vi "NoGV_Omniax_MotorDrive_XYZR_20111213stable2.vi"() -> ()   [LabVIEW 2010]
uses:
  <vilib>/Utility/file.llb/Read From Spreadsheet File (string).vi
  <vilib>/Utility/file.llb/Read From Spreadsheet File (DBL).vi
  <vilib>/Instr/_visa.llb/VISA Configure Serial Port (Instr).vi
  <vilib>/Utility/file.llb/Write To Spreadsheet File (string).vi
  <vilib>/Utility/file.llb/Write To Spreadsheet File (DBL).vi
panel:
  out "Scanning":bool
  out "Laser Shutter":bool
  in  "SHUTTER SYNC":bool
  in  "Laser Shutter":bool
  out "#th loop":dbl
  in  "# of loops":dbl
  in  "LOOP":bool
  out "OP":bool
  out "CL":bool
  out "V5 Valve \nopend/closed":bool
  in  "OK Button":bool
  out "STATUS":string
  in  "Delete Button":bool
  in  "String":string
  in  "Add Button":bool
  in  "Set Button":bool
  in  "Preset positions":i32(ring) items=["ZERO", "Default", "CDOSE", "QMS", "test", "test2", "test3", "yag position", "Sample Long Edge  ", "SPUTTER POS"]
  out "Presets":i32[][](array[numeric])
  out "X MINPOS":i32=-94296
  out "X MAXPOS":i32=-34296
  out "Y MINPOS":i32=-94296
  out "Y MAXPOS":i32=-34296
  out "R MAXPOS":i32=-34296
  out "R MINPOS":i32=-94296
  out "Z MINPOS":i32=-94296
  out "Z MAXPOS":i32=-34296
  in  "HARDSTOP":bool
  in  "GO":bool
  out "XYZR VEL PV Array":i32[](array[numeric])
  out "XYZ in RANGE Array":bool[](array[boolean])
  out "STEP SP Array":i32[](array[numeric])
  out "RUNHOLDArray":i32[](array[numeric])
  out "ZCONSTArray":dbl[](array[numeric])
  out "RCONSTArray":dbl[](array[numeric])
  out "XCONSTArray":dbl[](array[numeric])
  out "YCONSTArray":dbl[](array[numeric])
  out "Error Array":errorcluster[](array[cluster])
  out "COM PORT Array":refnum<visa-resource-name>[](array[refnum])
  out "Z COM PORT":refnum<visa-resource-name>="COM6"
  in  "Tab Control 3":enum32{"Status", "Reset"}(tab)
  out "Y in Range":bool
  out "Y Scan":bool
  out "Y in Motion":bool
  out "Y Backlash corr":bool
  out "X  in Range":bool
  out "X Scan":bool
  out "X  in Motion":bool
  out "X Backlash corr":bool
  out "Z in Range":bool
  out "Z Scan":bool
  out "Z in Motion":bool
  out "Z Backlash corr":bool
  out "R in Range":bool
  out "R Scan":bool
  out "R in Motion":bool
  out "R Backlash corr":bool
  out "X Ready":bool
  out "Y Ready":bool
  out "Z Ready":bool
  out "R Ready":bool
  in  "Reset Y Position mm":dbl
  out "Reset Y Motor Steps":i32
  in  "Reset X Position mm":dbl
  out "Reset X Motor Steps":i32
  in  "Reset Z Position mm":dbl
  out "Reset Z Motor Steps":i32
  in  "Reset R Position deg":dbl
  out "Reset R Motor Steps":i32
  in  "Reset":bool
  in  "Tab Control 2":enum32{"mm", "step"}(tab)
  in  "X Scan Length SP mm":dbl
  in  "X Scan Velocity SP mm/sec":dbl
  in  "Y Scan Length SP mm":dbl
  in  "Y Scan Velocity SP mm/sec":dbl
  in  "Set Scan \nParameters":bool
  in  "Z Scan Length SP mm":dbl
  in  "Z Scan Velocity SP mm/sec":dbl
  in  "R Scan Length SP deg":dbl
  in  "R Scan Velocity SP deg/sec":dbl
  in  "Z as dominating length":bool
  in  "X Scan Velocity SP steps/sec":i32=1 min=1 max=102400 step=1
  in  "X Scan Length SP steps":i32 min=-2304000 max=2304000 step=100
  out "X Scan length MV mm":dbl
  out "X Scan velocity MV mm/sec":dbl format="%#_6f"
  in  "Y Scan Velocity SP steps/sec":i32=1 min=1 max=102400 step=1
  in  "Y Scan Length SP steps":i32 min=-2304000 max=2304000 step=100
  out "Y Scan length MV mm":dbl
  out "Y Scan velocity MV mm/sec":dbl format="%#_6f"
  in  "Z Scan Velocity SP steps/sec":i32=1 min=1 max=204800 step=1
  in  "Z Scan Length SP steps":i32 min=-10240000 max=92160000 step=100
  out "Z Scan length MV mm":dbl
  out "Z Scan velocity MV mm/sec":dbl format="%#_6f"
  in  "R Scan Velocity SP steps/sec":i32=1 min=1 max=102400 step=1
  in  "R Scan Length SP steps":i32 min=-1501867 max=4642133 step=100
  out "R Scan length MV deg":dbl
  out "R Scan velocity MV deg/sec":dbl format="%#_6f"
  out "atan Y/Z":dbl
  in  "Tab Control":enum32{"mm", "step"}(tab)
  in  "X Position SP mm":dbl
  in  "X Velocity SP mm/sec":dbl
  in  "X Move Set":bool
  in  "Y Move Set":bool
  in  "Y Position SP mm":dbl
  in  "Y Velocity SP mm/sec":dbl
  in  "Z Position SP mm":dbl
  in  "Z Velocity SP mm/sec":dbl
  in  "Z Move Set":bool
  in  "R Position SP deg":dbl
  in  "R Velocity SP deg/sec":dbl
  in  "R Move Set":bool
  in  "X Velocity SP step/sec":i32 min=1 max=128000
  out "X Velocity MV mm/sec":dbl
  in  "Y Velocity SP step/sec":i32 min=1 max=128000
  out "Y Velocity MV mm/sec":dbl
  in  "Z Velocity SP step/sec":i32 min=1 max=204800
  out "Z Velocity MV mm/sec":dbl
  in  "R Velocity SP step/sec":i32 min=1 max=20000
  out "R Velocity MVdeg/sec":dbl
  in  "Y Step SP":i32=-20000 min=-2304000 max=2304000 step=500
  out "Y Position MV mm":dbl
  in  "X Step SP":i32=-20000 min=-2304000 max=2304000 step=500
  out "X Position MV mm":dbl
  in  "Z Step SP":i32=-20000 min=0 max=102400000 step=500
  out "Z Position MV mm":dbl
  in  "R Step SP":i32=-20000 min=-6144000 max=0 step=500
  out "R Position MV deg":dbl
  out "X Step PV":i32 max=2000
  out "Y Step PV":i32 max=2000
  out "Z Step PV":i32 max=2000
  out "R Step PV":i32 max=2000
  in  "Clear ZY":bool
  out "ZY Graph":cluster{dbl[], dbl[]}(graph)
  out "ZR Graph":cluster{"Y":dbl[], "Y":dbl[]}[](graph)
  out "XY Graph":cluster{"Y":dbl[], "Y":dbl[]}[](graph)
  out "X Scan Duration":dbl
  out "Y Scan Duration":dbl
  out "Z Scan Duration":dbl
  out "R Scan Duration":dbl
  out "R Backlash steps/sec":i32
  out "R Backlash":i32
  out "R Holding Current %":i32
  out "R Run Current %":i32
  out "R offset deg":dbl
  out "R deg/rev":dbl
  out "R steps/rev":u32
  out "R velocity PV step/sec":i32
  out "R COM PORT":refnum<visa-resource-name>="COM5"
  out "R Position deg PV":dbl=270.5
  out "Z Backlash steps/sec":i32
  out "Z Backlash":i32
  out "Z Holding Current %":i32
  out "Z Run Current %":i32
  out "Z offset mm":dbl
  out "Z mm/rev":dbl
  out "Z steps/rev":u32
  out "Z  velocity PV step/sec":i32
  out "Z Position mm PV":dbl=45.0
  out "X Position mm PV":dbl
  out "X velocity PV step/sec":i32
  in  "Send scan parameter":bool
  out "X Backlash steps/sec":i32
  out "X Backlash":i32
  out "X Holding Current %":i32
  out "X Run Current %":i32
  out "X offset mm":dbl
  out "X mm/rev":dbl
  out "X steps/rev":u32
  out "X COM PORT":refnum<visa-resource-name>="COM5"
  out "Y Backlash steps/sec":i32
  out "Y Backlash":i32
  out "Y Holding Current %":i32
  out "Y Run Current %":i32
  in  "Scan Cancel":bool
  out "Y Position mm PV":dbl
  out "Y offset mm":dbl
  out "Y mm/rev":dbl
  out "Y steps/rev":u32
  out "Y velocity PV step/sec":i32
  in  "Scan Go":bool
  in  "Stop":bool
  out "Y COM PORT":refnum<visa-resource-name>="COM5"
  # "MX"
  # "MY"
  # "MZ"
  # "MR"
  # "V5 Indicators"
  # "L"
  # "M"
  # "B"
  # "S"
  # "R"
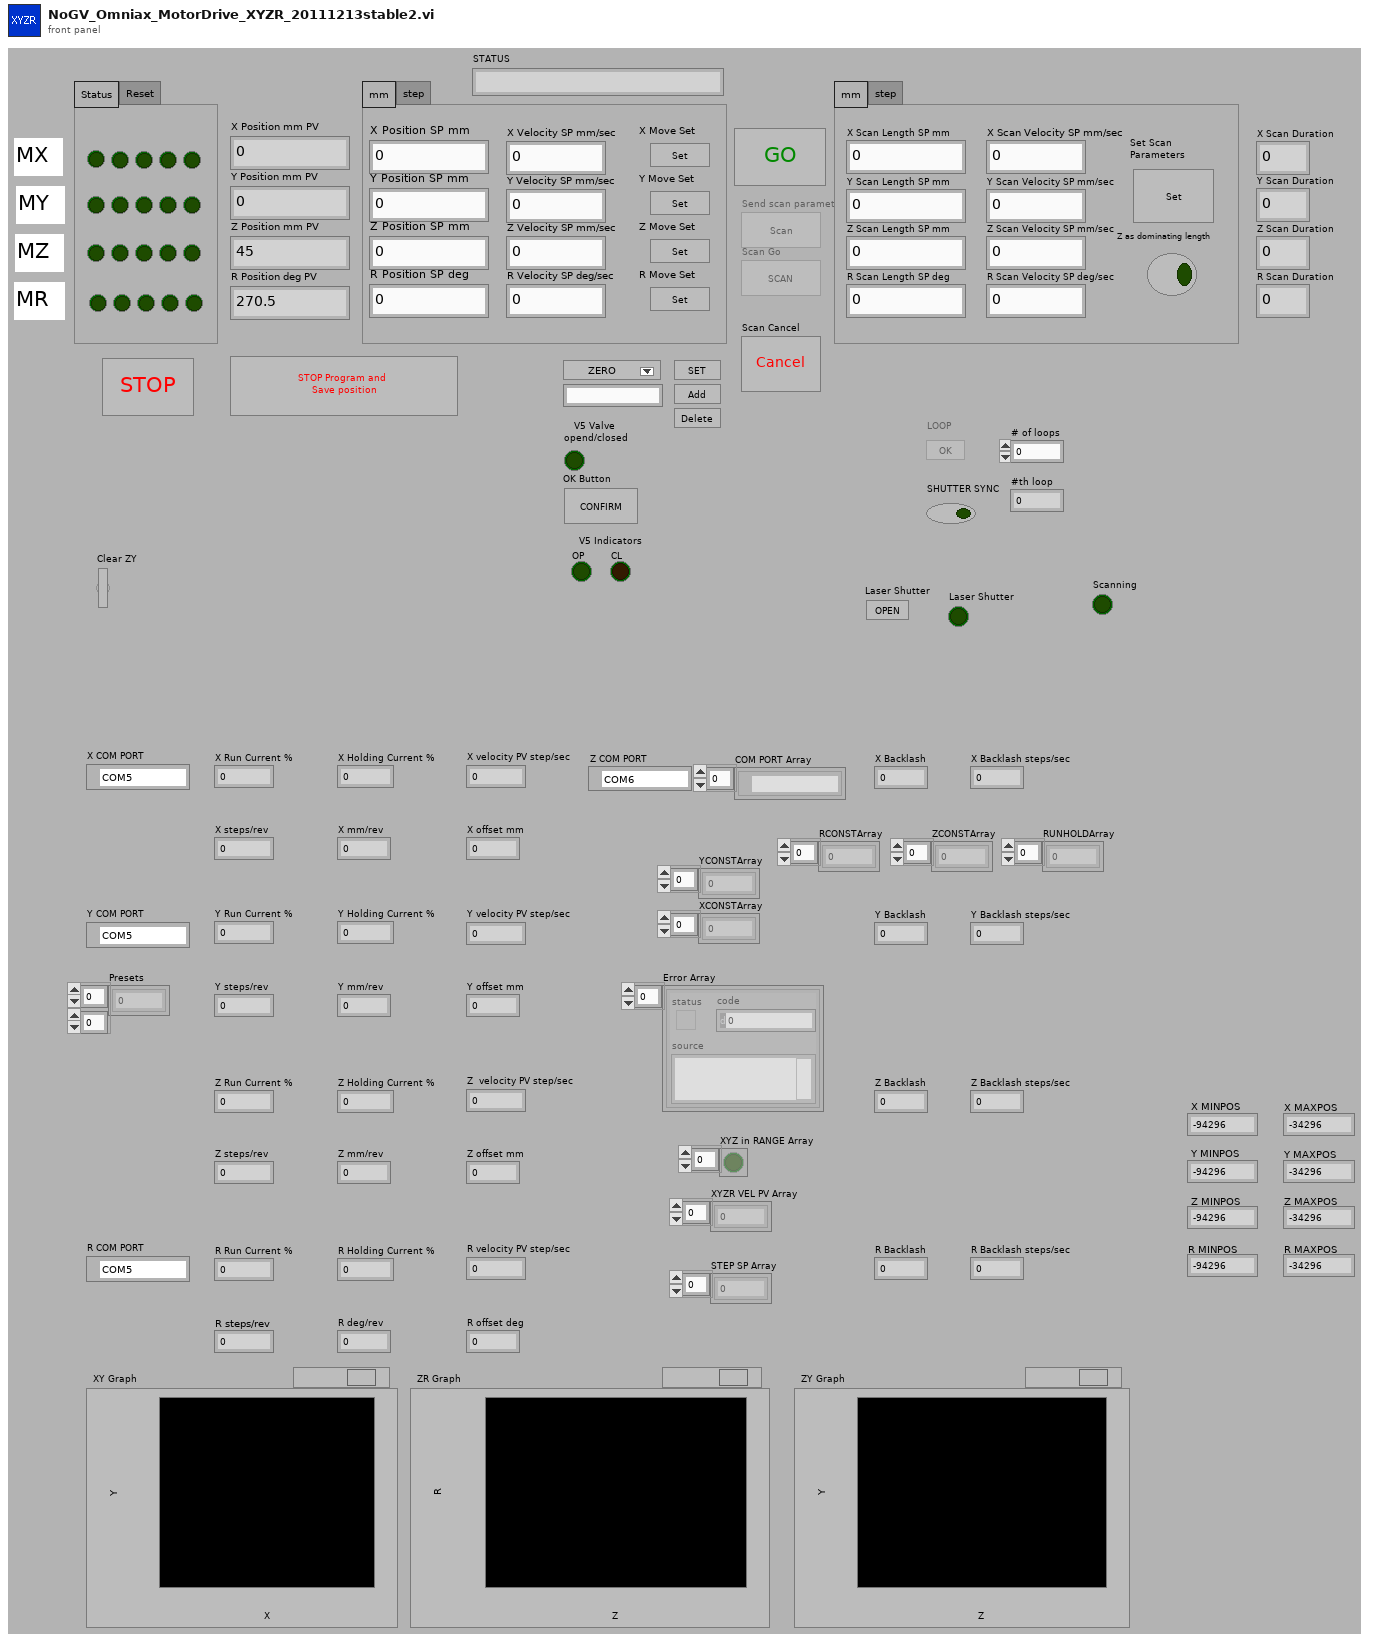
[diagram p1: front panel]
types:
  T1 = cluster{"Error Array OUT[0]":errorcluster, "Error Array OUT[1]":errorcluster, "Error Array OUT[2]":errorcluster, "Error Array OUT[3]":errorcluster, "Error Array OUT[4]":errorcluster, "Error Array OUT[5]":errorcluster, "Error Array OUT[6]":errorcluster, "Error Array OUT[7]":errorcluster, "Error Array OUT[8]":errorcluster}
  T2 = cluster{"COM PORT Array OUT[0]":refnum<visa-resource-name>, "COM PORT Array OUT[1]":refnum<visa-resource-name>, "COM PORT Array OUT[2]":refnum<visa-resource-name>, "COM PORT Array OUT[3]":refnum<visa-resource-name>, "COM PORT Array OUT[4]":refnum<visa-resource-name>, "COM PORT Array OUT[5]":refnum<visa-resource-name>, "COM PORT Array OUT[6]":refnum<visa-resource-name>, "COM PORT Array OUT[7]":refnum<visa-resource-name>, "COM PORT Array OUT[8]":refnum<visa-resource-name>}
  T3 = cluster{"STEP SP Array OUT[0]":i32, "STEP SP Array OUT[1]":i32, "STEP SP Array OUT[2]":i32, "STEP SP Array OUT[3]":i32, "STEP SP Array OUT[4]":i32, "STEP SP Array OUT[5]":i32, "STEP SP Array OUT[6]":i32, "STEP SP Array OUT[7]":i32, "STEP SP Array OUT[8]":i32}
  T4 = cluster{"XYZR MAX MIN POS[0]":i32, "XYZR MAX MIN POS[1]":i32, "XYZR MAX MIN POS[2]":i32, "XYZR MAX MIN POS[3]":i32, "XYZR MAX MIN POS[4]":i32, "XYZR MAX MIN POS[5]":i32, "XYZR MAX MIN POS[6]":i32, "XYZR MAX MIN POS[7]":i32, "XYZR MAX MIN POS[8]":i32}
  T5 = cluster{"XYZ in RANGE Array OUT[0]":bool, "XYZ in RANGE Array OUT[1]":bool, "XYZ in RANGE Array OUT[2]":bool, "XYZ in RANGE Array OUT[3]":bool, "XYZ in RANGE Array OUT[4]":bool, "XYZ in RANGE Array OUT[5]":bool, "XYZ in RANGE Array OUT[6]":bool, "XYZ in RANGE Array OUT[7]":bool, "XYZ in RANGE Array OUT[8]":bool}
  T6 = cluster{"XY Max Min array OUT[0]":dbl, "XY Max Min array OUT[1]":dbl, "XY Max Min array OUT[2]":dbl, "XY Max Min array OUT[3]":dbl, "XY Max Min array OUT[4]":dbl, "XY Max Min array OUT[5]":dbl, "XY Max Min array OUT[6]":dbl, "XY Max Min array OUT[7]":dbl, "XY Max Min array OUT[8]":dbl}
  T7 = cluster{"XYZR VEL PV Array OUT[0]":i32, "XYZR VEL PV Array OUT[1]":i32, "XYZR VEL PV Array OUT[2]":i32, "XYZR VEL PV Array OUT[3]":i32, "XYZR VEL PV Array OUT[4]":i32, "XYZR VEL PV Array OUT[5]":i32, "XYZR VEL PV Array OUT[6]":i32, "XYZR VEL PV Array OUT[7]":i32, "XYZR VEL PV Array OUT[8]":i32}
  T8 = cluster{"[0]":i32, "[1]":i32, "[2]":i32, "[3]":i32, "[4]":i32, "[5]":i32, "[6]":i32, "[7]":i32, "[8]":i32}
  T9 = enum8{"Enabled", "Disabled", "Disabled and Grayed Out"}
  T10 = enum16{"Stop", "Reset", "Run Current", "Holding Current", "Accel Rate", "Decel Rate", "Move to Relative Position", "Move to Absolute Position", "Echo Mode", "Print Parameter", "Send String", "Microstep Resolution", "Set Current Position", "Max Velocity"}
  T11 = cluster{"Presets[0]":i32, "Presets[1]":i32, "Presets[2]":i32, "Presets[3]":i32, "Presets[4]":i32, "Presets[5]":i32, "Presets[6]":i32, "Presets[7]":i32, "Presets[8]":i32}
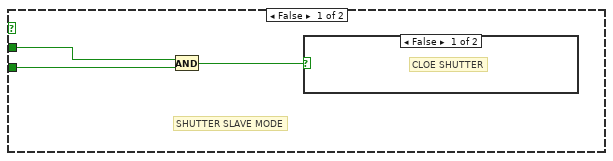
[diagram p2: hidden frame]
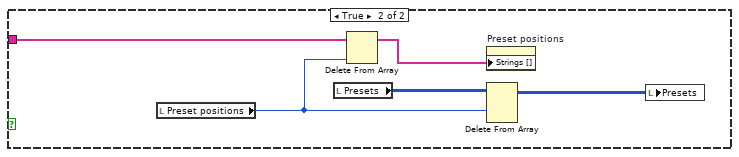
[diagram p4: hidden frame]
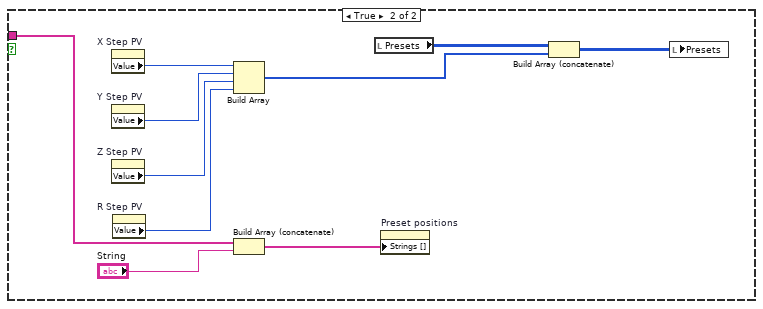
[diagram p5: hidden frame]
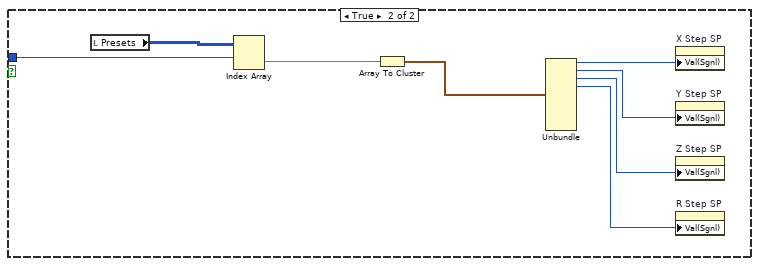
[diagram p6: hidden frame]
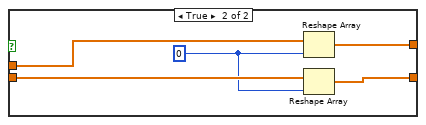
[diagram p8: hidden frame]
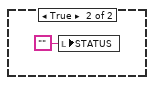
[diagram p10: hidden frame]
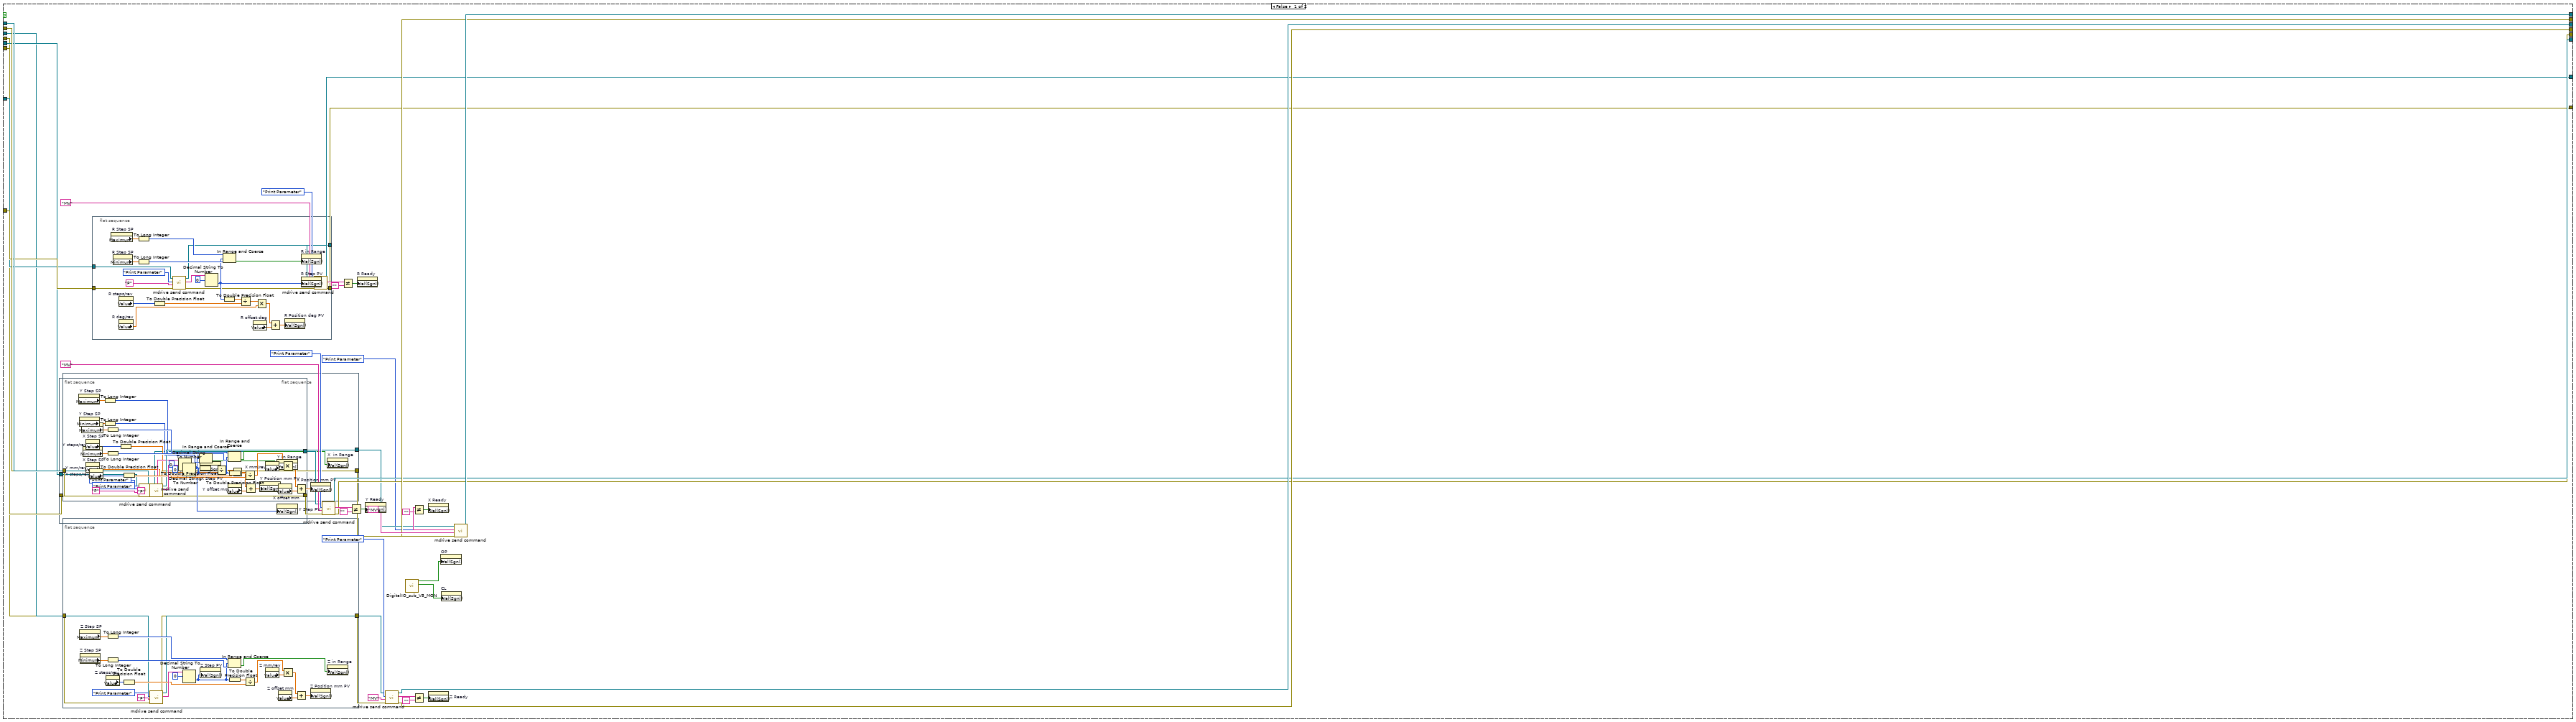
[diagram p11: hidden frame]
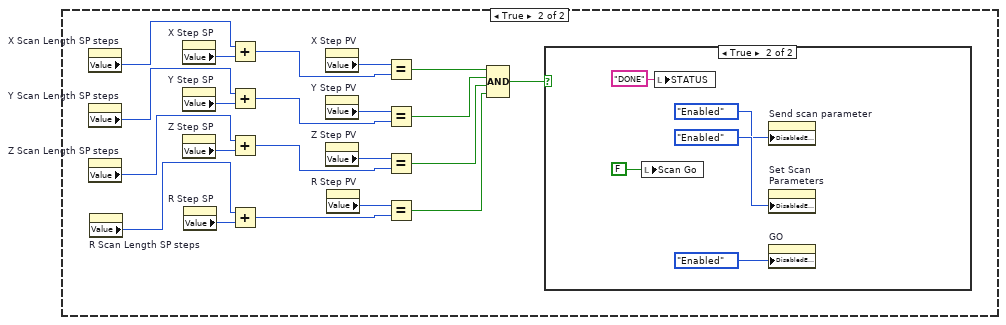
[diagram p14: hidden frame]
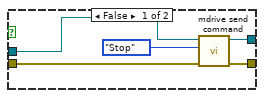
[diagram p16: hidden frame]
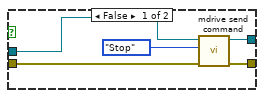
[diagram p18: hidden frame]
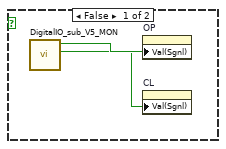
[diagram p20: hidden frame]
diagram:
  (unwired) FALSE ("LOOP MODE")
  n1 = flat-sequence {
    tunnel: [w153] -> w10
    tunnel: [w152] -> w9
    tunnel: [w151] -> w8
    tunnel: [w150] -> w7
    tunnel: [w149] -> w6
    tunnel: [w148] -> w5
    tunnel: [w147] -> w4
    tunnel: [w146] -> w3
    tunnel: [w143] -> w2
    tunnel: [w113] -> w1
    tunnel: [w188] -> w13
    tunnel: [w189] -> w14
    tunnel: [w190] -> w15
    tunnel: [w191] -> w16
    tunnel: [w192] -> w17
    tunnel: [w193] -> w18
    tunnel: [w194] -> w19
    tunnel: [w195] -> w20
    tunnel: [w196] -> w21
    tunnel: [w197] -> w22
    tunnel: w10 -> [w197]
    tunnel: w9 -> [w196]
    tunnel: w8 -> [w195]
    tunnel: w7 -> [w194]
    tunnel: w6 -> [w193]
    tunnel: w5 -> [w192]
    tunnel: w4 -> [w191]
    tunnel: w3 -> [w190]
    tunnel: w2 -> [w189]
    tunnel: w1 -> [w188]
    frame #0 {
      w113 = path "C:/Documents and Settings/b_ogasawara/Desktop/lv1/LV codes/IMS/PRESET.TXT"
      w111 = 0 ("element")
      w143 = path "C:/Documents and Settings/b_ogasawara/Desktop/lv1/LV codes/IMS/POS.TXT"
      w173 = refnum<visa-resource-name> "COM7" ("COM PORT")
      w174 = refnum<visa-resource-name> "COM5" ("COM PORT")
      w175 = refnum<visa-resource-name> "COM6" ("VISA resource name")
      w176 = refnum<visa-resource-name> "COM4" ("COM PORT")
      n2 = property on="Z Step SP" class="DigNum (strict)"() -> ("Maximum"=w68:dbl)  [unwired: 2 in, 2 out]
      n3 = property on="R Step SP" class="DigNum (strict)"() -> ("Maximum"=w66:dbl)  [unwired: 2 in, 2 out]
      n4 = property on="Z Step SP" class="DigNum (strict)"() -> ("Minimum"=w69:dbl)  [unwired: 2 in, 2 out]
      n5 = property on="R Step SP" class="DigNum (strict)"() -> ("Minimum"=w67:dbl)  [unwired: 2 in, 2 out]
      n6 = property on="X steps/rev" class="DigNum (strict)"() -> ("Value"=w84:u32)  [unwired: 2 in, 2 out]
      n7 = property on="Y steps/rev" class="DigNum (strict)"() -> ("Value"=w83:u32)  [unwired: 2 in, 2 out]
      n8 = property on="Z steps/rev" class="DigNum (strict)"() -> ("Value"=w82:u32)  [unwired: 2 in, 2 out]
      n9 = property on="R steps/rev" class="DigNum (strict)"() -> ("Value"=w81:u32)  [unwired: 2 in, 2 out]
      n10 = call "DigitalIO_sub_V5_MON.vi"() -> ("CL"=w70:bool, "OP"=w71:bool)  [unwired: 8 in]
      n11 = local read "RUNHOLDArray"() -> (w163:i32[])
      n12 = local read "STEP SP Array"() -> (w166:i32[])
      n13 = local read "XYZ in RANGE Array"() -> (w165:bool[])
      n14 = local read "XYZR VEL PV Array"() -> (w164:i32[])
      n15 = property on="R offset deg" class="DigNum (strict)"() -> ("Value"=w76:dbl)  [unwired: 2 in, 2 out]
      n16 = property on="X offset mm" class="DigNum (strict)"() -> ("Value"=w73:dbl)  [unwired: 2 in, 2 out]
      n17 = property on="Y offset mm" class="DigNum (strict)"() -> ("Value"=w74:dbl)  [unwired: 2 in, 2 out]
      n18 = property on="Z offset mm" class="DigNum (strict)"() -> ("Value"=w75:dbl)  [unwired: 2 in, 2 out]
      n19 = property on="OP" class="Bool (strict)"("Val(Sgnl)"=w71) -> ()  [unwired: 2 in, 2 out]
      n20 = property on="CL" class="Bool (strict)"("Val(Sgnl)"=w70) -> ()  [unwired: 2 in, 2 out]
      n21 = Build Array(w176, w175, w174, w173) -> (w171:refnum<visa-resource-name>[])
      n22 = Build Array(w68, w69, w66, w67) -> (w65:dbl[])
      n23 = local write "STATUS"("INITIALIZING" ("STATUS")) -> ()
      n24 = for {
        N: 4 -> [_]
        tunnel: w171 -> [w179] mode=indexing
        tunnel: [w178] -> w169 mode=indexing
        tunnel: [w177] -> w170 mode=indexing
        w181 = u16 0 items=["None", "XON/XOFF", "RTS/CTS", "XON/XOFF & RTS/CTS", "DTR/DSR", "XON/XOFF & DTR/DSR"] ("flow control (0:none)")
        w182 = u16 10 items=["1.0"=10, "1.5"=15, "2.0"=20] ("stop bits (10: 1 bit)")
        # "Stop bits"
        n25 = call-poly "VISA Configure Serial Port"("VISA resource name"=w179, "timeout (10sec)"=u32 10000, "baud rate (9600)"=u32 9600, "data bits (8)"=u16 8, "parity (0:none)"=enum16{"None", "Odd", "Even", "Mark", "Space"}."None", "stop bits (10: 1 bit)"=w182, "flow control (0:none)"=w181) -> ("VISA resource name out"=w178:refnum<visa-resource-name>, "error out"=w177:errorcluster)  [unwired: 7 in]
      }
      "COM PORT Array" <- w169
      "Error Array" <- w170
      n26 = call "InitializeMotorsXYZR_V2.vi"("COM PORT Array IN"=w169, "STEP SP Array IN"=w166, "XYZ in RANGE Array IN"=w165, "XYZR VEL PV Array IN"=w164, "RUNHOLDArray IN"=w163, "Error Array IN"=w170, "ZR Max Min array"=w65) -> ("XY Max Min array OUT"=w64:dbl[], "COM PORT Array OUT"=w168:refnum<visa-resource-name>[], "STEP SP Array OUT"=w162:i32[], "XYZ in RANGE Array OUT"=w161:bool[], "XYZR VEL PV Array OUT"=w160:i32[], "XYZR MAX MIN POS"=w145:i32[], "Error Array OUT"=w167:errorcluster[])  [unwired: 6 in]
      n27 = Array To Cluster(array=w167) -> (cluster=w158:T1)
      n28 = Array To Cluster(array=w168) -> (cluster=w159:T2)
      n29 = Array To Cluster(array=w162) -> (cluster=w157:T3)
      n30 = Array To Cluster(array=w145) -> (cluster=w154:T4)
      n31 = Array To Cluster(array=w161) -> (cluster=w156:T5)
      n32 = Array To Cluster(array=w64) -> (cluster=w63:T6)
      n33 = Array To Cluster(array=w160) -> (cluster=w155:T7)
      n34 = Unbundle(w157) -> ("STEP SP Array OUT[0]"=w127:i32, "STEP SP Array OUT[1]"=w128:i32, "STEP SP Array OUT[2]"=w129:i32, "STEP SP Array OUT[3]"=w130:i32)  [unwired: 5 out]
      n35 = Unbundle(w154) -> ("XYZR MAX MIN POS[0]"=w138:i32, "XYZR MAX MIN POS[1]"=w137:i32, "XYZR MAX MIN POS[2]"=w136:i32, "XYZR MAX MIN POS[3]"=w135:i32, "XYZR MAX MIN POS[4]"=w134:i32, "XYZR MAX MIN POS[5]"=w133:i32, "XYZR MAX MIN POS[6]"=w132:i32, "XYZR MAX MIN POS[7]"=w131:i32)  [unwired: 1 out]
      n36 = Unbundle(w156) -> ("XYZ in RANGE Array OUT[0]"=w142:bool, "XYZ in RANGE Array OUT[1]"=w141:bool, "XYZ in RANGE Array OUT[2]"=w140:bool, "XYZ in RANGE Array OUT[3]"=w139:bool)  [unwired: 5 out]
      n37 = Unbundle(w63) -> ("XY Max Min array OUT[0]"=w62:dbl, "XY Max Min array OUT[1]"=w60:dbl, "XY Max Min array OUT[2]"=w59:dbl, "XY Max Min array OUT[3]"=w61:dbl)  [unwired: 5 out]
      n38 = Unbundle(w155) -> ("XYZR VEL PV Array OUT[0]"=w126:i32, "XYZR VEL PV Array OUT[1]"=w125:i32, "XYZR VEL PV Array OUT[2]"=w124:i32, "XYZR VEL PV Array OUT[3]"=w123:i32)  [unwired: 5 out]
      n39 = call-poly <vilib>:"Read From Spreadsheet File.vi"("file path (dialog if empty)"=w113) -> ("all rows"=w118:string[][])  [unwired: 6 in, 4 out]
      n40 = call-poly <vilib>:"Read From Spreadsheet File.vi"("file path (dialog if empty)"=w143) -> ("first row"=w144:dbl[])  [unwired: 6 in, 4 out]
      n41 = To Long Integer(number=w144) -> (32bit integer=w110:i32[])
      n42 = Transpose 2D Array(2D array=w118) -> (transposed array=w117:string[][])
      n43 = property on="X Step SP" class="DigNum (strict)"("Val(Sgnl)"=w127) -> ()  [unwired: 2 in, 2 out]
      n44 = property on="Y Step SP" class="DigNum (strict)"("Val(Sgnl)"=w128) -> ()  [unwired: 2 in, 2 out]
      n45 = property on="Z Step SP" class="DigNum (strict)"("Val(Sgnl)"=w129) -> ()  [unwired: 2 in, 2 out]
      n46 = property on="R Step SP" class="DigNum (strict)"("Val(Sgnl)"=w130) -> ()  [unwired: 2 in, 2 out]
      n47 = property on="X MAXPOS" class="DigNum (strict)"("Val(Sgnl)"=w138) -> ()  [unwired: 2 in, 2 out]
      n48 = property on="X MINPOS" class="DigNum (strict)"("Val(Sgnl)"=w137) -> ()  [unwired: 2 in, 2 out]
      n49 = property on="Y MAXPOS" class="DigNum (strict)"("Val(Sgnl)"=w136) -> ()  [unwired: 2 in, 2 out]
      n50 = property on="Y MINPOS" class="DigNum (strict)"("Val(Sgnl)"=w135) -> ()  [unwired: 2 in, 2 out]
      n51 = property on="Z MAXPOS" class="DigNum (strict)"("Val(Sgnl)"=w134) -> ()  [unwired: 2 in, 2 out]
      n52 = property on="Z MINPOS" class="DigNum (strict)"("Val(Sgnl)"=w133) -> ()  [unwired: 2 in, 2 out]
      n53 = property on="R MAXPOS" class="DigNum (strict)"("Val(Sgnl)"=w132) -> ()  [unwired: 2 in, 2 out]
      n54 = property on="R MINPOS" class="DigNum (strict)"("Val(Sgnl)"=w131) -> ()  [unwired: 2 in, 2 out]
      n55 = property on="X  in Range" class="Bool (strict)"("Val(Sgnl)"=w142) -> ()  [unwired: 2 in, 2 out]
      n56 = property on="Y in Range" class="Bool (strict)"("Val(Sgnl)"=w141) -> ()  [unwired: 2 in, 2 out]
      n57 = property on="Z in Range" class="Bool (strict)"("Val(Sgnl)"=w140) -> ()  [unwired: 2 in, 2 out]
      n58 = property on="R in Range" class="Bool (strict)"("Val(Sgnl)"=w139) -> ()  [unwired: 2 in, 2 out]
      n59 = property on="X velocity PV step/sec" class="DigNum (strict)"("Val(Sgnl)"=w126) -> ()  [unwired: 2 in, 2 out]
      n60 = property on="R velocity PV step/sec" class="DigNum (strict)"("Val(Sgnl)"=w123) -> ()  [unwired: 2 in, 2 out]
      n61 = property on="X Step SP" class="DigNum (strict)"("Maximum"=w62) -> ()  [unwired: 2 in, 2 out]
      n62 = property on="X Step SP" class="DigNum (strict)"("Minimum"=w60) -> ()  [unwired: 2 in, 2 out]
      n63 = property on="Y Step SP" class="DigNum (strict)"("Maximum"=w59) -> ()  [unwired: 2 in, 2 out]
      n64 = property on="Y Step SP" class="DigNum (strict)"("Minimum"=w61) -> ()  [unwired: 2 in, 2 out]
      n65 = property on="Y velocity PV step/sec" class="DigNum (strict)"("Val(Sgnl)"=w125) -> ()  [unwired: 2 in, 2 out]
      n66 = property on="Z  velocity PV step/sec" class="DigNum (strict)"("Val(Sgnl)"=w124) -> ()  [unwired: 2 in, 2 out]
      n67 = Array To Cluster(array=w110) -> (cluster=w109:T8)
      n68 = Delete From Array(array=w117, index (row)=0) -> (deleted portion=w112:string[], array with subset deleted=w115:string[][])  [unwired: 2 in]
      n69 = Transpose 2D Array(2D array=w115) -> (transposed array=w114:string[][])
      n70 = property on="Preset positions" class="Ring (strict)"("Strings []"=w112) -> ()  [unwired: 2 in, 2 out]
      n71 = Unbundle(w109) -> ("[0]"=w85:i32, "[1]"=w86:i32, "[2]"=w87:i32, "[3]"=w88:i32)  [unwired: 5 out]
      n72 = To Double Precision Float(number=w84) -> (double precision float=w105:dbl)
      n73 = To Double Precision Float(number=w85) -> (double precision float=w106:dbl)
      n74 = To Double Precision Float(number=w83) -> (double precision float=w101:dbl)
      n75 = To Double Precision Float(number=w86) -> (double precision float=w102:dbl)
      n76 = To Double Precision Float(number=w87) -> (double precision float=w98:dbl)
      n77 = To Double Precision Float(number=w82) -> (double precision float=w97:dbl)
      n78 = To Double Precision Float(number=w88) -> (double precision float=w94:dbl)
      n79 = To Double Precision Float(number=w81) -> (double precision float=w93:dbl)
      n80 = property on="Reset X Motor Steps" class="DigNum (strict)"("Val(Sgnl)"=w85) -> ()  [unwired: 2 in, 2 out]
      n81 = property on="Reset Y Motor Steps" class="DigNum (strict)"("Val(Sgnl)"=w86) -> ()  [unwired: 2 in, 2 out]
      n82 = property on="Reset Z Motor Steps" class="DigNum (strict)"("Val(Sgnl)"=w87) -> ()  [unwired: 2 in, 2 out]
      n83 = property on="Reset R Motor Steps" class="DigNum (strict)"("Val(Sgnl)"=w88) -> ()  [unwired: 2 in, 2 out]
      n84 = Decimal String To Number(string=w114) -> (number=w116:i32[][])  [unwired: 2 in, 1 out]
      n85 = Divide(x=w106, y=w105) -> (x/y=w108:dbl)
      n86 = Divide(x=w102, y=w101) -> (x/y=w104:dbl)
      n87 = Divide(x=w98, y=w97) -> (x/y=w100:dbl)
      n88 = Divide(x=w94, y=w93) -> (x/y=w96:dbl)
      n89 = Initialize Array(w111, w111, 4 ("dimension size")) -> (w121:i32[][])
      n90 = Build Array (concatenate)(w121, w116) -> (→"Presets":i32[][])
      n91 = property on="X mm/rev" class="DigNum (strict)"() -> ("Value"=w78:dbl)  [unwired: 2 in, 2 out]
      n92 = property on="Y mm/rev" class="DigNum (strict)"() -> ("Value"=w79:dbl)  [unwired: 2 in, 2 out]
      n93 = property on="Z mm/rev" class="DigNum (strict)"() -> ("Value"=w80:dbl)  [unwired: 2 in, 2 out]
      n94 = property on="R deg/rev" class="DigNum (strict)"() -> ("Value"=w77:dbl)  [unwired: 2 in, 2 out]
      n95 = Multiply(x=w108, y=w78) -> (x*y=w107:dbl)
      n96 = Multiply(x=w104, y=w79) -> (x*y=w103:dbl)
      n97 = Multiply(x=w100, y=w80) -> (x*y=w99:dbl)
      n98 = Multiply(x=w96, y=w77) -> (x*y=w95:dbl)
      n99 = Add(x=w107, y=w73) -> (x+y=w89:dbl)
      n100 = Add(x=w103, y=w74) -> (x+y=w90:dbl)
      n101 = Add(x=w99, y=w75) -> (x+y=w91:dbl)
      n102 = Add(x=w95, y=w76) -> (x+y=w92:dbl)
      n103 = property on="X Position mm PV" class="DigNum (strict)"("Val(Sgnl)"=w89) -> ()  [unwired: 2 in, 2 out]
      n104 = property on="X Position SP mm" class="DigNum (strict)"("Val(Sgnl)"=w89) -> ()  [unwired: 2 in, 2 out]
      n105 = property on="Y Position SP mm" class="DigNum (strict)"("Val(Sgnl)"=w90) -> ()  [unwired: 2 in, 2 out]
      n106 = property on="Y Position mm PV" class="DigNum (strict)"("Val(Sgnl)"=w90) -> ()  [unwired: 2 in, 2 out]
      n107 = property on="Z Position SP mm" class="DigNum (strict)"("Val(Sgnl)"=w91) -> ()  [unwired: 2 in, 2 out]
      n108 = property on="Z Position mm PV" class="DigNum (strict)"("Val(Sgnl)"=w91) -> ()  [unwired: 2 in, 2 out]
      n109 = property on="R Position deg PV" class="DigNum (strict)"("Val(Sgnl)"=w92) -> ()  [unwired: 2 in, 2 out]
      n110 = property on="R Position SP deg" class="DigNum (strict)"("Val(Sgnl)"=w92) -> ()  [unwired: 2 in, 2 out]
      n111 = Unbundle(w159) -> ("COM PORT Array OUT[0]"=w153:refnum<visa-resource-name>, "COM PORT Array OUT[1]"=w152:refnum<visa-resource-name>, "COM PORT Array OUT[2]"=w151:refnum<visa-resource-name>, "COM PORT Array OUT[3]"=w150:refnum<visa-resource-name>)  [unwired: 5 out]
      n112 = Unbundle(w158) -> ("Error Array OUT[0]"=w149:errorcluster, "Error Array OUT[1]"=w148:errorcluster, "Error Array OUT[2]"=w147:errorcluster, "Error Array OUT[3]"=w146:errorcluster)  [unwired: 5 out]
      "X COM PORT" <- w176
      "Z COM PORT" <- w175
      "Y COM PORT" <- w174
      "R COM PORT" <- w173
    }
    frame #1 {
      w186 = T9."Disabled and Grayed Out" ("Disabled")
      w187 = T9."Enabled" ("Disabled")
      n113 = property on="LOOP" class="Bool (strict)"("DisabledEnum"=w186) -> ()  [unwired: 2 in, 2 out]
      n114 = property on="GO" class="Bool"("DisabledEnum"=w187) -> ()  [unwired: 2 in, 2 out]
      n115 = property on="Set Scan \nParameters" class="Bool"("DisabledEnum"=w187) -> ()  [unwired: 2 in, 2 out]
      n116 = property on="Send scan parameter" class="Bool"("DisabledEnum"=w186) -> ()  [unwired: 2 in, 2 out]
    }
  }
  n117 = local read "X  in Range"() -> (w33:bool)
  n118 = local read "Z  velocity PV step/sec"() -> (w26:i32)
  n119 = local read "Y in Range"() -> (w32:bool)
  n120 = local read "Z in Range"() -> (w31:bool)
  n121 = local read "R in Range"() -> (w30:bool)
  n122 = local read "X velocity PV step/sec"() -> (w29:i32)
  n123 = local read "Y velocity PV step/sec"() -> (w27:i32)
  n124 = local read "R velocity PV step/sec"() -> (w28:i32)
  n125 = flat-sequence {
    frame #0 {
      n126 = property on="Y Scan" class="Bool (strict)"("Val(Sgnl)"=FALSE ("Value (Signaling)")) -> ()  [unwired: 2 in, 2 out]
      n127 = property on="Z Scan Velocity SP mm/sec" class="DigNum (strict)"("Val(Sgnl)"=0.1 ("Value (Signaling)")) -> ()  [unwired: 2 in, 2 out]
      n128 = property on="Z Scan Velocity SP steps/sec" class="DigNum (strict)"("Minimum"=1.0 ("Data Entry Limits:Maximum")) -> ()  [unwired: 2 in, 2 out]
      n129 = property on="R Scan" class="Bool (strict)"("Val(Sgnl)"=FALSE ("Value (Signaling)")) -> ()  [unwired: 2 in, 2 out]
      n130 = property on="X Scan Velocity SP mm/sec" class="DigNum (strict)"("Val(Sgnl)"=0.1 ("Value (Signaling)")) -> ()  [unwired: 2 in, 2 out]
      n131 = property on="R Velocity SP deg/sec" class="DigNum (strict)"("Val(Sgnl)"=0.1 ("Value (Signaling)")) -> ()  [unwired: 2 in, 2 out]
      n132 = property on="Z Scan Velocity SP steps/sec" class="DigNum (strict)"("Maximum"=204800.0 ("Data Entry Limits:Maximum")) -> ()  [unwired: 2 in, 2 out]
      n133 = property on="X Scan" class="Bool (strict)"("Val(Sgnl)"=FALSE ("Value (Signaling)")) -> ()  [unwired: 2 in, 2 out]
      n134 = property on="Y Scan Velocity SP mm/sec" class="DigNum (strict)"("Val(Sgnl)"=0.1 ("Value (Signaling)")) -> ()  [unwired: 2 in, 2 out]
      n135 = property on="Z Scan" class="Bool (strict)"("Val(Sgnl)"=FALSE ("Value (Signaling)")) -> ()  [unwired: 2 in, 2 out]
      n136 = property on="Scan Go" class="Bool (strict)"("DisabledEnum"=T9."Disabled and Grayed Out" ("Disabled")) -> ()  [unwired: 2 in, 2 out]
    }
  }
  n137 = flat-sequence {
    tunnel: [w212] -> w45
    frame #0 {
      w210 = 0.2 ("MM/rev")
      w215 = u32 51200 ("step/rev")
      w217 = 128000 ("Value (Signaling)")
      w218 = 1.0 ("Data Entry Limits:Minimum")
      w211 = 0.0 ("offset")
      # "a=1000000"
      n138 = property on="X Velocity SP step/sec" class="DigNum (strict)"("Val(Sgnl)"=w217) -> ()  [unwired: 2 in, 2 out]
      n139 = To Double Precision Float(number=w215) -> (double precision float=w220:dbl)
      n140 = To Double Precision Float(number=w217) -> (double precision float=w209:dbl)
      n141 = Divide(x=w209, y=w220) -> (x/y=w219:dbl)
      n142 = property on="X Velocity SP step/sec" class="DigNum (strict)"("Maximum"=w209) -> ()  [unwired: 2 in, 2 out]
      n143 = Multiply(x=w219, y=w210) -> (x*y=w213:dbl)
      n144 = To Double Precision Float(number=w217) -> (double precision float=w216:dbl)
      n145 = To Double Precision Float(number=w215) -> (double precision float=w214:dbl)
      n146 = property on="X Velocity SP step/sec" class="DigNum (strict)"("Minimum"=w218) -> ()  [unwired: 2 in, 2 out]
      n147 = Build Array(w218, w216, w214, w213, w209, w210, w211) -> (w212:dbl[])
      n148 = property on="X Velocity SP mm/sec" class="DigNum (strict)"("Val(Sgnl)"=w213) -> ()  [unwired: 2 in, 2 out]
      "X offset mm" <- w211
      "X steps/rev" <- w215
      "X mm/rev" <- w210
    }
  }
  n149 = flat-sequence {
    tunnel: [w224] -> w46
    frame #0 {
      w222 = 0.2 ("MM/rev")
      w227 = u32 51200 ("step/rev")
      w229 = 128000 ("Value (Signaling)")
      w230 = 1.0 ("Data Entry Limits:Minimum")
      w223 = 0.0 ("offset")
      n150 = property on="Y Velocity SP step/sec" class="DigNum (strict)"("Val(Sgnl)"=w229) -> ()  [unwired: 2 in, 2 out]
      n151 = To Double Precision Float(number=w227) -> (double precision float=w232:dbl)
      n152 = To Double Precision Float(number=w229) -> (double precision float=w221:dbl)
      n153 = Divide(x=w221, y=w232) -> (x/y=w231:dbl)
      n154 = property on="Y Velocity SP step/sec" class="DigNum (strict)"("Maximum"=w221) -> ()  [unwired: 2 in, 2 out]
      n155 = Multiply(x=w231, y=w222) -> (x*y=w225:dbl)
      n156 = To Double Precision Float(number=w229) -> (double precision float=w228:dbl)
      n157 = To Double Precision Float(number=w227) -> (double precision float=w226:dbl)
      n158 = property on="Y Velocity SP step/sec" class="DigNum (strict)"("Minimum"=w230) -> ()  [unwired: 2 in, 2 out]
      n159 = Build Array(w230, w228, w226, w225, w221, w222, w223) -> (w224:dbl[])
      n160 = property on="Y Velocity SP mm/sec" class="DigNum (strict)"("Val(Sgnl)"=w225) -> ()  [unwired: 2 in, 2 out]
      "Y offset mm" <- w223
      "Y steps/rev" <- w227
      "Y mm/rev" <- w222
    }
  }
  n161 = flat-sequence {
    frame #0 {
      n162 = property on="X Backlash corr" class="Bool (strict)"("Val(Sgnl)"=FALSE ("Value (Signaling)")) -> ()  [unwired: 2 in, 2 out]
      n163 = property on="Y Backlash corr" class="Bool (strict)"("Val(Sgnl)"=FALSE ("Value (Signaling)")) -> ()  [unwired: 2 in, 2 out]
      n164 = property on="R Backlash corr" class="Bool (strict)"("Val(Sgnl)"=FALSE ("Value (Signaling)")) -> ()  [unwired: 2 in, 2 out]
      n165 = property on="Z Backlash corr" class="Bool (strict)"("Val(Sgnl)"=FALSE ("Value (Signaling)")) -> ()  [unwired: 2 in, 2 out]
      "Z Backlash steps/sec" <- 25600 ("Z Backlash steps/sec")
      "Z Backlash" <- -12800 ("Z Backlash")
      "X Backlash steps/sec" <- 25600 ("Value (Signaling)")
      "X Backlash" <- 5120 ("Backlash2")
      "Y Backlash" <- -5120 ("Backlash2")
      "Y Backlash steps/sec" <- 25600 ("Value (Signaling)")
      "R Backlash steps/sec" <- 6400 ("R Backlash steps/sec")
      "R Backlash" <- -12800 ("R Backlash")
    }
  }
  n166 = flat-sequence {
    tunnel: [w245] -> w43
    frame #0 {
      w247 = 0.2 ("Z mm/rev")
      w251 = u32 51200 ("step/rev")
      w253 = 204800 ("Value (Signaling)")
      w254 = 1.0 ("Data Entry Limits:Minimum")
      w246 = 0.0 ("Z offset mm")
      n167 = property on="Z Velocity SP step/sec" class="DigNum (strict)"("Val(Sgnl)"=w253) -> ()  [unwired: 2 in, 2 out]
      n168 = To Double Precision Float(number=w251) -> (double precision float=w256:dbl)
      n169 = To Double Precision Float(number=w253) -> (double precision float=w249:dbl)
      n170 = Divide(x=w249, y=w256) -> (x/y=w255:dbl)
      n171 = property on="Z Velocity SP step/sec" class="DigNum (strict)"("Maximum"=w249) -> ()  [unwired: 2 in, 2 out]
      n172 = Multiply(x=w255, y=w247) -> (x*y=w248:dbl)
      n173 = To Double Precision Float(number=w251) -> (double precision float=w250:dbl)
      n174 = To Double Precision Float(number=w253) -> (double precision float=w252:dbl)
      n175 = Build Array(w254, w252, w250, w249, w248, w247, w246) -> (w245:dbl[])
      n176 = property on="Z Velocity SP mm/sec" class="DigNum (strict)"("Val(Sgnl)"=w248) -> ()  [unwired: 2 in, 2 out]
      n177 = property on="Z Velocity SP step/sec" class="DigNum (strict)"("Minimum"=w254) -> ()  [unwired: 2 in, 2 out]
      "Z offset mm" <- w246
      "Z mm/rev" <- w247
      "Z steps/rev" <- w251
    }
  }
  n178 = flat-sequence {
    tunnel: [w257] -> w42
    frame #0 {
      w260 = 20 ("R Holding Current %")
      w259 = 40 ("R Run Current %")
      w262 = 20 ("Holding Current %")
      w261 = 40 ("Run Current %")
      w264 = 20 ("Holding Current %")
      w265 = 40 ("Run Current %")
      w263 = 40 ("Z Run Current %")
      w258 = 20 ("Z Holding Current %")
      n179 = Build Array(w265, w264, w263, w262, w261, w260, w259, w258) -> (w257:i32[])
      "Z Holding Current %" <- w258
      "Z Run Current %" <- w263
      "X Run Current %" <- w265
      "X Holding Current %" <- w264
      "Y Run Current %" <- w261
      "Y Holding Current %" <- w262
      "R Holding Current %" <- w260
      "R Run Current %" <- w259
    }
  }
  n180 = flat-sequence {
    tunnel: [w266] -> w44
    frame #0 {
      w275 = 1.0 ("Data Entry Limits:Minimum")
      w269 = 0.0 ("R offset deg")
      w270 = -3.0 ("R deg/rev")
      w273 = u32 51200 ("step/rev")
      w274 = 20000 ("Value (Signaling)")
      n181 = property on="R Velocity SP step/sec" class="DigNum (strict)"("Val(Sgnl)"=w274) -> ()  [unwired: 2 in, 2 out]
      n182 = To Double Precision Float(number=w273) -> (double precision float=w276:dbl)
      n183 = To Double Precision Float(number=w274) -> (double precision float=w272:dbl)
      n184 = Divide(x=w272, y=w276) -> (x/y=w278:dbl)
      n185 = property on="R Velocity SP step/sec" class="DigNum (strict)"("Maximum"=w272) -> ()  [unwired: 2 in, 2 out]
      n186 = Multiply(x=w278, y=w270) -> (x*y=w277:dbl)
      n187 = To Double Precision Float(number=w273) -> (double precision float=w267:dbl)
      n188 = To Double Precision Float(number=w274) -> (double precision float=w268:dbl)
      n189 = Absolute Value(x=w277) -> (abs(x)=w271:dbl)
      n190 = Build Array(w275, w268, w267, w272, w271, w270, w269) -> (w266:dbl[])
      n191 = property on="R Velocity SP deg/sec" class="DigNum (strict)"("Val(Sgnl)"=w271) -> ()  [unwired: 2 in, 2 out]
      n192 = property on="R Velocity SP step/sec" class="DigNum (strict)"("Minimum"=w275) -> ()  [unwired: 2 in, 2 out]
      "R offset deg" <- w269
      "R deg/rev" <- w270
      "R steps/rev" <- w273
    }
  }
  n193 = property on="Z Step SP" class="DigNum (strict)"("Minimum"=0.0 ("lower limit")) -> ()  [unwired: 2 in, 2 out]
  n194 = property on="R Step SP" class="DigNum (strict)"("Maximum"=0.0 ("Data Entry Limits:Maximum")) -> ()  [unwired: 2 in, 2 out]
  n195 = property on="R Step SP" class="DigNum (strict)"("Minimum"=-6144000.0 ("Data Entry Limits:Minimum")) -> ()  [unwired: 2 in, 2 out]
  n196 = property on="Z Step SP" class="DigNum (strict)"("Maximum"=102400000.0 ("upper limit")) -> ()  [unwired: 2 in, 2 out]
  n197 = Build Array(w33, w32, w31, w30) -> (→"XYZ in RANGE Array":bool[])
  n198 = Build Array("X Step SP", "Y Step SP", "Z Step SP", "R Step SP", "X Velocity SP step/sec", "Y Velocity SP step/sec", "Z Velocity SP step/sec", "R Velocity SP step/sec") -> (→"STEP SP Array":i32[])
  n199 = Build Array(w29, w27, w26, w28) -> (→"XYZR VEL PV Array":i32[])
  n200 = while {
    tunnel: [w306] -> w49
    tunnel: [w309] -> w50
    tunnel: [w312] -> w58
    tunnel: [w305] -> w57
    tunnel: [w311] -> w52
    tunnel: [w310] -> w51
    tunnel: [w308] -> w48
    tunnel: [w307] -> w47
    tunnel: w22 -> [w320]
    tunnel: w21 -> [w318]
    tunnel: w20 -> [w316]
    tunnel: w19 -> [w314]
    tunnel: w18 -> [w319]
    tunnel: w17 -> [w317]
    tunnel: w16 -> [w315]
    tunnel: w15 -> [w313]
    tunnel: w14 -> [w302]
    tunnel: w13 -> [w301]
    shift-right: [w295] -> _
    shift-left: dbl[] [] -> [w293]
    shift-right: [w294] -> _
    shift-left: dbl[] [] -> [w292]
    stop <- w303 stop-if-true
    # "XZYR"
    n201 = property on="Preset positions" class="Ring (strict)"() -> ("Strings []"=w296:string[])  [unwired: 2 in, 2 out]
    n202 = event shown="[0] Timeout" {
      selector: _ -> [_ _ _ _ _ _ _ _ _ _ _ _ _ _ _ _ _]
      dyn-events: _ -> [_ _ _ _ _ _ _ _ _ _ _ _ _ _ _ _ _]
      timeout: 100 -> [_ _ _ _ _ _ _ _ _ _ _ _ _ _ _ _ _]
      tunnel: w320 -> [w524 _ w1390 w1686 _ _ _ _ _ _ _ _ w2216 w2350 w2417 w2647 w2695]
      tunnel: w319 -> [w523 _ w1389 w1707 _ _ _ _ _ _ _ _ w2217 w2348 w2416 w2651 w2691]
      tunnel: w318 -> [w522 _ w1387 w1689 _ _ _ _ _ _ _ _ w2184 w2349 w2415 w2646 w2693]
      tunnel: w317 -> [w521 _ w1388 w1706 _ _ _ _ _ _ _ _ w2185 w2347 w2414 w2650 w2689]
      tunnel: w316 -> [w520 _ w1385 w1692 _ _ _ _ _ _ _ _ w2196 w2346 w2413 w2645 w2687]
      tunnel: w315 -> [w519 _ w1386 w1705 _ _ _ _ _ _ _ _ w2197 w2344 w2412 w2649 w2685]
      tunnel: w314 -> [w518 _ w1383 w1695 _ _ _ _ _ _ _ _ w2172 w2345 w2411 w2644 w2699]
      tunnel: w313 -> [w517 _ w1384 w1704 _ _ _ _ _ _ _ _ w2173 w2343 w2410 w2648 w2697]
      tunnel: [w500 _ _ _ _ _ _ _ _ _ _ _ _ _ _ _ _] -> w295
      tunnel: [w498 _ _ _ _ _ _ _ _ _ _ _ _ _ _ _ _] -> w294
      tunnel: w293 -> [w503 _ _ _ _ _ _ _ _ _ _ _ _ _ _ _ _]
      tunnel: w292 -> [w502 _ _ _ _ _ _ _ _ _ _ _ _ _ _ _ _]
      tunnel: [w496 _ w1368 _ _ _ _ _ _ _ _ _ _ _ _ _ _] -> w286
      tunnel: [w495 _ w1367 _ _ _ _ _ _ _ _ _ _ _ _ _ _] -> w283
      tunnel: [w494 _ w1366 _ _ _ _ _ _ _ _ _ _ _ _ _ _] -> w285
      tunnel: [w493 _ w1365 _ _ _ _ _ _ _ _ _ _ _ _ _ _] -> w284
      tunnel: [w490 _ w1364 _ _ _ _ _ _ _ _ _ _ _ _ _ _] -> w282
      tunnel: [w489 _ w1363 _ _ _ _ _ _ _ _ _ _ _ _ _ _] -> w281
      tunnel: [w492 _ w1362 _ _ _ _ _ _ _ _ _ _ _ _ _ _] -> w279
      tunnel: [_ _ w1361 _ _ _ _ _ _ _ _ _ _ _ _ _ _] -> w280
      tunnel: [w491 _ _ _ _ _ _ _ _ _ _ _ _ _ _ _ _] -> _
      event Timeout {
        # "R"
        # "Y"
        # "Z"
        # "X"
        n203 = event-data() -> ()  [unwired: 1 in, 2 out]
        n204 = property on="X Position mm PV" class="DigNum (strict)"() -> ("Value"=w537:dbl)  [unwired: 2 in, 2 out]
        n205 = property on="Z Position mm PV" class="DigNum (strict)"() -> ("Value"=w506:dbl)  [unwired: 2 in, 2 out]
        n206 = property on="Y Position mm PV" class="DigNum (strict)"() -> ("Value"=w505:dbl)  [unwired: 2 in, 2 out]
        n207 = property on="R Position deg PV" class="DigNum (strict)"() -> ("Value"=w538:dbl)  [unwired: 2 in, 2 out]
        n208 = property on="GO" class="Bool"() -> ("DisabledEnum"=w513:T9)  [unwired: 2 in, 2 out]
        n209 = property on="Y Scan Length SP steps" class="DigNum (strict)"() -> ("Value"=w527:i32)  [unwired: 2 in, 2 out]
        n210 = property on="Z Scan Length SP steps" class="DigNum (strict)"() -> ("Value"=w528:i32)  [unwired: 2 in, 2 out]
        n211 = call "Build XY Graph2"("Reset"=TRUE, "Y Input"=w538, "X Input"=w506) -> ("XY Graph"=→"ZR Graph":cluster{"Y":dbl[], "Y":dbl[]}[])  [unwired: 7 in, 1 out]
        n212 = call "Build XY Graph"("Reset"=TRUE, "Y Input"=w505, "X Input"=w537) -> ("XY Graph"=→"XY Graph":cluster{"Y":dbl[], "Y":dbl[]}[])  [unwired: 7 in, 1 out]
        n213 = Build Array (concatenate)(w503, w506) -> (w501:dbl[])
        n214 = Build Array (concatenate)(w502, w505) -> (w499:dbl[])
        n215 = Equal?(x=w513, y=T9."Enabled") -> (x = y?=w511:bool)
        n216 = To Double Precision Float(number=w527) -> (double precision float=w526:dbl)
        n217 = To Double Precision Float(number=w528) -> (double precision float=w525:dbl)
        n218 = Bundle(w501, w499) -> (→"ZY Graph":cluster{dbl[], dbl[]})  [unwired: 1 in]
        n219 = property on="Clear ZY" class="Bool (strict)"() -> ("Value"=w497:bool)  [unwired: 2 in, 2 out]
        n220 = property on="Scan Go" class="Bool (strict)"() -> ("DisabledEnum"=w510:T9)  [unwired: 2 in, 2 out]
        n221 = property on="GO" class="Bool"() -> ("DisabledEnum"=w516:T9)  [unwired: 2 in, 2 out]
        n222 = Divide(x=w526, y=w525) -> (x/y=w529:dbl)
        n223 = Equal?(x=w510, y=T9."Disabled and Grayed Out") -> (x = y?=w507:bool)
        n224 = Equal?(x=w516, y=T9."Disabled and Grayed Out") -> (x = y?=w514:bool)
        n225 = Inverse Tangent(1:w529) -> (0:w530:dbl)
        n226 = case shown="True" w514 {
          tunnel: [w580 w706] -> w496
          tunnel: [w579 w705] -> w495
          tunnel: [w578 w704] -> w494
          tunnel: [w577 w703] -> w493
          tunnel: [w576 w702] -> w490
          tunnel: [w575 w701] -> w489
          tunnel: [w574 w700] -> w492
          tunnel: [w573 w699] -> w491
          tunnel: w524 -> [w566 w698]
          tunnel: w523 -> [w564 w697]
          tunnel: w522 -> [w553 w696]
          tunnel: w521 -> [w552 w695]
          tunnel: w520 -> [w557 w694]
          tunnel: w519 -> [w556 w693]
          tunnel: w518 -> [w562 w692]
          tunnel: w517 -> [w563 w691]
          frame False {
            n227 = flat-sequence {
              tunnel: [w621] -> w558
              tunnel: w557 -> [w620]
              tunnel: [w619] -> w559
              tunnel: w556 -> [w618]
              frame #0 {
                n228 = property on="Y Step SP" class="DigNum (strict)"() -> ("Maximum"=w635:dbl)  [unwired: 2 in, 2 out]
                n229 = property on="Y Step SP" class="DigNum (strict)"() -> ("Minimum"=w637:dbl)  [unwired: 2 in, 2 out]
                n230 = property on="Y steps/rev" class="DigNum (strict)"() -> ("Value"=w632:u32)  [unwired: 2 in, 2 out]
                n231 = property on="Y mm/rev" class="DigNum (strict)"() -> ("Value"=w630:dbl)  [unwired: 2 in, 2 out]
                n232 = To Long Integer(number=w635) -> (32bit integer=w634:i32)
                n233 = To Long Integer(number=w637) -> (32bit integer=w636:i32)
                n234 = To Double Precision Float(number=w632) -> (double precision float=w633:dbl)
                n235 = call "mdrive send command.vi"("error in (no error)"=w618, "Extra"="P", "Command"=T10."Print Parameter", "VISA resource name"=w620) -> ("error out"=w619:errorcluster, "read buffer"=w639:string, "VISA resource name out"=w621:refnum<visa-resource-name>)  [unwired: 3 in]
                n236 = Decimal String To Number(string=w639, offset=0) -> (number=w622:i32)  [unwired: 1 in, 1 out]
                n237 = In Range and Coerce(upper limit=w634, x=w622, lower limit=w636) -> (In Range?=w623:bool)  [unwired: 1 out]
                n238 = To Double Precision Float(number=w622) -> (double precision float=w627:dbl)
                n239 = Divide(x=w627, y=w633) -> (x/y=w631:dbl)
                n240 = property on="Y offset mm" class="DigNum (strict)"() -> ("Value"=w628:dbl)  [unwired: 2 in, 2 out]
                n241 = Multiply(x=w631, y=w630) -> (x*y=w629:dbl)
                n242 = Add(x=w629, y=w628) -> (x+y=w626:dbl)
                n243 = property on="Y Position mm PV" class="DigNum (strict)"("Val(Sgnl)"=w626) -> ()  [unwired: 2 in, 2 out]
                n244 = property on="Y in Range" class="Bool (strict)"("Val(Sgnl)"=w623) -> ()  [unwired: 2 in, 2 out]
                n245 = property on="Y Step PV" class="DigNum (strict)"("Val(Sgnl)"=w622) -> ()  [unwired: 2 in, 2 out]
              }
            }
            n246 = flat-sequence {
              tunnel: [w665] -> w551
              tunnel: w566 -> [w664]
              tunnel: [w663] -> w565
              tunnel: w564 -> [w662]
              frame #0 {
                n247 = property on="X Step SP" class="DigNum (strict)"() -> ("Maximum"=w679:dbl)  [unwired: 2 in, 2 out]
                n248 = property on="X Step SP" class="DigNum (strict)"() -> ("Minimum"=w681:dbl)  [unwired: 2 in, 2 out]
                n249 = property on="X steps/rev" class="DigNum (strict)"() -> ("Value"=w676:u32)  [unwired: 2 in, 2 out]
                n250 = To Long Integer(number=w679) -> (32bit integer=w678:i32)
                n251 = To Long Integer(number=w681) -> (32bit integer=w680:i32)
                n252 = To Double Precision Float(number=w676) -> (double precision float=w677:dbl)
                n253 = call "mdrive send command.vi"("error in (no error)"=w662, "Extra"="P", "Command"=T10."Print Parameter", "VISA resource name"=w664) -> ("error out"=w663:errorcluster, "read buffer"=w683:string, "VISA resource name out"=w665:refnum<visa-resource-name>)  [unwired: 3 in]
                n254 = Decimal String To Number(string=w683, offset=0) -> (number=w666:i32)  [unwired: 1 in, 1 out]
                n255 = property on="X Step PV" class="DigNum (strict)"("Val(Sgnl)"=w666) -> ()  [unwired: 2 in, 2 out]
                n256 = In Range and Coerce(upper limit=w678, x=w666, lower limit=w680) -> (In Range?=w667:bool)  [unwired: 1 out]
                n257 = To Double Precision Float(number=w666) -> (double precision float=w671:dbl)
                n258 = Divide(x=w671, y=w677) -> (x/y=w675:dbl)
                n259 = property on="X mm/rev" class="DigNum (strict)"() -> ("Value"=w674:dbl)  [unwired: 2 in, 2 out]
                n260 = property on="X offset mm" class="DigNum (strict)"() -> ("Value"=w672:dbl)  [unwired: 2 in, 2 out]
                n261 = Multiply(x=w675, y=w674) -> (x*y=w673:dbl)
                n262 = Add(x=w673, y=w672) -> (x+y=w670:dbl)
                n263 = property on="X Position mm PV" class="DigNum (strict)"("Val(Sgnl)"=w670) -> ()  [unwired: 2 in, 2 out]
                n264 = property on="X  in Range" class="Bool (strict)"("Val(Sgnl)"=w667) -> ()  [unwired: 2 in, 2 out]
              }
            }
            n265 = flat-sequence {
              tunnel: [w599] -> w555
              tunnel: [w598] -> w554
              tunnel: w553 -> [w597]
              tunnel: w552 -> [w596]
              frame #0 {
                n266 = property on="Z Step SP" class="DigNum (strict)"() -> ("Maximum"=w613:dbl)  [unwired: 2 in, 2 out]
                n267 = property on="Z Step SP" class="DigNum (strict)"() -> ("Minimum"=w615:dbl)  [unwired: 2 in, 2 out]
                n268 = property on="Z steps/rev" class="DigNum (strict)"() -> ("Value"=w610:u32)  [unwired: 2 in, 2 out]
                n269 = To Long Integer(number=w613) -> (32bit integer=w612:i32)
                n270 = To Long Integer(number=w615) -> (32bit integer=w614:i32)
                n271 = To Double Precision Float(number=w610) -> (double precision float=w611:dbl)
                n272 = call "mdrive send command.vi"("error in (no error)"=w596, "Extra"="P", "Command"=T10."Print Parameter", "VISA resource name"=w597) -> ("error out"=w598:errorcluster, "read buffer"=w617:string, "VISA resource name out"=w599:refnum<visa-resource-name>)  [unwired: 3 in]
                n273 = Decimal String To Number(string=w617, offset=0) -> (number=w600:i32)  [unwired: 1 in, 1 out]
                n274 = property on="Z Step PV" class="DigNum (strict)"("Val(Sgnl)"=w600) -> ()  [unwired: 2 in, 2 out]
                n275 = In Range and Coerce(upper limit=w612, x=w600, lower limit=w614) -> (In Range?=w601:bool)  [unwired: 1 out]
                n276 = To Double Precision Float(number=w600) -> (double precision float=w605:dbl)
                n277 = Divide(x=w605, y=w611) -> (x/y=w609:dbl)
                n278 = property on="Z mm/rev" class="DigNum (strict)"() -> ("Value"=w608:dbl)  [unwired: 2 in, 2 out]
                n279 = property on="Z offset mm" class="DigNum (strict)"() -> ("Value"=w606:dbl)  [unwired: 2 in, 2 out]
                n280 = Multiply(x=w609, y=w608) -> (x*y=w607:dbl)
                n281 = Add(x=w607, y=w606) -> (x+y=w604:dbl)
                n282 = property on="Z Position mm PV" class="DigNum (strict)"("Val(Sgnl)"=w604) -> ()  [unwired: 2 in, 2 out]
                n283 = property on="Z in Range" class="Bool (strict)"("Val(Sgnl)"=w601) -> ()  [unwired: 2 in, 2 out]
              }
            }
            n284 = flat-sequence {
              tunnel: [w643] -> w560
              tunnel: w562 -> [w642]
              tunnel: [w641] -> w561
              tunnel: w563 -> [w640]
              frame #0 {
                n285 = property on="R Step SP" class="DigNum (strict)"() -> ("Maximum"=w657:dbl)  [unwired: 2 in, 2 out]
                n286 = property on="R Step SP" class="DigNum (strict)"() -> ("Minimum"=w659:dbl)  [unwired: 2 in, 2 out]
                n287 = property on="R steps/rev" class="DigNum (strict)"() -> ("Value"=w654:u32)  [unwired: 2 in, 2 out]
                n288 = property on="R deg/rev" class="DigNum (strict)"() -> ("Value"=w652:dbl)  [unwired: 2 in, 2 out]
                n289 = To Long Integer(number=w657) -> (32bit integer=w656:i32)
                n290 = To Long Integer(number=w659) -> (32bit integer=w658:i32)
                n291 = To Double Precision Float(number=w654) -> (double precision float=w655:dbl)
                n292 = call "mdrive send command.vi"("error in (no error)"=w640, "Extra"="P", "Command"=T10."Print Parameter", "VISA resource name"=w642) -> ("error out"=w641:errorcluster, "read buffer"=w661:string, "VISA resource name out"=w643:refnum<visa-resource-name>)  [unwired: 3 in]
                n293 = Decimal String To Number(string=w661, offset=0) -> (number=w644:i32)  [unwired: 1 in, 1 out]
                n294 = In Range and Coerce(upper limit=w656, x=w644, lower limit=w658) -> (In Range?=w645:bool)  [unwired: 1 out]
                n295 = To Double Precision Float(number=w644) -> (double precision float=w649:dbl)
                n296 = Divide(x=w649, y=w655) -> (x/y=w653:dbl)
                n297 = property on="R offset deg" class="DigNum (strict)"() -> ("Value"=w650:dbl)  [unwired: 2 in, 2 out]
                n298 = Multiply(x=w653, y=w652) -> (x*y=w651:dbl)
                n299 = Add(x=w651, y=w650) -> (x+y=w648:dbl)
                n300 = property on="R Position deg PV" class="DigNum (strict)"("Val(Sgnl)"=w648) -> ()  [unwired: 2 in, 2 out]
                n301 = property on="R in Range" class="Bool (strict)"("Val(Sgnl)"=w645) -> ()  [unwired: 2 in, 2 out]
                n302 = property on="R Step PV" class="DigNum (strict)"("Val(Sgnl)"=w644) -> ()  [unwired: 2 in, 2 out]
              }
            }
            n303 = call "mdrive send command.vi"("error in (no error)"=w561, "Extra"="MV", "Command"=T10."Print Parameter", "VISA resource name"=w560) -> ("error out"=w573:errorcluster, "read buffer"=w582:string, "VISA resource name out"=w574:refnum<visa-resource-name>)  [unwired: 3 in]
            n304 = call "mdrive send command.vi"("error in (no error)"=w559, "Extra"="MV", "Command"=T10."Print Parameter", "VISA resource name"=w558) -> ("error out"=w575:errorcluster, "read buffer"=w586:string, "VISA resource name out"=w576:refnum<visa-resource-name>)  [unwired: 3 in]
            n305 = Not Equal?(x=w582, y="") -> (x != y?=w569:bool)
            n306 = Not Equal?(x=w586, y="") -> (x != y?=w570:bool)
            n307 = property on="R Ready" class="Bool (strict)"("Val(Sgnl)"=w569) -> ()  [unwired: 2 in, 2 out]
            n308 = property on="Y Ready" class="Bool (strict)"("Val(Sgnl)"=w570) -> ()  [unwired: 2 in, 2 out]
            n309 = call "mdrive send command.vi"("error in (no error)"=w554, "Extra"="MV", "Command"=T10."Print Parameter", "VISA resource name"=w555) -> ("error out"=w577:errorcluster, "read buffer"=w590:string, "VISA resource name out"=w578:refnum<visa-resource-name>)  [unwired: 3 in]
            n310 = call "DigitalIO_sub_V5_MON.vi"() -> ("CL"=w567:bool, "OP"=w568:bool)  [unwired: 8 in]
            n311 = Not Equal?(x=w590, y="") -> (x != y?=w571:bool)
            n312 = property on="Z Ready" class="Bool (strict)"("Val(Sgnl)"=w571) -> ()  [unwired: 2 in, 2 out]
            n313 = property on="OP" class="Bool (strict)"("Val(Sgnl)"=w568) -> ()  [unwired: 2 in, 2 out]
            n314 = property on="CL" class="Bool (strict)"("Val(Sgnl)"=w567) -> ()  [unwired: 2 in, 2 out]
            n315 = call "mdrive send command.vi"("error in (no error)"=w565, "Extra"="MV", "Command"=T10."Print Parameter", "VISA resource name"=w551) -> ("error out"=w579:errorcluster, "read buffer"=w594:string, "VISA resource name out"=w580:refnum<visa-resource-name>)  [unwired: 3 in]
            n316 = Not Equal?(x=w594, y="") -> (x != y?=w572:bool)
            n317 = property on="X Ready" class="Bool (strict)"("Val(Sgnl)"=w572) -> ()  [unwired: 2 in, 2 out]
          }
          frame True {
            n318 = flat-sequence {
              tunnel: [w1216] -> w762
              tunnel: [w1215] -> w761
              tunnel: [w1214] -> w760
              tunnel: w698 -> [w1213]
              tunnel: w697 -> [w1212]
              tunnel: [w1238] -> w759
              tunnel: [w1237] -> w758
              tunnel: [w1235] -> w757
              tunnel: [w1236] -> w756
              tunnel: w762 -> [w1235]
              tunnel: w761 -> [w1234]
              tunnel: w760 -> [w1233]
              tunnel: w759 -> [w1252]
              tunnel: [w1252] -> w755
              tunnel: w758 -> [w1251]
              tunnel: [w1251] -> w754
              tunnel: w757 -> [w1250]
              tunnel: [w1250] -> w753
              tunnel: w756 -> [w1249]
              tunnel: [w1249] -> w752
              tunnel: [w1256] -> w751
              tunnel: [w1257] -> w750
              tunnel: [w1253] -> w749
              tunnel: w752 -> [w1253]
              tunnel: w753 -> [w1254]
              tunnel: w754 -> [w1258]
              tunnel: w755 -> [w1255]
              tunnel: w751 -> [w1268]
              tunnel: w750 -> [w1269]
              tunnel: w749 -> [w1271]
              tunnel: [w1267] -> w705
              tunnel: [w1266] -> w706
              frame #0 {
                n319 = property on="X Step SP" class="DigNum (strict)"() -> ("Maximum"=w1228:dbl)  [unwired: 2 in, 2 out]
                n320 = property on="X Step SP" class="DigNum (strict)"() -> ("Minimum"=w1230:dbl)  [unwired: 2 in, 2 out]
                n321 = property on="X steps/rev" class="DigNum (strict)"() -> ("Value"=w1225:u32)  [unwired: 2 in, 2 out]
                n322 = property on="X offset mm" class="DigNum (strict)"() -> ("Value"=w1221:dbl)  [unwired: 2 in, 2 out]
                n323 = To Long Integer(number=w1228) -> (32bit integer=w1227:i32)
                n324 = To Long Integer(number=w1230) -> (32bit integer=w1229:i32)
                n325 = To Double Precision Float(number=w1225) -> (double precision float=w1226:dbl)
                n326 = call "mdrive send command.vi"("error in (no error)"=w1212, "Extra"="P", "Command"=T10."Print Parameter", "VISA resource name"=w1213) -> ("error out"=w1214:errorcluster, "read buffer"=w1232:string, "VISA resource name out"=w1215:refnum<visa-resource-name>)  [unwired: 3 in]
                n327 = Decimal String To Number(string=w1232, offset=0) -> (number=w1211:i32)  [unwired: 1 in, 1 out]
                n328 = property on="X Step PV" class="DigNum (strict)"("Val(Sgnl)"=w1211) -> ()  [unwired: 2 in, 2 out]
                n329 = In Range and Coerce(upper limit=w1227, x=w1211, lower limit=w1229) -> (In Range?=w1216:bool)  [unwired: 1 out]
                n330 = To Double Precision Float(number=w1211) -> (double precision float=w1220:dbl)
                n331 = property on="X  in Range" class="Bool (strict)"("Val(Sgnl)"=w1216) -> ()  [unwired: 2 in, 2 out]
                n332 = Divide(x=w1220, y=w1226) -> (x/y=w1224:dbl)
                n333 = property on="X mm/rev" class="DigNum (strict)"() -> ("Value"=w1223:dbl)  [unwired: 2 in, 2 out]
                n334 = Multiply(x=w1224, y=w1223) -> (x*y=w1222:dbl)
                n335 = Add(x=w1222, y=w1221) -> (x+y=w1219:dbl)
                n336 = property on="X Position mm PV" class="DigNum (strict)"("Val(Sgnl)"=w1219) -> ()  [unwired: 2 in, 2 out]
              }
              frame #1 {
                n337 = call "mdrive send command.vi"("error in (no error)"=w1233, "Extra"="MV", "Command"=T10."Print Parameter", "VISA resource name"=w1234) -> ("error out"=w1237:errorcluster, "read buffer"=w1241:string, "VISA resource name out"=w1238:refnum<visa-resource-name>)  [unwired: 3 in]
                n338 = Decimal String To Number(string=w1241, offset=0 ("offset (0)")) -> (number=w1244:i32)  [unwired: 1 in, 1 out]
                n339 = Not Equal?(x=w1241, y="") -> (x != y?=w1239:bool)
                n340 = property on="X Ready" class="Bool (strict)"("Val(Sgnl)"=w1239) -> ()  [unwired: 2 in, 2 out]
                n341 = Number To Boolean Array(number=w1244) -> (Boolean array=w1243:bool[])
                n342 = Index Array(array=w1243, index=0) -> (element=w1236:bool)
                n343 = property on="X  in Motion" class="Bool (strict)"("Val(Sgnl)"=w1236) -> ()  [unwired: 2 in, 2 out]
              }
              frame #2 {
                n344 = Wait (ms)(milliseconds to wait=u32 50) -> ()  [unwired: 1 out]
              }
              frame #3 {
                n345 = case shown="True" w1254 {
                  tunnel: w1255 -> [w1261 w1265]
                  tunnel: [w1262 w1265] -> w1256
                  tunnel: [w1263 w1264] -> w1257
                  tunnel: w1258 -> [w1260 w1264]
                  frame False {
                    n346 = call "mdrive send command.vi"("error in (no error)"=w1260, "Command"=T10."Stop", "VISA resource name"=w1261) -> ("error out"=w1263:errorcluster, "VISA resource name out"=w1262:refnum<visa-resource-name>)  [unwired: 4 in, 1 out]
                  }
                  frame True {
                  }
                }
              }
              frame #4 {
                n347 = property on="X Backlash corr" class="Bool (strict)"() -> ("Value"=w1272:bool)  [unwired: 2 in, 2 out]
                n348 = Implies(1:w1271, 2:w1272) -> (0:w1270:bool)
                n349 = case shown="False" w1270 {
                  tunnel: w1269 -> [w1280 w1337]
                  tunnel: w1268 -> [w1279 w1338]
                  tunnel: [w1274 w1337] -> w1267
                  tunnel: [w1278 w1338] -> w1266
                  frame False {
                    # "Backlash"
                    n350 = flat-sequence {
                      tunnel: [w1295] -> w1292
                      tunnel: [w1297] -> w1291
                      tunnel: [w1296] -> w1290
                      tunnel: w1280 -> [w1294]
                      tunnel: w1279 -> [w1293]
                      tunnel: w1292 -> [w1305]
                      tunnel: [w1305] -> w1289
                      tunnel: w1291 -> [w1304]
                      tunnel: w1290 -> [w1303]
                      tunnel: [w1302] -> w1288
                      tunnel: [w1301] -> w1287
                      tunnel: [w1300] -> w1277
                      tunnel: w1289 -> [w1319]
                      tunnel: w1288 -> [w1310]
                      tunnel: w1287 -> [w1318]
                      tunnel: [w1310] -> w1286
                      tunnel: [w1318] -> w1285
                      tunnel: [w1309] -> w1282
                      tunnel: [w1317] -> w1281
                      tunnel: w1277 -> [w1317]
                      tunnel: w1286 -> [w1322]
                      tunnel: w1285 -> [w1323]
                      tunnel: [w1321] -> w1284
                      tunnel: [w1329] -> w1283
                      tunnel: w1282 -> [w1329]
                      tunnel: w1281 -> [w1325]
                      tunnel: [w1324] -> w1275
                      tunnel: w1284 -> [w1332]
                      tunnel: w1283 -> [w1331]
                      tunnel: [w1333] -> w1276
                      tunnel: w1275 -> [w1333]
                      tunnel: [w1332] -> w1273
                      tunnel: [w1336] -> w1278
                      tunnel: w1276 -> [w1336]
                      tunnel: [w1334] -> w1274
                      tunnel: w1273 -> [w1334]
                      frame #0 {
                        n351 = property on="X Backlash steps/sec" class="DigNum (strict)"() -> ("Value"=w1295:i32)  [unwired: 2 in, 2 out]
                        n352 = Number To Decimal String(number=w1295) -> (decimal integer string=w1298:string)  [unwired: 1 in]
                        n353 = call "mdrive send command.vi"("error in (no error)"=w1294, "Extra"=w1298, "Command"=T10."Max Velocity", "VISA resource name"=w1293) -> ("error out"=w1296:errorcluster, "VISA resource name out"=w1297:refnum<visa-resource-name>)  [unwired: 3 in, 1 out]
                      }
                      frame #1 {
                        n354 = property on="X Backlash" class="DigNum (strict)"() -> ("Value"=w1300:i32)  [unwired: 2 in, 2 out]
                        n355 = Number To Decimal String(number=w1300) -> (decimal integer string=w1306:string)  [unwired: 1 in]
                        n356 = call "mdrive send command.vi"("error in (no error)"=w1303, "Extra"=w1306, "Command"=T10."Move to Relative Position", "VISA resource name"=w1304) -> ("error out"=w1302:errorcluster, "VISA resource name out"=w1301:refnum<visa-resource-name>)  [unwired: 3 in, 1 out]
                      }
                      frame #2 {
                        n357 = To Double Precision Float(number=w1317) -> (double precision float=w1315:dbl)
                        n358 = To Double Precision Float(number=w1319) -> (double precision float=w1320:dbl)
                        n359 = Absolute Value(x=w1315) -> (abs(x)=w1316:dbl)
                        n360 = Divide(x=w1316, y=w1320) -> (x/y=w1313:dbl)
                        n361 = Multiply(x=1000.0, y=w1313) -> (x*y=w1311:dbl)
                        n362 = Add(x=w1311, y=300.0) -> (x+y=w1309:dbl)
                        n363 = To Unsigned Long Integer(number=w1309) -> (unsigned 32bit integer=w1308:u32)
                        n364 = Wait (ms)(milliseconds to wait=w1308) -> ()  [unwired: 1 out]
                      }
                      frame #3 {
                        n365 = Negate(x=w1325) -> (-x=w1326:i32)
                        n366 = Number To Decimal String(number=w1326) -> (decimal integer string=w1327:string)  [unwired: 1 in]
                        n367 = call "mdrive send command.vi"("error in (no error)"=w1322, "Extra"=w1327, "Command"=T10."Move to Relative Position", "VISA resource name"=w1323) -> ("error out"=w1321:errorcluster, "VISA resource name out"=w1324:refnum<visa-resource-name>)  [unwired: 3 in, 1 out]
                      }
                      frame #4 {
                        n368 = To Unsigned Long Integer(number=w1331) -> (unsigned 32bit integer=w1330:u32)
                        n369 = Wait (ms)(milliseconds to wait=w1330) -> ()  [unwired: 1 out]
                      }
                      frame #5 {
                        n370 = property on="X Backlash corr" class="Bool (strict)"("Val(Sgnl)"=FALSE ("Value (Signaling)")) -> ()  [unwired: 2 in, 2 out]
                      }
                    }
                  }
                  frame True {
                  }
                }
              }
            }
            n371 = flat-sequence {
              tunnel: [w1085] -> w748
              tunnel: [w1076] -> w747
              tunnel: [w1075] -> w746
              tunnel: w696 -> [w1079]
              tunnel: w695 -> [w1078]
              tunnel: [w1114] -> w745
              tunnel: [w1113] -> w744
              tunnel: [w1112] -> w743
              tunnel: [w1105] -> w742
              tunnel: w748 -> [w1112]
              tunnel: w747 -> [w1111]
              tunnel: w746 -> [w1110]
              tunnel: w745 -> [w1124]
              tunnel: [w1124] -> w741
              tunnel: w744 -> [w1123]
              tunnel: [w1123] -> w740
              tunnel: w743 -> [w1122]
              tunnel: [w1122] -> w739
              tunnel: w742 -> [w1121]
              tunnel: [w1121] -> w738
              tunnel: [w1128] -> w737
              tunnel: [w1129] -> w736
              tunnel: [w1125] -> w735
              tunnel: w738 -> [w1125]
              tunnel: w739 -> [w1126]
              tunnel: w740 -> [w1130]
              tunnel: w741 -> [w1127]
              tunnel: w737 -> [w1141]
              tunnel: w736 -> [w1142]
              tunnel: w735 -> [w1144]
              tunnel: [w1140] -> w703
              tunnel: [w1139] -> w704
              frame #0 {
                n372 = property on="Z Step SP" class="DigNum (strict)"() -> ("Maximum"=w1086:dbl)  [unwired: 2 in, 2 out]
                n373 = property on="Z Step SP" class="DigNum (strict)"() -> ("Minimum"=w1080:dbl)  [unwired: 2 in, 2 out]
                n374 = property on="OK Button" class="Bool (strict)"() -> ("Value"=w1071:bool)  [unwired: 2 in, 2 out]
                n375 = property on="Z steps/rev" class="DigNum (strict)"() -> ("Value"=w1084:u32)  [unwired: 2 in, 2 out]
                n376 = To Double Precision Float(number=w1084) -> (double precision float=w1091:dbl)
                n377 = To Long Integer(number=w1086) -> (32bit integer=w1092:i32)
                n378 = To Long Integer(number=w1080) -> (32bit integer=w1093:i32)
                n379 = property on="Z offset mm" class="DigNum (strict)"() -> ("Value"=w1082:dbl)  [unwired: 2 in, 2 out]
                n380 = Not Equal?(x=w1071, y=TRUE) -> (x != y?=w1069:bool)
                n381 = call "mdrive send command.vi"("error in (no error)"=w1078, "Extra"="P", "Command"=T10."Print Parameter", "VISA resource name"=w1079) -> ("error out"=w1075:errorcluster, "read buffer"=w1095:string, "VISA resource name out"=w1076:refnum<visa-resource-name>)  [unwired: 3 in]
                n382 = Decimal String To Number(string=w1095, offset=0) -> (number=w1074:i32)  [unwired: 1 in, 1 out]
                n383 = property on="Z Step PV" class="DigNum (strict)"("Val(Sgnl)"=w1074) -> ()  [unwired: 2 in, 2 out]
                n384 = Equal?(x=w1074, y=15360000) -> (x = y?=w1068:bool)
                n385 = To Double Precision Float(number=w1074) -> (double precision float=w1089:dbl)
                n386 = In Range and Coerce(upper limit=w1092, x=w1074, lower limit=w1093) -> (In Range?=w1085:bool)  [unwired: 1 out]
                n387 = property on="Z in Range" class="Bool (strict)"("Val(Sgnl)"=w1085) -> ()  [unwired: 2 in, 2 out]
                n388 = Divide(x=w1089, y=w1091) -> (x/y=w1090:dbl)
                n389 = And(x=w1068, y=w1069) -> (x .and. y?=w1067:bool)
                n390 = case shown="True" w1067 {
                  tunnel: [FALSE ("true") w1103] -> w1072
                  frame False {
                  }
                  frame True {
                    n391 = One Button Dialog(message="HAVE YOU OPEND THE VALVE???\nTHEN REWRITE YOUR POSITION\n AND PRESS GO!") -> (true=w1103:bool)  [unwired: 1 in]
                  }
                }
                n392 = property on="Z mm/rev" class="DigNum (strict)"() -> ("Value"=w1083:dbl)  [unwired: 2 in, 2 out]
                n393 = Multiply(x=w1090, y=w1083) -> (x*y=w1077:dbl)
                n394 = Add(x=w1077, y=w1082) -> (x+y=w1081:dbl)
                n395 = property on="Z Position mm PV" class="DigNum (strict)"("Val(Sgnl)"=w1081) -> ()  [unwired: 2 in, 2 out]
                n396 = case shown="True" w1072 {
                  frame False {
                    n397 = call "DigitalIO_sub_V5_MON.vi"() -> ("CL"=w1096:bool, "OP"=w1097:bool)  [unwired: 8 in]
                    n398 = property on="OP" class="Bool (strict)"("Val(Sgnl)"=w1097) -> ()  [unwired: 2 in, 2 out]
                    n399 = property on="CL" class="Bool (strict)"("Val(Sgnl)"=w1096) -> ()  [unwired: 2 in, 2 out]
                  }
                  frame True {
                    n400 = while {
                      stop <- w1101 stop-if-true
                      n401 = call "DigitalIO_sub_V5_MON.vi"() -> ("CL"=w1098:bool, "OP"=w1099:bool)  [unwired: 8 in]
                      n402 = property on="OP" class="Bool (strict)"("Val(Sgnl)"=w1099) -> ()  [unwired: 2 in, 2 out]
                      n403 = property on="CL" class="Bool (strict)"("Val(Sgnl)"=w1098) -> ()  [unwired: 2 in, 2 out]
                      n404 = property on="V5 Valve \nopend/closed" class="Bool (strict)"("Val(Sgnl)"=w1098) -> ()  [unwired: 2 in, 2 out]
                      n405 = Equal?(x=w1098, y=TRUE) -> (x = y?=w1101:bool)
                    }
                  }
                }
              }
              frame #1 {
                n406 = call "mdrive send command.vi"("error in (no error)"=w1110, "Extra"="MV", "Command"=T10."Print Parameter", "VISA resource name"=w1111) -> ("error out"=w1113:errorcluster, "read buffer"=w1116:string, "VISA resource name out"=w1114:refnum<visa-resource-name>)  [unwired: 3 in]
                n407 = Decimal String To Number(string=w1116, offset=0 ("offset (0)")) -> (number=w1106:i32)  [unwired: 1 in, 1 out]
                n408 = Not Equal?(x=w1116, y="") -> (x != y?=w1109:bool)
                n409 = property on="Z Ready" class="Bool (strict)"("Val(Sgnl)"=w1109) -> ()  [unwired: 2 in, 2 out]
                n410 = Number To Boolean Array(number=w1106) -> (Boolean array=w1108:bool[])
                n411 = Index Array(array=w1108, index=0) -> (element=w1105:bool)
                n412 = property on="Z in Motion" class="Bool (strict)"("Val(Sgnl)"=w1105) -> ()  [unwired: 2 in, 2 out]
              }
              frame #2 {
                n413 = Wait (ms)(milliseconds to wait=u32 50) -> ()  [unwired: 1 out]
              }
              frame #3 {
                n414 = case shown="False" w1126 {
                  tunnel: w1127 -> [w1133 w1137]
                  tunnel: [w1134 w1137] -> w1128
                  tunnel: [w1135 w1136] -> w1129
                  tunnel: w1130 -> [w1132 w1136]
                  frame False {
                    n415 = call "mdrive send command.vi"("error in (no error)"=w1132, "Command"=T10."Stop", "VISA resource name"=w1133) -> ("error out"=w1135:errorcluster, "VISA resource name out"=w1134:refnum<visa-resource-name>)  [unwired: 4 in, 1 out]
                  }
                  frame True {
                  }
                }
              }
              frame #4 {
                n416 = property on="Z Backlash corr" class="Bool (strict)"() -> ("Value"=w1138:bool)  [unwired: 2 in, 2 out]
                n417 = Implies(1:w1144, 2:w1138) -> (0:w1143:bool)
                n418 = case shown="False" w1143 {
                  tunnel: w1142 -> [w1152 w1209]
                  tunnel: w1141 -> [w1151 w1210]
                  tunnel: [w1146 w1209] -> w1140
                  tunnel: [w1150 w1210] -> w1139
                  frame False {
                    # "Backlash"
                    n419 = flat-sequence {
                      tunnel: [w1165] -> w1164
                      tunnel: [w1169] -> w1163
                      tunnel: [w1168] -> w1162
                      tunnel: w1152 -> [w1167]
                      tunnel: w1151 -> [w1166]
                      tunnel: w1164 -> [w1177]
                      tunnel: [w1177] -> w1161
                      tunnel: w1163 -> [w1176]
                      tunnel: w1162 -> [w1175]
                      tunnel: [w1174] -> w1160
                      tunnel: [w1173] -> w1159
                      tunnel: [w1172] -> w1149
                      tunnel: w1161 -> [w1191]
                      tunnel: w1160 -> [w1182]
                      tunnel: w1159 -> [w1190]
                      tunnel: [w1182] -> w1158
                      tunnel: [w1190] -> w1157
                      tunnel: [w1181] -> w1154
                      tunnel: [w1189] -> w1153
                      tunnel: w1149 -> [w1189]
                      tunnel: w1158 -> [w1194]
                      tunnel: w1157 -> [w1195]
                      tunnel: [w1193] -> w1156
                      tunnel: [w1201] -> w1155
                      tunnel: w1154 -> [w1201]
                      tunnel: w1153 -> [w1197]
                      tunnel: [w1196] -> w1147
                      tunnel: w1156 -> [w1204]
                      tunnel: w1155 -> [w1203]
                      tunnel: [w1205] -> w1148
                      tunnel: w1147 -> [w1205]
                      tunnel: [w1204] -> w1145
                      tunnel: [w1208] -> w1150
                      tunnel: w1148 -> [w1208]
                      tunnel: [w1207] -> w1146
                      tunnel: w1145 -> [w1207]
                      frame #0 {
                        n420 = property on="Z Backlash steps/sec" class="DigNum (strict)"() -> ("Value"=w1165:i32)  [unwired: 2 in, 2 out]
                        n421 = Number To Decimal String(number=w1165) -> (decimal integer string=w1170:string)  [unwired: 1 in]
                        n422 = call "mdrive send command.vi"("error in (no error)"=w1167, "Extra"=w1170, "Command"=T10."Max Velocity", "VISA resource name"=w1166) -> ("error out"=w1168:errorcluster, "VISA resource name out"=w1169:refnum<visa-resource-name>)  [unwired: 3 in, 1 out]
                      }
                      frame #1 {
                        n423 = property on="Z Backlash" class="DigNum (strict)"() -> ("Value"=w1172:i32)  [unwired: 2 in, 2 out]
                        n424 = Number To Decimal String(number=w1172) -> (decimal integer string=w1178:string)  [unwired: 1 in]
                        n425 = call "mdrive send command.vi"("error in (no error)"=w1175, "Extra"=w1178, "Command"=T10."Move to Relative Position", "VISA resource name"=w1176) -> ("error out"=w1174:errorcluster, "VISA resource name out"=w1173:refnum<visa-resource-name>)  [unwired: 3 in, 1 out]
                      }
                      frame #2 {
                        n426 = To Double Precision Float(number=w1189) -> (double precision float=w1187:dbl)
                        n427 = To Double Precision Float(number=w1191) -> (double precision float=w1192:dbl)
                        n428 = Absolute Value(x=w1187) -> (abs(x)=w1188:dbl)
                        n429 = Divide(x=w1188, y=w1192) -> (x/y=w1185:dbl)
                        n430 = Multiply(x=1000.0, y=w1185) -> (x*y=w1183:dbl)
                        n431 = Add(x=w1183, y=300.0) -> (x+y=w1181:dbl)
                        n432 = To Unsigned Long Integer(number=w1181) -> (unsigned 32bit integer=w1180:u32)
                        n433 = Wait (ms)(milliseconds to wait=w1180) -> ()  [unwired: 1 out]
                      }
                      frame #3 {
                        n434 = Negate(x=w1197) -> (-x=w1198:i32)
                        n435 = Number To Decimal String(number=w1198) -> (decimal integer string=w1199:string)  [unwired: 1 in]
                        n436 = call "mdrive send command.vi"("error in (no error)"=w1194, "Extra"=w1199, "Command"=T10."Move to Relative Position", "VISA resource name"=w1195) -> ("error out"=w1193:errorcluster, "VISA resource name out"=w1196:refnum<visa-resource-name>)  [unwired: 3 in, 1 out]
                      }
                      frame #4 {
                        n437 = To Unsigned Long Integer(number=w1203) -> (unsigned 32bit integer=w1202:u32)
                        n438 = Wait (ms)(milliseconds to wait=w1202) -> ()  [unwired: 1 out]
                      }
                      frame #5 {
                        n439 = property on="Z Backlash corr" class="Bool (strict)"("Val(Sgnl)"=FALSE ("Value (Signaling)")) -> ()  [unwired: 2 in, 2 out]
                      }
                    }
                  }
                  frame True {
                  }
                }
              }
            }
            n440 = flat-sequence {
              tunnel: [w948] -> w734
              tunnel: [w950] -> w733
              tunnel: [w949] -> w732
              tunnel: w694 -> [w941]
              tunnel: w693 -> [w940]
              tunnel: [w970] -> w731
              tunnel: [w969] -> w730
              tunnel: [w968] -> w729
              tunnel: [w961] -> w728
              tunnel: w734 -> [w968]
              tunnel: w733 -> [w967]
              tunnel: w732 -> [w966]
              tunnel: w731 -> [w980]
              tunnel: [w980] -> w727
              tunnel: w730 -> [w979]
              tunnel: [w979] -> w726
              tunnel: w729 -> [w978]
              tunnel: [w978] -> w725
              tunnel: w728 -> [w977]
              tunnel: [w977] -> w724
              tunnel: [w984] -> w723
              tunnel: [w985] -> w722
              tunnel: [w981] -> w721
              tunnel: w724 -> [w981]
              tunnel: w725 -> [w982]
              tunnel: w726 -> [w986]
              tunnel: w727 -> [w983]
              tunnel: w723 -> [w997]
              tunnel: w722 -> [w998]
              tunnel: w721 -> [w1000]
              tunnel: [w996] -> w701
              tunnel: [w995] -> w702
              frame #0 {
                n441 = property on="Y Step SP" class="DigNum (strict)"() -> ("Maximum"=w943:dbl)  [unwired: 2 in, 2 out]
                n442 = property on="Y Step SP" class="DigNum (strict)"() -> ("Minimum"=w942:dbl)  [unwired: 2 in, 2 out]
                n443 = property on="Y steps/rev" class="DigNum (strict)"() -> ("Value"=w944:u32)  [unwired: 2 in, 2 out]
                n444 = property on="Y offset mm" class="DigNum (strict)"() -> ("Value"=w946:dbl)  [unwired: 2 in, 2 out]
                n445 = To Long Integer(number=w943) -> (32bit integer=w957:i32)
                n446 = To Long Integer(number=w942) -> (32bit integer=w958:i32)
                n447 = To Double Precision Float(number=w944) -> (double precision float=w956:dbl)
                n448 = call "mdrive send command.vi"("error in (no error)"=w940, "Extra"="P", "Command"=T10."Print Parameter", "VISA resource name"=w941) -> ("error out"=w949:errorcluster, "read buffer"=w960:string, "VISA resource name out"=w950:refnum<visa-resource-name>)  [unwired: 3 in]
                n449 = Decimal String To Number(string=w960, offset=0) -> (number=w939:i32)  [unwired: 1 in, 1 out]
                n450 = property on="Y Step PV" class="DigNum (strict)"("Val(Sgnl)"=w939) -> ()  [unwired: 2 in, 2 out]
                n451 = In Range and Coerce(upper limit=w957, x=w939, lower limit=w958) -> (In Range?=w948:bool)  [unwired: 1 out]
                n452 = To Double Precision Float(number=w939) -> (double precision float=w953:dbl)
                n453 = property on="Y in Range" class="Bool (strict)"("Val(Sgnl)"=w948) -> ()  [unwired: 2 in, 2 out]
                n454 = Divide(x=w953, y=w956) -> (x/y=w955:dbl)
                n455 = property on="Y mm/rev" class="DigNum (strict)"() -> ("Value"=w945:dbl)  [unwired: 2 in, 2 out]
                n456 = Multiply(x=w955, y=w945) -> (x*y=w954:dbl)
                n457 = Add(x=w954, y=w946) -> (x+y=w947:dbl)
                n458 = property on="Y Position mm PV" class="DigNum (strict)"("Val(Sgnl)"=w947) -> ()  [unwired: 2 in, 2 out]
              }
              frame #1 {
                n459 = call "mdrive send command.vi"("error in (no error)"=w966, "Extra"="MV", "Command"=T10."Print Parameter", "VISA resource name"=w967) -> ("error out"=w969:errorcluster, "read buffer"=w972:string, "VISA resource name out"=w970:refnum<visa-resource-name>)  [unwired: 3 in]
                n460 = Decimal String To Number(string=w972, offset=0 ("offset (0)")) -> (number=w962:i32)  [unwired: 1 in, 1 out]
                n461 = Not Equal?(x=w972, y="") -> (x != y?=w965:bool)
                n462 = property on="Y Ready" class="Bool (strict)"("Val(Sgnl)"=w965) -> ()  [unwired: 2 in, 2 out]
                n463 = Number To Boolean Array(number=w962) -> (Boolean array=w964:bool[])
                n464 = Index Array(array=w964, index=0) -> (element=w961:bool)
                n465 = property on="Y in Motion" class="Bool (strict)"("Val(Sgnl)"=w961) -> ()  [unwired: 2 in, 2 out]
              }
              frame #2 {
                n466 = Wait (ms)(milliseconds to wait=u32 50) -> ()  [unwired: 1 out]
              }
              frame #3 {
                n467 = case shown="True" w982 {
                  tunnel: w983 -> [w989 w992]
                  tunnel: [w990 w992] -> w984
                  tunnel: [w991 w993] -> w985
                  tunnel: w986 -> [w988 w993]
                  frame False {
                    n468 = call "mdrive send command.vi"("error in (no error)"=w988, "Command"=T10."Stop", "VISA resource name"=w989) -> ("error out"=w991:errorcluster, "VISA resource name out"=w990:refnum<visa-resource-name>)  [unwired: 4 in, 1 out]
                  }
                  frame True {
                  }
                }
              }
              frame #4 {
                n469 = property on="Y Backlash corr" class="Bool (strict)"() -> ("Value"=w994:bool)  [unwired: 2 in, 2 out]
                n470 = Implies(1:w1000, 2:w994) -> (0:w999:bool)
                n471 = case shown="False" w999 {
                  tunnel: w998 -> [w1008 w1065]
                  tunnel: w997 -> [w1007 w1066]
                  tunnel: [w1002 w1065] -> w996
                  tunnel: [w1006 w1066] -> w995
                  frame False {
                    # "Backlash"
                    n472 = flat-sequence {
                      tunnel: [w1021] -> w1020
                      tunnel: [w1025] -> w1019
                      tunnel: [w1024] -> w1018
                      tunnel: w1008 -> [w1023]
                      tunnel: w1007 -> [w1022]
                      tunnel: w1020 -> [w1033]
                      tunnel: [w1033] -> w1017
                      tunnel: w1019 -> [w1032]
                      tunnel: w1018 -> [w1031]
                      tunnel: [w1030] -> w1016
                      tunnel: [w1029] -> w1015
                      tunnel: [w1028] -> w1005
                      tunnel: w1017 -> [w1047]
                      tunnel: w1016 -> [w1038]
                      tunnel: w1015 -> [w1046]
                      tunnel: [w1038] -> w1014
                      tunnel: [w1046] -> w1013
                      tunnel: [w1037] -> w1010
                      tunnel: [w1045] -> w1009
                      tunnel: w1005 -> [w1045]
                      tunnel: w1014 -> [w1050]
                      tunnel: w1013 -> [w1051]
                      tunnel: [w1049] -> w1012
                      tunnel: [w1057] -> w1011
                      tunnel: w1010 -> [w1057]
                      tunnel: w1009 -> [w1053]
                      tunnel: [w1052] -> w1003
                      tunnel: w1012 -> [w1060]
                      tunnel: w1011 -> [w1059]
                      tunnel: [w1061] -> w1004
                      tunnel: w1003 -> [w1061]
                      tunnel: [w1060] -> w1001
                      tunnel: [w1064] -> w1006
                      tunnel: w1004 -> [w1064]
                      tunnel: [w1063] -> w1002
                      tunnel: w1001 -> [w1063]
                      frame #0 {
                        n473 = property on="Y Backlash steps/sec" class="DigNum (strict)"() -> ("Value"=w1021:i32)  [unwired: 2 in, 2 out]
                        n474 = Number To Decimal String(number=w1021) -> (decimal integer string=w1026:string)  [unwired: 1 in]
                        n475 = call "mdrive send command.vi"("error in (no error)"=w1023, "Extra"=w1026, "Command"=T10."Max Velocity", "VISA resource name"=w1022) -> ("error out"=w1024:errorcluster, "VISA resource name out"=w1025:refnum<visa-resource-name>)  [unwired: 3 in, 1 out]
                      }
                      frame #1 {
                        n476 = property on="Y Backlash" class="DigNum (strict)"() -> ("Value"=w1028:i32)  [unwired: 2 in, 2 out]
                        n477 = Number To Decimal String(number=w1028) -> (decimal integer string=w1034:string)  [unwired: 1 in]
                        n478 = call "mdrive send command.vi"("error in (no error)"=w1031, "Extra"=w1034, "Command"=T10."Move to Relative Position", "VISA resource name"=w1032) -> ("error out"=w1030:errorcluster, "VISA resource name out"=w1029:refnum<visa-resource-name>)  [unwired: 3 in, 1 out]
                      }
                      frame #2 {
                        n479 = To Double Precision Float(number=w1045) -> (double precision float=w1043:dbl)
                        n480 = To Double Precision Float(number=w1047) -> (double precision float=w1048:dbl)
                        n481 = Absolute Value(x=w1043) -> (abs(x)=w1044:dbl)
                        n482 = Divide(x=w1044, y=w1048) -> (x/y=w1041:dbl)
                        n483 = Multiply(x=1000.0, y=w1041) -> (x*y=w1039:dbl)
                        n484 = Add(x=w1039, y=300.0) -> (x+y=w1037:dbl)
                        n485 = To Unsigned Long Integer(number=w1037) -> (unsigned 32bit integer=w1036:u32)
                        n486 = Wait (ms)(milliseconds to wait=w1036) -> ()  [unwired: 1 out]
                      }
                      frame #3 {
                        n487 = Negate(x=w1053) -> (-x=w1054:i32)
                        n488 = Number To Decimal String(number=w1054) -> (decimal integer string=w1055:string)  [unwired: 1 in]
                        n489 = call "mdrive send command.vi"("error in (no error)"=w1050, "Extra"=w1055, "Command"=T10."Move to Relative Position", "VISA resource name"=w1051) -> ("error out"=w1049:errorcluster, "VISA resource name out"=w1052:refnum<visa-resource-name>)  [unwired: 3 in, 1 out]
                      }
                      frame #4 {
                        n490 = To Unsigned Long Integer(number=w1059) -> (unsigned 32bit integer=w1058:u32)
                        n491 = Wait (ms)(milliseconds to wait=w1058) -> ()  [unwired: 1 out]
                      }
                      frame #5 {
                        n492 = property on="Y Backlash corr" class="Bool (strict)"("Val(Sgnl)"=FALSE ("Value (Signaling)")) -> ()  [unwired: 2 in, 2 out]
                      }
                    }
                  }
                  frame True {
                  }
                }
              }
            }
            n493 = flat-sequence {
              tunnel: [w820] -> w720
              tunnel: [w822] -> w719
              tunnel: [w821] -> w718
              tunnel: w692 -> [w813]
              tunnel: w691 -> [w812]
              tunnel: [w842] -> w717
              tunnel: [w841] -> w716
              tunnel: [w840] -> w715
              tunnel: [w833] -> w714
              tunnel: w720 -> [w840]
              tunnel: w719 -> [w839]
              tunnel: w718 -> [w838]
              tunnel: w717 -> [w852]
              tunnel: [w852] -> w713
              tunnel: w716 -> [w851]
              tunnel: [w851] -> w712
              tunnel: w715 -> [w850]
              tunnel: [w850] -> w711
              tunnel: w714 -> [w849]
              tunnel: [w849] -> w710
              tunnel: [w856] -> w709
              tunnel: [w857] -> w708
              tunnel: [w853] -> w707
              tunnel: w710 -> [w853]
              tunnel: w711 -> [w854]
              tunnel: w712 -> [w858]
              tunnel: w713 -> [w855]
              tunnel: w709 -> [w869]
              tunnel: w708 -> [w870]
              tunnel: w707 -> [w872]
              tunnel: [w868] -> w699
              tunnel: [w867] -> w700
              frame #0 {
                n494 = property on="R Step SP" class="DigNum (strict)"() -> ("Maximum"=w815:dbl)  [unwired: 2 in, 2 out]
                n495 = property on="R Step SP" class="DigNum (strict)"() -> ("Minimum"=w816:dbl)  [unwired: 2 in, 2 out]
                n496 = property on="R steps/rev" class="DigNum (strict)"() -> ("Value"=w814:u32)  [unwired: 2 in, 2 out]
                n497 = property on="R offset deg" class="DigNum (strict)"() -> ("Value"=w818:dbl)  [unwired: 2 in, 2 out]
                n498 = To Long Integer(number=w815) -> (32bit integer=w829:i32)
                n499 = To Long Integer(number=w816) -> (32bit integer=w830:i32)
                n500 = To Double Precision Float(number=w814) -> (double precision float=w828:dbl)
                n501 = call "mdrive send command.vi"("error in (no error)"=w812, "Extra"="P", "Command"=T10."Print Parameter", "VISA resource name"=w813) -> ("error out"=w821:errorcluster, "read buffer"=w832:string, "VISA resource name out"=w822:refnum<visa-resource-name>)  [unwired: 3 in]
                n502 = Decimal String To Number(string=w832, offset=0) -> (number=w811:i32)  [unwired: 1 in, 1 out]
                n503 = property on="R Step PV" class="DigNum (strict)"("Val(Sgnl)"=w811) -> ()  [unwired: 2 in, 2 out]
                n504 = In Range and Coerce(upper limit=w829, x=w811, lower limit=w830) -> (In Range?=w820:bool)  [unwired: 1 out]
                n505 = To Double Precision Float(number=w811) -> (double precision float=w825:dbl)
                n506 = property on="R in Range" class="Bool (strict)"("Val(Sgnl)"=w820) -> ()  [unwired: 2 in, 2 out]
                n507 = Divide(x=w825, y=w828) -> (x/y=w827:dbl)
                n508 = property on="R deg/rev" class="DigNum (strict)"() -> ("Value"=w817:dbl)  [unwired: 2 in, 2 out]
                n509 = Multiply(x=w827, y=w817) -> (x*y=w826:dbl)
                n510 = Add(x=w826, y=w818) -> (x+y=w819:dbl)
                n511 = property on="R Position deg PV" class="DigNum (strict)"("Val(Sgnl)"=w819) -> ()  [unwired: 2 in, 2 out]
              }
              frame #1 {
                n512 = call "mdrive send command.vi"("error in (no error)"=w838, "Extra"="MV", "Command"=T10."Print Parameter", "VISA resource name"=w839) -> ("error out"=w841:errorcluster, "read buffer"=w844:string, "VISA resource name out"=w842:refnum<visa-resource-name>)  [unwired: 3 in]
                n513 = Decimal String To Number(string=w844, offset=0 ("offset (0)")) -> (number=w834:i32)  [unwired: 1 in, 1 out]
                n514 = Not Equal?(x=w844, y="") -> (x != y?=w837:bool)
                n515 = property on="R Ready" class="Bool (strict)"("Val(Sgnl)"=w837) -> ()  [unwired: 2 in, 2 out]
                n516 = Number To Boolean Array(number=w834) -> (Boolean array=w836:bool[])
                n517 = Index Array(array=w836, index=0) -> (element=w833:bool)
                n518 = property on="R in Motion" class="Bool (strict)"("Val(Sgnl)"=w833) -> ()  [unwired: 2 in, 2 out]
              }
              frame #2 {
                n519 = Wait (ms)(milliseconds to wait=u32 50) -> ()  [unwired: 1 out]
              }
              frame #3 {
                n520 = case shown="True" w854 {
                  tunnel: w855 -> [w861 w865]
                  tunnel: [w862 w865] -> w856
                  tunnel: [w863 w864] -> w857
                  tunnel: w858 -> [w860 w864]
                  frame False {
                    n521 = call "mdrive send command.vi"("error in (no error)"=w860, "Command"=T10."Stop", "VISA resource name"=w861) -> ("error out"=w863:errorcluster, "VISA resource name out"=w862:refnum<visa-resource-name>)  [unwired: 4 in, 1 out]
                  }
                  frame True {
                  }
                }
              }
              frame #4 {
                n522 = property on="R Backlash corr" class="Bool (strict)"() -> ("Value"=w866:bool)  [unwired: 2 in, 2 out]
                n523 = Implies(1:w872, 2:w866) -> (0:w871:bool)
                n524 = case shown="False" w871 {
                  tunnel: w870 -> [w880 w937]
                  tunnel: w869 -> [w879 w938]
                  tunnel: [w874 w937] -> w868
                  tunnel: [w878 w938] -> w867
                  frame False {
                    # "Backlash"
                    n525 = flat-sequence {
                      tunnel: [w893] -> w892
                      tunnel: [w897] -> w891
                      tunnel: [w896] -> w890
                      tunnel: w880 -> [w895]
                      tunnel: w879 -> [w894]
                      tunnel: w892 -> [w905]
                      tunnel: [w905] -> w889
                      tunnel: w891 -> [w904]
                      tunnel: w890 -> [w903]
                      tunnel: [w902] -> w888
                      tunnel: [w901] -> w887
                      tunnel: [w900] -> w877
                      tunnel: w889 -> [w919]
                      tunnel: w888 -> [w910]
                      tunnel: w887 -> [w918]
                      tunnel: [w910] -> w886
                      tunnel: [w918] -> w885
                      tunnel: [w909] -> w882
                      tunnel: [w917] -> w881
                      tunnel: w877 -> [w917]
                      tunnel: w886 -> [w922]
                      tunnel: w885 -> [w923]
                      tunnel: [w921] -> w884
                      tunnel: [w929] -> w883
                      tunnel: w882 -> [w929]
                      tunnel: w881 -> [w925]
                      tunnel: [w924] -> w875
                      tunnel: w884 -> [w932]
                      tunnel: w883 -> [w931]
                      tunnel: [w933] -> w876
                      tunnel: w875 -> [w933]
                      tunnel: [w932] -> w873
                      tunnel: [w936] -> w878
                      tunnel: w876 -> [w936]
                      tunnel: [w935] -> w874
                      tunnel: w873 -> [w935]
                      frame #0 {
                        n526 = property on="R Backlash steps/sec" class="DigNum (strict)"() -> ("Value"=w893:i32)  [unwired: 2 in, 2 out]
                        n527 = Number To Decimal String(number=w893) -> (decimal integer string=w898:string)  [unwired: 1 in]
                        n528 = call "mdrive send command.vi"("error in (no error)"=w895, "Extra"=w898, "Command"=T10."Max Velocity", "VISA resource name"=w894) -> ("error out"=w896:errorcluster, "VISA resource name out"=w897:refnum<visa-resource-name>)  [unwired: 3 in, 1 out]
                      }
                      frame #1 {
                        n529 = property on="R Backlash" class="DigNum (strict)"() -> ("Value"=w900:i32)  [unwired: 2 in, 2 out]
                        n530 = Number To Decimal String(number=w900) -> (decimal integer string=w906:string)  [unwired: 1 in]
                        n531 = call "mdrive send command.vi"("error in (no error)"=w903, "Extra"=w906, "Command"=T10."Move to Relative Position", "VISA resource name"=w904) -> ("error out"=w902:errorcluster, "VISA resource name out"=w901:refnum<visa-resource-name>)  [unwired: 3 in, 1 out]
                      }
                      frame #2 {
                        n532 = To Double Precision Float(number=w917) -> (double precision float=w915:dbl)
                        n533 = To Double Precision Float(number=w919) -> (double precision float=w920:dbl)
                        n534 = Absolute Value(x=w915) -> (abs(x)=w916:dbl)
                        n535 = Divide(x=w916, y=w920) -> (x/y=w913:dbl)
                        n536 = Multiply(x=1000.0, y=w913) -> (x*y=w911:dbl)
                        n537 = Add(x=w911, y=300.0) -> (x+y=w909:dbl)
                        n538 = To Unsigned Long Integer(number=w909) -> (unsigned 32bit integer=w908:u32)
                        n539 = Wait (ms)(milliseconds to wait=w908) -> ()  [unwired: 1 out]
                      }
                      frame #3 {
                        n540 = Negate(x=w925) -> (-x=w926:i32)
                        n541 = Number To Decimal String(number=w926) -> (decimal integer string=w927:string)  [unwired: 1 in]
                        n542 = call "mdrive send command.vi"("error in (no error)"=w922, "Extra"=w927, "Command"=T10."Move to Relative Position", "VISA resource name"=w923) -> ("error out"=w921:errorcluster, "VISA resource name out"=w924:refnum<visa-resource-name>)  [unwired: 3 in, 1 out]
                      }
                      frame #4 {
                        n543 = To Unsigned Long Integer(number=w931) -> (unsigned 32bit integer=w930:u32)
                        n544 = Wait (ms)(milliseconds to wait=w930) -> ()  [unwired: 1 out]
                      }
                      frame #5 {
                        n545 = property on="R Backlash corr" class="Bool (strict)"("Val(Sgnl)"=FALSE ("Value (Signaling)")) -> ()  [unwired: 2 in, 2 out]
                      }
                    }
                  }
                  frame True {
                  }
                }
              }
            }
            n546 = property on="Scan Go" class="Bool (strict)"() -> ("Value"=w690:bool)  [unwired: 2 in, 2 out]
            n547 = Equal?(x=w690, y=TRUE) -> (x = y?=w685:bool)
            n548 = property on="STATUS" class="Str"() -> ("Value"=w688:string)  [unwired: 2 in, 2 out]
            n549 = Equal?(x=w688, y="SCANNING MODE" ("STATUS")) -> (x = y?=w686:bool)
            n550 = Or(x=w686, y=w685) -> (x .or. y?=w684:bool)
            n551 = case shown="False" w684 {
              frame False {
                n552 = property on="Y in Motion" class="Bool (strict)"() -> ("Value"=w766:bool)  [unwired: 2 in, 2 out]
                n553 = property on="Z in Motion" class="Bool (strict)"() -> ("Value"=w769:bool)  [unwired: 2 in, 2 out]
                n554 = property on="X  in Motion" class="Bool (strict)"() -> ("Value"=w767:bool)  [unwired: 2 in, 2 out]
                n555 = property on="R in Motion" class="Bool (strict)"() -> ("Value"=w768:bool)  [unwired: 2 in, 2 out]
                n556 = Compound Arithmetic op=AND(w767, w766, w769, w768) -> (w764:bool)
                n557 = Equal?(x=w764, y=FALSE) -> (x = y?=w765:bool)
                n558 = case shown="True" w765 {
                  frame False {
                  }
                  frame True {
                    n559 = property on="X Step SP" class="DigNum (strict)"() -> ("Value"=w777:i32)  [unwired: 2 in, 2 out]
                    n560 = property on="X Step PV" class="DigNum (strict)"() -> ("Value"=w776:i32)  [unwired: 2 in, 2 out]
                    n561 = property on="Y Step SP" class="DigNum (strict)"() -> ("Value"=w775:i32)  [unwired: 2 in, 2 out]
                    n562 = property on="Y Step PV" class="DigNum (strict)"() -> ("Value"=w774:i32)  [unwired: 2 in, 2 out]
                    n563 = property on="Z Step SP" class="DigNum (strict)"() -> ("Value"=w773:i32)  [unwired: 2 in, 2 out]
                    n564 = property on="Z Step PV" class="DigNum (strict)"() -> ("Value"=w772:i32)  [unwired: 2 in, 2 out]
                    n565 = property on="R Step SP" class="DigNum (strict)"() -> ("Value"=w770:i32)  [unwired: 2 in, 2 out]
                    n566 = property on="R Step PV" class="DigNum (strict)"() -> ("Value"=w771:i32)  [unwired: 2 in, 2 out]
                    n567 = Equal?(x=w777, y=w776) -> (x = y?=w782:bool)
                    n568 = Equal?(x=w775, y=w774) -> (x = y?=w781:bool)
                    n569 = Equal?(x=w773, y=w772) -> (x = y?=w779:bool)
                    n570 = Equal?(x=w770, y=w771) -> (x = y?=w780:bool)
                    n571 = Compound Arithmetic op=AND(w782, w781, w779, w780) -> (w778:bool)
                    n572 = case shown="True" w778 {
                      frame False {
                      }
                      frame True {
                        n573 = property on="GO" class="Bool"("DisabledEnum"=T9."Enabled" ("Disabled")) -> ()  [unwired: 2 in, 2 out]
                        n574 = local write "STATUS"("SCANNING DONE" ("STATUS")) -> ()
                      }
                    }
                  }
                }
              }
              frame True {
                n575 = property on="X Scan Length SP steps" class="DigNum (strict)"() -> ("Value"=w796:i32)  [unwired: 2 in, 2 out]
                n576 = property on="Y Scan Length SP steps" class="DigNum (strict)"() -> ("Value"=w795:i32)  [unwired: 2 in, 2 out]
                n577 = property on="Z Scan Length SP steps" class="DigNum (strict)"() -> ("Value"=w794:i32)  [unwired: 2 in, 2 out]
                n578 = property on="R Scan Length SP steps" class="DigNum (strict)"() -> ("Value"=w793:i32)  [unwired: 2 in, 2 out]
                n579 = property on="X Step SP" class="DigNum (strict)"() -> ("Value"=w792:i32)  [unwired: 2 in, 2 out]
                n580 = property on="Y Step SP" class="DigNum (strict)"() -> ("Value"=w791:i32)  [unwired: 2 in, 2 out]
                n581 = property on="Z Step SP" class="DigNum (strict)"() -> ("Value"=w790:i32)  [unwired: 2 in, 2 out]
                n582 = property on="R Step SP" class="DigNum (strict)"() -> ("Value"=w789:i32)  [unwired: 2 in, 2 out]
                n583 = Add(x=w796, y=w792) -> (x+y=w805:i32)
                n584 = Add(x=w795, y=w791) -> (x+y=w804:i32)
                n585 = Add(x=w794, y=w790) -> (x+y=w803:i32)
                n586 = Add(x=w793, y=w789) -> (x+y=w802:i32)
                n587 = property on="X Step PV" class="DigNum (strict)"() -> ("Value"=w788:i32)  [unwired: 2 in, 2 out]
                n588 = property on="Y Step PV" class="DigNum (strict)"() -> ("Value"=w787:i32)  [unwired: 2 in, 2 out]
                n589 = property on="Z Step PV" class="DigNum (strict)"() -> ("Value"=w786:i32)  [unwired: 2 in, 2 out]
                n590 = property on="R Step PV" class="DigNum (strict)"() -> ("Value"=w785:i32)  [unwired: 2 in, 2 out]
                n591 = Equal?(x=w788, y=w805) -> (x = y?=w801:bool)
                n592 = Equal?(x=w787, y=w804) -> (x = y?=w800:bool)
                n593 = Equal?(x=w786, y=w803) -> (x = y?=w798:bool)
                n594 = Equal?(x=w785, y=w802) -> (x = y?=w799:bool)
                n595 = Compound Arithmetic op=AND(w801, w800, w798, w799) -> (w797:bool)
                n596 = case shown="True" w797 {
                  frame False {
                  }
                  frame True {
                    n597 = local write "Scan Go"(FALSE ("Scan Go")) -> ()
                    n598 = local write "STATUS"("DONE" ("STATUS")) -> ()
                    n599 = property on="Send scan parameter" class="Bool"("DisabledEnum"=T9."Enabled" ("Disabled")) -> ()  [unwired: 2 in, 2 out]
                    n600 = property on="Set Scan \nParameters" class="Bool"("DisabledEnum"=T9."Enabled" ("Disabled")) -> ()  [unwired: 2 in, 2 out]
                    n601 = property on="GO" class="Bool"("DisabledEnum"=T9."Enabled" ("Disabled")) -> ()  [unwired: 2 in, 2 out]
                  }
                }
              }
            }
          }
        }
        n602 = case shown="False" w497 {
          tunnel: w501 -> [w542 w547]
          tunnel: [w542 w546] -> w500
          tunnel: w499 -> [w541 w545]
          tunnel: [w541 w544] -> w498
          frame False {
          }
          frame True {
            w543 = 0 ("dimension size")
            n603 = Reshape Array(w547, w543) -> (w546:dbl[])
            n604 = Reshape Array(w545, w543) -> (w544:dbl[])
          }
        }
        n605 = And(x=w511, y=w507) -> (x .and. y?=w508:bool)
        n606 = case shown="False" w507 {
          frame False {
            n607 = local write "STATUS"("SCANNING MODE" ("STATUS")) -> ()
          }
          frame True {
          }
        }
        n608 = Divide(x=w530, y=6.283185307179586) -> (x/y=w531:dbl)
        n609 = case shown="False" w508 {
          frame False {
          }
          frame True {
            n610 = local write "STATUS"("") -> ()
          }
        }
        n611 = Multiply(x=360.0, y=w531) -> (x*y=w534:dbl)
        n612 = property on="atan Y/Z" class="DigNum (strict)"("Val(Sgnl)"=w534) -> ()  [unwired: 2 in, 2 out]
      }
      event "OK Button": Value Change {
        n613 = event-data() -> ()  [unwired: 1 in, 5 out]
        n614 = property on="OK Button" class="Bool (strict)"() -> ("Value"=w1339:bool)  [unwired: 2 in, 2 out]
        n615 = property on="Z Step PV" class="DigNum (strict)"() -> ("Value"=w1344:i32)  [unwired: 2 in, 2 out]
        n616 = Greater?(x=w1344, y=15360000) -> (0:w1341:bool)
        n617 = Equal?(x=w1339, y=TRUE) -> (x = y?=w1342:bool)
        n618 = local write "STATUS"("VALVE CHANGED" ("STATUS")) -> ()
        n619 = And(x=w1342, y=w1341) -> (x .and. y?=w1340:bool)
        n620 = case shown="False" w1340 {
          frame False {
            n621 = property on="OK Button" class="Bool (strict)"() -> ("Value"=w1347:bool)  [unwired: 2 in, 2 out]
            n622 = property on="Z Step PV" class="DigNum (strict)"() -> ("Value"=w1352:i32)  [unwired: 2 in, 2 out]
            n623 = Greater?(x=w1352, y=15360000) -> (0:w1350:bool)
            n624 = Equal?(x=w1347, y=FALSE) -> (x = y?=w1349:bool)
            n625 = And(x=w1349, y=w1350) -> (x .and. y?=w1348:bool)
            n626 = case shown="True" w1348 {
              frame False {
              }
              frame True {
                n627 = One Button Dialog(message="YOU CAN'T CLOSE THE VALVE\nWHEN YOU ARE IN THE THIS\nPOSITION!!") -> (true=w1354:bool)  [unwired: 1 in]
                n628 = property on="OK Button" class="Bool (strict)"("Val(Sgnl)"=w1354) -> ()  [unwired: 2 in, 2 out]
              }
            }
          }
          frame True {
            n629 = flat-sequence {
              frame #0 {
                n630 = local read "OK Button"() -> (w1357:bool)
                n631 = call "DigitalIO_sub_V1_CNTL.vi"("OK Button"=w1357) -> ("Boolean"=w1356:bool)  [unwired: 2 in]
                n632 = property on="V5 Valve \nopend/closed" class="Bool (strict)"("Val(Sgnl)"=w1356) -> ()  [unwired: 2 in, 2 out]
              }
              frame #1 {
                n633 = call "DigitalIO_sub_V1_MON.vi"() -> ("CL"=w1359:bool, "OP"=w1358:bool)  [unwired: 8 in]
                n634 = property on="OP" class="Bool (strict)"("Val(Sgnl)"=w1358) -> ()  [unwired: 2 in, 2 out]
                n635 = property on="CL" class="Bool (strict)"("Val(Sgnl)"=w1359) -> ()  [unwired: 2 in, 2 out]
              }
              frame #2 {
                n636 = Wait (ms)(milliseconds to wait=u32 100) -> ()  [unwired: 1 out]
              }
            }
          }
        }
      }
      event "GO": Mouse Up {
        n637 = event-data() -> ()  [unwired: 1 in, 7 out]
        n638 = local write "STATUS"("MOVING" ("STATUS")) -> ()
        n639 = property on="X Position mm PV" class="DigNum (strict)"() -> ("Value"=w1381:dbl)  [unwired: 2 in, 2 out]
        n640 = property on="X Position SP mm" class="DigNum (strict)"() -> ("Value"=w1380:dbl)  [unwired: 2 in, 2 out]
        n641 = property on="Z Position mm PV" class="DigNum (strict)"() -> ("Value"=w1377:dbl)  [unwired: 2 in, 2 out]
        n642 = property on="Z Position SP mm" class="DigNum (strict)"() -> ("Value"=w1369:dbl)  [unwired: 2 in, 2 out]
        n643 = property on="Y Position mm PV" class="DigNum (strict)"() -> ("Value"=w1375:dbl)  [unwired: 2 in, 2 out]
        n644 = property on="Y Position SP mm" class="DigNum (strict)"() -> ("Value"=w1374:dbl)  [unwired: 2 in, 2 out]
        n645 = property on="R Position SP deg" class="DigNum (strict)"() -> ("Value"=w1372:dbl)  [unwired: 2 in, 2 out]
        n646 = property on="R Position deg PV" class="DigNum (strict)"() -> ("Value"=w1371:dbl)  [unwired: 2 in, 2 out]
        n647 = Not Equal?(x=w1381, y=w1380) -> (x != y?=w1379:bool)
        n648 = Not Equal?(x=w1377, y=w1369) -> (x != y?=w1378:bool)
        n649 = Not Equal?(x=w1375, y=w1374) -> (x != y?=w1376:bool)
        n650 = Not Equal?(x=w1372, y=w1371) -> (x != y?=w1373:bool)
        n651 = case shown="True" w1378 {
          tunnel: w1388 -> [w1531 w1538]
          tunnel: w1387 -> [w1532 w1537]
          tunnel: [w1532 w1536] -> w1366
          tunnel: [w1531 w1535] -> w1365
          frame False {
          }
          frame True {
            n652 = flat-sequence {
              tunnel: w1537 -> [w1560]
              tunnel: w1538 -> [w1561]
              tunnel: [w1561] -> w1534
              tunnel: [w1560] -> w1533
              tunnel: [w1576] -> w1552
              tunnel: [w1575] -> w1551
              tunnel: [w1563] -> w1550
              tunnel: w1534 -> [w1576]
              tunnel: w1533 -> [w1575]
              tunnel: [w1579] -> w1549
              tunnel: [w1578] -> w1548
              tunnel: [w1577] -> w1547
              tunnel: w1550 -> [w1577]
              tunnel: w1551 -> [w1578]
              tunnel: w1552 -> [w1579]
              tunnel: [w1595] -> w1546
              tunnel: [w1594] -> w1545
              tunnel: w1549 -> [w1593]
              tunnel: w1548 -> [w1592]
              tunnel: [w1591] -> w1544
              tunnel: w1547 -> [w1591]
              tunnel: w1546 -> [w1602]
              tunnel: [w1602] -> w1543
              tunnel: w1545 -> [w1601]
              tunnel: [w1601] -> w1542
              tunnel: w1544 -> [w1600]
              tunnel: [w1600] -> w1541
              tunnel: [w1607] -> w1540
              tunnel: [w1606] -> w1539
              tunnel: w1543 -> [w1605]
              tunnel: w1542 -> [w1604]
              tunnel: w1541 -> [w1603]
              tunnel: [w1611] -> w1535
              tunnel: [w1612] -> w1536
              tunnel: w1540 -> [w1612]
              tunnel: w1539 -> [w1611]
              frame #0 {
                n653 = property on="Z Position mm PV" class="DigNum (strict)"() -> ("Value"=w1553:dbl)  [unwired: 2 in, 2 out]
                n654 = property on="Z Position SP mm" class="DigNum (strict)"() -> ("Value"=w1555:dbl)  [unwired: 2 in, 2 out]
                n655 = Less?(x=w1553, y=60.0) -> (x < y?=w1557:bool)
                n656 = Greater?(x=w1555, y=60.0) -> (0:w1558:bool)
                n657 = And(x=w1557, y=w1558) -> (x .and. y?=w1559:bool)
                n658 = case shown="True" w1559 {
                  frame False {
                  }
                  frame True {
                    n659 = property on="Z Position SP mm" class="DigNum (strict)"("Val(Sgnl)"=60.0 ("Value (Signaling)")) -> ()  [unwired: 2 in, 2 out]
                  }
                }
              }
              frame #1 {
                n660 = property on="Z steps/rev" class="DigNum (strict)"() -> ("Value"=w1572:u32)  [unwired: 2 in, 2 out]
                n661 = To Double Precision Float(number=w1572) -> (double precision float=w1568:dbl)
                n662 = property on="Z offset mm" class="DigNum (strict)"() -> ("Value"=w1570:dbl)  [unwired: 2 in, 2 out]
                n663 = property on="Z Position SP mm" class="DigNum (strict)"() -> ("Value"=w1569:dbl)  [unwired: 2 in, 2 out]
                n664 = Subtract(x=w1569, y=w1570) -> (x-y=w1565:dbl)
                n665 = property on="Z mm/rev" class="DigNum (strict)"() -> ("Value"=w1571:dbl)  [unwired: 2 in, 2 out]
                n666 = Divide(x=w1565, y=w1571) -> (x/y=w1564:dbl)
                n667 = property on="Z Step SP" class="DigNum (strict)"() -> ("Maximum"=w1574:dbl)  [unwired: 2 in, 2 out]
                n668 = property on="Z Step SP" class="DigNum (strict)"() -> ("Minimum"=w1573:dbl)  [unwired: 2 in, 2 out]
                n669 = Multiply(x=w1564, y=w1568) -> (x*y=w1566:dbl)
                n670 = In Range and Coerce(upper limit=w1574, x=w1566, lower limit=w1573) -> (coerced(x)=w1567:dbl)  [unwired: 1 out]
                n671 = To Long Integer(number=w1567) -> (32bit integer=w1563:i32)
                n672 = property on="Z Step SP" class="DigNum (strict)"("Val(Sgnl)"=w1563) -> ()  [unwired: 2 in, 2 out]
              }
              frame #2 {
                n673 = property on="Z Step SP" class="DigNum (strict)"() -> ("Value"=w1588:i32)  [unwired: 2 in, 2 out]
                n674 = property on="Z Step PV" class="DigNum (strict)"() -> ("Value"=w1587:i32)  [unwired: 2 in, 2 out]
                n675 = property on="Z Backlash" class="DigNum (strict)"() -> ("Value"=w1580:i32)  [unwired: 2 in, 2 out]
                n676 = Subtract(x=w1588, y=w1587) -> (x-y=w1586:i32)
                n677 = Sign(1:w1580) -> (0:w1584:i32)
                n678 = Sign(1:w1586) -> (0:w1585:i32)
                n679 = Multiply(x=w1585, y=w1584) -> (x*y=w1583:i32)
                n680 = Equal?(x=w1583, y=1) -> (x = y?=w1581:bool)
                n681 = case shown="False" w1581 {
                  frame False {
                    n682 = property on="Z Backlash corr" class="Bool (strict)"("Val(Sgnl)"=FALSE ("Value (Signaling)")) -> ()  [unwired: 2 in, 2 out]
                  }
                  frame True {
                    n683 = property on="Z Backlash corr" class="Bool (strict)"("Val(Sgnl)"=TRUE ("Value (Signaling)")) -> ()  [unwired: 2 in, 2 out]
                  }
                }
              }
              frame #3 {
                # "Velocity Setting"
                n684 = property on="Z Velocity SP step/sec" class="DigNum (strict)"() -> ("Value"=w1596:i32)  [unwired: 2 in, 2 out]
                n685 = Number To Decimal String(number=w1596) -> (decimal integer string=w1597:string)  [unwired: 1 in]
                n686 = call "mdrive send command.vi"("error in (no error)"=w1593, "Extra"=w1597, "Command"=T10."Max Velocity", "VISA resource name"=w1592) -> ("error out"=w1594:errorcluster, "VISA resource name out"=w1595:refnum<visa-resource-name>)  [unwired: 3 in, 1 out]
              }
              frame #4 {
                n687 = Wait (ms)(milliseconds to wait=u32 50) -> ()  [unwired: 1 out]
              }
              frame #5 {
                # "Move to Abs Position"
                n688 = Number To Decimal String(number=w1603) -> (decimal integer string=w1609:string)  [unwired: 1 in]
                n689 = call "mdrive send command.vi"("error in (no error)"=w1604, "Extra"=w1609, "Command"=T10."Move to Absolute Position", "VISA resource name"=w1605) -> ("error out"=w1606:errorcluster, "VISA resource name out"=w1607:refnum<visa-resource-name>)  [unwired: 3 in, 1 out]
              }
              frame #6 {
                n690 = Wait (ms)(milliseconds to wait=u32 50) -> ()  [unwired: 1 out]
              }
            }
          }
        }
        n691 = property on="GO" class="Bool"("DisabledEnum"=T9."Disabled and Grayed Out" ("Disabled")) -> ()  [unwired: 2 in, 2 out]
        n692 = case shown="True" w1379 {
          tunnel: w1390 -> [w1614 w1618]
          tunnel: w1389 -> [w1613 w1617]
          tunnel: [w1614 w1616] -> w1368
          tunnel: [w1613 w1615] -> w1367
          frame False {
          }
          frame True {
            n693 = flat-sequence {
              tunnel: w1617 -> [w1645]
              tunnel: w1618 -> [w1646]
              tunnel: [w1646] -> w1632
              tunnel: [w1645] -> w1631
              tunnel: [w1634] -> w1630
              tunnel: [w1649] -> w1629
              tunnel: [w1648] -> w1628
              tunnel: [w1647] -> w1627
              tunnel: w1630 -> [w1647]
              tunnel: w1631 -> [w1648]
              tunnel: w1632 -> [w1649]
              tunnel: [w1665] -> w1626
              tunnel: [w1664] -> w1625
              tunnel: w1629 -> [w1663]
              tunnel: w1628 -> [w1662]
              tunnel: w1627 -> [w1661]
              tunnel: [w1661] -> w1624
              tunnel: w1626 -> [w1672]
              tunnel: [w1672] -> w1623
              tunnel: w1625 -> [w1671]
              tunnel: [w1671] -> w1622
              tunnel: [w1669] -> w1621
              tunnel: w1624 -> [w1669]
              tunnel: [w1677] -> w1620
              tunnel: [w1676] -> w1619
              tunnel: w1623 -> [w1675]
              tunnel: w1622 -> [w1674]
              tunnel: w1621 -> [w1673]
              tunnel: [w1681] -> w1615
              tunnel: [w1682] -> w1616
              tunnel: w1620 -> [w1682]
              tunnel: w1619 -> [w1681]
              frame #0 {
                n694 = property on="X steps/rev" class="DigNum (strict)"() -> ("Value"=w1644:u32)  [unwired: 2 in, 2 out]
                n695 = To Double Precision Float(number=w1644) -> (double precision float=w1639:dbl)
                n696 = property on="X offset mm" class="DigNum (strict)"() -> ("Value"=w1643:dbl)  [unwired: 2 in, 2 out]
                n697 = property on="X Position SP mm" class="DigNum (strict)"() -> ("Value"=w1642:dbl)  [unwired: 2 in, 2 out]
                n698 = Subtract(x=w1642, y=w1643) -> (x-y=w1636:dbl)
                n699 = property on="X mm/rev" class="DigNum (strict)"() -> ("Value"=w1633:dbl)  [unwired: 2 in, 2 out]
                n700 = Divide(x=w1636, y=w1633) -> (x/y=w1635:dbl)
                n701 = property on="X Step SP" class="DigNum (strict)"() -> ("Maximum"=w1641:dbl)  [unwired: 2 in, 2 out]
                n702 = property on="X Step SP" class="DigNum (strict)"() -> ("Minimum"=w1640:dbl)  [unwired: 2 in, 2 out]
                n703 = Multiply(x=w1635, y=w1639) -> (x*y=w1637:dbl)
                n704 = In Range and Coerce(upper limit=w1641, x=w1637, lower limit=w1640) -> (coerced(x)=w1638:dbl)  [unwired: 1 out]
                n705 = To Long Integer(number=w1638) -> (32bit integer=w1634:i32)
                n706 = property on="X Step SP" class="DigNum (strict)"("Val(Sgnl)"=w1634) -> ()  [unwired: 2 in, 2 out]
              }
              frame #1 {
                n707 = property on="X Step SP" class="DigNum (strict)"() -> ("Value"=w1658:i32)  [unwired: 2 in, 2 out]
                n708 = property on="X Step PV" class="DigNum (strict)"() -> ("Value"=w1657:i32)  [unwired: 2 in, 2 out]
                n709 = property on="X Backlash" class="DigNum (strict)"() -> ("Value"=w1650:i32)  [unwired: 2 in, 2 out]
                n710 = Subtract(x=w1658, y=w1657) -> (x-y=w1656:i32)
                n711 = Sign(1:w1650) -> (0:w1654:i32)
                n712 = Sign(1:w1656) -> (0:w1655:i32)
                n713 = Multiply(x=w1655, y=w1654) -> (x*y=w1653:i32)
                n714 = Equal?(x=w1653, y=1) -> (x = y?=w1651:bool)
                n715 = case shown="False" w1651 {
                  frame False {
                    n716 = property on="X Backlash corr" class="Bool (strict)"("Val(Sgnl)"=FALSE ("Value (Signaling)")) -> ()  [unwired: 2 in, 2 out]
                  }
                  frame True {
                    n717 = property on="X Backlash corr" class="Bool (strict)"("Val(Sgnl)"=TRUE ("Value (Signaling)")) -> ()  [unwired: 2 in, 2 out]
                  }
                }
              }
              frame #2 {
                # "Velocity Setting"
                n718 = property on="X Velocity SP step/sec" class="DigNum (strict)"() -> ("Value"=w1666:i32)  [unwired: 2 in, 2 out]
                n719 = Number To Decimal String(number=w1666) -> (decimal integer string=w1667:string)  [unwired: 1 in]
                n720 = call "mDrive Send Command.vi"("error in (no error)"=w1662, "Extra"=w1667, "Command"=T10."Max Velocity", "VISA resource name"=w1663) -> ("error out"=w1664:errorcluster, "VISA resource name out"=w1665:refnum<visa-resource-name>)  [unwired: 3 in, 1 out]
              }
              frame #3 {
                n721 = Wait (ms)(milliseconds to wait=u32 50) -> ()  [unwired: 1 out]
              }
              frame #4 {
                # "Move to Abs Position"
                n722 = Number To Decimal String(number=w1673) -> (decimal integer string=w1679:string)  [unwired: 1 in]
                n723 = call "mDrive Send Command.vi"("error in (no error)"=w1674, "Extra"=w1679, "Command"=T10."Move to Absolute Position", "VISA resource name"=w1675) -> ("error out"=w1676:errorcluster, "VISA resource name out"=w1677:refnum<visa-resource-name>)  [unwired: 3 in, 1 out]
              }
              frame #5 {
                n724 = Wait (ms)(milliseconds to wait=u32 50) -> ()  [unwired: 1 out]
              }
            }
          }
        }
        n725 = case shown="True" w1376 {
          tunnel: w1386 -> [w1461 w1466]
          tunnel: w1385 -> [w1462 w1465]
          tunnel: [w1462 w1464] -> w1364
          tunnel: [w1461 w1463] -> w1363
          frame False {
          }
          frame True {
            n726 = flat-sequence {
              tunnel: [w1494] -> w1480
              tunnel: [w1493] -> w1479
              tunnel: [w1481] -> w1478
              tunnel: w1465 -> [w1493]
              tunnel: w1466 -> [w1494]
              tunnel: [w1497] -> w1477
              tunnel: [w1496] -> w1476
              tunnel: [w1495] -> w1475
              tunnel: w1478 -> [w1495]
              tunnel: w1479 -> [w1496]
              tunnel: w1480 -> [w1497]
              tunnel: [w1513] -> w1474
              tunnel: [w1512] -> w1473
              tunnel: w1477 -> [w1511]
              tunnel: w1476 -> [w1510]
              tunnel: [w1509] -> w1472
              tunnel: w1475 -> [w1509]
              tunnel: w1474 -> [w1520]
              tunnel: [w1520] -> w1471
              tunnel: w1473 -> [w1519]
              tunnel: [w1519] -> w1470
              tunnel: [w1517] -> w1469
              tunnel: w1472 -> [w1517]
              tunnel: [w1525] -> w1468
              tunnel: [w1524] -> w1467
              tunnel: w1471 -> [w1523]
              tunnel: w1470 -> [w1522]
              tunnel: w1469 -> [w1521]
              tunnel: [w1528] -> w1463
              tunnel: [w1530] -> w1464
              tunnel: w1468 -> [w1530]
              tunnel: w1467 -> [w1528]
              frame #0 {
                n727 = property on="Y steps/rev" class="DigNum (strict)"() -> ("Value"=w1490:u32)  [unwired: 2 in, 2 out]
                n728 = To Double Precision Float(number=w1490) -> (double precision float=w1486:dbl)
                n729 = property on="Y offset mm" class="DigNum (strict)"() -> ("Value"=w1488:dbl)  [unwired: 2 in, 2 out]
                n730 = property on="Y Position SP mm" class="DigNum (strict)"() -> ("Value"=w1487:dbl)  [unwired: 2 in, 2 out]
                n731 = Subtract(x=w1487, y=w1488) -> (x-y=w1483:dbl)
                n732 = property on="Y mm/rev" class="DigNum (strict)"() -> ("Value"=w1489:dbl)  [unwired: 2 in, 2 out]
                n733 = Divide(x=w1483, y=w1489) -> (x/y=w1482:dbl)
                n734 = property on="Y Step SP" class="DigNum (strict)"() -> ("Maximum"=w1491:dbl)  [unwired: 2 in, 2 out]
                n735 = property on="Y Step SP" class="DigNum (strict)"() -> ("Minimum"=w1492:dbl)  [unwired: 2 in, 2 out]
                n736 = Multiply(x=w1482, y=w1486) -> (x*y=w1484:dbl)
                n737 = In Range and Coerce(upper limit=w1491, x=w1484, lower limit=w1492) -> (coerced(x)=w1485:dbl)  [unwired: 1 out]
                n738 = To Long Integer(number=w1485) -> (32bit integer=w1481:i32)
                n739 = property on="Y Step SP" class="DigNum (strict)"("Val(Sgnl)"=w1481) -> ()  [unwired: 2 in, 2 out]
              }
              frame #1 {
                n740 = property on="Y Step SP" class="DigNum (strict)"() -> ("Value"=w1506:i32)  [unwired: 2 in, 2 out]
                n741 = property on="Y Step PV" class="DigNum (strict)"() -> ("Value"=w1505:i32)  [unwired: 2 in, 2 out]
                n742 = property on="Y Backlash" class="DigNum (strict)"() -> ("Value"=w1498:i32)  [unwired: 2 in, 2 out]
                n743 = Subtract(x=w1506, y=w1505) -> (x-y=w1504:i32)
                n744 = Sign(1:w1498) -> (0:w1502:i32)
                n745 = Sign(1:w1504) -> (0:w1503:i32)
                n746 = Multiply(x=w1503, y=w1502) -> (x*y=w1501:i32)
                n747 = Equal?(x=w1501, y=1) -> (x = y?=w1499:bool)
                n748 = case shown="False" w1499 {
                  frame False {
                    n749 = property on="Y Backlash corr" class="Bool (strict)"("Val(Sgnl)"=FALSE ("Value (Signaling)")) -> ()  [unwired: 2 in, 2 out]
                  }
                  frame True {
                    n750 = property on="Y Backlash corr" class="Bool (strict)"("Val(Sgnl)"=TRUE ("Value (Signaling)")) -> ()  [unwired: 2 in, 2 out]
                  }
                }
              }
              frame #2 {
                # "Velocity Setting"
                n751 = property on="Y Velocity SP step/sec" class="DigNum (strict)"() -> ("Value"=w1514:i32)  [unwired: 2 in, 2 out]
                n752 = Number To Decimal String(number=w1514) -> (decimal integer string=w1515:string)  [unwired: 1 in]
                n753 = call "mdrive send command.vi"("error in (no error)"=w1511, "Extra"=w1515, "Command"=T10."Max Velocity", "VISA resource name"=w1510) -> ("error out"=w1512:errorcluster, "VISA resource name out"=w1513:refnum<visa-resource-name>)  [unwired: 3 in, 1 out]
              }
              frame #3 {
                n754 = Wait (ms)(milliseconds to wait=u32 50) -> ()  [unwired: 1 out]
              }
              frame #4 {
                # "Move to Abs Position"
                n755 = Number To Decimal String(number=w1521) -> (decimal integer string=w1527:string)  [unwired: 1 in]
                n756 = call "mdrive send command.vi"("error in (no error)"=w1522, "Extra"=w1527, "Command"=T10."Move to Absolute Position", "VISA resource name"=w1523) -> ("error out"=w1524:errorcluster, "VISA resource name out"=w1525:refnum<visa-resource-name>)  [unwired: 3 in, 1 out]
              }
              frame #5 {
                n757 = Wait (ms)(milliseconds to wait=u32 25) -> ()  [unwired: 1 out]
              }
            }
          }
        }
        n758 = case shown="True" w1373 {
          tunnel: w1384 -> [w1391 w1396]
          tunnel: w1383 -> [w1392 w1395]
          tunnel: [w1392 w1394] -> w1362
          tunnel: [w1391 w1393] -> w1361
          frame False {
          }
          frame True {
            n759 = flat-sequence {
              tunnel: w1395 -> [w1423]
              tunnel: w1396 -> [w1424]
              tunnel: [w1424] -> w1410
              tunnel: [w1423] -> w1409
              tunnel: [w1411] -> w1408
              tunnel: [w1427] -> w1407
              tunnel: [w1426] -> w1406
              tunnel: [w1425] -> w1405
              tunnel: w1408 -> [w1425]
              tunnel: w1409 -> [w1426]
              tunnel: w1410 -> [w1427]
              tunnel: [w1443] -> w1404
              tunnel: [w1442] -> w1403
              tunnel: w1407 -> [w1441]
              tunnel: w1406 -> [w1440]
              tunnel: [w1439] -> w1402
              tunnel: w1405 -> [w1439]
              tunnel: w1404 -> [w1450]
              tunnel: [w1450] -> w1401
              tunnel: w1403 -> [w1449]
              tunnel: [w1449] -> w1400
              tunnel: w1402 -> [w1448]
              tunnel: [w1448] -> w1399
              tunnel: [w1455] -> w1398
              tunnel: [w1454] -> w1397
              tunnel: w1401 -> [w1453]
              tunnel: w1400 -> [w1452]
              tunnel: w1399 -> [w1451]
              tunnel: [w1460] -> w1394
              tunnel: w1398 -> [w1460]
              tunnel: w1397 -> [w1459]
              tunnel: [w1459] -> w1393
              frame #0 {
                n760 = property on="R steps/rev" class="DigNum (strict)"() -> ("Value"=w1419:u32)  [unwired: 2 in, 2 out]
                n761 = To Double Precision Float(number=w1419) -> (double precision float=w1416:dbl)
                n762 = property on="R offset deg" class="DigNum (strict)"() -> ("Value"=w1420:dbl)  [unwired: 2 in, 2 out]
                n763 = property on="R Position SP deg" class="DigNum (strict)"() -> ("Value"=w1421:dbl)  [unwired: 2 in, 2 out]
                n764 = Subtract(x=w1421, y=w1420) -> (x-y=w1413:dbl)
                n765 = property on="R deg/rev" class="DigNum (strict)"() -> ("Value"=w1422:dbl)  [unwired: 2 in, 2 out]
                n766 = Divide(x=w1413, y=w1422) -> (x/y=w1412:dbl)
                n767 = property on="R Step SP" class="DigNum (strict)"() -> ("Maximum"=w1417:dbl)  [unwired: 2 in, 2 out]
                n768 = Multiply(x=w1412, y=w1416) -> (x*y=w1414:dbl)
                n769 = property on="R Step SP" class="DigNum (strict)"() -> ("Minimum"=w1418:dbl)  [unwired: 2 in, 2 out]
                n770 = In Range and Coerce(upper limit=w1417, x=w1414, lower limit=w1418) -> (coerced(x)=w1415:dbl)  [unwired: 1 out]
                n771 = To Long Integer(number=w1415) -> (32bit integer=w1411:i32)
                n772 = property on="R Step SP" class="DigNum (strict)"("Val(Sgnl)"=w1411) -> ()  [unwired: 2 in, 2 out]
              }
              frame #1 {
                n773 = property on="R Step SP" class="DigNum (strict)"() -> ("Value"=w1436:i32)  [unwired: 2 in, 2 out]
                n774 = property on="R Step PV" class="DigNum (strict)"() -> ("Value"=w1435:i32)  [unwired: 2 in, 2 out]
                n775 = property on="R Backlash" class="DigNum (strict)"() -> ("Value"=w1428:i32)  [unwired: 2 in, 2 out]
                n776 = Subtract(x=w1436, y=w1435) -> (x-y=w1434:i32)
                n777 = Sign(1:w1428) -> (0:w1432:i32)
                n778 = Sign(1:w1434) -> (0:w1433:i32)
                n779 = Multiply(x=w1433, y=w1432) -> (x*y=w1431:i32)
                n780 = Equal?(x=w1431, y=1) -> (x = y?=w1429:bool)
                n781 = case shown="False" w1429 {
                  frame False {
                    n782 = property on="R Backlash corr" class="Bool (strict)"("Val(Sgnl)"=FALSE ("Value (Signaling)")) -> ()  [unwired: 2 in, 2 out]
                  }
                  frame True {
                    n783 = property on="R Backlash corr" class="Bool (strict)"("Val(Sgnl)"=TRUE ("Value (Signaling)")) -> ()  [unwired: 2 in, 2 out]
                  }
                }
              }
              frame #2 {
                # "Velocity Setting"
                n784 = property on="R Velocity SP step/sec" class="DigNum (strict)"() -> ("Value"=w1444:i32)  [unwired: 2 in, 2 out]
                n785 = Number To Decimal String(number=w1444) -> (decimal integer string=w1445:string)  [unwired: 1 in]
                n786 = call "mdrive send command.vi"("error in (no error)"=w1441, "Extra"=w1445, "Command"=T10."Max Velocity", "VISA resource name"=w1440) -> ("error out"=w1442:errorcluster, "VISA resource name out"=w1443:refnum<visa-resource-name>)  [unwired: 3 in, 1 out]
              }
              frame #3 {
                n787 = Wait (ms)(milliseconds to wait=u32 50) -> ()  [unwired: 1 out]
              }
              frame #4 {
                # "Move to Abs Position"
                n788 = Number To Decimal String(number=w1451) -> (decimal integer string=w1457:string)  [unwired: 1 in]
                n789 = call "mdrive send command.vi"("error in (no error)"=w1452, "Extra"=w1457, "Command"=T10."Move to Absolute Position", "VISA resource name"=w1453) -> ("error out"=w1454:errorcluster, "VISA resource name out"=w1455:refnum<visa-resource-name>)  [unwired: 3 in, 1 out]
              }
              frame #5 {
                n790 = Wait (ms)(milliseconds to wait=u32 25) -> ()  [unwired: 1 out]
              }
            }
          }
        }
      }
      event "HARDSTOP": Mouse Down {
        n791 = event-data() -> ()  [unwired: 1 in, 7 out]
        n792 = flat-sequence {
          tunnel: w1707 -> [w1736]
          tunnel: [w1735] -> w1702
          tunnel: w1686 -> [w1734]
          tunnel: [w1733] -> w1684
          tunnel: [w1740] -> w1703
          tunnel: w1702 -> [w1740]
          tunnel: [w1739] -> w1685
          tunnel: w1684 -> [w1739]
          tunnel: w1703 -> [w1757]
          tunnel: w1685 -> [w1754]
          tunnel: [w1753] -> _
          tunnel: [w1752] -> _
          frame #0 {
            n793 = call "mDrive Send Command.vi"("error in (no error)"=w1736, "Command"=T10."Stop", "VISA resource name"=w1734) -> ("error out"=w1735:errorcluster, "VISA resource name out"=w1733:refnum<visa-resource-name>)  [unwired: 4 in, 1 out]
          }
          frame #1 {
            n794 = Wait (ms)(milliseconds to wait=u32 50) -> ()  [unwired: 1 out]
          }
          frame #2 {
            n795 = property on="X steps/rev" class="DigNum (strict)"() -> ("Value"=w1743:u32)  [unwired: 2 in, 2 out]
            n796 = property on="X offset mm" class="DigNum (strict)"() -> ("Value"=w1741:dbl)  [unwired: 2 in, 2 out]
            n797 = To Double Precision Float(number=w1743) -> (double precision float=w1748:dbl)
            n798 = call "mDrive Send Command.vi"("error in (no error)"=w1757, "Extra"="P", "Command"=T10."Print Parameter", "VISA resource name"=w1754) -> ("error out"=w1752:errorcluster, "read buffer"=w1747:string, "VISA resource name out"=w1753:refnum<visa-resource-name>)  [unwired: 3 in]
            n799 = Decimal String To Number(string=w1747, offset=0) -> (number=w1745:i32)  [unwired: 1 in, 1 out]
            n800 = property on="X Step PV" class="DigNum (strict)"("Val(Sgnl)"=w1745) -> ()  [unwired: 2 in, 2 out]
            n801 = To Double Precision Float(number=w1745) -> (double precision float=w1749:dbl)
            n802 = Divide(x=w1749, y=w1748) -> (x/y=w1751:dbl)
            n803 = property on="X mm/rev" class="DigNum (strict)"() -> ("Value"=w1742:dbl)  [unwired: 2 in, 2 out]
            n804 = Multiply(x=w1751, y=w1742) -> (x*y=w1750:dbl)
            n805 = Add(x=w1750, y=w1741) -> (x+y=w1744:dbl)
            n806 = property on="X Position mm PV" class="DigNum (strict)"("Val(Sgnl)"=w1744) -> ()  [unwired: 2 in, 2 out]
          }
        }
        n807 = property on="GO" class="Bool"("DisabledEnum"=T9."Enabled" ("Disabled")) -> ()  [unwired: 2 in, 2 out]
        n808 = flat-sequence {
          tunnel: w1704 -> [w1711]
          tunnel: [w1710] -> w1696
          tunnel: w1695 -> [w1709]
          tunnel: [w1708] -> w1693
          tunnel: [w1715] -> w1697
          tunnel: w1696 -> [w1715]
          tunnel: [w1714] -> w1694
          tunnel: w1693 -> [w1714]
          tunnel: w1697 -> [w1732]
          tunnel: w1694 -> [w1729]
          tunnel: [w1728] -> _
          tunnel: [w1727] -> _
          frame #0 {
            n809 = call "mDrive Send Command.vi"("error in (no error)"=w1711, "Command"=T10."Stop", "VISA resource name"=w1709) -> ("error out"=w1710:errorcluster, "VISA resource name out"=w1708:refnum<visa-resource-name>)  [unwired: 4 in, 1 out]
          }
          frame #1 {
            n810 = Wait (ms)(milliseconds to wait=u32 50) -> ()  [unwired: 1 out]
          }
          frame #2 {
            n811 = property on="R steps/rev" class="DigNum (strict)"() -> ("Value"=w1720:u32)  [unwired: 2 in, 2 out]
            n812 = property on="R offset deg" class="DigNum (strict)"() -> ("Value"=w1717:dbl)  [unwired: 2 in, 2 out]
            n813 = To Double Precision Float(number=w1720) -> (double precision float=w1723:dbl)
            n814 = call "mDrive Send Command.vi"("error in (no error)"=w1732, "Extra"="P", "Command"=T10."Print Parameter", "VISA resource name"=w1729) -> ("error out"=w1727:errorcluster, "read buffer"=w1722:string, "VISA resource name out"=w1728:refnum<visa-resource-name>)  [unwired: 3 in]
            n815 = Decimal String To Number(string=w1722, offset=0) -> (number=w1719:i32)  [unwired: 1 in, 1 out]
            n816 = property on="R Step PV" class="DigNum (strict)"("Val(Sgnl)"=w1719) -> ()  [unwired: 2 in, 2 out]
            n817 = To Double Precision Float(number=w1719) -> (double precision float=w1724:dbl)
            n818 = Divide(x=w1724, y=w1723) -> (x/y=w1726:dbl)
            n819 = property on="R deg/rev" class="DigNum (strict)"() -> ("Value"=w1718:dbl)  [unwired: 2 in, 2 out]
            n820 = Multiply(x=w1726, y=w1718) -> (x*y=w1725:dbl)
            n821 = Add(x=w1725, y=w1717) -> (x+y=w1716:dbl)
            n822 = property on="R Position deg PV" class="DigNum (strict)"("Val(Sgnl)"=w1716) -> ()  [unwired: 2 in, 2 out]
          }
        }
        n823 = flat-sequence {
          tunnel: w1706 -> [w1761]
          tunnel: [w1760] -> w1700
          tunnel: w1689 -> [w1759]
          tunnel: [w1758] -> w1687
          tunnel: [w1765] -> w1701
          tunnel: w1700 -> [w1765]
          tunnel: [w1764] -> w1688
          tunnel: w1687 -> [w1764]
          tunnel: w1701 -> [w1782]
          tunnel: w1688 -> [w1779]
          tunnel: [w1778] -> _
          tunnel: [w1777] -> _
          frame #0 {
            n824 = call "mDrive Send Command.vi"("error in (no error)"=w1761, "Command"=T10."Stop", "VISA resource name"=w1759) -> ("error out"=w1760:errorcluster, "VISA resource name out"=w1758:refnum<visa-resource-name>)  [unwired: 4 in, 1 out]
          }
          frame #1 {
            n825 = Wait (ms)(milliseconds to wait=u32 50) -> ()  [unwired: 1 out]
          }
          frame #2 {
            n826 = property on="Z steps/rev" class="DigNum (strict)"() -> ("Value"=w1768:u32)  [unwired: 2 in, 2 out]
            n827 = property on="Z offset mm" class="DigNum (strict)"() -> ("Value"=w1766:dbl)  [unwired: 2 in, 2 out]
            n828 = To Double Precision Float(number=w1768) -> (double precision float=w1773:dbl)
            n829 = call "mDrive Send Command.vi"("error in (no error)"=w1782, "Extra"="P", "Command"=T10."Print Parameter", "VISA resource name"=w1779) -> ("error out"=w1777:errorcluster, "read buffer"=w1772:string, "VISA resource name out"=w1778:refnum<visa-resource-name>)  [unwired: 3 in]
            n830 = Decimal String To Number(string=w1772, offset=0) -> (number=w1770:i32)  [unwired: 1 in, 1 out]
            n831 = property on="Z Step PV" class="DigNum (strict)"("Val(Sgnl)"=w1770) -> ()  [unwired: 2 in, 2 out]
            n832 = To Double Precision Float(number=w1770) -> (double precision float=w1774:dbl)
            n833 = Divide(x=w1774, y=w1773) -> (x/y=w1776:dbl)
            n834 = property on="Z mm/rev" class="DigNum (strict)"() -> ("Value"=w1767:dbl)  [unwired: 2 in, 2 out]
            n835 = Multiply(x=w1776, y=w1767) -> (x*y=w1775:dbl)
            n836 = Add(x=w1775, y=w1766) -> (x+y=w1769:dbl)
            n837 = property on="Z Position mm PV" class="DigNum (strict)"("Val(Sgnl)"=w1769) -> ()  [unwired: 2 in, 2 out]
          }
        }
        n838 = flat-sequence {
          tunnel: w1705 -> [w1786]
          tunnel: [w1785] -> w1698
          tunnel: w1692 -> [w1784]
          tunnel: [w1783] -> w1690
          tunnel: [w1790] -> w1699
          tunnel: w1698 -> [w1790]
          tunnel: [w1789] -> w1691
          tunnel: w1690 -> [w1789]
          tunnel: w1699 -> [w1807]
          tunnel: w1691 -> [w1804]
          tunnel: [w1803] -> _
          tunnel: [w1802] -> _
          frame #0 {
            n839 = call "mDrive Send Command.vi"("error in (no error)"=w1786, "Command"=T10."Stop", "VISA resource name"=w1784) -> ("error out"=w1785:errorcluster, "VISA resource name out"=w1783:refnum<visa-resource-name>)  [unwired: 4 in, 1 out]
          }
          frame #1 {
            n840 = Wait (ms)(milliseconds to wait=u32 50) -> ()  [unwired: 1 out]
          }
          frame #2 {
            n841 = property on="Y steps/rev" class="DigNum (strict)"() -> ("Value"=w1793:u32)  [unwired: 2 in, 2 out]
            n842 = property on="Y offset mm" class="DigNum (strict)"() -> ("Value"=w1791:dbl)  [unwired: 2 in, 2 out]
            n843 = To Double Precision Float(number=w1793) -> (double precision float=w1798:dbl)
            n844 = call "mDrive Send Command.vi"("error in (no error)"=w1807, "Extra"="P", "Command"=T10."Print Parameter", "VISA resource name"=w1804) -> ("error out"=w1802:errorcluster, "read buffer"=w1797:string, "VISA resource name out"=w1803:refnum<visa-resource-name>)  [unwired: 3 in]
            n845 = Decimal String To Number(string=w1797, offset=0) -> (number=w1794:i32)  [unwired: 1 in, 1 out]
            n846 = property on="Y Step PV" class="DigNum (strict)"("Val(Sgnl)"=w1794) -> ()  [unwired: 2 in, 2 out]
            n847 = To Double Precision Float(number=w1794) -> (double precision float=w1799:dbl)
            n848 = Divide(x=w1799, y=w1798) -> (x/y=w1801:dbl)
            n849 = property on="Y mm/rev" class="DigNum (strict)"() -> ("Value"=w1792:dbl)  [unwired: 2 in, 2 out]
            n850 = Multiply(x=w1801, y=w1792) -> (x*y=w1800:dbl)
            n851 = Add(x=w1800, y=w1791) -> (x+y=w1795:dbl)
            n852 = property on="Y Position mm PV" class="DigNum (strict)"("Val(Sgnl)"=w1795) -> ()  [unwired: 2 in, 2 out]
          }
        }
      }
      event "Reset Y Position mm", "Reset X Position mm", "Reset Z Position mm", "Reset R Position deg": Value Change {
        n853 = event-data() -> ()  [unwired: 1 in, 5 out]
        n854 = property on="Y steps/rev" class="DigNum (strict)"() -> ("Value"=w1838:u32)  [unwired: 2 in, 2 out]
        n855 = property on="X steps/rev" class="DigNum (strict)"() -> ("Value"=w1829:u32)  [unwired: 2 in, 2 out]
        n856 = property on="Z steps/rev" class="DigNum (strict)"() -> ("Value"=w1820:u32)  [unwired: 2 in, 2 out]
        n857 = property on="R steps/rev" class="DigNum (strict)"() -> ("Value"=w1811:u32)  [unwired: 2 in, 2 out]
        n858 = property on="R offset deg" class="DigNum (strict)"() -> ("Value"=w1809:dbl)  [unwired: 2 in, 2 out]
        n859 = property on="Y offset mm" class="DigNum (strict)"() -> ("Value"=w1836:dbl)  [unwired: 2 in, 2 out]
        n860 = property on="X offset mm" class="DigNum (strict)"() -> ("Value"=w1827:dbl)  [unwired: 2 in, 2 out]
        n861 = property on="Z offset mm" class="DigNum (strict)"() -> ("Value"=w1818:dbl)  [unwired: 2 in, 2 out]
        n862 = To Double Precision Float(number=w1811) -> (double precision float=w1814:dbl)
        n863 = To Double Precision Float(number=w1829) -> (double precision float=w1832:dbl)
        n864 = To Double Precision Float(number=w1820) -> (double precision float=w1823:dbl)
        n865 = property on="Reset Y Position mm" class="DigNum (strict)"() -> ("Value"=w1844:dbl)  [unwired: 2 in, 2 out]
        n866 = property on="Reset X Position mm" class="DigNum (strict)"() -> ("Value"=w1835:dbl)  [unwired: 2 in, 2 out]
        n867 = property on="Reset Z Position mm" class="DigNum (strict)"() -> ("Value"=w1826:dbl)  [unwired: 2 in, 2 out]
        n868 = property on="Reset R Position deg" class="DigNum (strict)"() -> ("Value"=w1817:dbl)  [unwired: 2 in, 2 out]
        n869 = local write "STATUS"("RESSETTING" ("STATUS")) -> ()
        n870 = Subtract(x=w1844, y=w1836) -> (x-y=w1843:dbl)
        n871 = Subtract(x=w1817, y=w1809) -> (x-y=w1816:dbl)
        n872 = Subtract(x=w1835, y=w1827) -> (x-y=w1834:dbl)
        n873 = Subtract(x=w1826, y=w1818) -> (x-y=w1825:dbl)
        n874 = property on="Y mm/rev" class="DigNum (strict)"() -> ("Value"=w1837:dbl)  [unwired: 2 in, 2 out]
        n875 = property on="X mm/rev" class="DigNum (strict)"() -> ("Value"=w1828:dbl)  [unwired: 2 in, 2 out]
        n876 = property on="Z mm/rev" class="DigNum (strict)"() -> ("Value"=w1819:dbl)  [unwired: 2 in, 2 out]
        n877 = property on="R deg/rev" class="DigNum (strict)"() -> ("Value"=w1810:dbl)  [unwired: 2 in, 2 out]
        n878 = Divide(x=w1816, y=w1810) -> (x/y=w1815:dbl)
        n879 = Divide(x=w1834, y=w1828) -> (x/y=w1833:dbl)
        n880 = Divide(x=w1825, y=w1819) -> (x/y=w1824:dbl)
        n881 = Divide(x=w1843, y=w1837) -> (x/y=w1842:dbl)
        n882 = To Double Precision Float(number=w1838) -> (double precision float=w1841:dbl)
        n883 = Multiply(x=w1842, y=w1841) -> (x*y=w1840:dbl)
        n884 = Multiply(x=w1815, y=w1814) -> (x*y=w1813:dbl)
        n885 = Multiply(x=w1833, y=w1832) -> (x*y=w1831:dbl)
        n886 = Multiply(x=w1824, y=w1823) -> (x*y=w1822:dbl)
        n887 = To Long Integer(number=w1840) -> (32bit integer=w1839:i32)
        n888 = To Long Integer(number=w1813) -> (32bit integer=w1812:i32)
        n889 = To Long Integer(number=w1831) -> (32bit integer=w1830:i32)
        n890 = To Long Integer(number=w1822) -> (32bit integer=w1821:i32)
        n891 = property on="Reset Y Motor Steps" class="DigNum (strict)"("Val(Sgnl)"=w1839) -> ()  [unwired: 2 in, 2 out]
        n892 = property on="Reset R Motor Steps" class="DigNum (strict)"("Val(Sgnl)"=w1812) -> ()  [unwired: 2 in, 2 out]
        n893 = property on="Reset X Motor Steps" class="DigNum (strict)"("Val(Sgnl)"=w1830) -> ()  [unwired: 2 in, 2 out]
        n894 = property on="Reset Z Motor Steps" class="DigNum (strict)"("Val(Sgnl)"=w1821) -> ()  [unwired: 2 in, 2 out]
      }
      event "Y Velocity SP step/sec", "X Velocity SP step/sec", "R Velocity SP step/sec", "Z Velocity SP step/sec", "Y Step SP", "X Step SP", "Z Step SP", "R Step SP": Value Change {
        n895 = event-data() -> ()  [unwired: 1 in, 5 out]
        n896 = property on="X Step SP" class="DigNum (strict)"() -> ("Value"=w1869:i32)  [unwired: 2 in, 2 out]
        n897 = property on="Z Step SP" class="DigNum (strict)"() -> ("Value"=w1861:i32)  [unwired: 2 in, 2 out]
        n898 = property on="Y Step SP" class="DigNum (strict)"() -> ("Value"=w1877:i32)  [unwired: 2 in, 2 out]
        n899 = property on="X steps/rev" class="DigNum (strict)"() -> ("Value"=w1894:u32)  [unwired: 2 in, 2 out]
        n900 = property on="X steps/rev" class="DigNum (strict)"() -> ("Value"=w1867:u32)  [unwired: 2 in, 2 out]
        n901 = property on="R Step SP" class="DigNum (strict)"() -> ("Value"=w1853:i32)  [unwired: 2 in, 2 out]
        n902 = property on="Z steps/rev" class="DigNum (strict)"() -> ("Value"=w1888:u32)  [unwired: 2 in, 2 out]
        n903 = property on="Z steps/rev" class="DigNum (strict)"() -> ("Value"=w1859:u32)  [unwired: 2 in, 2 out]
        n904 = property on="Y steps/rev" class="DigNum (strict)"() -> ("Value"=w1900:u32)  [unwired: 2 in, 2 out]
        n905 = property on="Y steps/rev" class="DigNum (strict)"() -> ("Value"=w1875:u32)  [unwired: 2 in, 2 out]
        n906 = property on="R steps/rev" class="DigNum (strict)"() -> ("Value"=w1882:u32)  [unwired: 2 in, 2 out]
        n907 = property on="R steps/rev" class="DigNum (strict)"() -> ("Value"=w1851:u32)  [unwired: 2 in, 2 out]
        n908 = property on="R offset deg" class="DigNum (strict)"() -> ("Value"=w1850:dbl)  [unwired: 2 in, 2 out]
        n909 = property on="X offset mm" class="DigNum (strict)"() -> ("Value"=w1866:dbl)  [unwired: 2 in, 2 out]
        n910 = property on="Z offset mm" class="DigNum (strict)"() -> ("Value"=w1858:dbl)  [unwired: 2 in, 2 out]
        n911 = property on="Y offset mm" class="DigNum (strict)"() -> ("Value"=w1874:dbl)  [unwired: 2 in, 2 out]
        n912 = To Double Precision Float(number=w1894) -> (double precision float=w1899:dbl)
        n913 = To Double Precision Float(number=w1869) -> (double precision float=w1870:dbl)
        n914 = To Double Precision Float(number=w1867) -> (double precision float=w1873:dbl)
        n915 = To Double Precision Float(number=w1882) -> (double precision float=w1887:dbl)
        n916 = To Double Precision Float(number=w1853) -> (double precision float=w1854:dbl)
        n917 = To Double Precision Float(number=w1851) -> (double precision float=w1857:dbl)
        n918 = To Double Precision Float(number=w1888) -> (double precision float=w1893:dbl)
        n919 = To Double Precision Float(number=w1861) -> (double precision float=w1862:dbl)
        n920 = To Double Precision Float(number=w1859) -> (double precision float=w1865:dbl)
        n921 = To Double Precision Float(number=w1900) -> (double precision float=w1905:dbl)
        n922 = To Double Precision Float(number=w1877) -> (double precision float=w1878:dbl)
        n923 = To Double Precision Float(number=w1875) -> (double precision float=w1881:dbl)
        n924 = Divide(x=w1870, y=w1873) -> (x/y=w1872:dbl)
        n925 = Divide(x=w1862, y=w1865) -> (x/y=w1864:dbl)
        n926 = Divide(x=w1878, y=w1881) -> (x/y=w1880:dbl)
        n927 = Divide(x=w1854, y=w1857) -> (x/y=w1856:dbl)
        n928 = property on="X Velocity SP step/sec" class="DigNum (strict)"() -> ("Value"=w1896:i32)  [unwired: 2 in, 2 out]
        n929 = property on="X mm/rev" class="DigNum (strict)"() -> ("Value"=w1847:dbl)  [unwired: 2 in, 2 out]
        n930 = property on="Z Velocity SP step/sec" class="DigNum (strict)"() -> ("Value"=w1890:i32)  [unwired: 2 in, 2 out]
        n931 = property on="Z mm/rev" class="DigNum (strict)"() -> ("Value"=w1848:dbl)  [unwired: 2 in, 2 out]
        n932 = property on="Y Velocity SP step/sec" class="DigNum (strict)"() -> ("Value"=w1902:i32)  [unwired: 2 in, 2 out]
        n933 = property on="Y mm/rev" class="DigNum (strict)"() -> ("Value"=w1846:dbl)  [unwired: 2 in, 2 out]
        n934 = property on="R Velocity SP step/sec" class="DigNum (strict)"() -> ("Value"=w1884:i32)  [unwired: 2 in, 2 out]
        n935 = property on="R deg/rev" class="DigNum (strict)"() -> ("Value"=w1849:dbl)  [unwired: 2 in, 2 out]
        n936 = Multiply(x=w1872, y=w1847) -> (x*y=w1871:dbl)
        n937 = Multiply(x=w1856, y=w1849) -> (x*y=w1855:dbl)
        n938 = Multiply(x=w1864, y=w1848) -> (x*y=w1863:dbl)
        n939 = Multiply(x=w1880, y=w1846) -> (x*y=w1879:dbl)
        n940 = To Double Precision Float(number=w1896) -> (double precision float=w1897:dbl)
        n941 = To Double Precision Float(number=w1884) -> (double precision float=w1885:dbl)
        n942 = To Double Precision Float(number=w1890) -> (double precision float=w1891:dbl)
        n943 = To Double Precision Float(number=w1902) -> (double precision float=w1903:dbl)
        n944 = Divide(x=w1897, y=w1899) -> (x/y=w1898:dbl)
        n945 = Add(x=w1871, y=w1866) -> (x+y=w1868:dbl)
        n946 = Divide(x=w1885, y=w1887) -> (x/y=w1886:dbl)
        n947 = Add(x=w1855, y=w1850) -> (x+y=w1852:dbl)
        n948 = Divide(x=w1891, y=w1893) -> (x/y=w1892:dbl)
        n949 = Add(x=w1863, y=w1858) -> (x+y=w1860:dbl)
        n950 = Divide(x=w1903, y=w1905) -> (x/y=w1904:dbl)
        n951 = Add(x=w1879, y=w1874) -> (x+y=w1876:dbl)
        n952 = Multiply(x=w1898, y=w1847) -> (x*y=w1895:dbl)
        n953 = Multiply(x=w1886, y=w1849) -> (x*y=w1883:dbl)
        n954 = Multiply(x=w1892, y=w1848) -> (x*y=w1889:dbl)
        n955 = Multiply(x=w1904, y=w1846) -> (x*y=w1901:dbl)
        n956 = property on="X Position MV mm" class="DigNum (strict)"("Val(Sgnl)"=w1868) -> ()  [unwired: 2 in, 2 out]
        n957 = property on="R Position MV deg" class="DigNum (strict)"("Val(Sgnl)"=w1852) -> ()  [unwired: 2 in, 2 out]
        n958 = property on="Z Position MV mm" class="DigNum (strict)"("Val(Sgnl)"=w1860) -> ()  [unwired: 2 in, 2 out]
        n959 = property on="Y Position MV mm" class="DigNum (strict)"("Val(Sgnl)"=w1876) -> ()  [unwired: 2 in, 2 out]
        n960 = property on="X Velocity MV mm/sec" class="DigNum (strict)"("Val(Sgnl)"=w1895) -> ()  [unwired: 2 in, 2 out]
        n961 = property on="Z Velocity MV mm/sec" class="DigNum (strict)"("Val(Sgnl)"=w1889) -> ()  [unwired: 2 in, 2 out]
        n962 = property on="Y Velocity MV mm/sec" class="DigNum (strict)"("Val(Sgnl)"=w1901) -> ()  [unwired: 2 in, 2 out]
        n963 = Absolute Value(x=w1883) -> (abs(x)=w1845:dbl)
        n964 = property on="R Velocity MVdeg/sec" class="DigNum (strict)"("Val(Sgnl)"=w1845) -> ()  [unwired: 2 in, 2 out]
      }
      event "Y Scan Length SP steps", "Y Scan Velocity SP steps/sec", "X Scan Velocity SP steps/sec", "X Scan Length SP steps", "Z Scan Velocity SP steps/sec", "Z Scan Length SP steps", "R Scan Velocity SP steps/sec", "R Scan Length SP steps": Value Change {
        n965 = event-data() -> ()  [unwired: 1 in, 5 out]
        n966 = property on="R Step PV" class="DigNum (strict)"() -> ("Value"=w1938:i32)  [unwired: 2 in, 2 out]
        n967 = property on="X steps/rev" class="DigNum (strict)"() -> ("Value"=w1979:u32)  [unwired: 2 in, 2 out]
        n968 = property on="Y steps/rev" class="DigNum (strict)"() -> ("Value"=w1967:u32)  [unwired: 2 in, 2 out]
        n969 = property on="Z steps/rev" class="DigNum (strict)"() -> ("Value"=w1954:u32)  [unwired: 2 in, 2 out]
        n970 = property on="X Step PV" class="DigNum (strict)"() -> ("Value"=w1978:i32)  [unwired: 2 in, 2 out]
        n971 = property on="Y Step PV" class="DigNum (strict)"() -> ("Value"=w1965:i32)  [unwired: 2 in, 2 out]
        n972 = property on="Z Step PV" class="DigNum (strict)"() -> ("Value"=w1952:i32)  [unwired: 2 in, 2 out]
        n973 = property on="R steps/rev" class="DigNum (strict)"() -> ("Value"=w1940:u32)  [unwired: 2 in, 2 out]
        n974 = To Double Precision Float(number=w1978) -> (double precision float=w1932:dbl)
        n975 = To Double Precision Float(number=w1965) -> (double precision float=w1931:dbl)
        n976 = To Double Precision Float(number=w1952) -> (double precision float=w1930:dbl)
        n977 = To Double Precision Float(number=w1938) -> (double precision float=w1929:dbl)
        n978 = To Double Precision Float(number=w1979) -> (double precision float=w1977:dbl)
        n979 = To Double Precision Float(number=w1967) -> (double precision float=w1922:dbl)
        n980 = To Double Precision Float(number=w1940) -> (double precision float=w1937:dbl)
        n981 = To Double Precision Float(number=w1954) -> (double precision float=w1951:dbl)
        n982 = property on="X Step SP" class="DigNum (strict)"() -> ("Maximum"=w1982:dbl)  [unwired: 2 in, 2 out]
        n983 = property on="Y Step SP" class="DigNum (strict)"() -> ("Maximum"=w1971:dbl)  [unwired: 2 in, 2 out]
        n984 = property on="Z Step SP" class="DigNum (strict)"() -> ("Maximum"=w1958:dbl)  [unwired: 2 in, 2 out]
        n985 = property on="R Step SP" class="DigNum (strict)"() -> ("Maximum"=w1946:dbl)  [unwired: 2 in, 2 out]
        n986 = property on="X Scan Length SP steps" class="DigNum (strict)"() -> ("Value"=w1976:i32)  [unwired: 2 in, 2 out]
        n987 = property on="X Scan Length SP mm" class="DigNum (strict)"() -> ("Value"=w1908:dbl)  [unwired: 2 in, 2 out]
        n988 = property on="Y Scan Length SP mm" class="DigNum (strict)"() -> ("Value"=w1909:dbl)  [unwired: 2 in, 2 out]
        n989 = property on="Y Scan Length SP steps" class="DigNum (strict)"() -> ("Value"=w1968:i32)  [unwired: 2 in, 2 out]
        n990 = property on="Z Scan Length SP steps" class="DigNum (strict)"() -> ("Value"=w1955:i32)  [unwired: 2 in, 2 out]
        n991 = property on="R Scan Length SP steps" class="DigNum (strict)"() -> ("Value"=w1941:i32)  [unwired: 2 in, 2 out]
        n992 = property on="X Step SP" class="DigNum (strict)"() -> ("Minimum"=w1983:dbl)  [unwired: 2 in, 2 out]
        n993 = property on="Y Step SP" class="DigNum (strict)"() -> ("Minimum"=w1972:dbl)  [unwired: 2 in, 2 out]
        n994 = property on="Z Step SP" class="DigNum (strict)"() -> ("Minimum"=w1959:dbl)  [unwired: 2 in, 2 out]
        n995 = property on="R Step SP" class="DigNum (strict)"() -> ("Minimum"=w1943:dbl)  [unwired: 2 in, 2 out]
        n996 = property on="Z Scan Velocity SP steps/sec" class="DigNum (strict)"() -> ("Value"=w1950:i32)  [unwired: 2 in, 2 out]
        n997 = property on="R Scan Velocity SP steps/sec" class="DigNum (strict)"() -> ("Value"=w1936:i32)  [unwired: 2 in, 2 out]
        n998 = Subtract(x=w1982, y=w1932) -> (x-y=w1981:dbl)
        n999 = Subtract(x=w1983, y=w1932) -> (x-y=w1984:dbl)
        n1000 = Subtract(x=w1972, y=w1931) -> (x-y=w1973:dbl)
        n1001 = Subtract(x=w1971, y=w1931) -> (x-y=w1970:dbl)
        n1002 = Subtract(x=w1959, y=w1930) -> (x-y=w1960:dbl)
        n1003 = Subtract(x=w1958, y=w1930) -> (x-y=w1957:dbl)
        n1004 = Subtract(x=w1943, y=w1929) -> (x-y=w1944:dbl)
        n1005 = Subtract(x=w1946, y=w1929) -> (x-y=w1945:dbl)
        n1006 = To Double Precision Float(number=w1941) -> (double precision float=w1926:dbl)
        n1007 = To Double Precision Float(number=w1955) -> (double precision float=w1928:dbl)
        n1008 = To Double Precision Float(number=w1976) -> (double precision float=w1919:dbl)
        n1009 = To Double Precision Float(number=w1968) -> (double precision float=w1921:dbl)
        n1010 = property on="X Scan Velocity SP steps/sec" class="DigNum (strict)"() -> ("Value"=w1980:i32)  [unwired: 2 in, 2 out]
        n1011 = property on="Y Scan Velocity SP steps/sec" class="DigNum (strict)"() -> ("Value"=w1964:i32)  [unwired: 2 in, 2 out]
        n1012 = Equal?(x=w1908, y=0.0) -> (x = y?=w1906:bool)
        n1013 = Equal?(x=w1909, y=0.0) -> (x = y?=w1907:bool)
        n1014 = property on="X Scan Length SP steps" class="DigNum (strict)"("Maximum"=w1981) -> ()  [unwired: 2 in, 2 out]
        n1015 = property on="X Scan Length SP steps" class="DigNum (strict)"("Minimum"=w1984) -> ()  [unwired: 2 in, 2 out]
        n1016 = property on="Y Scan Length SP steps" class="DigNum (strict)"("Minimum"=w1973) -> ()  [unwired: 2 in, 2 out]
        n1017 = property on="Y Scan Length SP steps" class="DigNum (strict)"("Maximum"=w1970) -> ()  [unwired: 2 in, 2 out]
        n1018 = property on="Z Scan Length SP steps" class="DigNum (strict)"("Minimum"=w1960) -> ()  [unwired: 2 in, 2 out]
        n1019 = property on="Z Scan Length SP steps" class="DigNum (strict)"("Maximum"=w1957) -> ()  [unwired: 2 in, 2 out]
        n1020 = property on="R Scan Length SP steps" class="DigNum (strict)"("Minimum"=w1944) -> ()  [unwired: 2 in, 2 out]
        n1021 = property on="R Scan Length SP steps" class="DigNum (strict)"("Maximum"=w1945) -> ()  [unwired: 2 in, 2 out]
        n1022 = Divide(x=w1919, y=w1977) -> (x/y=w1914:dbl)
        n1023 = Divide(x=w1921, y=w1922) -> (x/y=w1969:dbl)
        n1024 = Divide(x=w1928, y=w1951) -> (x/y=w1956:dbl)
        n1025 = Divide(x=w1926, y=w1937) -> (x/y=w1942:dbl)
        n1026 = To Double Precision Float(number=w1980) -> (double precision float=w1918:dbl)
        n1027 = To Double Precision Float(number=w1964) -> (double precision float=w1920:dbl)
        n1028 = To Double Precision Float(number=w1950) -> (double precision float=w1927:dbl)
        n1029 = To Double Precision Float(number=w1936) -> (double precision float=w1925:dbl)
        n1030 = property on="X mm/rev" class="DigNum (strict)"() -> ("Value"=w1913:dbl)  [unwired: 2 in, 2 out]
        n1031 = property on="Y mm/rev" class="DigNum (strict)"() -> ("Value"=w1966:dbl)  [unwired: 2 in, 2 out]
        n1032 = property on="Z mm/rev" class="DigNum (strict)"() -> ("Value"=w1953:dbl)  [unwired: 2 in, 2 out]
        n1033 = property on="R deg/rev" class="DigNum (strict)"() -> ("Value"=w1939:dbl)  [unwired: 2 in, 2 out]
        n1034 = Multiply(x=w1914, y=w1913) -> (x*y=w1974:dbl)
        n1035 = Divide(x=w1918, y=w1977) -> (x/y=w1912:dbl)
        n1036 = Multiply(x=w1969, y=w1966) -> (x*y=w1962:dbl)
        n1037 = Divide(x=w1920, y=w1922) -> (x/y=w1963:dbl)
        n1038 = Divide(x=w1926, y=w1925) -> (x/y=w1924:dbl)
        n1039 = Multiply(x=w1942, y=w1939) -> (x*y=w1934:dbl)
        n1040 = Divide(x=w1925, y=w1937) -> (x/y=w1935:dbl)
        n1041 = Multiply(x=w1956, y=w1953) -> (x*y=w1948:dbl)
        n1042 = Divide(x=w1928, y=w1927) -> (x/y=w1923:dbl)
        n1043 = Divide(x=w1927, y=w1951) -> (x/y=w1949:dbl)
        n1044 = case shown="True" w1906 {
          tunnel: w1919 -> [w1987 _]
          tunnel: w1918 -> [w1986 _]
          frame False {
            n1045 = Divide(x=w1987, y=w1986) -> (x/y=w1988:dbl)
            n1046 = Absolute Value(x=w1988) -> (abs(x)=→"X Scan Duration":dbl)
          }
          frame True {
            n1047 = local write "X Scan Duration"(0.0 ("X Scan Duration")) -> ()
          }
        }
        n1048 = case shown="True" w1907 {
          tunnel: w1921 -> [w1993 _]
          tunnel: w1920 -> [w1992 _]
          frame False {
            n1049 = Divide(x=w1993, y=w1992) -> (x/y=w1991:dbl)
            n1050 = Absolute Value(x=w1991) -> (abs(x)=→"Y Scan Duration":dbl)
          }
          frame True {
            n1051 = local write "Y Scan Duration"(0.0 ("Y Scan Duration")) -> ()
          }
        }
        n1052 = Multiply(x=w1913, y=w1912) -> (x*y=w1975:dbl)
        n1053 = Multiply(x=w1966, y=w1963) -> (x*y=w1961:dbl)
        n1054 = Multiply(x=w1939, y=w1935) -> (x*y=w1933:dbl)
        n1055 = Multiply(x=w1953, y=w1949) -> (x*y=w1947:dbl)
        n1056 = Absolute Value(x=w1924) -> (abs(x)=→"R Scan Duration":dbl)
        n1057 = Absolute Value(x=w1923) -> (abs(x)=→"Z Scan Duration":dbl)
        n1058 = property on="X Scan length MV mm" class="DigNum (strict)"("Val(Sgnl)"=w1974) -> ()  [unwired: 2 in, 2 out]
        n1059 = property on="Y Scan length MV mm" class="DigNum (strict)"("Value"=w1962) -> ()  [unwired: 2 in, 2 out]
        n1060 = property on="R Scan length MV deg" class="DigNum (strict)"("Value"=w1934) -> ()  [unwired: 2 in, 2 out]
        n1061 = property on="Z Scan length MV mm" class="DigNum (strict)"("Value"=w1948) -> ()  [unwired: 2 in, 2 out]
        n1062 = Absolute Value(x=w1933) -> (abs(x)=w1917:dbl)
        n1063 = property on="X Scan velocity MV mm/sec" class="DigNum (strict)"("Value"=w1975) -> ()  [unwired: 2 in, 2 out]
        n1064 = property on="Y Scan velocity MV mm/sec" class="DigNum (strict)"("Val(Sgnl)"=w1961) -> ()  [unwired: 2 in, 2 out]
        n1065 = property on="Z Scan velocity MV mm/sec" class="DigNum (strict)"("Val(Sgnl)"=w1947) -> ()  [unwired: 2 in, 2 out]
        n1066 = property on="R Scan Velocity SP deg/sec" class="DigNum (strict)"("Val(Sgnl)"=w1917) -> ()  [unwired: 2 in, 2 out]
      }
      event "Y Move Set": Mouse Down {
        n1067 = event-data() -> ()  [unwired: 1 in, 7 out]
        n1068 = property on="Y steps/rev" class="DigNum (strict)"() -> ("Value"=w2013:u32)  [unwired: 2 in, 2 out]
        n1069 = Wait (ms)(milliseconds to wait=u32 100) -> ()  [unwired: 1 out]
        n1070 = To Double Precision Float(number=w2013) -> (double precision float=w1998:dbl)
        n1071 = property on="Y offset mm" class="DigNum (strict)"() -> ("Value"=w2011:dbl)  [unwired: 2 in, 2 out]
        n1072 = property on="Y Position SP mm" class="DigNum (strict)"() -> ("Value"=w2010:dbl)  [unwired: 2 in, 2 out]
        n1073 = local write "STATUS"("SETTING Y" ("STATUS")) -> ()
        n1074 = property on="Y Velocity SP step/sec" class="DigNum (strict)"() -> ("Maximum"=w2000:dbl)  [unwired: 2 in, 2 out]
        n1075 = property on="Y Velocity SP step/sec" class="DigNum (strict)"() -> ("Minimum"=w1999:dbl)  [unwired: 2 in, 2 out]
        n1076 = Subtract(x=w2010, y=w2011) -> (x-y=w2014:dbl)
        n1077 = property on="Y Velocity SP mm/sec" class="DigNum (strict)"() -> ("Value"=w2004:dbl)  [unwired: 2 in, 2 out]
        n1078 = property on="Y mm/rev" class="DigNum (strict)"() -> ("Value"=w1997:dbl)  [unwired: 2 in, 2 out]
        n1079 = Divide(x=w2014, y=w1997) -> (x/y=w2015:dbl)
        n1080 = Divide(x=w2004, y=w1997) -> (x/y=w2005:dbl)
        n1081 = Multiply(x=w2015, y=w1998) -> (x*y=w2009:dbl)
        n1082 = Multiply(x=w2005, y=w1998) -> (x*y=w2002:dbl)
        n1083 = In Range and Coerce(upper limit=w2000, x=w2002, lower limit=w1999) -> (coerced(x)=w2001:dbl)  [unwired: 1 out]
        n1084 = property on="Y Step SP" class="DigNum (strict)"() -> ("Maximum"=w2007:dbl)  [unwired: 2 in, 2 out]
        n1085 = property on="Y Step SP" class="DigNum (strict)"() -> ("Minimum"=w2006:dbl)  [unwired: 2 in, 2 out]
        n1086 = To Long Integer(number=w2001) -> (32bit integer=w2003:i32)
        n1087 = In Range and Coerce(upper limit=w2007, x=w2009, lower limit=w2006) -> (coerced(x)=w2008:dbl)  [unwired: 1 out]
        n1088 = To Long Integer(number=w2008) -> (32bit integer=w2012:i32)
        n1089 = property on="Y Velocity SP step/sec" class="DigNum (strict)"("Val(Sgnl)"=w2003) -> ()  [unwired: 2 in, 2 out]
        n1090 = property on="Y Step SP" class="DigNum (strict)"("Val(Sgnl)"=w2012) -> ()  [unwired: 2 in, 2 out]
      }
      event "X Move Set": Mouse Down {
        n1091 = event-data() -> ()  [unwired: 1 in, 7 out]
        n1092 = property on="X steps/rev" class="DigNum (strict)"() -> ("Value"=w2034:u32)  [unwired: 2 in, 2 out]
        n1093 = Wait (ms)(milliseconds to wait=u32 100) -> ()  [unwired: 1 out]
        n1094 = property on="X offset mm" class="DigNum (strict)"() -> ("Value"=w2032:dbl)  [unwired: 2 in, 2 out]
        n1095 = property on="X Position SP mm" class="DigNum (strict)"() -> ("Value"=w2031:dbl)  [unwired: 2 in, 2 out]
        n1096 = local write "STATUS"("SETTING X" ("STATUS")) -> ()
        n1097 = property on="X Velocity SP step/sec" class="DigNum (strict)"() -> ("Maximum"=w2021:dbl)  [unwired: 2 in, 2 out]
        n1098 = property on="X Velocity SP step/sec" class="DigNum (strict)"() -> ("Minimum"=w2020:dbl)  [unwired: 2 in, 2 out]
        n1099 = Subtract(x=w2031, y=w2032) -> (x-y=w2035:dbl)
        n1100 = property on="X Velocity SP mm/sec" class="DigNum (strict)"() -> ("Value"=w2025:dbl)  [unwired: 2 in, 2 out]
        n1101 = property on="X mm/rev" class="DigNum (strict)"() -> ("Value"=w2018:dbl)  [unwired: 2 in, 2 out]
        n1102 = Divide(x=w2035, y=w2018) -> (x/y=w2036:dbl)
        n1103 = Divide(x=w2025, y=w2018) -> (x/y=w2026:dbl)
        n1104 = To Double Precision Float(number=w2034) -> (double precision float=w2019:dbl)
        n1105 = Multiply(x=w2036, y=w2019) -> (x*y=w2030:dbl)
        n1106 = Multiply(x=w2026, y=w2019) -> (x*y=w2023:dbl)
        n1107 = In Range and Coerce(upper limit=w2021, x=w2023, lower limit=w2020) -> (coerced(x)=w2022:dbl)  [unwired: 1 out]
        n1108 = property on="X Step SP" class="DigNum (strict)"() -> ("Maximum"=w2028:dbl)  [unwired: 2 in, 2 out]
        n1109 = property on="X Step SP" class="DigNum (strict)"() -> ("Minimum"=w2027:dbl)  [unwired: 2 in, 2 out]
        n1110 = To Long Integer(number=w2022) -> (32bit integer=w2024:i32)
        n1111 = In Range and Coerce(upper limit=w2028, x=w2030, lower limit=w2027) -> (coerced(x)=w2029:dbl)  [unwired: 1 out]
        n1112 = To Long Integer(number=w2029) -> (32bit integer=w2033:i32)
        n1113 = property on="X Velocity SP step/sec" class="DigNum (strict)"("Val(Sgnl)"=w2024) -> ()  [unwired: 2 in, 2 out]
        n1114 = property on="X Step SP" class="DigNum (strict)"("Val(Sgnl)"=w2033) -> ()  [unwired: 2 in, 2 out]
      }
      event "Z Move Set": Mouse Down {
        n1115 = event-data() -> ()  [unwired: 1 in, 7 out]
        n1116 = property on="Z steps/rev" class="DigNum (strict)"() -> ("Value"=w2053:u32)  [unwired: 2 in, 2 out]
        n1117 = Wait (ms)(milliseconds to wait=u32 100) -> ()  [unwired: 1 out]
        n1118 = property on="Z offset mm" class="DigNum (strict)"() -> ("Value"=w2051:dbl)  [unwired: 2 in, 2 out]
        n1119 = property on="Z Position SP mm" class="DigNum (strict)"() -> ("Value"=w2050:dbl)  [unwired: 2 in, 2 out]
        n1120 = local write "STATUS"("SETTING Z" ("STATUS")) -> ()
        n1121 = property on="Z Velocity SP step/sec" class="DigNum (strict)"() -> ("Maximum"=w2040:dbl)  [unwired: 2 in, 2 out]
        n1122 = property on="Z Velocity SP step/sec" class="DigNum (strict)"() -> ("Minimum"=w2039:dbl)  [unwired: 2 in, 2 out]
        n1123 = Subtract(x=w2050, y=w2051) -> (x-y=w2054:dbl)
        n1124 = property on="Z Velocity SP mm/sec" class="DigNum (strict)"() -> ("Value"=w2044:dbl)  [unwired: 2 in, 2 out]
        n1125 = property on="Z mm/rev" class="DigNum (strict)"() -> ("Value"=w2056:dbl)  [unwired: 2 in, 2 out]
        n1126 = Divide(x=w2054, y=w2056) -> (x/y=w2055:dbl)
        n1127 = Divide(x=w2044, y=w2056) -> (x/y=w2045:dbl)
        n1128 = To Double Precision Float(number=w2053) -> (double precision float=w2057:dbl)
        n1129 = Multiply(x=w2055, y=w2057) -> (x*y=w2049:dbl)
        n1130 = Multiply(x=w2045, y=w2057) -> (x*y=w2042:dbl)
        n1131 = In Range and Coerce(upper limit=w2040, x=w2042, lower limit=w2039) -> (coerced(x)=w2041:dbl)  [unwired: 1 out]
        n1132 = property on="Z Step SP" class="DigNum (strict)"() -> ("Maximum"=w2047:dbl)  [unwired: 2 in, 2 out]
        n1133 = property on="Z Step SP" class="DigNum (strict)"() -> ("Minimum"=w2046:dbl)  [unwired: 2 in, 2 out]
        n1134 = To Long Integer(number=w2041) -> (32bit integer=w2043:i32)
        n1135 = In Range and Coerce(upper limit=w2047, x=w2049, lower limit=w2046) -> (coerced(x)=w2048:dbl)  [unwired: 1 out]
        n1136 = To Long Integer(number=w2048) -> (32bit integer=w2052:i32)
        n1137 = property on="Z Velocity SP step/sec" class="DigNum (strict)"("Val(Sgnl)"=w2043) -> ()  [unwired: 2 in, 2 out]
        n1138 = property on="Z Step SP" class="DigNum (strict)"("Val(Sgnl)"=w2052) -> ()  [unwired: 2 in, 2 out]
      }
      event "R Move Set": Mouse Down {
        n1139 = event-data() -> ()  [unwired: 1 in, 7 out]
        n1140 = property on="R steps/rev" class="DigNum (strict)"() -> ("Value"=w2077:u32)  [unwired: 2 in, 2 out]
        n1141 = Wait (ms)(milliseconds to wait=u32 100) -> ()  [unwired: 1 out]
        n1142 = property on="R offset deg" class="DigNum (strict)"() -> ("Value"=w2075:dbl)  [unwired: 2 in, 2 out]
        n1143 = property on="R Position SP deg" class="DigNum (strict)"() -> ("Value"=w2074:dbl)  [unwired: 2 in, 2 out]
        n1144 = local write "STATUS"("SETTING R" ("STATUS")) -> ()
        n1145 = property on="R Velocity SP step/sec" class="DigNum (strict)"() -> ("Maximum"=w2064:dbl)  [unwired: 2 in, 2 out]
        n1146 = property on="R Velocity SP step/sec" class="DigNum (strict)"() -> ("Minimum"=w2063:dbl)  [unwired: 2 in, 2 out]
        n1147 = Subtract(x=w2074, y=w2075) -> (x-y=w2078:dbl)
        n1148 = property on="R Velocity SP deg/sec" class="DigNum (strict)"() -> ("Value"=w2068:dbl)  [unwired: 2 in, 2 out]
        n1149 = property on="R deg/rev" class="DigNum (strict)"() -> ("Value"=w2061:dbl)  [unwired: 2 in, 2 out]
        n1150 = Divide(x=w2078, y=w2061) -> (x/y=w2079:dbl)
        n1151 = Divide(x=w2068, y=w2061) -> (x/y=w2069:dbl)
        n1152 = To Double Precision Float(number=w2077) -> (double precision float=w2062:dbl)
        n1153 = Multiply(x=w2079, y=w2062) -> (x*y=w2073:dbl)
        n1154 = Multiply(x=w2069, y=w2062) -> (x*y=w2066:dbl)
        n1155 = property on="R Step SP" class="DigNum (strict)"() -> ("Maximum"=w2071:dbl)  [unwired: 2 in, 2 out]
        n1156 = property on="R Step SP" class="DigNum (strict)"() -> ("Minimum"=w2070:dbl)  [unwired: 2 in, 2 out]
        n1157 = Absolute Value(x=w2066) -> (abs(x)=w2060:dbl)
        n1158 = In Range and Coerce(upper limit=w2071, x=w2073, lower limit=w2070) -> (coerced(x)=w2072:dbl)  [unwired: 1 out]
        n1159 = In Range and Coerce(upper limit=w2064, x=w2060, lower limit=w2063) -> (coerced(x)=w2065:dbl)  [unwired: 1 out]
        n1160 = To Long Integer(number=w2072) -> (32bit integer=w2076:i32)
        n1161 = To Long Integer(number=w2065) -> (32bit integer=w2067:i32)
        n1162 = property on="R Step SP" class="DigNum (strict)"("Val(Sgnl)"=w2076) -> ()  [unwired: 2 in, 2 out]
        n1163 = property on="R Velocity SP step/sec" class="DigNum (strict)"("Val(Sgnl)"=w2067) -> ()  [unwired: 2 in, 2 out]
      }
      event "Set Scan \nParameters": Mouse Down {
        n1164 = event-data() -> ()  [unwired: 1 in, 7 out]
        n1165 = flat-sequence {
          frame #0 {
            n1166 = property on="Z steps/rev" class="DigNum (strict)"() -> ("Value"=w2148:u32)  [unwired: 2 in, 2 out]
            n1167 = property on="X steps/rev" class="DigNum (strict)"() -> ("Value"=w2131:u32)  [unwired: 2 in, 2 out]
            n1168 = property on="Y steps/rev" class="DigNum (strict)"() -> ("Value"=w2096:u32)  [unwired: 2 in, 2 out]
            n1169 = property on="R steps/rev" class="DigNum (strict)"() -> ("Value"=w2114:u32)  [unwired: 2 in, 2 out]
            n1170 = To Double Precision Float(number=w2148) -> (double precision float=w2134:dbl)
            n1171 = To Double Precision Float(number=w2131) -> (double precision float=w2117:dbl)
            n1172 = To Double Precision Float(number=w2096) -> (double precision float=w2082:dbl)
            n1173 = To Double Precision Float(number=w2114) -> (double precision float=w2100:dbl)
            n1174 = property on="R Velocity SP step/sec" class="DigNum (strict)"() -> ("Maximum"=w2102:dbl)  [unwired: 2 in, 2 out]
            n1175 = property on="Z mm/rev" class="DigNum (strict)"() -> ("Value"=w2133:dbl)  [unwired: 2 in, 2 out]
            n1176 = property on="X mm/rev" class="DigNum (strict)"() -> ("Value"=w2116:dbl)  [unwired: 2 in, 2 out]
            n1177 = property on="Y mm/rev" class="DigNum (strict)"() -> ("Value"=w2081:dbl)  [unwired: 2 in, 2 out]
            n1178 = property on="Z Scan Length SP mm" class="DigNum (strict)"() -> ("Value"=w2146:dbl)  [unwired: 2 in, 2 out]
            n1179 = property on="Z Scan Velocity SP mm/sec" class="DigNum (strict)"() -> ("Value"=w2140:dbl)  [unwired: 2 in, 2 out]
            n1180 = property on="X Scan Length SP mm" class="DigNum (strict)"() -> ("Value"=w2129:dbl)  [unwired: 2 in, 2 out]
            n1181 = property on="X Scan Velocity SP mm/sec" class="DigNum (strict)"() -> ("Value"=w2123:dbl)  [unwired: 2 in, 2 out]
            n1182 = property on="Y Scan Length SP mm" class="DigNum (strict)"() -> ("Value"=w2094:dbl)  [unwired: 2 in, 2 out]
            n1183 = property on="Y Scan Velocity SP mm/sec" class="DigNum (strict)"() -> ("Value"=w2088:dbl)  [unwired: 2 in, 2 out]
            n1184 = property on="R Scan Length SP deg" class="DigNum (strict)"() -> ("Value"=w2112:dbl)  [unwired: 2 in, 2 out]
            n1185 = property on="R deg/rev" class="DigNum (strict)"() -> ("Value"=w2099:dbl)  [unwired: 2 in, 2 out]
            n1186 = property on="Z Scan Velocity SP steps/sec" class="DigNum (strict)"() -> ("Maximum"=w2136:dbl)  [unwired: 2 in, 2 out]
            n1187 = property on="X Scan Velocity SP steps/sec" class="DigNum (strict)"() -> ("Maximum"=w2119:dbl)  [unwired: 2 in, 2 out]
            n1188 = property on="Y Scan Velocity SP steps/sec" class="DigNum (strict)"() -> ("Maximum"=w2084:dbl)  [unwired: 2 in, 2 out]
            n1189 = property on="R Scan Velocity SP steps/sec" class="DigNum (strict)"() -> ("Minimum"=w2101:dbl)  [unwired: 2 in, 2 out]
            n1190 = property on="Z Scan Velocity SP steps/sec" class="DigNum (strict)"() -> ("Minimum"=w2135:dbl)  [unwired: 2 in, 2 out]
            n1191 = property on="X Scan Velocity SP steps/sec" class="DigNum (strict)"() -> ("Minimum"=w2118:dbl)  [unwired: 2 in, 2 out]
            n1192 = property on="Y Scan Velocity SP steps/sec" class="DigNum (strict)"() -> ("Minimum"=w2083:dbl)  [unwired: 2 in, 2 out]
            n1193 = property on="R Scan Velocity SP deg/sec" class="DigNum (strict)"() -> ("Value"=w2106:dbl)  [unwired: 2 in, 2 out]
            n1194 = Divide(x=w2146, y=w2133) -> (x/y=w2149:dbl)
            n1195 = Divide(x=w2140, y=w2133) -> (x/y=w2141:dbl)
            n1196 = Divide(x=w2129, y=w2116) -> (x/y=w2132:dbl)
            n1197 = Divide(x=w2123, y=w2116) -> (x/y=w2124:dbl)
            n1198 = Divide(x=w2094, y=w2081) -> (x/y=w2097:dbl)
            n1199 = Divide(x=w2088, y=w2081) -> (x/y=w2089:dbl)
            n1200 = Divide(x=w2112, y=w2099) -> (x/y=w2115:dbl)
            n1201 = Multiply(x=w2149, y=w2134) -> (x*y=w2145:dbl)
            n1202 = Multiply(x=w2141, y=w2134) -> (x*y=w2138:dbl)
            n1203 = Multiply(x=w2132, y=w2117) -> (x*y=w2128:dbl)
            n1204 = Multiply(x=w2124, y=w2117) -> (x*y=w2121:dbl)
            n1205 = Multiply(x=w2097, y=w2082) -> (x*y=w2093:dbl)
            n1206 = Multiply(x=w2089, y=w2082) -> (x*y=w2086:dbl)
            n1207 = Multiply(x=w2115, y=w2100) -> (x*y=w2111:dbl)
            n1208 = Divide(x=w2106, y=w2099) -> (x/y=w2107:dbl)
            n1209 = property on="Z Step SP" class="DigNum (strict)"() -> ("Maximum"=w2142:dbl)  [unwired: 2 in, 2 out]
            n1210 = property on="X Step SP" class="DigNum (strict)"() -> ("Maximum"=w2125:dbl)  [unwired: 2 in, 2 out]
            n1211 = property on="Y Step SP" class="DigNum (strict)"() -> ("Maximum"=w2090:dbl)  [unwired: 2 in, 2 out]
            n1212 = property on="R Step SP" class="DigNum (strict)"() -> ("Maximum"=w2108:dbl)  [unwired: 2 in, 2 out]
            n1213 = property on="Z Step SP" class="DigNum (strict)"() -> ("Minimum"=w2143:dbl)  [unwired: 2 in, 2 out]
            n1214 = property on="X Step SP" class="DigNum (strict)"() -> ("Minimum"=w2126:dbl)  [unwired: 2 in, 2 out]
            n1215 = property on="Y Step SP" class="DigNum (strict)"() -> ("Minimum"=w2091:dbl)  [unwired: 2 in, 2 out]
            n1216 = property on="R Step SP" class="DigNum (strict)"() -> ("Minimum"=w2109:dbl)  [unwired: 2 in, 2 out]
            n1217 = Multiply(x=w2107, y=w2100) -> (x*y=w2104:dbl)
            n1218 = In Range and Coerce(upper limit=w2136, x=w2138, lower limit=w2135) -> (coerced(x)=w2137:dbl)  [unwired: 1 out]
            n1219 = In Range and Coerce(upper limit=w2119, x=w2121, lower limit=w2118) -> (coerced(x)=w2120:dbl)  [unwired: 1 out]
            n1220 = In Range and Coerce(upper limit=w2084, x=w2086, lower limit=w2083) -> (coerced(x)=w2085:dbl)  [unwired: 1 out]
            n1221 = To Long Integer(number=w2137) -> (32bit integer=w2139:i32)
            n1222 = To Long Integer(number=w2120) -> (32bit integer=w2122:i32)
            n1223 = To Long Integer(number=w2085) -> (32bit integer=w2087:i32)
            n1224 = Absolute Value(x=w2104) -> (abs(x)=w2098:dbl)
            n1225 = In Range and Coerce(upper limit=w2142, x=w2145, lower limit=w2143) -> (coerced(x)=w2144:dbl)  [unwired: 1 out]
            n1226 = In Range and Coerce(upper limit=w2125, x=w2128, lower limit=w2126) -> (coerced(x)=w2127:dbl)  [unwired: 1 out]
            n1227 = In Range and Coerce(upper limit=w2090, x=w2093, lower limit=w2091) -> (coerced(x)=w2092:dbl)  [unwired: 1 out]
            n1228 = In Range and Coerce(upper limit=w2108, x=w2111, lower limit=w2109) -> (coerced(x)=w2110:dbl)  [unwired: 1 out]
            n1229 = To Long Integer(number=w2144) -> (32bit integer=w2147:i32)
            n1230 = To Long Integer(number=w2127) -> (32bit integer=w2130:i32)
            n1231 = To Long Integer(number=w2092) -> (32bit integer=w2095:i32)
            n1232 = To Long Integer(number=w2110) -> (32bit integer=w2113:i32)
            n1233 = property on="Z Scan Velocity SP steps/sec" class="DigNum (strict)"("Val(Sgnl)"=w2139) -> ()  [unwired: 2 in, 2 out]
            n1234 = property on="X Scan Velocity SP steps/sec" class="DigNum (strict)"("Val(Sgnl)"=w2122) -> ()  [unwired: 2 in, 2 out]
            n1235 = property on="Y Scan Velocity SP steps/sec" class="DigNum (strict)"("Val(Sgnl)"=w2087) -> ()  [unwired: 2 in, 2 out]
            n1236 = In Range and Coerce(upper limit=w2102, x=w2098, lower limit=w2101) -> (coerced(x)=w2103:dbl)  [unwired: 1 out]
            n1237 = To Long Integer(number=w2103) -> (32bit integer=w2105:i32)
            n1238 = property on="Z Scan Length SP steps" class="DigNum (strict)"("Val(Sgnl)"=w2147) -> ()  [unwired: 2 in, 2 out]
            n1239 = property on="X Scan Length SP steps" class="DigNum (strict)"("Val(Sgnl)"=w2130) -> ()  [unwired: 2 in, 2 out]
            n1240 = property on="Y Scan Length SP steps" class="DigNum (strict)"("Val(Sgnl)"=w2095) -> ()  [unwired: 2 in, 2 out]
            n1241 = property on="R Scan Length SP steps" class="DigNum (strict)"("Val(Sgnl)"=w2113) -> ()  [unwired: 2 in, 2 out]
            n1242 = property on="R Scan Velocity SP steps/sec" class="DigNum (strict)"("Val(Sgnl)"=w2105) -> ()  [unwired: 2 in, 2 out]
          }
          frame #1 {
            n1243 = case shown="True" "Z as dominating length" {
              frame False {
              }
              frame True {
                n1244 = property on="Y Scan Length SP steps" class="DigNum (strict)"() -> ("Value"=w2159:i32)  [unwired: 2 in, 2 out]
                n1245 = property on="Z Scan Length SP steps" class="DigNum (strict)"() -> ("Value"=w2158:i32)  [unwired: 2 in, 2 out]
                n1246 = property on="X Scan Length SP steps" class="DigNum (strict)"() -> ("Value"=w2167:i32)  [unwired: 2 in, 2 out]
                n1247 = property on="Z Scan Length SP steps" class="DigNum (strict)"() -> ("Value"=w2166:i32)  [unwired: 2 in, 2 out]
                n1248 = property on="Y Scan Velocity SP steps/sec" class="DigNum (strict)"() -> ("Value"=w2155:i32)  [unwired: 2 in, 2 out]
                n1249 = property on="X Scan Velocity SP steps/sec" class="DigNum (strict)"() -> ("Value"=w2165:i32)  [unwired: 2 in, 2 out]
                n1250 = To Double Precision Float(number=w2159) -> (double precision float=w2157:dbl)
                n1251 = To Double Precision Float(number=w2158) -> (double precision float=w2156:dbl)
                n1252 = To Double Precision Float(number=w2167) -> (double precision float=w2161:dbl)
                n1253 = To Double Precision Float(number=w2166) -> (double precision float=w2162:dbl)
                n1254 = Divide(x=w2157, y=w2156) -> (x/y=w2151:dbl)
                n1255 = Divide(x=w2161, y=w2162) -> (x/y=w2168:dbl)
                n1256 = To Double Precision Float(number=w2155) -> (double precision float=w2154:dbl)
                n1257 = To Double Precision Float(number=w2165) -> (double precision float=w2163:dbl)
                n1258 = Multiply(x=w2151, y=w2154) -> (x*y=w2153:dbl)
                n1259 = Multiply(x=w2168, y=w2163) -> (x*y=w2164:dbl)
                n1260 = To Long Integer(number=w2153) -> (32bit integer=w2152:i32)
                n1261 = To Long Integer(number=w2164) -> (32bit integer=w2160:i32)
                n1262 = property on="Y Scan Velocity SP steps/sec" class="DigNum (strict)"("Val(Sgnl)"=w2152) -> ()  [unwired: 2 in, 2 out]
                n1263 = property on="X Scan Velocity SP steps/sec" class="DigNum (strict)"("Val(Sgnl)"=w2160) -> ()  [unwired: 2 in, 2 out]
              }
            }
          }
          frame #2 {
            w2169 = T9."Enabled" ("Disabled")
            n1264 = property on="Send scan parameter" class="Bool"("DisabledEnum"=w2169) -> ()  [unwired: 2 in, 2 out]
            n1265 = property on="LOOP" class="Bool (strict)"("DisabledEnum"=w2169) -> ()  [unwired: 2 in, 2 out]
          }
        }
        n1266 = local write "STATUS"("SCANNING PARAMETERS SET" ("STATUS")) -> ()
      }
      event "Send scan parameter": Mouse Up {
        n1267 = event-data() -> ()  [unwired: 1 in, 7 out]
        n1268 = local write "STATUS"("READY TO SCAN" ("STATUS")) -> ()
        n1269 = flat-sequence {
          tunnel: [w2223] -> w2183
          tunnel: [w2222] -> w2182
          tunnel: w2173 -> [w2221]
          tunnel: w2172 -> [w2220]
          tunnel: w2183 -> [w2229]
          tunnel: [w2229] -> w2181
          tunnel: w2182 -> [w2228]
          tunnel: [w2228] -> w2180
          tunnel: w2181 -> [w2235]
          tunnel: [w2234] -> w2179
          tunnel: w2180 -> [w2233]
          tunnel: [w2232] -> w2178
          tunnel: w2179 -> [w2241]
          tunnel: w2178 -> [w2240]
          tunnel: [w2241] -> w2177
          tunnel: [w2240] -> w2176
          tunnel: w2177 -> [w2246]
          tunnel: w2176 -> [w2245]
          tunnel: [w2246] -> w2175
          tunnel: [w2245] -> w2174
          tunnel: [w2248] -> _
          tunnel: [w2249] -> _
          tunnel: w2175 -> [w2249]
          tunnel: w2174 -> [w2248]
          frame #0 {
            n1270 = property on="R Scan Velocity SP steps/sec" class="DigNum (strict)"() -> ("Value"=w2225:i32)  [unwired: 2 in, 2 out]
            n1271 = Number To Decimal String(number=w2225) -> (decimal integer string=w2226:string)  [unwired: 1 in]
            n1272 = call "mDrive Send Command.vi"("error in (no error)"=w2221, "Extra"=w2226, "Command"=T10."Max Velocity", "VISA resource name"=w2220) -> ("error out"=w2222:errorcluster, "VISA resource name out"=w2223:refnum<visa-resource-name>)  [unwired: 3 in, 1 out]
          }
          frame #1 {
            n1273 = Wait (ms)(milliseconds to wait=u32 100) -> ()  [unwired: 1 out]
          }
          frame #2 {
            # "VELOCITY"
            n1274 = call "mdrive send command.vi"("error in (no error)"=w2233, "Extra"="VM", "Command"=T10."Print Parameter", "VISA resource name"=w2235) -> ("error out"=w2232:errorcluster, "read buffer"=w2237:string, "VISA resource name out"=w2234:refnum<visa-resource-name>)  [unwired: 3 in]
            n1275 = Decimal String To Number(string=w2237, offset=0) -> (number=w2236:i32)  [unwired: 1 in, 1 out]
            n1276 = property on="R velocity PV step/sec" class="DigNum (strict)"("Val(Sgnl)"=w2236) -> ()  [unwired: 2 in, 2 out]
          }
          frame #3 {
            n1277 = Wait (ms)(milliseconds to wait=u32 100) -> ()  [unwired: 1 out]
          }
          frame #4 {
            n1278 = property on="Scan Go" class="Bool (strict)"("DisabledEnum"=T9."Enabled" ("Disabled")) -> ()  [unwired: 2 in, 2 out]
            n1279 = property on="R Scan Velocity SP steps/sec" class="DigNum (strict)"("DisabledEnum"=T9."Disabled and Grayed Out" ("Disabled")) -> ()  [unwired: 2 in, 2 out]
            n1280 = property on="R Scan Length SP steps" class="DigNum (strict)"("DisabledEnum"=T9."Disabled and Grayed Out" ("Disabled")) -> ()  [unwired: 2 in, 2 out]
          }
          frame #5 {
            n1281 = property on="R Scan" class="Bool (strict)"("Val(Sgnl)"=TRUE ("Slew Ready 2")) -> ()  [unwired: 2 in, 2 out]
          }
        }
        n1282 = flat-sequence {
          tunnel: [w2283] -> w2207
          tunnel: [w2282] -> w2206
          tunnel: w2197 -> [w2281]
          tunnel: w2196 -> [w2280]
          tunnel: w2207 -> [w2289]
          tunnel: [w2289] -> w2205
          tunnel: w2206 -> [w2288]
          tunnel: [w2288] -> w2204
          tunnel: w2205 -> [w2293]
          tunnel: [w2292] -> w2203
          tunnel: w2204 -> [w2291]
          tunnel: [w2290] -> w2202
          tunnel: w2203 -> [w2301]
          tunnel: [w2301] -> w2201
          tunnel: w2202 -> [w2300]
          tunnel: [w2300] -> w2200
          tunnel: w2201 -> [w2306]
          tunnel: w2200 -> [w2305]
          tunnel: [w2306] -> w2199
          tunnel: [w2305] -> w2198
          tunnel: [w2308] -> _
          tunnel: [w2309] -> _
          tunnel: w2199 -> [w2309]
          tunnel: w2198 -> [w2308]
          frame #0 {
            n1283 = property on="Y Scan Velocity SP steps/sec" class="DigNum (strict)"() -> ("Value"=w2285:i32)  [unwired: 2 in, 2 out]
            n1284 = Number To Decimal String(number=w2285) -> (decimal integer string=w2286:string)  [unwired: 1 in]
            n1285 = call "mdrive send command.vi"("error in (no error)"=w2281, "Extra"=w2286, "Command"=T10."Max Velocity", "VISA resource name"=w2280) -> ("error out"=w2282:errorcluster, "VISA resource name out"=w2283:refnum<visa-resource-name>)  [unwired: 3 in, 1 out]
          }
          frame #1 {
            n1286 = Wait (ms)(milliseconds to wait=u32 100) -> ()  [unwired: 1 out]
          }
          frame #2 {
            # "VELOCITY"
            n1287 = call "mdrive send command.vi"("error in (no error)"=w2291, "Extra"="VM", "Command"=T10."Print Parameter", "VISA resource name"=w2293) -> ("error out"=w2290:errorcluster, "read buffer"=w2297:string, "VISA resource name out"=w2292:refnum<visa-resource-name>)  [unwired: 3 in]
            n1288 = Decimal String To Number(string=w2297, offset=0) -> (number=w2295:i32)  [unwired: 1 in, 1 out]
            n1289 = property on="Y velocity PV step/sec" class="DigNum (strict)"("Val(Sgnl)"=w2295) -> ()  [unwired: 2 in, 2 out]
          }
          frame #3 {
            n1290 = Wait (ms)(milliseconds to wait=u32 100) -> ()  [unwired: 1 out]
          }
          frame #4 {
            n1291 = property on="Scan Go" class="Bool (strict)"("DisabledEnum"=T9."Enabled" ("Disabled")) -> ()  [unwired: 2 in, 2 out]
            n1292 = property on="Y Scan Velocity SP steps/sec" class="DigNum (strict)"("DisabledEnum"=T9."Disabled and Grayed Out" ("Disabled")) -> ()  [unwired: 2 in, 2 out]
            n1293 = property on="Y Scan Length SP steps" class="DigNum (strict)"("DisabledEnum"=T9."Disabled and Grayed Out" ("Disabled")) -> ()  [unwired: 2 in, 2 out]
          }
          frame #5 {
            n1294 = property on="Y Scan" class="Bool (strict)"("Val(Sgnl)"=TRUE ("Slew Ready 2")) -> ()  [unwired: 2 in, 2 out]
          }
        }
        n1295 = flat-sequence {
          tunnel: [w2311] -> w2211
          tunnel: [w2310] -> w2209
          tunnel: w2217 -> [w2313]
          tunnel: w2216 -> [w2312]
          tunnel: w2211 -> [w2319]
          tunnel: [w2319] -> w2210
          tunnel: w2209 -> [w2318]
          tunnel: [w2318] -> w2208
          tunnel: w2210 -> [w2323]
          tunnel: [w2322] -> w2213
          tunnel: w2208 -> [w2321]
          tunnel: [w2320] -> w2212
          tunnel: w2213 -> [w2331]
          tunnel: [w2331] -> w2215
          tunnel: w2212 -> [w2330]
          tunnel: [w2330] -> w2214
          tunnel: w2215 -> [w2336]
          tunnel: w2214 -> [w2335]
          tunnel: [w2336] -> w2219
          tunnel: [w2335] -> w2218
          tunnel: [w2338] -> _
          tunnel: [w2339] -> _
          tunnel: w2219 -> [w2339]
          tunnel: w2218 -> [w2338]
          frame #0 {
            n1296 = property on="X Scan Velocity SP steps/sec" class="DigNum (strict)"() -> ("Value"=w2315:i32)  [unwired: 2 in, 2 out]
            n1297 = Number To Decimal String(number=w2315) -> (decimal integer string=w2316:string)  [unwired: 1 in]
            n1298 = call "mdrive send command.vi"("error in (no error)"=w2313, "Extra"=w2316, "Command"=T10."Max Velocity", "VISA resource name"=w2312) -> ("error out"=w2310:errorcluster, "VISA resource name out"=w2311:refnum<visa-resource-name>)  [unwired: 3 in, 1 out]
          }
          frame #1 {
            n1299 = Wait (ms)(milliseconds to wait=u32 100) -> ()  [unwired: 1 out]
          }
          frame #2 {
            # "VELOCITY"
            n1300 = call "mdrive send command.vi"("error in (no error)"=w2321, "Extra"="VM", "Command"=T10."Print Parameter", "VISA resource name"=w2323) -> ("error out"=w2320:errorcluster, "read buffer"=w2326:string, "VISA resource name out"=w2322:refnum<visa-resource-name>)  [unwired: 3 in]
            n1301 = Decimal String To Number(string=w2326, offset=0) -> (number=w2324:i32)  [unwired: 1 in, 1 out]
            n1302 = property on="X velocity PV step/sec" class="DigNum (strict)"("Val(Sgnl)"=w2324) -> ()  [unwired: 2 in, 2 out]
          }
          frame #3 {
            n1303 = Wait (ms)(milliseconds to wait=u32 100) -> ()  [unwired: 1 out]
          }
          frame #4 {
            n1304 = property on="Scan Go" class="Bool (strict)"("DisabledEnum"=T9."Enabled" ("Disabled")) -> ()  [unwired: 2 in, 2 out]
            n1305 = property on="X Scan Velocity SP steps/sec" class="DigNum (strict)"("DisabledEnum"=T9."Disabled and Grayed Out" ("Disabled")) -> ()  [unwired: 2 in, 2 out]
            n1306 = property on="X Scan Length SP steps" class="DigNum (strict)"("DisabledEnum"=T9."Disabled and Grayed Out" ("Disabled")) -> ()  [unwired: 2 in, 2 out]
          }
          frame #5 {
            n1307 = property on="X Scan" class="Bool (strict)"("Val(Sgnl)"=TRUE ("Slew Ready 2")) -> ()  [unwired: 2 in, 2 out]
          }
        }
        n1308 = flat-sequence {
          tunnel: [w2253] -> w2195
          tunnel: [w2252] -> w2194
          tunnel: w2185 -> [w2251]
          tunnel: w2184 -> [w2250]
          tunnel: w2195 -> [w2259]
          tunnel: [w2259] -> w2193
          tunnel: w2194 -> [w2258]
          tunnel: [w2258] -> w2192
          tunnel: w2193 -> [w2265]
          tunnel: [w2264] -> w2191
          tunnel: w2192 -> [w2263]
          tunnel: [w2262] -> w2190
          tunnel: w2191 -> [w2271]
          tunnel: [w2271] -> w2189
          tunnel: w2190 -> [w2270]
          tunnel: [w2270] -> w2188
          tunnel: w2189 -> [w2276]
          tunnel: w2188 -> [w2275]
          tunnel: [w2276] -> w2187
          tunnel: [w2275] -> w2186
          tunnel: [w2278] -> _
          tunnel: [w2279] -> _
          tunnel: w2187 -> [w2279]
          tunnel: w2186 -> [w2278]
          frame #0 {
            n1309 = property on="Z Scan Velocity SP steps/sec" class="DigNum (strict)"() -> ("Value"=w2255:i32)  [unwired: 2 in, 2 out]
            n1310 = Number To Decimal String(number=w2255) -> (decimal integer string=w2256:string)  [unwired: 1 in]
            n1311 = call "mdrive send command.vi"("error in (no error)"=w2251, "Extra"=w2256, "Command"=T10."Max Velocity", "VISA resource name"=w2250) -> ("error out"=w2252:errorcluster, "VISA resource name out"=w2253:refnum<visa-resource-name>)  [unwired: 3 in, 1 out]
          }
          frame #1 {
            n1312 = Wait (ms)(milliseconds to wait=u32 100) -> ()  [unwired: 1 out]
          }
          frame #2 {
            # "VELOCITY"
            n1313 = call "mdrive send command.vi"("error in (no error)"=w2263, "Extra"="VM", "Command"=T10."Print Parameter", "VISA resource name"=w2265) -> ("error out"=w2262:errorcluster, "read buffer"=w2266:string, "VISA resource name out"=w2264:refnum<visa-resource-name>)  [unwired: 3 in]
            n1314 = Decimal String To Number(string=w2266, offset=0) -> (number=w2267:i32)  [unwired: 1 in, 1 out]
            n1315 = property on="Z  velocity PV step/sec" class="DigNum (strict)"("Val(Sgnl)"=w2267) -> ()  [unwired: 2 in, 2 out]
          }
          frame #3 {
            n1316 = Wait (ms)(milliseconds to wait=u32 100) -> ()  [unwired: 1 out]
          }
          frame #4 {
            n1317 = property on="Scan Go" class="Bool (strict)"("DisabledEnum"=T9."Enabled" ("Disabled")) -> ()  [unwired: 2 in, 2 out]
            n1318 = property on="Z Scan Velocity SP steps/sec" class="DigNum (strict)"("DisabledEnum"=T9."Disabled and Grayed Out" ("Disabled")) -> ()  [unwired: 2 in, 2 out]
            n1319 = property on="Z Scan Length SP steps" class="DigNum (strict)"("DisabledEnum"=T9."Disabled and Grayed Out" ("Disabled")) -> ()  [unwired: 2 in, 2 out]
          }
          frame #5 {
            n1320 = property on="Z Scan" class="Bool (strict)"("Val(Sgnl)"=TRUE ("Slew Ready 2")) -> ()  [unwired: 2 in, 2 out]
          }
        }
        n1321 = property on="GO" class="Bool"("DisabledEnum"=T9."Disabled and Grayed Out" ("Disabled")) -> ()  [unwired: 2 in, 2 out]
      }
      event "Scan Cancel": Mouse Down {
        n1322 = event-data() -> ()  [unwired: 1 in, 7 out]
        n1323 = flat-sequence {
          tunnel: [w2364] -> w2352
          tunnel: [w2363] -> w2351
          tunnel: w2345 -> [w2361]
          tunnel: w2343 -> [w2360]
          tunnel: [w2368] -> _
          tunnel: [w2369] -> _
          tunnel: w2352 -> [w2369]
          tunnel: w2351 -> [w2368]
          frame #0 {
            n1324 = call "mDrive Send Command.vi"("error in (no error)"=w2360, "Command"=T10."Stop", "VISA resource name"=w2361) -> ("error out"=w2363:errorcluster, "VISA resource name out"=w2364:refnum<visa-resource-name>)  [unwired: 4 in, 1 out]
          }
          frame #1 {
            n1325 = property on="R Scan" class="Bool (strict)"("Value"=FALSE ("Slew Ready")) -> ()  [unwired: 2 in, 2 out]
            n1326 = property on="R Scan Length SP steps" class="DigNum (strict)"("DisabledEnum"=T9."Enabled" ("Disabled")) -> ()  [unwired: 2 in, 2 out]
            n1327 = property on="R Scan Velocity SP steps/sec" class="DigNum (strict)"("DisabledEnum"=T9."Enabled" ("Disabled")) -> ()  [unwired: 2 in, 2 out]
          }
        }
        n1328 = flat-sequence {
          tunnel: [w2384] -> w2356
          tunnel: [w2383] -> w2355
          tunnel: w2350 -> [w2381]
          tunnel: w2348 -> [w2380]
          tunnel: [w2388] -> _
          tunnel: [w2389] -> _
          tunnel: w2356 -> [w2389]
          tunnel: w2355 -> [w2388]
          frame #0 {
            n1329 = call "mDrive Send Command.vi"("error in (no error)"=w2380, "Command"=T10."Stop", "VISA resource name"=w2381) -> ("error out"=w2383:errorcluster, "VISA resource name out"=w2384:refnum<visa-resource-name>)  [unwired: 4 in, 1 out]
          }
          frame #1 {
            n1330 = property on="X Scan" class="Bool (strict)"("Value"=FALSE ("Slew Ready")) -> ()  [unwired: 2 in, 2 out]
            n1331 = property on="X Scan Velocity SP steps/sec" class="DigNum (strict)"("DisabledEnum"=T9."Enabled" ("Disabled")) -> ()  [unwired: 2 in, 2 out]
            n1332 = property on="X Scan Length SP steps" class="DigNum (strict)"("DisabledEnum"=T9."Enabled" ("Disabled")) -> ()  [unwired: 2 in, 2 out]
          }
        }
        n1333 = flat-sequence {
          tunnel: [w2374] -> w2354
          tunnel: [w2373] -> w2353
          tunnel: w2349 -> [w2371]
          tunnel: w2347 -> [w2370]
          tunnel: [w2378] -> _
          tunnel: [w2379] -> _
          tunnel: w2354 -> [w2379]
          tunnel: w2353 -> [w2378]
          frame #0 {
            n1334 = call "mDrive Send Command.vi"("error in (no error)"=w2370, "Command"=T10."Stop", "VISA resource name"=w2371) -> ("error out"=w2373:errorcluster, "VISA resource name out"=w2374:refnum<visa-resource-name>)  [unwired: 4 in, 1 out]
          }
          frame #1 {
            n1335 = property on="Z Scan" class="Bool (strict)"("Value"=FALSE ("Slew Ready")) -> ()  [unwired: 2 in, 2 out]
            n1336 = property on="Z Scan Velocity SP steps/sec" class="DigNum (strict)"("DisabledEnum"=T9."Enabled" ("Disabled")) -> ()  [unwired: 2 in, 2 out]
            n1337 = property on="Z Scan Length SP steps" class="DigNum (strict)"("DisabledEnum"=T9."Enabled" ("Disabled")) -> ()  [unwired: 2 in, 2 out]
          }
        }
        n1338 = flat-sequence {
          tunnel: [w2394] -> w2358
          tunnel: [w2393] -> w2357
          tunnel: w2346 -> [w2391]
          tunnel: w2344 -> [w2390]
          tunnel: [w2398] -> _
          tunnel: [w2399] -> _
          tunnel: w2358 -> [w2399]
          tunnel: w2357 -> [w2398]
          frame #0 {
            n1339 = call "mDrive Send Command.vi"("error in (no error)"=w2390, "Command"=T10."Stop", "VISA resource name"=w2391) -> ("error out"=w2393:errorcluster, "VISA resource name out"=w2394:refnum<visa-resource-name>)  [unwired: 4 in, 1 out]
          }
          frame #1 {
            n1340 = property on="Y Scan" class="Bool (strict)"("Value"=FALSE ("Slew Ready")) -> ()  [unwired: 2 in, 2 out]
            n1341 = property on="Y Scan Velocity SP steps/sec" class="DigNum (strict)"("DisabledEnum"=T9."Enabled" ("Disabled")) -> ()  [unwired: 2 in, 2 out]
            n1342 = property on="Y Scan Length SP steps" class="DigNum (strict)"("DisabledEnum"=T9."Enabled" ("Disabled")) -> ()  [unwired: 2 in, 2 out]
          }
        }
        n1343 = property on="GO" class="Bool"("DisabledEnum"=T9."Enabled" ("Disabled")) -> ()  [unwired: 2 in, 2 out]
        n1344 = property on="Set Scan \nParameters" class="Bool"("DisabledEnum"=T9."Enabled" ("Disabled")) -> ()  [unwired: 2 in, 2 out]
        n1345 = property on="Send scan parameter" class="Bool"("DisabledEnum"=T9."Enabled" ("Disabled")) -> ()  [unwired: 2 in, 2 out]
        n1346 = property on="Scan Go" class="Bool (strict)"("DisabledEnum"=T9."Disabled and Grayed Out" ("Disabled")) -> ()  [unwired: 2 in, 2 out]
      }
      event "Scan Go": Mouse Up {
        w2400 = T9."Disabled and Grayed Out" ("Disabled")
        n1347 = event-data() -> ()  [unwired: 1 in, 7 out]
        n1348 = flat-sequence {
          tunnel: [w2473] -> w2457
          tunnel: [w2471] -> w2450
          tunnel: [w2472] -> w2447
          tunnel: [w2466] -> w2446
          tunnel: [w2470] -> w2445
          tunnel: [w2469] -> w2444
          tunnel: [w2468] -> w2443
          tunnel: [w2467] -> w2442
          tunnel: w2417 -> [w2465]
          tunnel: w2416 -> [w2464]
          tunnel: w2415 -> [w2463]
          tunnel: w2414 -> [w2462]
          tunnel: w2413 -> [w2461]
          tunnel: w2412 -> [w2460]
          tunnel: w2411 -> [w2459]
          tunnel: w2410 -> [w2458]
          tunnel: [w2465] -> w2409
          tunnel: [w2464] -> w2408
          tunnel: [w2463] -> w2407
          tunnel: [w2462] -> w2406
          tunnel: [w2461] -> w2405
          tunnel: [w2460] -> w2404
          tunnel: [w2459] -> w2403
          tunnel: [w2458] -> w2402
          tunnel: [w2525] -> w2454
          tunnel: [w2524] -> w2452
          tunnel: w2457 -> [w2523]
          tunnel: w2450 -> [w2522]
          tunnel: [w2522] -> w2448
          tunnel: w2447 -> [w2521]
          tunnel: w2446 -> [w2510]
          tunnel: w2445 -> [w2520]
          tunnel: w2444 -> [w2516]
          tunnel: w2443 -> [w2513]
          tunnel: w2442 -> [w2519]
          tunnel: [w2518] -> w2440
          tunnel: [w2517] -> w2438
          tunnel: [w2516] -> w2435
          tunnel: [w2515] -> w2433
          tunnel: [w2514] -> w2431
          tunnel: [w2513] -> w2429
          tunnel: [w2512] -> w2427
          tunnel: [w2511] -> w2425
          tunnel: [w2510] -> w2424
          tunnel: w2409 -> [w2509]
          tunnel: w2408 -> [w2508]
          tunnel: w2407 -> [w2507]
          tunnel: w2406 -> [w2506]
          tunnel: w2405 -> [w2505]
          tunnel: w2404 -> [w2504]
          tunnel: w2403 -> [w2503]
          tunnel: w2402 -> [w2502]
          tunnel: w2454 -> [w2566]
          tunnel: [w2566] -> w2453
          tunnel: w2452 -> [w2565]
          tunnel: [w2565] -> w2451
          tunnel: [w2564] -> w2449
          tunnel: w2448 -> [w2564]
          tunnel: [w2563] -> w2441
          tunnel: w2440 -> [w2563]
          tunnel: [w2562] -> w2439
          tunnel: w2438 -> [w2562]
          tunnel: [w2561] -> w2437
          tunnel: [w2560] -> w2436
          tunnel: w2435 -> [w2560]
          tunnel: [w2559] -> w2434
          tunnel: w2433 -> [w2559]
          tunnel: [w2558] -> w2432
          tunnel: w2431 -> [w2558]
          tunnel: [w2557] -> w2430
          tunnel: w2429 -> [w2557]
          tunnel: [w2556] -> w2428
          tunnel: w2427 -> [w2556]
          tunnel: [w2555] -> w2426
          tunnel: w2425 -> [w2555]
          tunnel: w2424 -> [w2561]
          tunnel: w2453 -> [w2586]
          tunnel: [w2584] -> w2456
          tunnel: w2451 -> [w2585]
          tunnel: [w2583] -> w2455
          tunnel: w2449 -> [w2582]
          tunnel: w2441 -> [w2581]
          tunnel: w2439 -> [w2580]
          tunnel: w2437 -> [w2579]
          tunnel: w2436 -> [w2578]
          tunnel: w2434 -> [w2577]
          tunnel: w2432 -> [w2576]
          tunnel: w2430 -> [w2575]
          tunnel: w2428 -> [w2574]
          tunnel: w2426 -> [w2573]
          tunnel: [w2572] -> w2423
          tunnel: [w2571] -> w2422
          tunnel: [w2570] -> w2421
          tunnel: [w2569] -> w2420
          tunnel: [w2568] -> w2419
          tunnel: [w2567] -> w2418
          tunnel: w2456 -> [w2643]
          tunnel: w2455 -> [w2642]
          tunnel: [w2643] -> _
          tunnel: [w2642] -> _
          tunnel: [w2637] -> _
          tunnel: w2423 -> [w2637]
          tunnel: [w2636] -> _
          tunnel: w2422 -> [w2636]
          tunnel: w2421 -> [w2626]
          tunnel: [w2626] -> _
          tunnel: [w2625] -> _
          tunnel: w2420 -> [w2625]
          tunnel: [w2624] -> _
          tunnel: w2419 -> [w2624]
          tunnel: [w2623] -> _
          tunnel: w2418 -> [w2623]
          frame #0 {
            n1349 = property on="X Scan" class="Bool (strict)"() -> ("Value"=w2466:bool)  [unwired: 2 in, 2 out]
            n1350 = property on="Z Scan" class="Bool (strict)"() -> ("Value"=w2468:bool)  [unwired: 2 in, 2 out]
            n1351 = property on="Y Scan" class="Bool (strict)"() -> ("Value"=w2471:bool)  [unwired: 2 in, 2 out]
            n1352 = property on="R Scan" class="Bool (strict)"() -> ("Value"=w2469:bool)  [unwired: 2 in, 2 out]
            n1353 = case shown="False" w2466 {
              tunnel: ["" w2489] -> w2472
              frame False {
              }
              frame True {
                n1354 = property on="X Scan Length SP steps" class="DigNum (strict)"() -> ("Value"=w2494:i32)  [unwired: 2 in, 2 out]
                n1355 = Number To Decimal String(number=w2494) -> (decimal integer string=w2491:string)  [unwired: 1 in]
                n1356 = call <vilib>:"Space Constant.vi"() -> ("String"=w2492:string)
                n1357 = Concatenate Strings("MR", w2492, w2491, "\r") -> (w2489:string)
              }
            }
            n1358 = case shown="False" w2468 {
              tunnel: ["" w2482] -> w2470
              frame False {
              }
              frame True {
                n1359 = property on="Z Scan Length SP steps" class="DigNum (strict)"() -> ("Value"=w2487:i32)  [unwired: 2 in, 2 out]
                n1360 = Number To Decimal String(number=w2487) -> (decimal integer string=w2484:string)  [unwired: 1 in]
                n1361 = call <vilib>:"Space Constant.vi"() -> ("String"=w2485:string)
                n1362 = Concatenate Strings("MR", w2485, w2484, "\r") -> (w2482:string)
              }
            }
            n1363 = case shown="False" w2471 {
              tunnel: ["" w2496] -> w2473
              frame False {
              }
              frame True {
                n1364 = property on="Y Scan Length SP steps" class="DigNum (strict)"() -> ("Value"=w2501:i32)  [unwired: 2 in, 2 out]
                n1365 = Number To Decimal String(number=w2501) -> (decimal integer string=w2498:string)  [unwired: 1 in]
                n1366 = call <vilib>:"Space Constant.vi"() -> ("String"=w2499:string)
                n1367 = Concatenate Strings("MR", w2499, w2498, "\r") -> (w2496:string)
              }
            }
            n1368 = case shown="False" w2469 {
              tunnel: ["" w2475] -> w2467
              frame False {
              }
              frame True {
                n1369 = property on="R Scan Length SP steps" class="DigNum (strict)"() -> ("Value"=w2480:i32)  [unwired: 2 in, 2 out]
                n1370 = Number To Decimal String(number=w2480) -> (decimal integer string=w2477:string)  [unwired: 1 in]
                n1371 = call <vilib>:"Space Constant.vi"() -> ("String"=w2478:string)
                n1372 = Concatenate Strings("MR", w2478, w2477, "\r") -> (w2475:string)
              }
            }
          }
          frame #1 {
            n1373 = case shown="False" w2510 {
              tunnel: [w2541 w2546] -> w2518
              tunnel: [w2540 w2545] -> w2517
              tunnel: w2521 -> [_ w2544]
              tunnel: w2509 -> [w2541 w2543]
              tunnel: w2508 -> [w2540 w2542]
              frame False {
              }
              frame True {
                n1374 = VISA Write(VISA resource name=w2543, write buffer=w2544, error in (no error)=w2542) -> (VISA resource name out=w2546:refnum<visa-resource-name>, error out=w2545:errorcluster)  [unwired: 1 out]
              }
            }
            n1375 = case shown="True" w2513 {
              tunnel: [w2534 w2539] -> w2512
              tunnel: [w2533 w2538] -> w2511
              tunnel: w2520 -> [_ w2537]
              tunnel: w2507 -> [w2534 w2536]
              tunnel: w2506 -> [w2533 w2535]
              frame False {
              }
              frame True {
                n1376 = VISA Write(VISA resource name=w2536, write buffer=w2537, error in (no error)=w2535) -> (VISA resource name out=w2539:refnum<visa-resource-name>, error out=w2538:errorcluster)  [unwired: 1 out]
              }
            }
            n1377 = case shown="True" w2522 {
              tunnel: [w2548 w2553] -> w2525
              tunnel: [w2547 w2552] -> w2524
              tunnel: w2523 -> [_ w2551]
              tunnel: w2505 -> [w2548 w2550]
              tunnel: w2504 -> [w2547 w2549]
              frame False {
              }
              frame True {
                n1378 = VISA Write(VISA resource name=w2550, write buffer=w2551, error in (no error)=w2549) -> (VISA resource name out=w2553:refnum<visa-resource-name>, error out=w2552:errorcluster)  [unwired: 1 out]
              }
            }
            n1379 = case shown="True" w2516 {
              tunnel: [w2527 w2532] -> w2515
              tunnel: [w2526 w2531] -> w2514
              tunnel: w2519 -> [_ w2530]
              tunnel: w2503 -> [w2527 w2529]
              tunnel: w2502 -> [w2526 w2528]
              frame False {
              }
              frame True {
                n1380 = VISA Write(VISA resource name=w2529, write buffer=w2530, error in (no error)=w2528) -> (VISA resource name out=w2532:refnum<visa-resource-name>, error out=w2531:errorcluster)  [unwired: 1 out]
              }
            }
          }
          frame #2 {
            n1381 = Wait (ms)(milliseconds to wait=u32 100) -> ()  [unwired: 1 out]
          }
          frame #3 {
            n1382 = case shown="True" w2579 {
              tunnel: w2581 -> [w2606 w2610]
              tunnel: w2580 -> [w2605 w2609]
              tunnel: [w2606 w2608] -> w2568
              tunnel: [w2605 w2607] -> w2567
              frame False {
              }
              frame True {
                n1383 = property class="Instr"(reference=w2610, error in=w2609) -> (reference out=w2612:refnum<visa-resource-name>, error out=w2611:errorcluster, "Serial Settings:Number of Bytes at Serial Port"=w2613:u32)
                n1384 = VISA Read(VISA resource name=w2612, byte count=w2613, error in (no error)=w2611) -> (VISA resource name out=w2608:refnum<visa-resource-name>, error out=w2607:errorcluster)  [unwired: 2 out]
              }
            }
            n1385 = case shown="True" w2575 {
              tunnel: w2574 -> [w2588 w2592]
              tunnel: w2573 -> [w2587 w2591]
              tunnel: [w2588 w2590] -> w2572
              tunnel: [w2587 w2589] -> w2571
              frame False {
              }
              frame True {
                n1386 = property class="Instr"(reference=w2592, error in=w2591) -> (reference out=w2594:refnum<visa-resource-name>, error out=w2593:errorcluster, "Serial Settings:Number of Bytes at Serial Port"=w2595:u32)
                n1387 = VISA Read(VISA resource name=w2594, byte count=w2595, error in (no error)=w2593) -> (VISA resource name out=w2590:refnum<visa-resource-name>, error out=w2589:errorcluster)  [unwired: 2 out]
              }
            }
            n1388 = case shown="True" w2582 {
              tunnel: w2586 -> [w2615 w2619]
              tunnel: w2585 -> [w2614 w2618]
              tunnel: [w2615 w2617] -> w2584
              tunnel: [w2614 w2616] -> w2583
              frame False {
              }
              frame True {
                n1389 = property class="Instr"(reference=w2619, error in=w2618) -> (reference out=w2621:refnum<visa-resource-name>, error out=w2620:errorcluster, "Serial Settings:Number of Bytes at Serial Port"=w2622:u32)
                n1390 = VISA Read(VISA resource name=w2621, byte count=w2622, error in (no error)=w2620) -> (VISA resource name out=w2617:refnum<visa-resource-name>, error out=w2616:errorcluster)  [unwired: 2 out]
              }
            }
            n1391 = case shown="True" w2578 {
              tunnel: w2577 -> [w2597 w2601]
              tunnel: w2576 -> [w2596 w2600]
              tunnel: [w2597 w2599] -> w2570
              tunnel: [w2596 w2598] -> w2569
              frame False {
              }
              frame True {
                n1392 = property class="Instr"(reference=w2601, error in=w2600) -> (reference out=w2603:refnum<visa-resource-name>, error out=w2602:errorcluster, "Serial Settings:Number of Bytes at Serial Port"=w2604:u32)
                n1393 = VISA Read(VISA resource name=w2603, byte count=w2604, error in (no error)=w2602) -> (VISA resource name out=w2599:refnum<visa-resource-name>, error out=w2598:errorcluster)  [unwired: 2 out]
              }
            }
          }
          frame #4 {
            n1394 = property on="R Scan" class="Bool (strict)"("Val(Sgnl)"=FALSE ("Slew Ready 2")) -> ()  [unwired: 2 in, 2 out]
            n1395 = property on="Z Scan" class="Bool (strict)"("Val(Sgnl)"=FALSE ("Slew Ready 2")) -> ()  [unwired: 2 in, 2 out]
            n1396 = property on="Y Scan" class="Bool (strict)"("Val(Sgnl)"=FALSE ("Slew Ready 2")) -> ()  [unwired: 2 in, 2 out]
            n1397 = property on="X Scan" class="Bool (strict)"("Val(Sgnl)"=FALSE ("Slew Ready 2")) -> ()  [unwired: 2 in, 2 out]
            n1398 = property on="R Scan Length SP steps" class="DigNum (strict)"("DisabledEnum"=T9."Enabled" ("Disabled")) -> ()  [unwired: 2 in, 2 out]
            n1399 = property on="Z Scan Velocity SP steps/sec" class="DigNum (strict)"("DisabledEnum"=T9."Enabled" ("Disabled")) -> ()  [unwired: 2 in, 2 out]
            n1400 = property on="X Scan Length SP steps" class="DigNum (strict)"("DisabledEnum"=T9."Enabled" ("Disabled")) -> ()  [unwired: 2 in, 2 out]
            n1401 = property on="Y Scan Selocity SP steps/sec" class="DigNum (strict)"("DisabledEnum"=T9."Enabled" ("Disabled")) -> ()  [unwired: 2 in, 2 out]
            n1402 = property on="Z Scan Length SP steps" class="DigNum (strict)"("DisabledEnum"=T9."Enabled" ("Disabled")) -> ()  [unwired: 2 in, 2 out]
            n1403 = property on="X Scan Velocity SP steps/sec" class="DigNum (strict)"("DisabledEnum"=T9."Enabled" ("Disabled")) -> ()  [unwired: 2 in, 2 out]
            n1404 = property on="Y Scan Length SP steps" class="DigNum (strict)"("DisabledEnum"=T9."Enabled" ("Disabled")) -> ()  [unwired: 2 in, 2 out]
            n1405 = property on="R Scan Velocity SP steps/sec" class="DigNum (strict)"("DisabledEnum"=T9."Enabled" ("Disabled")) -> ()  [unwired: 2 in, 2 out]
            n1406 = property on="Scan Go" class="Bool (strict)"("DisabledEnum"=T9."Disabled and Grayed Out" ("Disabled")) -> ()  [unwired: 2 in, 2 out]
          }
        }
        n1407 = local write "STATUS"("SCANNING" ("STATUS")) -> ()
        n1408 = property on="GO" class="Bool"("DisabledEnum"=w2400) -> ()  [unwired: 2 in, 2 out]
        n1409 = property on="Set Scan \nParameters" class="Bool"("DisabledEnum"=w2400) -> ()  [unwired: 2 in, 2 out]
        n1410 = property on="Send scan parameter" class="Bool"("DisabledEnum"=w2400) -> ()  [unwired: 2 in, 2 out]
      }
      event "Reset": Mouse Down {
        n1411 = event-data() -> ()  [unwired: 1 in, 7 out]
        n1412 = flat-sequence {
          tunnel: [w2655] -> _
          tunnel: [w2656] -> _
          tunnel: w2648 -> [w2653]
          tunnel: w2644 -> [w2652]
          frame #0 {
            n1413 = property on="Reset R Motor Steps" class="DigNum (strict)"() -> ("Value"=w2654:i32)  [unwired: 2 in, 2 out]
            n1414 = Number To Decimal String(number=w2654) -> (decimal integer string=w2657:string)  [unwired: 1 in]
            n1415 = call "mDrive Send Command.vi"("error in (no error)"=w2653, "Extra"=w2657, "Command"=T10."Set Current Position", "VISA resource name"=w2652) -> ("error out"=w2656:errorcluster, "VISA resource name out"=w2655:refnum<visa-resource-name>)  [unwired: 3 in, 1 out]
          }
        }
        n1416 = flat-sequence {
          tunnel: [w2675] -> _
          tunnel: [w2676] -> _
          tunnel: w2651 -> [w2674]
          tunnel: w2647 -> [w2673]
          frame #0 {
            n1417 = property on="Reset X Motor Steps" class="DigNum (strict)"() -> ("Value"=w2677:i32)  [unwired: 2 in, 2 out]
            n1418 = Number To Decimal String(number=w2677) -> (decimal integer string=w2678:string)  [unwired: 1 in]
            n1419 = call "mDrive Send Command.vi"("error in (no error)"=w2674, "Extra"=w2678, "Command"=T10."Set Current Position", "VISA resource name"=w2673) -> ("error out"=w2676:errorcluster, "VISA resource name out"=w2675:refnum<visa-resource-name>)  [unwired: 3 in, 1 out]
          }
        }
        n1420 = flat-sequence {
          tunnel: [w2669] -> _
          tunnel: [w2670] -> _
          tunnel: w2650 -> [w2667]
          tunnel: w2646 -> [w2666]
          frame #0 {
            n1421 = property on="Reset Z Motor Steps" class="DigNum (strict)"() -> ("Value"=w2668:i32)  [unwired: 2 in, 2 out]
            n1422 = Number To Decimal String(number=w2668) -> (decimal integer string=w2671:string)  [unwired: 1 in]
            n1423 = call "mDrive Send Command.vi"("error in (no error)"=w2667, "Extra"=w2671, "Command"=T10."Set Current Position", "VISA resource name"=w2666) -> ("error out"=w2670:errorcluster, "VISA resource name out"=w2669:refnum<visa-resource-name>)  [unwired: 3 in, 1 out]
          }
        }
        n1424 = flat-sequence {
          tunnel: [w2662] -> _
          tunnel: [w2663] -> _
          tunnel: w2649 -> [w2660]
          tunnel: w2645 -> [w2659]
          frame #0 {
            n1425 = property on="Reset Y Motor Steps" class="DigNum (strict)"() -> ("Value"=w2661:i32)  [unwired: 2 in, 2 out]
            n1426 = Number To Decimal String(number=w2661) -> (decimal integer string=w2664:string)  [unwired: 1 in]
            n1427 = call "mDrive Send Command.vi"("error in (no error)"=w2660, "Extra"=w2664, "Command"=T10."Set Current Position", "VISA resource name"=w2659) -> ("error out"=w2663:errorcluster, "VISA resource name out"=w2662:refnum<visa-resource-name>)  [unwired: 3 in, 1 out]
          }
        }
      }
      event "LOOP": Mouse Up {
        n1428 = event-data() -> ()  [unwired: 1 in, 7 out]
        n1429 = flat-sequence {
          tunnel: w2699 -> [w4285]
          tunnel: [w4285] -> w2698
          tunnel: w2697 -> [w4284]
          tunnel: [w4284] -> w2696
          tunnel: w2695 -> [w4283]
          tunnel: [w4283] -> w2694
          tunnel: w2693 -> [w4282]
          tunnel: [w4282] -> w2692
          tunnel: w2691 -> [w4281]
          tunnel: [w4281] -> w2690
          tunnel: w2689 -> [w4280]
          tunnel: [w4280] -> w2688
          tunnel: w2687 -> [w4279]
          tunnel: [w4279] -> w2686
          tunnel: w2685 -> [w4278]
          tunnel: [w4278] -> w2684
          frame #0 {
            w4286 = T9."Disabled and Grayed Out" ("Disabled")
            n1430 = local write "STATUS"("ENTERING LOOP" ("STATUS")) -> ()
            n1431 = property on="Z Scan Length SP steps" class="DigNum (strict)"("DisabledEnum"=T9."Disabled and Grayed Out" ("Disabled")) -> ()  [unwired: 2 in, 2 out]
            n1432 = property on="Z Scan Velocity SP steps/sec" class="DigNum (strict)"("DisabledEnum"=T9."Disabled and Grayed Out" ("Disabled")) -> ()  [unwired: 2 in, 2 out]
            n1433 = property on="GO" class="Bool"("DisabledEnum"=w4286) -> ()  [unwired: 2 in, 2 out]
            n1434 = property on="Set Scan \nParameters" class="Bool"("DisabledEnum"=w4286) -> ()  [unwired: 2 in, 2 out]
            n1435 = property on="Scan Go" class="Bool (strict)"("DisabledEnum"=w4286) -> ()  [unwired: 2 in, 2 out]
            n1436 = property on="Send scan parameter" class="Bool"("DisabledEnum"=w4286) -> ()  [unwired: 2 in, 2 out]
            n1437 = property on="R Scan Length SP steps" class="DigNum (strict)"("DisabledEnum"=T9."Disabled and Grayed Out" ("Disabled")) -> ()  [unwired: 2 in, 2 out]
            n1438 = property on="R Scan Velocity SP steps/sec" class="DigNum (strict)"("DisabledEnum"=T9."Disabled and Grayed Out" ("Disabled")) -> ()  [unwired: 2 in, 2 out]
            n1439 = property on="Y Scan Length SP steps" class="DigNum (strict)"("DisabledEnum"=T9."Disabled and Grayed Out" ("Disabled")) -> ()  [unwired: 2 in, 2 out]
            n1440 = property on="Y Scan Velocity SP steps/sec" class="DigNum (strict)"("DisabledEnum"=T9."Disabled and Grayed Out" ("Disabled")) -> ()  [unwired: 2 in, 2 out]
            n1441 = property on="X Scan Length SP steps" class="DigNum (strict)"("DisabledEnum"=T9."Disabled and Grayed Out" ("Disabled")) -> ()  [unwired: 2 in, 2 out]
            n1442 = property on="X Scan Velocity SP steps/sec" class="DigNum (strict)"("DisabledEnum"=T9."Disabled and Grayed Out" ("Disabled")) -> ()  [unwired: 2 in, 2 out]
          }
        }
        n1443 = while {
          tunnel: w2694 -> [w2756]
          tunnel: w2690 -> [w2755]
          tunnel: w2692 -> [w2754]
          tunnel: w2688 -> [w2753]
          tunnel: w2686 -> [w2752]
          tunnel: w2684 -> [w2751]
          tunnel: w2696 -> [w2750]
          tunnel: w2698 -> [w2749]
          tunnel: [w2748] -> w2683 mode=indexing
          tunnel: [w2747] -> w2682 mode=indexing
          tunnel: [w2746] -> w2681 mode=indexing
          tunnel: [w2745] -> w2680 mode=indexing
          i -> [w2711]
          stop <- w2700 stop-if-true
          # "XZYR"
          n1444 = flat-sequence {
            tunnel: w2755 -> [w2784]
            tunnel: w2756 -> [w2785]
            tunnel: [w2781] -> w2772
            tunnel: [w2774] -> w2771
            tunnel: [w2780] -> w2770
            tunnel: [w2779] -> w2769
            tunnel: [w2778] -> w2768
            tunnel: [w2777] -> w2767
            tunnel: [w2773] -> w2766
            tunnel: [w2776] -> w2765
            tunnel: w2754 -> [w2789]
            tunnel: w2753 -> [w2788]
            tunnel: w2752 -> [w2787]
            tunnel: w2751 -> [w2786]
            tunnel: w2750 -> [w2783]
            tunnel: w2749 -> [w2782]
            tunnel: [w2919] -> w2728
            tunnel: [w2918] -> w2726
            tunnel: [w2917] -> w2724
            tunnel: [w2916] -> w2722
            tunnel: [w2914] -> w2720
            tunnel: [w2913] -> w2718
            tunnel: [w2915] -> w2716
            tunnel: w2772 -> [w2912]
            tunnel: w2771 -> [w2911]
            tunnel: w2770 -> [w2910]
            tunnel: w2769 -> [w2909]
            tunnel: w2768 -> [w2908]
            tunnel: w2767 -> [w2907]
            tunnel: w2766 -> [w2906]
            tunnel: w2765 -> [w2905]
            tunnel: [w2904] -> w2714
            tunnel: w2728 -> [w3044]
            tunnel: [w3044] -> w2727
            tunnel: w2726 -> [w3043]
            tunnel: [w3043] -> w2725
            tunnel: w2724 -> [w3042]
            tunnel: [w3042] -> w2723
            tunnel: w2722 -> [w3041]
            tunnel: [w3041] -> w2721
            tunnel: w2720 -> [w3040]
            tunnel: [w3040] -> w2719
            tunnel: w2718 -> [w3039]
            tunnel: [w3039] -> w2717
            tunnel: w2716 -> [w3038]
            tunnel: [w3038] -> w2715
            tunnel: w2714 -> [w3037]
            tunnel: [w3037] -> w2713
            tunnel: [w3059] -> w2744
            tunnel: [w3057] -> w2742
            tunnel: [w3050] -> w2740
            tunnel: [w3049] -> w2738
            tunnel: [w3048] -> w2736
            tunnel: [w3047] -> w2734
            tunnel: [w3046] -> w2732
            tunnel: [w3045] -> w2730
            tunnel: w2727 -> [w3060]
            tunnel: w2725 -> [w3058]
            tunnel: w2723 -> [w3055]
            tunnel: w2721 -> [w3054]
            tunnel: w2719 -> [w3052]
            tunnel: w2717 -> [w3051]
            tunnel: w2715 -> [w3053]
            tunnel: w2713 -> [w3056]
            tunnel: w2744 -> [w3339]
            tunnel: [w3339] -> w2743
            tunnel: w2742 -> [w3338]
            tunnel: [w3338] -> w2741
            tunnel: w2740 -> [w3337]
            tunnel: [w3337] -> w2739
            tunnel: w2738 -> [w3336]
            tunnel: [w3336] -> w2737
            tunnel: w2736 -> [w3335]
            tunnel: [w3335] -> w2735
            tunnel: w2734 -> [w3334]
            tunnel: [w3334] -> w2733
            tunnel: w2732 -> [w3333]
            tunnel: [w3333] -> w2731
            tunnel: w2730 -> [w3332]
            tunnel: [w3332] -> w2729
            tunnel: w2743 -> [w3357]
            tunnel: w2741 -> [w3355]
            tunnel: w2739 -> [w3356]
            tunnel: w2737 -> [w3354]
            tunnel: w2735 -> [w3353]
            tunnel: w2733 -> [w3352]
            tunnel: w2731 -> [w3351]
            tunnel: w2729 -> [w3350]
            tunnel: [w3349] -> w2764
            tunnel: [w3348] -> w2763
            tunnel: [w3347] -> w2762
            tunnel: [w3346] -> w2761
            tunnel: [w3345] -> w2760
            tunnel: [w3344] -> w2759
            tunnel: [w3343] -> w2758
            tunnel: [w3342] -> w2757
            tunnel: w2764 -> [w3650]
            tunnel: w2763 -> [w3651]
            tunnel: w2762 -> [w3653]
            tunnel: w2761 -> [w3652]
            tunnel: w2760 -> [w3656]
            tunnel: w2759 -> [w3657]
            tunnel: w2758 -> [w3654]
            tunnel: w2757 -> [w3655]
            tunnel: [w3659] -> w2710
            tunnel: [w3658] -> w2709
            tunnel: [w3660] -> w2708
            tunnel: [w3661] -> w2707
            tunnel: [w3664] -> w2706
            tunnel: [w3665] -> w2705
            tunnel: [w3662] -> w2704
            tunnel: [w3663] -> w2703
            tunnel: [w4257] -> _
            tunnel: [w4258] -> w2748
            tunnel: [w4259] -> _
            tunnel: [w4260] -> w2747
            tunnel: [w4261] -> _
            tunnel: [w4262] -> w2745
            tunnel: [w4263] -> w2746
            tunnel: [w4264] -> _
            tunnel: w2710 -> [w4264]
            tunnel: w2709 -> [w4263]
            tunnel: w2708 -> [w4262]
            tunnel: w2707 -> [w4261]
            tunnel: w2706 -> [w4260]
            tunnel: w2705 -> [w4259]
            tunnel: w2704 -> [w4258]
            tunnel: w2703 -> [w4257]
            frame #0 {
              n1445 = flat-sequence {
                tunnel: [w2881] -> w2813
                tunnel: [w2880] -> w2812
                tunnel: w2784 -> [w2883]
                tunnel: w2785 -> [w2882]
                tunnel: w2813 -> [w2889]
                tunnel: [w2889] -> w2811
                tunnel: w2812 -> [w2888]
                tunnel: [w2888] -> w2810
                tunnel: w2811 -> [w2893]
                tunnel: [w2892] -> w2809
                tunnel: w2810 -> [w2891]
                tunnel: [w2890] -> w2808
                tunnel: w2809 -> [w2901]
                tunnel: w2808 -> [w2899]
                tunnel: [w2901] -> w2781
                tunnel: [w2899] -> w2774
                frame #0 {
                  n1446 = property on="X Scan Velocity SP steps/sec" class="DigNum (strict)"() -> ("Value"=w2885:i32)  [unwired: 2 in, 2 out]
                  n1447 = Number To Decimal String(number=w2885) -> (decimal integer string=w2886:string)  [unwired: 1 in]
                  n1448 = call "mDrive Send Command.vi"("error in (no error)"=w2883, "Extra"=w2886, "Command"=T10."Max Velocity", "VISA resource name"=w2882) -> ("error out"=w2880:errorcluster, "VISA resource name out"=w2881:refnum<visa-resource-name>)  [unwired: 3 in, 1 out]
                }
                frame #1 {
                  n1449 = Wait (ms)(milliseconds to wait=u32 100) -> ()  [unwired: 1 out]
                }
                frame #2 {
                  # "VELOCITY"
                  n1450 = call "mDrive Send Command.vi"("error in (no error)"=w2891, "Extra"="VM", "Command"=T10."Print Parameter", "VISA resource name"=w2893) -> ("error out"=w2890:errorcluster, "read buffer"=w2896:string, "VISA resource name out"=w2892:refnum<visa-resource-name>)  [unwired: 3 in]
                  n1451 = Decimal String To Number(string=w2896, offset=0) -> (number=w2894:i32)  [unwired: 1 in, 1 out]
                  n1452 = property on="X velocity PV step/sec" class="DigNum (strict)"("Val(Sgnl)"=w2894) -> ()  [unwired: 2 in, 2 out]
                }
                frame #3 {
                  n1453 = Wait (ms)(milliseconds to wait=u32 100) -> ()  [unwired: 1 out]
                }
              }
              n1454 = flat-sequence {
                tunnel: [w2839] -> w2801
                tunnel: [w2838] -> w2800
                tunnel: w2788 -> [w2837]
                tunnel: w2789 -> [w2836]
                tunnel: w2801 -> [w2845]
                tunnel: [w2845] -> w2799
                tunnel: w2800 -> [w2844]
                tunnel: [w2844] -> w2798
                tunnel: w2799 -> [w2851]
                tunnel: [w2850] -> w2797
                tunnel: w2798 -> [w2849]
                tunnel: [w2848] -> w2796
                tunnel: w2797 -> [w2857]
                tunnel: w2796 -> [w2856]
                tunnel: [w2857] -> w2780
                tunnel: [w2856] -> w2779
                frame #0 {
                  n1455 = property on="Z Scan Velocity SP steps/sec" class="DigNum (strict)"() -> ("Value"=w2841:i32)  [unwired: 2 in, 2 out]
                  n1456 = Number To Decimal String(number=w2841) -> (decimal integer string=w2842:string)  [unwired: 1 in]
                  n1457 = call "mDrive Send Command.vi"("error in (no error)"=w2837, "Extra"=w2842, "Command"=T10."Max Velocity", "VISA resource name"=w2836) -> ("error out"=w2838:errorcluster, "VISA resource name out"=w2839:refnum<visa-resource-name>)  [unwired: 3 in, 1 out]
                }
                frame #1 {
                  n1458 = Wait (ms)(milliseconds to wait=u32 100) -> ()  [unwired: 1 out]
                }
                frame #2 {
                  # "VELOCITY"
                  n1459 = call "mDrive Send Command.vi"("error in (no error)"=w2849, "Extra"="VM", "Command"=T10."Print Parameter", "VISA resource name"=w2851) -> ("error out"=w2848:errorcluster, "read buffer"=w2852:string, "VISA resource name out"=w2850:refnum<visa-resource-name>)  [unwired: 3 in]
                  n1460 = Decimal String To Number(string=w2852, offset=0) -> (number=w2853:i32)  [unwired: 1 in, 1 out]
                  n1461 = property on="Z  velocity PV step/sec" class="DigNum (strict)"("Val(Sgnl)"=w2853) -> ()  [unwired: 2 in, 2 out]
                }
                frame #3 {
                  n1462 = Wait (ms)(milliseconds to wait=u32 100) -> ()  [unwired: 1 out]
                }
              }
              n1463 = flat-sequence {
                tunnel: [w2861] -> w2807
                tunnel: [w2860] -> w2806
                tunnel: w2786 -> [w2859]
                tunnel: w2787 -> [w2858]
                tunnel: w2807 -> [w2867]
                tunnel: [w2867] -> w2805
                tunnel: w2806 -> [w2866]
                tunnel: [w2866] -> w2804
                tunnel: w2805 -> [w2871]
                tunnel: [w2870] -> w2803
                tunnel: w2804 -> [w2869]
                tunnel: [w2868] -> w2802
                tunnel: w2803 -> [w2879]
                tunnel: w2802 -> [w2878]
                tunnel: [w2879] -> w2778
                tunnel: [w2878] -> w2777
                frame #0 {
                  n1464 = property on="Y Scan Velocity SP steps/sec" class="DigNum (strict)"() -> ("Value"=w2863:i32)  [unwired: 2 in, 2 out]
                  n1465 = Number To Decimal String(number=w2863) -> (decimal integer string=w2864:string)  [unwired: 1 in]
                  n1466 = call "mDrive Send Command.vi"("error in (no error)"=w2859, "Extra"=w2864, "Command"=T10."Max Velocity", "VISA resource name"=w2858) -> ("error out"=w2860:errorcluster, "VISA resource name out"=w2861:refnum<visa-resource-name>)  [unwired: 3 in, 1 out]
                }
                frame #1 {
                  n1467 = Wait (ms)(milliseconds to wait=u32 100) -> ()  [unwired: 1 out]
                }
                frame #2 {
                  # "VELOCITY"
                  n1468 = call "mDrive Send Command.vi"("error in (no error)"=w2869, "Extra"="VM", "Command"=T10."Print Parameter", "VISA resource name"=w2871) -> ("error out"=w2868:errorcluster, "read buffer"=w2875:string, "VISA resource name out"=w2870:refnum<visa-resource-name>)  [unwired: 3 in]
                  n1469 = Decimal String To Number(string=w2875, offset=0) -> (number=w2873:i32)  [unwired: 1 in, 1 out]
                  n1470 = property on="Y velocity PV step/sec" class="DigNum (strict)"("Val(Sgnl)"=w2873) -> ()  [unwired: 2 in, 2 out]
                }
                frame #3 {
                  n1471 = Wait (ms)(milliseconds to wait=u32 100) -> ()  [unwired: 1 out]
                }
              }
              n1472 = flat-sequence {
                tunnel: [w2817] -> w2795
                tunnel: [w2816] -> w2794
                tunnel: w2783 -> [w2815]
                tunnel: w2782 -> [w2814]
                tunnel: w2795 -> [w2823]
                tunnel: [w2823] -> w2793
                tunnel: w2794 -> [w2822]
                tunnel: [w2822] -> w2792
                tunnel: w2793 -> [w2829]
                tunnel: [w2828] -> w2791
                tunnel: w2792 -> [w2827]
                tunnel: [w2826] -> w2790
                tunnel: w2791 -> [w2833]
                tunnel: w2790 -> [w2835]
                tunnel: [w2835] -> w2776
                tunnel: [w2833] -> w2773
                frame #0 {
                  n1473 = property on="R Scan Velocity SP steps/sec" class="DigNum (strict)"() -> ("Value"=w2819:i32)  [unwired: 2 in, 2 out]
                  n1474 = Number To Decimal String(number=w2819) -> (decimal integer string=w2820:string)  [unwired: 1 in]
                  n1475 = call "mDrive Send Command.vi"("error in (no error)"=w2815, "Extra"=w2820, "Command"=T10."Max Velocity", "VISA resource name"=w2814) -> ("error out"=w2816:errorcluster, "VISA resource name out"=w2817:refnum<visa-resource-name>)  [unwired: 3 in, 1 out]
                }
                frame #1 {
                  n1476 = Wait (ms)(milliseconds to wait=u32 100) -> ()  [unwired: 1 out]
                }
                frame #2 {
                  # "VELOCITY"
                  n1477 = call "mDrive Send Command.vi"("error in (no error)"=w2827, "Extra"="VM", "Command"=T10."Print Parameter", "VISA resource name"=w2829) -> ("error out"=w2826:errorcluster, "read buffer"=w2831:string, "VISA resource name out"=w2828:refnum<visa-resource-name>)  [unwired: 3 in]
                  n1478 = Decimal String To Number(string=w2831, offset=0) -> (number=w2830:i32)  [unwired: 1 in, 1 out]
                  n1479 = property on="R velocity PV step/sec" class="DigNum (strict)"("Val(Sgnl)"=w2830) -> ()  [unwired: 2 in, 2 out]
                }
                frame #3 {
                  n1480 = Wait (ms)(milliseconds to wait=u32 100) -> ()  [unwired: 1 out]
                }
              }
              n1481 = local write "STATUS"("LOOP INITIALIZING" ("STATUS")) -> ()
            }
            frame #1 {
              w2902 = TRUE ("R in Motion")
              n1482 = flat-sequence {
                tunnel: [w2979] -> w2947
                tunnel: [w2978] -> w2946
                tunnel: [w2977] -> w2945
                tunnel: [w2976] -> w2944
                tunnel: w2912 -> [w2975]
                tunnel: w2911 -> [w2974]
                tunnel: w2910 -> [w2973]
                tunnel: w2909 -> [w2972]
                tunnel: w2908 -> [w2971]
                tunnel: w2907 -> [w2970]
                tunnel: w2906 -> [w2969]
                tunnel: w2905 -> [w2968]
                tunnel: [w2975] -> w2943
                tunnel: [w2974] -> w2942
                tunnel: [w2973] -> w2941
                tunnel: [w2972] -> w2940
                tunnel: [w2971] -> w2939
                tunnel: [w2970] -> w2938
                tunnel: [w2969] -> w2937
                tunnel: [w2968] -> w2936
                tunnel: [w2999] -> w2935
                tunnel: [w2998] -> w2934
                tunnel: w2947 -> [w2997]
                tunnel: w2946 -> [w2996]
                tunnel: w2945 -> [w2995]
                tunnel: w2944 -> [w2994]
                tunnel: [w2993] -> w2933
                tunnel: [w2992] -> w2932
                tunnel: [w2991] -> w2931
                tunnel: [w2990] -> w2930
                tunnel: [w2989] -> w2929
                tunnel: [w2988] -> w2928
                tunnel: w2943 -> [w2987]
                tunnel: w2942 -> [w2986]
                tunnel: w2941 -> [w2985]
                tunnel: w2940 -> [w2984]
                tunnel: w2939 -> [w2983]
                tunnel: w2938 -> [w2982]
                tunnel: w2937 -> [w2981]
                tunnel: w2936 -> [w2980]
                tunnel: w2935 -> [w3008]
                tunnel: [w3008] -> w2927
                tunnel: w2934 -> [w3007]
                tunnel: [w3007] -> w2926
                tunnel: [w3006] -> w2925
                tunnel: w2933 -> [w3006]
                tunnel: [w3005] -> w2924
                tunnel: w2932 -> [w3005]
                tunnel: [w3004] -> w2923
                tunnel: w2931 -> [w3004]
                tunnel: [w3003] -> w2922
                tunnel: w2930 -> [w3003]
                tunnel: [w3002] -> w2921
                tunnel: w2929 -> [w3002]
                tunnel: [w3001] -> w2920
                tunnel: w2928 -> [w3001]
                tunnel: w2927 -> [w3036]
                tunnel: w2926 -> [w3035]
                tunnel: w2925 -> [w3032]
                tunnel: w2924 -> [w3031]
                tunnel: w2923 -> [w3030]
                tunnel: w2922 -> [w3029]
                tunnel: w2921 -> [w3028]
                tunnel: w2920 -> [w3027]
                tunnel: [w3034] -> w2916
                tunnel: [w3033] -> w2915
                tunnel: [w3026] -> w2917
                tunnel: [w3025] -> w2914
                tunnel: [w3024] -> w2913
                tunnel: [w3023] -> w2919
                tunnel: [w3022] -> w2918
                tunnel: [w3009] -> w2904
                frame #0 {
                  n1483 = property on="X Scan Length SP steps" class="DigNum (strict)"() -> ("Value"=w2962:i32)  [unwired: 2 in, 2 out]
                  n1484 = property on="Z Scan Length SP steps" class="DigNum (strict)"() -> ("Value"=w2967:i32)  [unwired: 2 in, 2 out]
                  n1485 = property on="Y Scan Length SP steps" class="DigNum (strict)"() -> ("Value"=w2957:i32)  [unwired: 2 in, 2 out]
                  n1486 = property on="R Scan Length SP steps" class="DigNum (strict)"() -> ("Value"=w2952:i32)  [unwired: 2 in, 2 out]
                  n1487 = Number To Decimal String(number=w2962) -> (decimal integer string=w2959:string)  [unwired: 1 in]
                  n1488 = Number To Decimal String(number=w2967) -> (decimal integer string=w2964:string)  [unwired: 1 in]
                  n1489 = Number To Decimal String(number=w2957) -> (decimal integer string=w2954:string)  [unwired: 1 in]
                  n1490 = Number To Decimal String(number=w2952) -> (decimal integer string=w2949:string)  [unwired: 1 in]
                  n1491 = call <vilib>:"Space Constant.vi"() -> ("String"=w2960:string)
                  n1492 = call <vilib>:"Space Constant.vi"() -> ("String"=w2965:string)
                  n1493 = call <vilib>:"Space Constant.vi"() -> ("String"=w2955:string)
                  n1494 = call <vilib>:"Space Constant.vi"() -> ("String"=w2950:string)
                  n1495 = Concatenate Strings("MR", w2960, w2959, "\r") -> (w2978:string)
                  n1496 = Concatenate Strings("MR", w2965, w2964, "\r") -> (w2977:string)
                  n1497 = Concatenate Strings("MR", w2955, w2954, "\r") -> (w2979:string)
                  n1498 = Concatenate Strings("MR", w2950, w2949, "\r") -> (w2976:string)
                }
                frame #1 {
                  n1499 = VISA Write(VISA resource name=w2987, write buffer=w2996, error in (no error)=w2986) -> (VISA resource name out=w2993:refnum<visa-resource-name>, error out=w2992:errorcluster)  [unwired: 1 out]
                  n1500 = VISA Write(VISA resource name=w2985, write buffer=w2995, error in (no error)=w2984) -> (VISA resource name out=w2989:refnum<visa-resource-name>, error out=w2988:errorcluster)  [unwired: 1 out]
                  n1501 = VISA Write(VISA resource name=w2983, write buffer=w2997, error in (no error)=w2982) -> (VISA resource name out=w2999:refnum<visa-resource-name>, error out=w2998:errorcluster)  [unwired: 1 out]
                  n1502 = VISA Write(VISA resource name=w2981, write buffer=w2994, error in (no error)=w2980) -> (VISA resource name out=w2991:refnum<visa-resource-name>, error out=w2990:errorcluster)  [unwired: 1 out]
                }
                frame #2 {
                  n1503 = Wait (ms)(milliseconds to wait=u32 100) -> ()  [unwired: 1 out]
                }
                frame #3 {
                  n1504 = property class="Instr"(reference=w3032, error in=w3031) -> (reference out=w3014:refnum<visa-resource-name>, error out=w3013:errorcluster, "Serial Settings:Number of Bytes at Serial Port"=w3015:u32)
                  n1505 = property class="Instr"(reference=w3028, error in=w3027) -> (reference out=w3011:refnum<visa-resource-name>, error out=w3010:errorcluster, "Serial Settings:Number of Bytes at Serial Port"=w3012:u32)
                  n1506 = property class="Instr"(reference=w3036, error in=w3035) -> (reference out=w3017:refnum<visa-resource-name>, error out=w3016:errorcluster, "Serial Settings:Number of Bytes at Serial Port"=w3018:u32)
                  n1507 = property class="Instr"(reference=w3030, error in=w3029) -> (reference out=w3020:refnum<visa-resource-name>, error out=w3019:errorcluster, "Serial Settings:Number of Bytes at Serial Port"=w3021:u32)
                  n1508 = VISA Read(VISA resource name=w3014, byte count=w3015, error in (no error)=w3013) -> (VISA resource name out=w3023:refnum<visa-resource-name>, error out=w3022:errorcluster)  [unwired: 2 out]
                  n1509 = VISA Read(VISA resource name=w3011, byte count=w3012, error in (no error)=w3010) -> (VISA resource name out=w3009:refnum<visa-resource-name>, error out=w3026:errorcluster)  [unwired: 2 out]
                  n1510 = VISA Read(VISA resource name=w3017, byte count=w3018, error in (no error)=w3016) -> (VISA resource name out=w3034:refnum<visa-resource-name>, error out=w3033:errorcluster)  [unwired: 2 out]
                  n1511 = VISA Read(VISA resource name=w3020, byte count=w3021, error in (no error)=w3019) -> (VISA resource name out=w3025:refnum<visa-resource-name>, error out=w3024:errorcluster)  [unwired: 2 out]
                }
              }
              n1512 = local write "STATUS"("LOOP SCANNING" ("STATUS")) -> ()
              n1513 = property on="Y in Motion" class="Bool (strict)"("Value"=w2902) -> ()  [unwired: 2 in, 2 out]
              n1514 = property on="Z in Motion" class="Bool (strict)"("Value"=w2902) -> ()  [unwired: 2 in, 2 out]
              n1515 = property on="X  in Motion" class="Bool (strict)"("Value"=w2902) -> ()  [unwired: 2 in, 2 out]
              n1516 = property on="R in Motion" class="Bool (strict)"("Value"=w2902) -> ()  [unwired: 2 in, 2 out]
            }
            frame #2 {
            }
            frame #3 {
              n1517 = while {
                tunnel: w3060 -> [w3082]
                tunnel: [w3070] -> w3059
                tunnel: w3058 -> [w3081]
                tunnel: [w3069] -> w3057
                tunnel: w3056 -> [w3080]
                tunnel: w3055 -> [w3079]
                tunnel: w3054 -> [w3078]
                tunnel: w3053 -> [w3077]
                tunnel: w3052 -> [w3076]
                tunnel: w3051 -> [w3075]
                tunnel: [w3072] -> w3050
                tunnel: [w3071] -> w3049
                tunnel: [w3068] -> w3048
                tunnel: [w3067] -> w3047
                tunnel: [w3066] -> w3046
                tunnel: [w3065] -> w3045
                stop <- w3061 stop-if-true
                n1518 = flat-sequence {
                  tunnel: [w3283] -> w3118
                  tunnel: [w3282] -> w3117
                  tunnel: [w3281] -> w3116
                  tunnel: w3082 -> [w3280]
                  tunnel: w3081 -> [w3279]
                  tunnel: [w3305] -> w3115
                  tunnel: [w3304] -> w3114
                  tunnel: [w3302] -> w3113
                  tunnel: w3118 -> [w3302]
                  tunnel: w3117 -> [w3301]
                  tunnel: w3116 -> [w3300]
                  tunnel: w3115 -> [w3318]
                  tunnel: [w3318] -> w3110
                  tunnel: w3114 -> [w3317]
                  tunnel: [w3317] -> w3111
                  tunnel: w3113 -> [w3316]
                  tunnel: [w3316] -> w3112
                  tunnel: w3112 -> [w3321]
                  tunnel: w3111 -> [w3323]
                  tunnel: w3110 -> [w3322]
                  tunnel: [w3320] -> w3070
                  tunnel: [w3319] -> w3069
                  frame #0 {
                    n1519 = property on="X Step SP" class="DigNum (strict)"() -> ("Maximum"=w3295:dbl)  [unwired: 2 in, 2 out]
                    n1520 = property on="X Step SP" class="DigNum (strict)"() -> ("Minimum"=w3297:dbl)  [unwired: 2 in, 2 out]
                    n1521 = property on="X steps/rev" class="DigNum (strict)"() -> ("Value"=w3292:u32)  [unwired: 2 in, 2 out]
                    n1522 = property on="X offset mm" class="DigNum (strict)"() -> ("Value"=w3288:dbl)  [unwired: 2 in, 2 out]
                    n1523 = To Long Integer(number=w3295) -> (32bit integer=w3294:i32)
                    n1524 = To Long Integer(number=w3297) -> (32bit integer=w3296:i32)
                    n1525 = To Double Precision Float(number=w3292) -> (double precision float=w3293:dbl)
                    n1526 = call "mDrive Send Command.vi"("error in (no error)"=w3279, "Extra"="P", "Command"=T10."Print Parameter", "VISA resource name"=w3280) -> ("error out"=w3281:errorcluster, "read buffer"=w3299:string, "VISA resource name out"=w3282:refnum<visa-resource-name>)  [unwired: 3 in]
                    n1527 = Decimal String To Number(string=w3299, offset=0) -> (number=w3278:i32)  [unwired: 1 in, 1 out]
                    n1528 = property on="X Step PV" class="DigNum (strict)"("Val(Sgnl)"=w3278) -> ()  [unwired: 2 in, 2 out]
                    n1529 = In Range and Coerce(upper limit=w3294, x=w3278, lower limit=w3296) -> (In Range?=w3283:bool)  [unwired: 1 out]
                    n1530 = To Double Precision Float(number=w3278) -> (double precision float=w3287:dbl)
                    n1531 = property on="X  in Range" class="Bool (strict)"("Val(Sgnl)"=w3283) -> ()  [unwired: 2 in, 2 out]
                    n1532 = Divide(x=w3287, y=w3293) -> (x/y=w3291:dbl)
                    n1533 = property on="X mm/rev" class="DigNum (strict)"() -> ("Value"=w3290:dbl)  [unwired: 2 in, 2 out]
                    n1534 = Multiply(x=w3291, y=w3290) -> (x*y=w3289:dbl)
                    n1535 = Add(x=w3289, y=w3288) -> (x+y=w3286:dbl)
                    n1536 = property on="X Position mm PV" class="DigNum (strict)"("Val(Sgnl)"=w3286) -> ()  [unwired: 2 in, 2 out]
                  }
                  frame #1 {
                    n1537 = call "mDrive Send Command.vi"("error in (no error)"=w3300, "Extra"="MV", "Command"=T10."Print Parameter", "VISA resource name"=w3301) -> ("error out"=w3304:errorcluster, "read buffer"=w3308:string, "VISA resource name out"=w3305:refnum<visa-resource-name>)  [unwired: 3 in]
                    n1538 = Decimal String To Number(string=w3308, offset=0 ("offset (0)")) -> (number=w3311:i32)  [unwired: 1 in, 1 out]
                    n1539 = Not Equal?(x=w3308, y="") -> (x != y?=w3306:bool)
                    n1540 = property on="X Ready" class="Bool (strict)"("Val(Sgnl)"=w3306) -> ()  [unwired: 2 in, 2 out]
                    n1541 = Number To Boolean Array(number=w3311) -> (Boolean array=w3310:bool[])
                    n1542 = Index Array(array=w3310, index=0) -> (element=w3303:bool)
                    n1543 = property on="X  in Motion" class="Bool (strict)"("Val(Sgnl)"=w3303) -> ()  [unwired: 2 in, 2 out]
                  }
                  frame #2 {
                    n1544 = Wait (ms)(milliseconds to wait=u32 10) -> ()  [unwired: 1 out]
                  }
                  frame #3 {
                    n1545 = case shown="False" w3321 {
                      tunnel: w3322 -> [w3326 w3330]
                      tunnel: [w3327 w3330] -> w3320
                      tunnel: [w3328 w3329] -> w3319
                      tunnel: w3323 -> [w3325 w3329]
                      frame False {
                        n1546 = call "mDrive Send Command.vi"("error in (no error)"=w3325, "Command"=T10."Stop", "VISA resource name"=w3326) -> ("error out"=w3328:errorcluster, "VISA resource name out"=w3327:refnum<visa-resource-name>)  [unwired: 4 in, 1 out]
                      }
                      frame True {
                      }
                    }
                  }
                }
                n1547 = flat-sequence {
                  tunnel: [w3236] -> w3109
                  tunnel: [w3227] -> w3108
                  tunnel: [w3226] -> w3107
                  tunnel: w3080 -> [w3230]
                  tunnel: w3079 -> [w3229]
                  tunnel: [w3256] -> w3106
                  tunnel: [w3255] -> w3105
                  tunnel: [w3254] -> w3104
                  tunnel: w3109 -> [w3254]
                  tunnel: w3108 -> [w3253]
                  tunnel: w3107 -> [w3252]
                  tunnel: w3106 -> [w3265]
                  tunnel: [w3265] -> w3101
                  tunnel: w3105 -> [w3264]
                  tunnel: [w3264] -> w3102
                  tunnel: w3104 -> [w3263]
                  tunnel: [w3263] -> w3103
                  tunnel: w3103 -> [w3268]
                  tunnel: w3102 -> [w3270]
                  tunnel: w3101 -> [w3269]
                  tunnel: [w3267] -> w3072
                  tunnel: [w3266] -> w3071
                  frame #0 {
                    n1548 = property on="Z Step SP" class="DigNum (strict)"() -> ("Maximum"=w3237:dbl)  [unwired: 2 in, 2 out]
                    n1549 = property on="Z Step SP" class="DigNum (strict)"() -> ("Minimum"=w3231:dbl)  [unwired: 2 in, 2 out]
                    n1550 = property on="Z steps/rev" class="DigNum (strict)"() -> ("Value"=w3235:u32)  [unwired: 2 in, 2 out]
                    n1551 = property on="Z offset mm" class="DigNum (strict)"() -> ("Value"=w3233:dbl)  [unwired: 2 in, 2 out]
                    n1552 = To Long Integer(number=w3237) -> (32bit integer=w3243:i32)
                    n1553 = To Long Integer(number=w3231) -> (32bit integer=w3244:i32)
                    n1554 = To Double Precision Float(number=w3235) -> (double precision float=w3242:dbl)
                    n1555 = call "mDrive Send Command.vi"("error in (no error)"=w3229, "Extra"="P", "Command"=T10."Print Parameter", "VISA resource name"=w3230) -> ("error out"=w3226:errorcluster, "read buffer"=w3246:string, "VISA resource name out"=w3227:refnum<visa-resource-name>)  [unwired: 3 in]
                    n1556 = Decimal String To Number(string=w3246, offset=0) -> (number=w3225:i32)  [unwired: 1 in, 1 out]
                    n1557 = property on="Z Step PV" class="DigNum (strict)"("Val(Sgnl)"=w3225) -> ()  [unwired: 2 in, 2 out]
                    n1558 = In Range and Coerce(upper limit=w3243, x=w3225, lower limit=w3244) -> (In Range?=w3236:bool)  [unwired: 1 out]
                    n1559 = To Double Precision Float(number=w3225) -> (double precision float=w3240:dbl)
                    n1560 = property on="Z in Range" class="Bool (strict)"("Val(Sgnl)"=w3236) -> ()  [unwired: 2 in, 2 out]
                    n1561 = Divide(x=w3240, y=w3242) -> (x/y=w3241:dbl)
                    n1562 = property on="Z mm/rev" class="DigNum (strict)"() -> ("Value"=w3234:dbl)  [unwired: 2 in, 2 out]
                    n1563 = Multiply(x=w3241, y=w3234) -> (x*y=w3228:dbl)
                    n1564 = Add(x=w3228, y=w3233) -> (x+y=w3232:dbl)
                    n1565 = property on="Z Position mm PV" class="DigNum (strict)"("Val(Sgnl)"=w3232) -> ()  [unwired: 2 in, 2 out]
                  }
                  frame #1 {
                    n1566 = call "mDrive Send Command.vi"("error in (no error)"=w3252, "Extra"="MV", "Command"=T10."Print Parameter", "VISA resource name"=w3253) -> ("error out"=w3255:errorcluster, "read buffer"=w3258:string, "VISA resource name out"=w3256:refnum<visa-resource-name>)  [unwired: 3 in]
                    n1567 = Decimal String To Number(string=w3258, offset=0 ("offset (0)")) -> (number=w3248:i32)  [unwired: 1 in, 1 out]
                    n1568 = Not Equal?(x=w3258, y="") -> (x != y?=w3251:bool)
                    n1569 = property on="Z Ready" class="Bool (strict)"("Val(Sgnl)"=w3251) -> ()  [unwired: 2 in, 2 out]
                    n1570 = Number To Boolean Array(number=w3248) -> (Boolean array=w3250:bool[])
                    n1571 = Index Array(array=w3250, index=0) -> (element=w3247:bool)
                    n1572 = property on="Z in Motion" class="Bool (strict)"("Val(Sgnl)"=w3247) -> ()  [unwired: 2 in, 2 out]
                  }
                  frame #2 {
                    n1573 = Wait (ms)(milliseconds to wait=u32 10) -> ()  [unwired: 1 out]
                  }
                  frame #3 {
                    n1574 = case shown="False" w3268 {
                      tunnel: w3269 -> [w3273 w3277]
                      tunnel: [w3274 w3277] -> w3267
                      tunnel: [w3275 w3276] -> w3266
                      tunnel: w3270 -> [w3272 w3276]
                      frame False {
                        n1575 = call "mDrive Send Command.vi"("error in (no error)"=w3272, "Command"=T10."Stop", "VISA resource name"=w3273) -> ("error out"=w3275:errorcluster, "VISA resource name out"=w3274:refnum<visa-resource-name>)  [unwired: 4 in, 1 out]
                      }
                      frame True {
                      }
                    }
                  }
                }
                n1576 = flat-sequence {
                  tunnel: [w3181] -> w3100
                  tunnel: [w3183] -> w3099
                  tunnel: [w3182] -> w3098
                  tunnel: w3078 -> [w3174]
                  tunnel: w3077 -> [w3173]
                  tunnel: [w3203] -> w3097
                  tunnel: [w3202] -> w3096
                  tunnel: [w3201] -> w3095
                  tunnel: w3100 -> [w3201]
                  tunnel: w3099 -> [w3200]
                  tunnel: w3098 -> [w3199]
                  tunnel: w3097 -> [w3212]
                  tunnel: [w3212] -> w3092
                  tunnel: w3096 -> [w3211]
                  tunnel: [w3211] -> w3093
                  tunnel: w3095 -> [w3210]
                  tunnel: [w3210] -> w3094
                  tunnel: w3094 -> [w3215]
                  tunnel: w3093 -> [w3217]
                  tunnel: w3092 -> [w3216]
                  tunnel: [w3213] -> w3068
                  tunnel: [w3214] -> w3067
                  frame #0 {
                    n1577 = property on="Y Step SP" class="DigNum (strict)"() -> ("Maximum"=w3176:dbl)  [unwired: 2 in, 2 out]
                    n1578 = property on="Y Step SP" class="DigNum (strict)"() -> ("Minimum"=w3175:dbl)  [unwired: 2 in, 2 out]
                    n1579 = property on="Y steps/rev" class="DigNum (strict)"() -> ("Value"=w3177:u32)  [unwired: 2 in, 2 out]
                    n1580 = property on="Y offset mm" class="DigNum (strict)"() -> ("Value"=w3179:dbl)  [unwired: 2 in, 2 out]
                    n1581 = To Long Integer(number=w3176) -> (32bit integer=w3190:i32)
                    n1582 = To Long Integer(number=w3175) -> (32bit integer=w3191:i32)
                    n1583 = To Double Precision Float(number=w3177) -> (double precision float=w3189:dbl)
                    n1584 = call "mDrive Send Command.vi"("error in (no error)"=w3173, "Extra"="P", "Command"=T10."Print Parameter", "VISA resource name"=w3174) -> ("error out"=w3182:errorcluster, "read buffer"=w3193:string, "VISA resource name out"=w3183:refnum<visa-resource-name>)  [unwired: 3 in]
                    n1585 = Decimal String To Number(string=w3193, offset=0) -> (number=w3172:i32)  [unwired: 1 in, 1 out]
                    n1586 = property on="Y Step PV" class="DigNum (strict)"("Val(Sgnl)"=w3172) -> ()  [unwired: 2 in, 2 out]
                    n1587 = In Range and Coerce(upper limit=w3190, x=w3172, lower limit=w3191) -> (In Range?=w3181:bool)  [unwired: 1 out]
                    n1588 = To Double Precision Float(number=w3172) -> (double precision float=w3186:dbl)
                    n1589 = property on="Y in Range" class="Bool (strict)"("Val(Sgnl)"=w3181) -> ()  [unwired: 2 in, 2 out]
                    n1590 = Divide(x=w3186, y=w3189) -> (x/y=w3188:dbl)
                    n1591 = property on="Y mm/rev" class="DigNum (strict)"() -> ("Value"=w3178:dbl)  [unwired: 2 in, 2 out]
                    n1592 = Multiply(x=w3188, y=w3178) -> (x*y=w3187:dbl)
                    n1593 = Add(x=w3187, y=w3179) -> (x+y=w3180:dbl)
                    n1594 = property on="Y Position mm PV" class="DigNum (strict)"("Val(Sgnl)"=w3180) -> ()  [unwired: 2 in, 2 out]
                  }
                  frame #1 {
                    n1595 = call "mDrive Send Command.vi"("error in (no error)"=w3199, "Extra"="MV", "Command"=T10."Print Parameter", "VISA resource name"=w3200) -> ("error out"=w3202:errorcluster, "read buffer"=w3205:string, "VISA resource name out"=w3203:refnum<visa-resource-name>)  [unwired: 3 in]
                    n1596 = Decimal String To Number(string=w3205, offset=0 ("offset (0)")) -> (number=w3195:i32)  [unwired: 1 in, 1 out]
                    n1597 = Not Equal?(x=w3205, y="") -> (x != y?=w3198:bool)
                    n1598 = property on="Y Ready" class="Bool (strict)"("Val(Sgnl)"=w3198) -> ()  [unwired: 2 in, 2 out]
                    n1599 = Number To Boolean Array(number=w3195) -> (Boolean array=w3197:bool[])
                    n1600 = Index Array(array=w3197, index=0) -> (element=w3194:bool)
                    n1601 = property on="Y in Motion" class="Bool (strict)"("Val(Sgnl)"=w3194) -> ()  [unwired: 2 in, 2 out]
                  }
                  frame #2 {
                    n1602 = Wait (ms)(milliseconds to wait=u32 10) -> ()  [unwired: 1 out]
                  }
                  frame #3 {
                    n1603 = case shown="False" w3215 {
                      tunnel: w3216 -> [w3220 w3223]
                      tunnel: [w3221 w3223] -> w3213
                      tunnel: [w3222 w3224] -> w3214
                      tunnel: w3217 -> [w3219 w3224]
                      frame False {
                        n1604 = call "mDrive Send Command.vi"("error in (no error)"=w3219, "Command"=T10."Stop", "VISA resource name"=w3220) -> ("error out"=w3222:errorcluster, "VISA resource name out"=w3221:refnum<visa-resource-name>)  [unwired: 4 in, 1 out]
                      }
                      frame True {
                      }
                    }
                  }
                }
                n1605 = flat-sequence {
                  tunnel: [w3128] -> w3091
                  tunnel: [w3130] -> w3090
                  tunnel: [w3129] -> w3089
                  tunnel: w3076 -> [w3121]
                  tunnel: w3075 -> [w3120]
                  tunnel: [w3150] -> w3088
                  tunnel: [w3149] -> w3087
                  tunnel: [w3148] -> w3086
                  tunnel: w3091 -> [w3148]
                  tunnel: w3090 -> [w3147]
                  tunnel: w3089 -> [w3146]
                  tunnel: w3088 -> [w3159]
                  tunnel: [w3159] -> w3083
                  tunnel: w3087 -> [w3158]
                  tunnel: [w3158] -> w3084
                  tunnel: w3086 -> [w3157]
                  tunnel: [w3157] -> w3085
                  tunnel: w3085 -> [w3162]
                  tunnel: w3084 -> [w3164]
                  tunnel: w3083 -> [w3163]
                  tunnel: [w3161] -> w3066
                  tunnel: [w3160] -> w3065
                  frame #0 {
                    n1606 = property on="R Step SP" class="DigNum (strict)"() -> ("Maximum"=w3123:dbl)  [unwired: 2 in, 2 out]
                    n1607 = property on="R Step SP" class="DigNum (strict)"() -> ("Minimum"=w3124:dbl)  [unwired: 2 in, 2 out]
                    n1608 = property on="R steps/rev" class="DigNum (strict)"() -> ("Value"=w3122:u32)  [unwired: 2 in, 2 out]
                    n1609 = property on="R offset deg" class="DigNum (strict)"() -> ("Value"=w3126:dbl)  [unwired: 2 in, 2 out]
                    n1610 = To Long Integer(number=w3123) -> (32bit integer=w3137:i32)
                    n1611 = To Long Integer(number=w3124) -> (32bit integer=w3138:i32)
                    n1612 = To Double Precision Float(number=w3122) -> (double precision float=w3136:dbl)
                    n1613 = call "mDrive Send Command.vi"("error in (no error)"=w3120, "Extra"="P", "Command"=T10."Print Parameter", "VISA resource name"=w3121) -> ("error out"=w3129:errorcluster, "read buffer"=w3140:string, "VISA resource name out"=w3130:refnum<visa-resource-name>)  [unwired: 3 in]
                    n1614 = Decimal String To Number(string=w3140, offset=0) -> (number=w3119:i32)  [unwired: 1 in, 1 out]
                    n1615 = property on="R Step PV" class="DigNum (strict)"("Val(Sgnl)"=w3119) -> ()  [unwired: 2 in, 2 out]
                    n1616 = In Range and Coerce(upper limit=w3137, x=w3119, lower limit=w3138) -> (In Range?=w3128:bool)  [unwired: 1 out]
                    n1617 = To Double Precision Float(number=w3119) -> (double precision float=w3133:dbl)
                    n1618 = property on="R in Range" class="Bool (strict)"("Val(Sgnl)"=w3128) -> ()  [unwired: 2 in, 2 out]
                    n1619 = Divide(x=w3133, y=w3136) -> (x/y=w3135:dbl)
                    n1620 = property on="R deg/rev" class="DigNum (strict)"() -> ("Value"=w3125:dbl)  [unwired: 2 in, 2 out]
                    n1621 = Multiply(x=w3135, y=w3125) -> (x*y=w3134:dbl)
                    n1622 = Add(x=w3134, y=w3126) -> (x+y=w3127:dbl)
                    n1623 = property on="R Position deg PV" class="DigNum (strict)"("Val(Sgnl)"=w3127) -> ()  [unwired: 2 in, 2 out]
                  }
                  frame #1 {
                    n1624 = call "mDrive Send Command.vi"("error in (no error)"=w3146, "Extra"="MV", "Command"=T10."Print Parameter", "VISA resource name"=w3147) -> ("error out"=w3149:errorcluster, "read buffer"=w3152:string, "VISA resource name out"=w3150:refnum<visa-resource-name>)  [unwired: 3 in]
                    n1625 = Decimal String To Number(string=w3152, offset=0 ("offset (0)")) -> (number=w3142:i32)  [unwired: 1 in, 1 out]
                    n1626 = Not Equal?(x=w3152, y="") -> (x != y?=w3145:bool)
                    n1627 = property on="R Ready" class="Bool (strict)"("Val(Sgnl)"=w3145) -> ()  [unwired: 2 in, 2 out]
                    n1628 = Number To Boolean Array(number=w3142) -> (Boolean array=w3144:bool[])
                    n1629 = Index Array(array=w3144, index=0) -> (element=w3141:bool)
                    n1630 = property on="R in Motion" class="Bool (strict)"("Val(Sgnl)"=w3141) -> ()  [unwired: 2 in, 2 out]
                  }
                  frame #2 {
                    n1631 = Wait (ms)(milliseconds to wait=u32 10) -> ()  [unwired: 1 out]
                  }
                  frame #3 {
                    n1632 = case shown="False" w3162 {
                      tunnel: w3163 -> [w3167 w3171]
                      tunnel: [w3168 w3171] -> w3161
                      tunnel: [w3169 w3170] -> w3160
                      tunnel: w3164 -> [w3166 w3170]
                      frame False {
                        n1633 = call "mDrive Send Command.vi"("error in (no error)"=w3166, "Command"=T10."Stop", "VISA resource name"=w3167) -> ("error out"=w3169:errorcluster, "VISA resource name out"=w3168:refnum<visa-resource-name>)  [unwired: 4 in, 1 out]
                      }
                      frame True {
                      }
                    }
                  }
                }
                n1634 = property on="Y in Motion" class="Bool (strict)"() -> ("Value"=w3074:bool)  [unwired: 2 in, 2 out]
                n1635 = property on="Z in Motion" class="Bool (strict)"() -> ("Value"=w3064:bool)  [unwired: 2 in, 2 out]
                n1636 = property on="X  in Motion" class="Bool (strict)"() -> ("Value"=w3073:bool)  [unwired: 2 in, 2 out]
                n1637 = property on="R in Motion" class="Bool (strict)"() -> ("Value"=w3063:bool)  [unwired: 2 in, 2 out]
                n1638 = Compound Arithmetic op=OR(w3073, w3074, w3064, w3063) -> (w3062:bool)
                n1639 = Not(x=w3062) -> (.not. x?=w3061:bool)
              }
            }
            frame #4 {
              n1640 = Wait (ms)(milliseconds to wait=u32 300) -> ()  [unwired: 1 out]
            }
            frame #5 {
              w3340 = TRUE ("R in Motion")
              n1641 = property on="X Position mm PV" class="DigNum (strict)"() -> ("Value"=w3369:dbl)  [unwired: 2 in, 2 out]
              n1642 = property on="X Position SP mm" class="DigNum (strict)"() -> ("Value"=w3368:dbl)  [unwired: 2 in, 2 out]
              n1643 = property on="Z Position mm PV" class="DigNum (strict)"() -> ("Value"=w3365:dbl)  [unwired: 2 in, 2 out]
              n1644 = property on="Z Position SP mm" class="DigNum (strict)"() -> ("Value"=w3358:dbl)  [unwired: 2 in, 2 out]
              n1645 = property on="Y Position mm PV" class="DigNum (strict)"() -> ("Value"=w3363:dbl)  [unwired: 2 in, 2 out]
              n1646 = property on="Y Position SP mm" class="DigNum (strict)"() -> ("Value"=w3362:dbl)  [unwired: 2 in, 2 out]
              n1647 = property on="R Position SP deg" class="DigNum (strict)"() -> ("Value"=w3360:dbl)  [unwired: 2 in, 2 out]
              n1648 = property on="R Position deg PV" class="DigNum (strict)"() -> ("Value"=w3359:dbl)  [unwired: 2 in, 2 out]
              n1649 = local write "STATUS"("LOOP HOMING" ("STATUS")) -> ()
              n1650 = Not Equal?(x=w3369, y=w3368) -> (x != y?=w3367:bool)
              n1651 = Not Equal?(x=w3365, y=w3358) -> (x != y?=w3366:bool)
              n1652 = Not Equal?(x=w3363, y=w3362) -> (x != y?=w3364:bool)
              n1653 = Not Equal?(x=w3360, y=w3359) -> (x != y?=w3361:bool)
              n1654 = case shown="True" w3367 {
                tunnel: w3357 -> [w3581 w3585]
                tunnel: w3355 -> [w3580 w3584]
                tunnel: [w3581 w3583] -> w3342
                tunnel: [w3580 w3582] -> w3343
                frame False {
                }
                frame True {
                  n1655 = flat-sequence {
                    tunnel: w3584 -> [w3600]
                    tunnel: w3585 -> [w3613]
                    tunnel: [w3613] -> w3599
                    tunnel: [w3600] -> w3598
                    tunnel: [w3602] -> w3597
                    tunnel: [w3616] -> w3596
                    tunnel: [w3615] -> w3595
                    tunnel: [w3614] -> w3594
                    tunnel: w3597 -> [w3614]
                    tunnel: w3598 -> [w3615]
                    tunnel: w3599 -> [w3616]
                    tunnel: [w3632] -> w3593
                    tunnel: [w3631] -> w3592
                    tunnel: w3596 -> [w3630]
                    tunnel: w3595 -> [w3629]
                    tunnel: w3594 -> [w3628]
                    tunnel: [w3628] -> w3591
                    tunnel: w3593 -> [w3639]
                    tunnel: [w3639] -> w3590
                    tunnel: w3592 -> [w3638]
                    tunnel: [w3638] -> w3589
                    tunnel: [w3636] -> w3588
                    tunnel: w3591 -> [w3636]
                    tunnel: [w3644] -> w3587
                    tunnel: [w3643] -> w3586
                    tunnel: w3590 -> [w3642]
                    tunnel: w3589 -> [w3641]
                    tunnel: w3588 -> [w3640]
                    tunnel: [w3648] -> w3582
                    tunnel: [w3649] -> w3583
                    tunnel: w3587 -> [w3649]
                    tunnel: w3586 -> [w3648]
                    frame #0 {
                      n1656 = property on="X steps/rev" class="DigNum (strict)"() -> ("Value"=w3612:u32)  [unwired: 2 in, 2 out]
                      n1657 = To Double Precision Float(number=w3612) -> (double precision float=w3607:dbl)
                      n1658 = property on="X offset mm" class="DigNum (strict)"() -> ("Value"=w3611:dbl)  [unwired: 2 in, 2 out]
                      n1659 = property on="X Position SP mm" class="DigNum (strict)"() -> ("Value"=w3610:dbl)  [unwired: 2 in, 2 out]
                      n1660 = Subtract(x=w3610, y=w3611) -> (x-y=w3604:dbl)
                      n1661 = property on="X mm/rev" class="DigNum (strict)"() -> ("Value"=w3601:dbl)  [unwired: 2 in, 2 out]
                      n1662 = Divide(x=w3604, y=w3601) -> (x/y=w3603:dbl)
                      n1663 = property on="X Step SP" class="DigNum (strict)"() -> ("Maximum"=w3609:dbl)  [unwired: 2 in, 2 out]
                      n1664 = property on="X Step SP" class="DigNum (strict)"() -> ("Minimum"=w3608:dbl)  [unwired: 2 in, 2 out]
                      n1665 = Multiply(x=w3603, y=w3607) -> (x*y=w3605:dbl)
                      n1666 = In Range and Coerce(upper limit=w3609, x=w3605, lower limit=w3608) -> (coerced(x)=w3606:dbl)  [unwired: 1 out]
                      n1667 = To Long Integer(number=w3606) -> (32bit integer=w3602:i32)
                      n1668 = property on="X Step SP" class="DigNum (strict)"("Val(Sgnl)"=w3602) -> ()  [unwired: 2 in, 2 out]
                    }
                    frame #1 {
                      n1669 = property on="X Step SP" class="DigNum (strict)"() -> ("Value"=w3625:i32)  [unwired: 2 in, 2 out]
                      n1670 = property on="X Step PV" class="DigNum (strict)"() -> ("Value"=w3624:i32)  [unwired: 2 in, 2 out]
                      n1671 = property on="X Backlash" class="DigNum (strict)"() -> ("Value"=w3617:i32)  [unwired: 2 in, 2 out]
                      n1672 = Subtract(x=w3625, y=w3624) -> (x-y=w3623:i32)
                      n1673 = Sign(1:w3617) -> (0:w3621:i32)
                      n1674 = Sign(1:w3623) -> (0:w3622:i32)
                      n1675 = Multiply(x=w3622, y=w3621) -> (x*y=w3620:i32)
                      n1676 = Equal?(x=w3620, y=1) -> (x = y?=w3618:bool)
                      n1677 = case shown="True" w3618 {
                        frame False {
                          n1678 = property on="X Backlash corr" class="Bool (strict)"("Val(Sgnl)"=FALSE ("Value (Signaling)")) -> ()  [unwired: 2 in, 2 out]
                        }
                        frame True {
                          n1679 = property on="X Backlash corr" class="Bool (strict)"("Val(Sgnl)"=TRUE ("Value (Signaling)")) -> ()  [unwired: 2 in, 2 out]
                        }
                      }
                    }
                    frame #2 {
                      # "Velocity Setting"
                      n1680 = property on="X Velocity SP step/sec" class="DigNum (strict)"() -> ("Value"=w3633:i32)  [unwired: 2 in, 2 out]
                      n1681 = Number To Decimal String(number=w3633) -> (decimal integer string=w3634:string)  [unwired: 1 in]
                      n1682 = call "mDrive Send Command.vi"("error in (no error)"=w3629, "Extra"=w3634, "Command"=T10."Max Velocity", "VISA resource name"=w3630) -> ("error out"=w3631:errorcluster, "VISA resource name out"=w3632:refnum<visa-resource-name>)  [unwired: 3 in, 1 out]
                    }
                    frame #3 {
                      n1683 = Wait (ms)(milliseconds to wait=u32 50) -> ()  [unwired: 1 out]
                    }
                    frame #4 {
                      # "Move to Abs Position"
                      n1684 = Number To Decimal String(number=w3640) -> (decimal integer string=w3646:string)  [unwired: 1 in]
                      n1685 = call "mDrive Send Command.vi"("error in (no error)"=w3641, "Extra"=w3646, "Command"=T10."Move to Absolute Position", "VISA resource name"=w3642) -> ("error out"=w3643:errorcluster, "VISA resource name out"=w3644:refnum<visa-resource-name>)  [unwired: 3 in, 1 out]
                    }
                    frame #5 {
                      n1686 = Wait (ms)(milliseconds to wait=u32 50) -> ()  [unwired: 1 out]
                    }
                  }
                }
              }
              n1687 = case shown="True" w3366 {
                tunnel: w3354 -> [w3510 w3515]
                tunnel: w3356 -> [w3511 w3514]
                tunnel: [w3511 w3513] -> w3344
                tunnel: [w3510 w3512] -> w3345
                frame False {
                }
                frame True {
                  n1688 = flat-sequence {
                    tunnel: [w3543] -> w3529
                    tunnel: [w3542] -> w3528
                    tunnel: [w3531] -> w3527
                    tunnel: w3515 -> [w3543]
                    tunnel: w3514 -> [w3542]
                    tunnel: [w3546] -> w3526
                    tunnel: [w3545] -> w3525
                    tunnel: [w3544] -> w3524
                    tunnel: w3527 -> [w3544]
                    tunnel: w3528 -> [w3545]
                    tunnel: w3529 -> [w3546]
                    tunnel: [w3562] -> w3523
                    tunnel: [w3561] -> w3522
                    tunnel: w3526 -> [w3560]
                    tunnel: w3525 -> [w3559]
                    tunnel: [w3558] -> w3521
                    tunnel: w3524 -> [w3558]
                    tunnel: w3523 -> [w3569]
                    tunnel: [w3569] -> w3520
                    tunnel: w3522 -> [w3568]
                    tunnel: [w3568] -> w3519
                    tunnel: w3521 -> [w3567]
                    tunnel: [w3567] -> w3518
                    tunnel: [w3574] -> w3517
                    tunnel: [w3573] -> w3516
                    tunnel: w3520 -> [w3572]
                    tunnel: w3519 -> [w3571]
                    tunnel: w3518 -> [w3570]
                    tunnel: [w3578] -> w3512
                    tunnel: [w3579] -> w3513
                    tunnel: w3517 -> [w3579]
                    tunnel: w3516 -> [w3578]
                    frame #0 {
                      n1689 = property on="Z steps/rev" class="DigNum (strict)"() -> ("Value"=w3530:u32)  [unwired: 2 in, 2 out]
                      n1690 = To Double Precision Float(number=w3530) -> (double precision float=w3536:dbl)
                      n1691 = property on="Z offset mm" class="DigNum (strict)"() -> ("Value"=w3538:dbl)  [unwired: 2 in, 2 out]
                      n1692 = property on="Z Position SP mm" class="DigNum (strict)"() -> ("Value"=w3537:dbl)  [unwired: 2 in, 2 out]
                      n1693 = Subtract(x=w3537, y=w3538) -> (x-y=w3533:dbl)
                      n1694 = property on="Z mm/rev" class="DigNum (strict)"() -> ("Value"=w3539:dbl)  [unwired: 2 in, 2 out]
                      n1695 = Divide(x=w3533, y=w3539) -> (x/y=w3532:dbl)
                      n1696 = property on="Z Step SP" class="DigNum (strict)"() -> ("Maximum"=w3541:dbl)  [unwired: 2 in, 2 out]
                      n1697 = property on="Z Step SP" class="DigNum (strict)"() -> ("Minimum"=w3540:dbl)  [unwired: 2 in, 2 out]
                      n1698 = Multiply(x=w3532, y=w3536) -> (x*y=w3534:dbl)
                      n1699 = In Range and Coerce(upper limit=w3541, x=w3534, lower limit=w3540) -> (coerced(x)=w3535:dbl)  [unwired: 1 out]
                      n1700 = To Long Integer(number=w3535) -> (32bit integer=w3531:i32)
                      n1701 = property on="Z Step SP" class="DigNum (strict)"("Val(Sgnl)"=w3531) -> ()  [unwired: 2 in, 2 out]
                    }
                    frame #1 {
                      n1702 = property on="Z Step SP" class="DigNum (strict)"() -> ("Value"=w3555:i32)  [unwired: 2 in, 2 out]
                      n1703 = property on="Z Backlash" class="DigNum (strict)"() -> ("Value"=w3547:i32)  [unwired: 2 in, 2 out]
                      n1704 = property on="Z Step PV" class="DigNum (strict)"() -> ("Value"=w3554:i32)  [unwired: 2 in, 2 out]
                      n1705 = Subtract(x=w3555, y=w3554) -> (x-y=w3553:i32)
                      n1706 = Sign(1:w3547) -> (0:w3551:i32)
                      n1707 = Sign(1:w3553) -> (0:w3552:i32)
                      n1708 = Multiply(x=w3552, y=w3551) -> (x*y=w3550:i32)
                      n1709 = Equal?(x=w3550, y=1) -> (x = y?=w3548:bool)
                      n1710 = case shown="False" w3548 {
                        frame False {
                          n1711 = property on="Z Backlash corr" class="Bool (strict)"("Val(Sgnl)"=FALSE ("Value (Signaling)")) -> ()  [unwired: 2 in, 2 out]
                        }
                        frame True {
                          n1712 = property on="Z Backlash corr" class="Bool (strict)"("Val(Sgnl)"=TRUE ("Value (Signaling)")) -> ()  [unwired: 2 in, 2 out]
                        }
                      }
                    }
                    frame #2 {
                      # "Velocity Setting"
                      n1713 = property on="Z Velocity SP step/sec" class="DigNum (strict)"() -> ("Value"=w3563:i32)  [unwired: 2 in, 2 out]
                      n1714 = Number To Decimal String(number=w3563) -> (decimal integer string=w3564:string)  [unwired: 1 in]
                      n1715 = call "mDrive Send Command.vi"("error in (no error)"=w3560, "Extra"=w3564, "Command"=T10."Max Velocity", "VISA resource name"=w3559) -> ("error out"=w3561:errorcluster, "VISA resource name out"=w3562:refnum<visa-resource-name>)  [unwired: 3 in, 1 out]
                    }
                    frame #3 {
                      n1716 = Wait (ms)(milliseconds to wait=u32 50) -> ()  [unwired: 1 out]
                    }
                    frame #4 {
                      # "Move to Abs Position"
                      n1717 = Number To Decimal String(number=w3570) -> (decimal integer string=w3576:string)  [unwired: 1 in]
                      n1718 = call "mDrive Send Command.vi"("error in (no error)"=w3571, "Extra"=w3576, "Command"=T10."Move to Absolute Position", "VISA resource name"=w3572) -> ("error out"=w3573:errorcluster, "VISA resource name out"=w3574:refnum<visa-resource-name>)  [unwired: 3 in, 1 out]
                    }
                    frame #5 {
                      n1719 = Wait (ms)(milliseconds to wait=u32 50) -> ()  [unwired: 1 out]
                    }
                  }
                }
              }
              n1720 = case shown="True" w3364 {
                tunnel: w3352 -> [w3440 w3445]
                tunnel: w3353 -> [w3441 w3444]
                tunnel: [w3441 w3443] -> w3346
                tunnel: [w3440 w3442] -> w3347
                frame False {
                }
                frame True {
                  n1721 = flat-sequence {
                    tunnel: [w3473] -> w3459
                    tunnel: [w3472] -> w3458
                    tunnel: [w3460] -> w3457
                    tunnel: w3444 -> [w3472]
                    tunnel: w3445 -> [w3473]
                    tunnel: [w3476] -> w3456
                    tunnel: [w3475] -> w3455
                    tunnel: [w3474] -> w3454
                    tunnel: w3457 -> [w3474]
                    tunnel: w3458 -> [w3475]
                    tunnel: w3459 -> [w3476]
                    tunnel: [w3492] -> w3453
                    tunnel: [w3491] -> w3452
                    tunnel: w3456 -> [w3490]
                    tunnel: w3455 -> [w3489]
                    tunnel: [w3488] -> w3451
                    tunnel: w3454 -> [w3488]
                    tunnel: w3453 -> [w3499]
                    tunnel: [w3499] -> w3450
                    tunnel: w3452 -> [w3498]
                    tunnel: [w3498] -> w3449
                    tunnel: [w3496] -> w3448
                    tunnel: w3451 -> [w3496]
                    tunnel: [w3504] -> w3447
                    tunnel: [w3503] -> w3446
                    tunnel: w3450 -> [w3502]
                    tunnel: w3449 -> [w3501]
                    tunnel: w3448 -> [w3500]
                    tunnel: [w3507] -> w3442
                    tunnel: [w3509] -> w3443
                    tunnel: w3447 -> [w3509]
                    tunnel: w3446 -> [w3507]
                    frame #0 {
                      n1722 = property on="Y steps/rev" class="DigNum (strict)"() -> ("Value"=w3469:u32)  [unwired: 2 in, 2 out]
                      n1723 = To Double Precision Float(number=w3469) -> (double precision float=w3465:dbl)
                      n1724 = property on="Y offset mm" class="DigNum (strict)"() -> ("Value"=w3467:dbl)  [unwired: 2 in, 2 out]
                      n1725 = property on="Y Position SP mm" class="DigNum (strict)"() -> ("Value"=w3466:dbl)  [unwired: 2 in, 2 out]
                      n1726 = Subtract(x=w3466, y=w3467) -> (x-y=w3462:dbl)
                      n1727 = property on="Y mm/rev" class="DigNum (strict)"() -> ("Value"=w3468:dbl)  [unwired: 2 in, 2 out]
                      n1728 = Divide(x=w3462, y=w3468) -> (x/y=w3461:dbl)
                      n1729 = property on="Y Step SP" class="DigNum (strict)"() -> ("Maximum"=w3470:dbl)  [unwired: 2 in, 2 out]
                      n1730 = property on="Y Step SP" class="DigNum (strict)"() -> ("Minimum"=w3471:dbl)  [unwired: 2 in, 2 out]
                      n1731 = Multiply(x=w3461, y=w3465) -> (x*y=w3463:dbl)
                      n1732 = In Range and Coerce(upper limit=w3470, x=w3463, lower limit=w3471) -> (coerced(x)=w3464:dbl)  [unwired: 1 out]
                      n1733 = To Long Integer(number=w3464) -> (32bit integer=w3460:i32)
                      n1734 = property on="Y Step SP" class="DigNum (strict)"("Val(Sgnl)"=w3460) -> ()  [unwired: 2 in, 2 out]
                    }
                    frame #1 {
                      n1735 = property on="Y Step SP" class="DigNum (strict)"() -> ("Value"=w3485:i32)  [unwired: 2 in, 2 out]
                      n1736 = property on="Y Backlash" class="DigNum (strict)"() -> ("Value"=w3477:i32)  [unwired: 2 in, 2 out]
                      n1737 = property on="Y Step PV" class="DigNum (strict)"() -> ("Value"=w3484:i32)  [unwired: 2 in, 2 out]
                      n1738 = Subtract(x=w3485, y=w3484) -> (x-y=w3483:i32)
                      n1739 = Sign(1:w3477) -> (0:w3481:i32)
                      n1740 = Sign(1:w3483) -> (0:w3482:i32)
                      n1741 = Multiply(x=w3482, y=w3481) -> (x*y=w3480:i32)
                      n1742 = Equal?(x=w3480, y=1) -> (x = y?=w3478:bool)
                      n1743 = case shown="True" w3478 {
                        frame False {
                          n1744 = property on="Y Backlash corr" class="Bool (strict)"("Val(Sgnl)"=FALSE ("Value (Signaling)")) -> ()  [unwired: 2 in, 2 out]
                        }
                        frame True {
                          n1745 = property on="Y Backlash corr" class="Bool (strict)"("Val(Sgnl)"=TRUE ("Value (Signaling)")) -> ()  [unwired: 2 in, 2 out]
                        }
                      }
                    }
                    frame #2 {
                      # "Velocity Setting"
                      n1746 = property on="Y Velocity SP step/sec" class="DigNum (strict)"() -> ("Value"=w3493:i32)  [unwired: 2 in, 2 out]
                      n1747 = Number To Decimal String(number=w3493) -> (decimal integer string=w3494:string)  [unwired: 1 in]
                      n1748 = call "mDrive Send Command.vi"("error in (no error)"=w3490, "Extra"=w3494, "Command"=T10."Max Velocity", "VISA resource name"=w3489) -> ("error out"=w3491:errorcluster, "VISA resource name out"=w3492:refnum<visa-resource-name>)  [unwired: 3 in, 1 out]
                    }
                    frame #3 {
                      n1749 = Wait (ms)(milliseconds to wait=u32 50) -> ()  [unwired: 1 out]
                    }
                    frame #4 {
                      # "Move to Abs Position"
                      n1750 = Number To Decimal String(number=w3500) -> (decimal integer string=w3506:string)  [unwired: 1 in]
                      n1751 = call "mDrive Send Command.vi"("error in (no error)"=w3501, "Extra"=w3506, "Command"=T10."Move to Absolute Position", "VISA resource name"=w3502) -> ("error out"=w3503:errorcluster, "VISA resource name out"=w3504:refnum<visa-resource-name>)  [unwired: 3 in, 1 out]
                    }
                    frame #5 {
                      n1752 = Wait (ms)(milliseconds to wait=u32 25) -> ()  [unwired: 1 out]
                    }
                  }
                }
              }
              n1753 = case shown="True" w3361 {
                tunnel: w3350 -> [w3370 w3375]
                tunnel: w3351 -> [w3371 w3374]
                tunnel: [w3371 w3373] -> w3349
                tunnel: [w3370 w3372] -> w3348
                frame False {
                }
                frame True {
                  n1754 = flat-sequence {
                    tunnel: w3374 -> [w3402]
                    tunnel: w3375 -> [w3403]
                    tunnel: [w3403] -> w3389
                    tunnel: [w3402] -> w3388
                    tunnel: [w3390] -> w3387
                    tunnel: [w3406] -> w3386
                    tunnel: [w3405] -> w3385
                    tunnel: [w3404] -> w3384
                    tunnel: w3387 -> [w3404]
                    tunnel: w3388 -> [w3405]
                    tunnel: w3389 -> [w3406]
                    tunnel: [w3422] -> w3383
                    tunnel: [w3421] -> w3382
                    tunnel: w3386 -> [w3420]
                    tunnel: w3385 -> [w3419]
                    tunnel: [w3418] -> w3381
                    tunnel: w3384 -> [w3418]
                    tunnel: w3383 -> [w3429]
                    tunnel: [w3429] -> w3380
                    tunnel: w3382 -> [w3428]
                    tunnel: [w3428] -> w3379
                    tunnel: w3381 -> [w3427]
                    tunnel: [w3427] -> w3378
                    tunnel: [w3434] -> w3377
                    tunnel: [w3433] -> w3376
                    tunnel: w3380 -> [w3432]
                    tunnel: w3379 -> [w3431]
                    tunnel: w3378 -> [w3430]
                    tunnel: [w3439] -> w3373
                    tunnel: w3377 -> [w3439]
                    tunnel: w3376 -> [w3438]
                    tunnel: [w3438] -> w3372
                    frame #0 {
                      n1755 = property on="R steps/rev" class="DigNum (strict)"() -> ("Value"=w3398:u32)  [unwired: 2 in, 2 out]
                      n1756 = To Double Precision Float(number=w3398) -> (double precision float=w3395:dbl)
                      n1757 = property on="R offset deg" class="DigNum (strict)"() -> ("Value"=w3399:dbl)  [unwired: 2 in, 2 out]
                      n1758 = property on="R Position SP deg" class="DigNum (strict)"() -> ("Value"=w3400:dbl)  [unwired: 2 in, 2 out]
                      n1759 = Subtract(x=w3400, y=w3399) -> (x-y=w3392:dbl)
                      n1760 = property on="R deg/rev" class="DigNum (strict)"() -> ("Value"=w3401:dbl)  [unwired: 2 in, 2 out]
                      n1761 = Divide(x=w3392, y=w3401) -> (x/y=w3391:dbl)
                      n1762 = property on="R Step SP" class="DigNum (strict)"() -> ("Maximum"=w3396:dbl)  [unwired: 2 in, 2 out]
                      n1763 = Multiply(x=w3391, y=w3395) -> (x*y=w3393:dbl)
                      n1764 = property on="R Step SP" class="DigNum (strict)"() -> ("Minimum"=w3397:dbl)  [unwired: 2 in, 2 out]
                      n1765 = In Range and Coerce(upper limit=w3396, x=w3393, lower limit=w3397) -> (coerced(x)=w3394:dbl)  [unwired: 1 out]
                      n1766 = To Long Integer(number=w3394) -> (32bit integer=w3390:i32)
                      n1767 = property on="R Step SP" class="DigNum (strict)"("Val(Sgnl)"=w3390) -> ()  [unwired: 2 in, 2 out]
                    }
                    frame #1 {
                      n1768 = property on="R Step SP" class="DigNum (strict)"() -> ("Value"=w3415:i32)  [unwired: 2 in, 2 out]
                      n1769 = property on="R Step PV" class="DigNum (strict)"() -> ("Value"=w3414:i32)  [unwired: 2 in, 2 out]
                      n1770 = property on="R Backlash" class="DigNum (strict)"() -> ("Value"=w3407:i32)  [unwired: 2 in, 2 out]
                      n1771 = Subtract(x=w3415, y=w3414) -> (x-y=w3413:i32)
                      n1772 = Sign(1:w3407) -> (0:w3411:i32)
                      n1773 = Sign(1:w3413) -> (0:w3412:i32)
                      n1774 = Multiply(x=w3412, y=w3411) -> (x*y=w3410:i32)
                      n1775 = Equal?(x=w3410, y=1) -> (x = y?=w3408:bool)
                      n1776 = case shown="True" w3408 {
                        frame False {
                          n1777 = property on="R Backlash corr" class="Bool (strict)"("Val(Sgnl)"=FALSE ("Value (Signaling)")) -> ()  [unwired: 2 in, 2 out]
                        }
                        frame True {
                          n1778 = property on="R Backlash corr" class="Bool (strict)"("Val(Sgnl)"=TRUE ("Value (Signaling)")) -> ()  [unwired: 2 in, 2 out]
                        }
                      }
                    }
                    frame #2 {
                      # "Velocity Setting"
                      n1779 = property on="R Velocity SP step/sec" class="DigNum (strict)"() -> ("Value"=w3423:i32)  [unwired: 2 in, 2 out]
                      n1780 = Number To Decimal String(number=w3423) -> (decimal integer string=w3424:string)  [unwired: 1 in]
                      n1781 = call "mDrive Send Command.vi"("error in (no error)"=w3420, "Extra"=w3424, "Command"=T10."Max Velocity", "VISA resource name"=w3419) -> ("error out"=w3421:errorcluster, "VISA resource name out"=w3422:refnum<visa-resource-name>)  [unwired: 3 in, 1 out]
                    }
                    frame #3 {
                      n1782 = Wait (ms)(milliseconds to wait=u32 50) -> ()  [unwired: 1 out]
                    }
                    frame #4 {
                      # "Move to Abs Position"
                      n1783 = Number To Decimal String(number=w3430) -> (decimal integer string=w3436:string)  [unwired: 1 in]
                      n1784 = call "mDrive Send Command.vi"("error in (no error)"=w3431, "Extra"=w3436, "Command"=T10."Move to Absolute Position", "VISA resource name"=w3432) -> ("error out"=w3433:errorcluster, "VISA resource name out"=w3434:refnum<visa-resource-name>)  [unwired: 3 in, 1 out]
                    }
                    frame #5 {
                      n1785 = Wait (ms)(milliseconds to wait=u32 25) -> ()  [unwired: 1 out]
                    }
                  }
                }
              }
              n1786 = property on="Y in Motion" class="Bool (strict)"("Value"=w3340) -> ()  [unwired: 2 in, 2 out]
              n1787 = property on="R in Motion" class="Bool (strict)"("Value"=w3340) -> ()  [unwired: 2 in, 2 out]
              n1788 = property on="X  in Motion" class="Bool (strict)"("Value"=w3340) -> ()  [unwired: 2 in, 2 out]
              n1789 = property on="Z in Motion" class="Bool (strict)"("Value"=w3340) -> ()  [unwired: 2 in, 2 out]
            }
            frame #6 {
              n1790 = while {
                tunnel: [w3687] -> w3663
                tunnel: [w3686] -> w3662
                tunnel: [w3685] -> w3665
                tunnel: [w3684] -> w3664
                tunnel: [w3683] -> w3661
                tunnel: [w3682] -> w3660
                tunnel: [w3681] -> w3659
                tunnel: [w3680] -> w3658
                tunnel: w3657 -> [w3669]
                tunnel: w3656 -> [w3668]
                tunnel: w3655 -> [w3671]
                tunnel: w3654 -> [w3670]
                tunnel: w3653 -> [w3676]
                tunnel: w3652 -> [w3675]
                tunnel: w3651 -> [w3674]
                tunnel: w3650 -> [w3673]
                stop <- w3672 stop-if-true
                n1791 = flat-sequence {
                  tunnel: [w4133] -> w3743
                  tunnel: [w4132] -> w3742
                  tunnel: [w4131] -> w3741
                  tunnel: w3669 -> [w4129]
                  tunnel: w3668 -> [w4128]
                  tunnel: [w4155] -> w3740
                  tunnel: [w4154] -> w3739
                  tunnel: [w4152] -> w3738
                  tunnel: [w4153] -> w3737
                  tunnel: w3743 -> [w4152]
                  tunnel: w3742 -> [w4151]
                  tunnel: w3741 -> [w4150]
                  tunnel: w3740 -> [w4169]
                  tunnel: [w4169] -> w3733
                  tunnel: w3739 -> [w4168]
                  tunnel: [w4168] -> w3734
                  tunnel: w3738 -> [w4167]
                  tunnel: [w4167] -> w3735
                  tunnel: w3737 -> [w4166]
                  tunnel: [w4166] -> w3736
                  tunnel: [w4173] -> w3732
                  tunnel: [w4174] -> w3731
                  tunnel: [w4170] -> w3730
                  tunnel: w3736 -> [w4170]
                  tunnel: w3735 -> [w4171]
                  tunnel: w3734 -> [w4175]
                  tunnel: w3733 -> [w4172]
                  tunnel: w3732 -> [w4185]
                  tunnel: w3731 -> [w4186]
                  tunnel: w3730 -> [w4188]
                  tunnel: [w4184] -> w3686
                  tunnel: [w4183] -> w3687
                  frame #0 {
                    n1792 = property on="Z Step SP" class="DigNum (strict)"() -> ("Maximum"=w4145:dbl)  [unwired: 2 in, 2 out]
                    n1793 = property on="Z Step SP" class="DigNum (strict)"() -> ("Minimum"=w4147:dbl)  [unwired: 2 in, 2 out]
                    n1794 = property on="Z steps/rev" class="DigNum (strict)"() -> ("Value"=w4142:u32)  [unwired: 2 in, 2 out]
                    n1795 = property on="Z offset mm" class="DigNum (strict)"() -> ("Value"=w4138:dbl)  [unwired: 2 in, 2 out]
                    n1796 = To Long Integer(number=w4145) -> (32bit integer=w4144:i32)
                    n1797 = To Long Integer(number=w4147) -> (32bit integer=w4146:i32)
                    n1798 = To Double Precision Float(number=w4142) -> (double precision float=w4143:dbl)
                    n1799 = call "mDrive Send Command.vi"("error in (no error)"=w4128, "Extra"="P", "Command"=T10."Print Parameter", "VISA resource name"=w4129) -> ("error out"=w4131:errorcluster, "read buffer"=w4149:string, "VISA resource name out"=w4132:refnum<visa-resource-name>)  [unwired: 3 in]
                    n1800 = Decimal String To Number(string=w4149, offset=0) -> (number=w4130:i32)  [unwired: 1 in, 1 out]
                    n1801 = property on="Z Step PV" class="DigNum (strict)"("Val(Sgnl)"=w4130) -> ()  [unwired: 2 in, 2 out]
                    n1802 = In Range and Coerce(upper limit=w4144, x=w4130, lower limit=w4146) -> (In Range?=w4133:bool)  [unwired: 1 out]
                    n1803 = To Double Precision Float(number=w4130) -> (double precision float=w4137:dbl)
                    n1804 = property on="Z in Range" class="Bool (strict)"("Val(Sgnl)"=w4133) -> ()  [unwired: 2 in, 2 out]
                    n1805 = Divide(x=w4137, y=w4143) -> (x/y=w4141:dbl)
                    n1806 = property on="Z mm/rev" class="DigNum (strict)"() -> ("Value"=w4140:dbl)  [unwired: 2 in, 2 out]
                    n1807 = Multiply(x=w4141, y=w4140) -> (x*y=w4139:dbl)
                    n1808 = Add(x=w4139, y=w4138) -> (x+y=w4136:dbl)
                    n1809 = property on="Z Position mm PV" class="DigNum (strict)"("Val(Sgnl)"=w4136) -> ()  [unwired: 2 in, 2 out]
                  }
                  frame #1 {
                    n1810 = call "mDrive Send Command.vi"("error in (no error)"=w4150, "Extra"="MV", "Command"=T10."Print Parameter", "VISA resource name"=w4151) -> ("error out"=w4154:errorcluster, "read buffer"=w4158:string, "VISA resource name out"=w4155:refnum<visa-resource-name>)  [unwired: 3 in]
                    n1811 = Decimal String To Number(string=w4158, offset=0 ("offset (0)")) -> (number=w4161:i32)  [unwired: 1 in, 1 out]
                    n1812 = Not Equal?(x=w4158, y="") -> (x != y?=w4156:bool)
                    n1813 = property on="Z Ready" class="Bool (strict)"("Val(Sgnl)"=w4156) -> ()  [unwired: 2 in, 2 out]
                    n1814 = Number To Boolean Array(number=w4161) -> (Boolean array=w4160:bool[])
                    n1815 = Index Array(array=w4160, index=0) -> (element=w4153:bool)
                    n1816 = property on="Z in Motion" class="Bool (strict)"("Val(Sgnl)"=w4153) -> ()  [unwired: 2 in, 2 out]
                  }
                  frame #2 {
                    n1817 = Wait (ms)(milliseconds to wait=u32 50) -> ()  [unwired: 1 out]
                  }
                  frame #3 {
                    n1818 = case shown="True" w4171 {
                      tunnel: w4172 -> [w4178 w4182]
                      tunnel: [w4179 w4182] -> w4173
                      tunnel: [w4180 w4181] -> w4174
                      tunnel: w4175 -> [w4177 w4181]
                      frame False {
                        n1819 = call "mDrive Send Command.vi"("error in (no error)"=w4177, "Command"=T10."Stop", "VISA resource name"=w4178) -> ("error out"=w4180:errorcluster, "VISA resource name out"=w4179:refnum<visa-resource-name>)  [unwired: 4 in, 1 out]
                      }
                      frame True {
                      }
                    }
                  }
                  frame #4 {
                    n1820 = property on="Z Backlash corr" class="Bool (strict)"() -> ("Value"=w4189:bool)  [unwired: 2 in, 2 out]
                    n1821 = Implies(1:w4188, 2:w4189) -> (0:w4187:bool)
                    n1822 = case shown="False" w4187 {
                      tunnel: w4186 -> [w4197 w4254]
                      tunnel: w4185 -> [w4196 w4255]
                      tunnel: [w4191 w4254] -> w4184
                      tunnel: [w4195 w4255] -> w4183
                      frame False {
                        # "Backlash"
                        n1823 = flat-sequence {
                          tunnel: [w4212] -> w4209
                          tunnel: [w4214] -> w4208
                          tunnel: [w4213] -> w4207
                          tunnel: w4197 -> [w4211]
                          tunnel: w4196 -> [w4210]
                          tunnel: w4209 -> [w4222]
                          tunnel: [w4222] -> w4206
                          tunnel: w4208 -> [w4221]
                          tunnel: w4207 -> [w4220]
                          tunnel: [w4219] -> w4205
                          tunnel: [w4218] -> w4204
                          tunnel: [w4217] -> w4194
                          tunnel: w4206 -> [w4236]
                          tunnel: w4205 -> [w4227]
                          tunnel: w4204 -> [w4235]
                          tunnel: [w4227] -> w4203
                          tunnel: [w4235] -> w4202
                          tunnel: [w4226] -> w4199
                          tunnel: [w4234] -> w4198
                          tunnel: w4194 -> [w4234]
                          tunnel: w4203 -> [w4239]
                          tunnel: w4202 -> [w4240]
                          tunnel: [w4238] -> w4201
                          tunnel: [w4246] -> w4200
                          tunnel: w4199 -> [w4246]
                          tunnel: w4198 -> [w4242]
                          tunnel: [w4241] -> w4192
                          tunnel: w4201 -> [w4249]
                          tunnel: w4200 -> [w4248]
                          tunnel: [w4250] -> w4193
                          tunnel: w4192 -> [w4250]
                          tunnel: [w4249] -> w4190
                          tunnel: [w4253] -> w4195
                          tunnel: w4193 -> [w4253]
                          tunnel: [w4251] -> w4191
                          tunnel: w4190 -> [w4251]
                          frame #0 {
                            n1824 = property on="Z Backlash steps/sec" class="DigNum (strict)"() -> ("Value"=w4212:i32)  [unwired: 2 in, 2 out]
                            n1825 = Number To Decimal String(number=w4212) -> (decimal integer string=w4215:string)  [unwired: 1 in]
                            n1826 = call "mDrive Send Command.vi"("error in (no error)"=w4211, "Extra"=w4215, "Command"=T10."Max Velocity", "VISA resource name"=w4210) -> ("error out"=w4213:errorcluster, "VISA resource name out"=w4214:refnum<visa-resource-name>)  [unwired: 3 in, 1 out]
                          }
                          frame #1 {
                            n1827 = property on="Z Backlash" class="DigNum (strict)"() -> ("Value"=w4217:i32)  [unwired: 2 in, 2 out]
                            n1828 = Number To Decimal String(number=w4217) -> (decimal integer string=w4223:string)  [unwired: 1 in]
                            n1829 = call "mDrive Send Command.vi"("error in (no error)"=w4220, "Extra"=w4223, "Command"=T10."Move to Relative Position", "VISA resource name"=w4221) -> ("error out"=w4219:errorcluster, "VISA resource name out"=w4218:refnum<visa-resource-name>)  [unwired: 3 in, 1 out]
                          }
                          frame #2 {
                            n1830 = To Double Precision Float(number=w4234) -> (double precision float=w4232:dbl)
                            n1831 = To Double Precision Float(number=w4236) -> (double precision float=w4237:dbl)
                            n1832 = Absolute Value(x=w4232) -> (abs(x)=w4233:dbl)
                            n1833 = Divide(x=w4233, y=w4237) -> (x/y=w4230:dbl)
                            n1834 = Multiply(x=1000.0, y=w4230) -> (x*y=w4228:dbl)
                            n1835 = Add(x=w4228, y=300.0) -> (x+y=w4226:dbl)
                            n1836 = To Unsigned Long Integer(number=w4226) -> (unsigned 32bit integer=w4225:u32)
                            n1837 = Wait (ms)(milliseconds to wait=w4225) -> ()  [unwired: 1 out]
                          }
                          frame #3 {
                            n1838 = Negate(x=w4242) -> (-x=w4243:i32)
                            n1839 = Number To Decimal String(number=w4243) -> (decimal integer string=w4244:string)  [unwired: 1 in]
                            n1840 = call "mDrive Send Command.vi"("error in (no error)"=w4239, "Extra"=w4244, "Command"=T10."Move to Relative Position", "VISA resource name"=w4240) -> ("error out"=w4238:errorcluster, "VISA resource name out"=w4241:refnum<visa-resource-name>)  [unwired: 3 in, 1 out]
                          }
                          frame #4 {
                            n1841 = To Unsigned Long Integer(number=w4248) -> (unsigned 32bit integer=w4247:u32)
                            n1842 = Wait (ms)(milliseconds to wait=w4247) -> ()  [unwired: 1 out]
                          }
                          frame #5 {
                            n1843 = property on="Z Backlash corr" class="Bool (strict)"("Val(Sgnl)"=FALSE ("Value (Signaling)")) -> ()  [unwired: 2 in, 2 out]
                          }
                        }
                      }
                      frame True {
                      }
                    }
                  }
                }
                n1844 = flat-sequence {
                  tunnel: [w4011] -> w3729
                  tunnel: [w4004] -> w3728
                  tunnel: [w4003] -> w3727
                  tunnel: w3671 -> [w4001]
                  tunnel: w3670 -> [w4000]
                  tunnel: [w4031] -> w3726
                  tunnel: [w4030] -> w3725
                  tunnel: [w4029] -> w3724
                  tunnel: [w4022] -> w3723
                  tunnel: w3729 -> [w4029]
                  tunnel: w3728 -> [w4028]
                  tunnel: w3727 -> [w4027]
                  tunnel: w3726 -> [w4041]
                  tunnel: [w4041] -> w3719
                  tunnel: w3725 -> [w4040]
                  tunnel: [w4040] -> w3720
                  tunnel: w3724 -> [w4039]
                  tunnel: [w4039] -> w3721
                  tunnel: w3723 -> [w4038]
                  tunnel: [w4038] -> w3722
                  tunnel: [w4045] -> w3718
                  tunnel: [w4046] -> w3717
                  tunnel: [w4042] -> w3716
                  tunnel: w3722 -> [w4042]
                  tunnel: w3721 -> [w4043]
                  tunnel: w3720 -> [w4047]
                  tunnel: w3719 -> [w4044]
                  tunnel: w3718 -> [w4058]
                  tunnel: w3717 -> [w4059]
                  tunnel: w3716 -> [w4061]
                  tunnel: [w4057] -> w3684
                  tunnel: [w4056] -> w3685
                  frame #0 {
                    n1845 = property on="X Step SP" class="DigNum (strict)"() -> ("Maximum"=w4012:dbl)  [unwired: 2 in, 2 out]
                    n1846 = property on="X Step SP" class="DigNum (strict)"() -> ("Minimum"=w4006:dbl)  [unwired: 2 in, 2 out]
                    n1847 = property on="X steps/rev" class="DigNum (strict)"() -> ("Value"=w4010:u32)  [unwired: 2 in, 2 out]
                    n1848 = property on="X offset mm" class="DigNum (strict)"() -> ("Value"=w4008:dbl)  [unwired: 2 in, 2 out]
                    n1849 = To Long Integer(number=w4012) -> (32bit integer=w4018:i32)
                    n1850 = To Long Integer(number=w4006) -> (32bit integer=w4019:i32)
                    n1851 = To Double Precision Float(number=w4010) -> (double precision float=w4017:dbl)
                    n1852 = call "mDrive Send Command.vi"("error in (no error)"=w4000, "Extra"="P", "Command"=T10."Print Parameter", "VISA resource name"=w4001) -> ("error out"=w4003:errorcluster, "read buffer"=w4021:string, "VISA resource name out"=w4004:refnum<visa-resource-name>)  [unwired: 3 in]
                    n1853 = Decimal String To Number(string=w4021, offset=0) -> (number=w4002:i32)  [unwired: 1 in, 1 out]
                    n1854 = property on="X Step PV" class="DigNum (strict)"("Val(Sgnl)"=w4002) -> ()  [unwired: 2 in, 2 out]
                    n1855 = In Range and Coerce(upper limit=w4018, x=w4002, lower limit=w4019) -> (In Range?=w4011:bool)  [unwired: 1 out]
                    n1856 = To Double Precision Float(number=w4002) -> (double precision float=w4015:dbl)
                    n1857 = property on="X  in Range" class="Bool (strict)"("Val(Sgnl)"=w4011) -> ()  [unwired: 2 in, 2 out]
                    n1858 = Divide(x=w4015, y=w4017) -> (x/y=w4016:dbl)
                    n1859 = property on="X mm/rev" class="DigNum (strict)"() -> ("Value"=w4009:dbl)  [unwired: 2 in, 2 out]
                    n1860 = Multiply(x=w4016, y=w4009) -> (x*y=w4005:dbl)
                    n1861 = Add(x=w4005, y=w4008) -> (x+y=w4007:dbl)
                    n1862 = property on="X Position mm PV" class="DigNum (strict)"("Val(Sgnl)"=w4007) -> ()  [unwired: 2 in, 2 out]
                  }
                  frame #1 {
                    n1863 = call "mDrive Send Command.vi"("error in (no error)"=w4027, "Extra"="MV", "Command"=T10."Print Parameter", "VISA resource name"=w4028) -> ("error out"=w4030:errorcluster, "read buffer"=w4033:string, "VISA resource name out"=w4031:refnum<visa-resource-name>)  [unwired: 3 in]
                    n1864 = Decimal String To Number(string=w4033, offset=0 ("offset (0)")) -> (number=w4023:i32)  [unwired: 1 in, 1 out]
                    n1865 = Not Equal?(x=w4033, y="") -> (x != y?=w4026:bool)
                    n1866 = property on="X Ready" class="Bool (strict)"("Val(Sgnl)"=w4026) -> ()  [unwired: 2 in, 2 out]
                    n1867 = Number To Boolean Array(number=w4023) -> (Boolean array=w4025:bool[])
                    n1868 = Index Array(array=w4025, index=0) -> (element=w4022:bool)
                    n1869 = property on="X  in Motion" class="Bool (strict)"("Val(Sgnl)"=w4022) -> ()  [unwired: 2 in, 2 out]
                  }
                  frame #2 {
                    n1870 = Wait (ms)(milliseconds to wait=u32 50) -> ()  [unwired: 1 out]
                  }
                  frame #3 {
                    n1871 = case shown="False" w4043 {
                      tunnel: w4044 -> [w4050 w4054]
                      tunnel: [w4051 w4054] -> w4045
                      tunnel: [w4052 w4053] -> w4046
                      tunnel: w4047 -> [w4049 w4053]
                      frame False {
                        n1872 = call "mDrive Send Command.vi"("error in (no error)"=w4049, "Command"=T10."Stop", "VISA resource name"=w4050) -> ("error out"=w4052:errorcluster, "VISA resource name out"=w4051:refnum<visa-resource-name>)  [unwired: 4 in, 1 out]
                      }
                      frame True {
                      }
                    }
                  }
                  frame #4 {
                    n1873 = property on="X Backlash corr" class="Bool (strict)"() -> ("Value"=w4055:bool)  [unwired: 2 in, 2 out]
                    n1874 = Implies(1:w4061, 2:w4055) -> (0:w4060:bool)
                    n1875 = case shown="False" w4060 {
                      tunnel: w4059 -> [w4069 w4126]
                      tunnel: w4058 -> [w4068 w4127]
                      tunnel: [w4063 w4126] -> w4057
                      tunnel: [w4067 w4127] -> w4056
                      frame False {
                        # "Backlash"
                        n1876 = flat-sequence {
                          tunnel: [w4082] -> w4081
                          tunnel: [w4086] -> w4080
                          tunnel: [w4085] -> w4079
                          tunnel: w4069 -> [w4084]
                          tunnel: w4068 -> [w4083]
                          tunnel: w4081 -> [w4094]
                          tunnel: [w4094] -> w4078
                          tunnel: w4080 -> [w4093]
                          tunnel: w4079 -> [w4092]
                          tunnel: [w4091] -> w4077
                          tunnel: [w4090] -> w4076
                          tunnel: [w4089] -> w4066
                          tunnel: w4078 -> [w4108]
                          tunnel: w4077 -> [w4099]
                          tunnel: w4076 -> [w4107]
                          tunnel: [w4099] -> w4075
                          tunnel: [w4107] -> w4074
                          tunnel: [w4098] -> w4071
                          tunnel: [w4106] -> w4070
                          tunnel: w4066 -> [w4106]
                          tunnel: w4075 -> [w4111]
                          tunnel: w4074 -> [w4112]
                          tunnel: [w4110] -> w4073
                          tunnel: [w4118] -> w4072
                          tunnel: w4071 -> [w4118]
                          tunnel: w4070 -> [w4114]
                          tunnel: [w4113] -> w4064
                          tunnel: w4073 -> [w4121]
                          tunnel: w4072 -> [w4120]
                          tunnel: [w4122] -> w4065
                          tunnel: w4064 -> [w4122]
                          tunnel: [w4121] -> w4062
                          tunnel: [w4125] -> w4067
                          tunnel: w4065 -> [w4125]
                          tunnel: [w4124] -> w4063
                          tunnel: w4062 -> [w4124]
                          frame #0 {
                            n1877 = property on="X Backlash steps/sec" class="DigNum (strict)"() -> ("Value"=w4082:i32)  [unwired: 2 in, 2 out]
                            n1878 = Number To Decimal String(number=w4082) -> (decimal integer string=w4087:string)  [unwired: 1 in]
                            n1879 = call "mDrive Send Command.vi"("error in (no error)"=w4084, "Extra"=w4087, "Command"=T10."Max Velocity", "VISA resource name"=w4083) -> ("error out"=w4085:errorcluster, "VISA resource name out"=w4086:refnum<visa-resource-name>)  [unwired: 3 in, 1 out]
                          }
                          frame #1 {
                            n1880 = property on="X Backlash" class="DigNum (strict)"() -> ("Value"=w4089:i32)  [unwired: 2 in, 2 out]
                            n1881 = Number To Decimal String(number=w4089) -> (decimal integer string=w4095:string)  [unwired: 1 in]
                            n1882 = call "mDrive Send Command.vi"("error in (no error)"=w4092, "Extra"=w4095, "Command"=T10."Move to Relative Position", "VISA resource name"=w4093) -> ("error out"=w4091:errorcluster, "VISA resource name out"=w4090:refnum<visa-resource-name>)  [unwired: 3 in, 1 out]
                          }
                          frame #2 {
                            n1883 = To Double Precision Float(number=w4106) -> (double precision float=w4104:dbl)
                            n1884 = To Double Precision Float(number=w4108) -> (double precision float=w4109:dbl)
                            n1885 = Absolute Value(x=w4104) -> (abs(x)=w4105:dbl)
                            n1886 = Divide(x=w4105, y=w4109) -> (x/y=w4102:dbl)
                            n1887 = Multiply(x=1000.0, y=w4102) -> (x*y=w4100:dbl)
                            n1888 = Add(x=w4100, y=300.0) -> (x+y=w4098:dbl)
                            n1889 = To Unsigned Long Integer(number=w4098) -> (unsigned 32bit integer=w4097:u32)
                            n1890 = Wait (ms)(milliseconds to wait=w4097) -> ()  [unwired: 1 out]
                          }
                          frame #3 {
                            n1891 = Negate(x=w4114) -> (-x=w4115:i32)
                            n1892 = Number To Decimal String(number=w4115) -> (decimal integer string=w4116:string)  [unwired: 1 in]
                            n1893 = call "mDrive Send Command.vi"("error in (no error)"=w4111, "Extra"=w4116, "Command"=T10."Move to Relative Position", "VISA resource name"=w4112) -> ("error out"=w4110:errorcluster, "VISA resource name out"=w4113:refnum<visa-resource-name>)  [unwired: 3 in, 1 out]
                          }
                          frame #4 {
                            n1894 = To Unsigned Long Integer(number=w4120) -> (unsigned 32bit integer=w4119:u32)
                            n1895 = Wait (ms)(milliseconds to wait=w4119) -> ()  [unwired: 1 out]
                          }
                          frame #5 {
                            n1896 = property on="X Backlash corr" class="Bool (strict)"("Val(Sgnl)"=FALSE ("Value (Signaling)")) -> ()  [unwired: 2 in, 2 out]
                          }
                        }
                      }
                      frame True {
                      }
                    }
                  }
                }
                n1897 = flat-sequence {
                  tunnel: [w3881] -> w3715
                  tunnel: [w3883] -> w3714
                  tunnel: [w3882] -> w3713
                  tunnel: w3676 -> [w3873]
                  tunnel: w3675 -> [w3872]
                  tunnel: [w3903] -> w3712
                  tunnel: [w3902] -> w3711
                  tunnel: [w3901] -> w3710
                  tunnel: [w3894] -> w3709
                  tunnel: w3715 -> [w3901]
                  tunnel: w3714 -> [w3900]
                  tunnel: w3713 -> [w3899]
                  tunnel: w3712 -> [w3913]
                  tunnel: [w3913] -> w3705
                  tunnel: w3711 -> [w3912]
                  tunnel: [w3912] -> w3706
                  tunnel: w3710 -> [w3911]
                  tunnel: [w3911] -> w3707
                  tunnel: w3709 -> [w3910]
                  tunnel: [w3910] -> w3708
                  tunnel: [w3917] -> w3704
                  tunnel: [w3918] -> w3703
                  tunnel: [w3914] -> w3702
                  tunnel: w3708 -> [w3914]
                  tunnel: w3707 -> [w3915]
                  tunnel: w3706 -> [w3919]
                  tunnel: w3705 -> [w3916]
                  tunnel: w3704 -> [w3930]
                  tunnel: w3703 -> [w3931]
                  tunnel: w3702 -> [w3933]
                  tunnel: [w3929] -> w3682
                  tunnel: [w3928] -> w3683
                  frame #0 {
                    n1898 = property on="Y Step SP" class="DigNum (strict)"() -> ("Maximum"=w3876:dbl)  [unwired: 2 in, 2 out]
                    n1899 = property on="Y Step SP" class="DigNum (strict)"() -> ("Minimum"=w3875:dbl)  [unwired: 2 in, 2 out]
                    n1900 = property on="Y steps/rev" class="DigNum (strict)"() -> ("Value"=w3877:u32)  [unwired: 2 in, 2 out]
                    n1901 = property on="Y offset mm" class="DigNum (strict)"() -> ("Value"=w3879:dbl)  [unwired: 2 in, 2 out]
                    n1902 = To Long Integer(number=w3876) -> (32bit integer=w3890:i32)
                    n1903 = To Long Integer(number=w3875) -> (32bit integer=w3891:i32)
                    n1904 = To Double Precision Float(number=w3877) -> (double precision float=w3889:dbl)
                    n1905 = call "mDrive Send Command.vi"("error in (no error)"=w3873, "Extra"="P", "Command"=T10."Print Parameter", "VISA resource name"=w3872) -> ("error out"=w3882:errorcluster, "read buffer"=w3893:string, "VISA resource name out"=w3883:refnum<visa-resource-name>)  [unwired: 3 in]
                    n1906 = Decimal String To Number(string=w3893, offset=0) -> (number=w3874:i32)  [unwired: 1 in, 1 out]
                    n1907 = property on="Y Step PV" class="DigNum (strict)"("Val(Sgnl)"=w3874) -> ()  [unwired: 2 in, 2 out]
                    n1908 = In Range and Coerce(upper limit=w3890, x=w3874, lower limit=w3891) -> (In Range?=w3881:bool)  [unwired: 1 out]
                    n1909 = To Double Precision Float(number=w3874) -> (double precision float=w3886:dbl)
                    n1910 = property on="Y in Range" class="Bool (strict)"("Val(Sgnl)"=w3881) -> ()  [unwired: 2 in, 2 out]
                    n1911 = Divide(x=w3886, y=w3889) -> (x/y=w3888:dbl)
                    n1912 = property on="Y mm/rev" class="DigNum (strict)"() -> ("Value"=w3878:dbl)  [unwired: 2 in, 2 out]
                    n1913 = Multiply(x=w3888, y=w3878) -> (x*y=w3887:dbl)
                    n1914 = Add(x=w3887, y=w3879) -> (x+y=w3880:dbl)
                    n1915 = property on="Y Position mm PV" class="DigNum (strict)"("Val(Sgnl)"=w3880) -> ()  [unwired: 2 in, 2 out]
                  }
                  frame #1 {
                    n1916 = call "mDrive Send Command.vi"("error in (no error)"=w3899, "Extra"="MV", "Command"=T10."Print Parameter", "VISA resource name"=w3900) -> ("error out"=w3902:errorcluster, "read buffer"=w3905:string, "VISA resource name out"=w3903:refnum<visa-resource-name>)  [unwired: 3 in]
                    n1917 = Decimal String To Number(string=w3905, offset=0 ("offset (0)")) -> (number=w3895:i32)  [unwired: 1 in, 1 out]
                    n1918 = Not Equal?(x=w3905, y="") -> (x != y?=w3898:bool)
                    n1919 = property on="Y Ready" class="Bool (strict)"("Val(Sgnl)"=w3898) -> ()  [unwired: 2 in, 2 out]
                    n1920 = Number To Boolean Array(number=w3895) -> (Boolean array=w3897:bool[])
                    n1921 = Index Array(array=w3897, index=0) -> (element=w3894:bool)
                    n1922 = property on="Y in Motion" class="Bool (strict)"("Val(Sgnl)"=w3894) -> ()  [unwired: 2 in, 2 out]
                  }
                  frame #2 {
                    n1923 = Wait (ms)(milliseconds to wait=u32 50) -> ()  [unwired: 1 out]
                  }
                  frame #3 {
                    n1924 = case shown="False" w3915 {
                      tunnel: w3916 -> [w3922 w3925]
                      tunnel: [w3923 w3925] -> w3917
                      tunnel: [w3924 w3926] -> w3918
                      tunnel: w3919 -> [w3921 w3926]
                      frame False {
                        n1925 = call "mDrive Send Command.vi"("error in (no error)"=w3921, "Command"=T10."Stop", "VISA resource name"=w3922) -> ("error out"=w3924:errorcluster, "VISA resource name out"=w3923:refnum<visa-resource-name>)  [unwired: 4 in, 1 out]
                      }
                      frame True {
                      }
                    }
                  }
                  frame #4 {
                    n1926 = property on="Y Backlash corr" class="Bool (strict)"() -> ("Value"=w3927:bool)  [unwired: 2 in, 2 out]
                    n1927 = Implies(1:w3933, 2:w3927) -> (0:w3932:bool)
                    n1928 = case shown="False" w3932 {
                      tunnel: w3931 -> [w3941 w3998]
                      tunnel: w3930 -> [w3940 w3999]
                      tunnel: [w3935 w3998] -> w3929
                      tunnel: [w3939 w3999] -> w3928
                      frame False {
                        # "Backlash"
                        n1929 = flat-sequence {
                          tunnel: [w3954] -> w3953
                          tunnel: [w3958] -> w3952
                          tunnel: [w3957] -> w3951
                          tunnel: w3941 -> [w3956]
                          tunnel: w3940 -> [w3955]
                          tunnel: w3953 -> [w3966]
                          tunnel: [w3966] -> w3950
                          tunnel: w3952 -> [w3965]
                          tunnel: w3951 -> [w3964]
                          tunnel: [w3963] -> w3949
                          tunnel: [w3962] -> w3948
                          tunnel: [w3961] -> w3938
                          tunnel: w3950 -> [w3980]
                          tunnel: w3949 -> [w3971]
                          tunnel: w3948 -> [w3979]
                          tunnel: [w3971] -> w3947
                          tunnel: [w3979] -> w3946
                          tunnel: [w3970] -> w3943
                          tunnel: [w3978] -> w3942
                          tunnel: w3938 -> [w3978]
                          tunnel: w3947 -> [w3983]
                          tunnel: w3946 -> [w3984]
                          tunnel: [w3982] -> w3945
                          tunnel: [w3990] -> w3944
                          tunnel: w3943 -> [w3990]
                          tunnel: w3942 -> [w3986]
                          tunnel: [w3985] -> w3936
                          tunnel: w3945 -> [w3993]
                          tunnel: w3944 -> [w3992]
                          tunnel: [w3994] -> w3937
                          tunnel: w3936 -> [w3994]
                          tunnel: [w3993] -> w3934
                          tunnel: [w3997] -> w3939
                          tunnel: w3937 -> [w3997]
                          tunnel: [w3996] -> w3935
                          tunnel: w3934 -> [w3996]
                          frame #0 {
                            n1930 = property on="Y Backlash steps/sec" class="DigNum (strict)"() -> ("Value"=w3954:i32)  [unwired: 2 in, 2 out]
                            n1931 = Number To Decimal String(number=w3954) -> (decimal integer string=w3959:string)  [unwired: 1 in]
                            n1932 = call "mDrive Send Command.vi"("error in (no error)"=w3956, "Extra"=w3959, "Command"=T10."Max Velocity", "VISA resource name"=w3955) -> ("error out"=w3957:errorcluster, "VISA resource name out"=w3958:refnum<visa-resource-name>)  [unwired: 3 in, 1 out]
                          }
                          frame #1 {
                            n1933 = property on="Y Backlash" class="DigNum (strict)"() -> ("Value"=w3961:i32)  [unwired: 2 in, 2 out]
                            n1934 = Number To Decimal String(number=w3961) -> (decimal integer string=w3967:string)  [unwired: 1 in]
                            n1935 = call "mDrive Send Command.vi"("error in (no error)"=w3964, "Extra"=w3967, "Command"=T10."Move to Relative Position", "VISA resource name"=w3965) -> ("error out"=w3963:errorcluster, "VISA resource name out"=w3962:refnum<visa-resource-name>)  [unwired: 3 in, 1 out]
                          }
                          frame #2 {
                            n1936 = To Double Precision Float(number=w3978) -> (double precision float=w3976:dbl)
                            n1937 = To Double Precision Float(number=w3980) -> (double precision float=w3981:dbl)
                            n1938 = Absolute Value(x=w3976) -> (abs(x)=w3977:dbl)
                            n1939 = Divide(x=w3977, y=w3981) -> (x/y=w3974:dbl)
                            n1940 = Multiply(x=1000.0, y=w3974) -> (x*y=w3972:dbl)
                            n1941 = Add(x=w3972, y=300.0) -> (x+y=w3970:dbl)
                            n1942 = To Unsigned Long Integer(number=w3970) -> (unsigned 32bit integer=w3969:u32)
                            n1943 = Wait (ms)(milliseconds to wait=w3969) -> ()  [unwired: 1 out]
                          }
                          frame #3 {
                            n1944 = Negate(x=w3986) -> (-x=w3987:i32)
                            n1945 = Number To Decimal String(number=w3987) -> (decimal integer string=w3988:string)  [unwired: 1 in]
                            n1946 = call "mDrive Send Command.vi"("error in (no error)"=w3983, "Extra"=w3988, "Command"=T10."Move to Relative Position", "VISA resource name"=w3984) -> ("error out"=w3982:errorcluster, "VISA resource name out"=w3985:refnum<visa-resource-name>)  [unwired: 3 in, 1 out]
                          }
                          frame #4 {
                            n1947 = To Unsigned Long Integer(number=w3992) -> (unsigned 32bit integer=w3991:u32)
                            n1948 = Wait (ms)(milliseconds to wait=w3991) -> ()  [unwired: 1 out]
                          }
                          frame #5 {
                            n1949 = property on="Y Backlash corr" class="Bool (strict)"("Val(Sgnl)"=FALSE ("Value (Signaling)")) -> ()  [unwired: 2 in, 2 out]
                          }
                        }
                      }
                      frame True {
                      }
                    }
                  }
                }
                n1950 = flat-sequence {
                  tunnel: [w3753] -> w3701
                  tunnel: [w3755] -> w3700
                  tunnel: [w3754] -> w3699
                  tunnel: w3674 -> [w3745]
                  tunnel: w3673 -> [w3744]
                  tunnel: [w3775] -> w3698
                  tunnel: [w3774] -> w3697
                  tunnel: [w3773] -> w3696
                  tunnel: [w3766] -> w3695
                  tunnel: w3701 -> [w3773]
                  tunnel: w3700 -> [w3772]
                  tunnel: w3699 -> [w3771]
                  tunnel: w3698 -> [w3785]
                  tunnel: [w3785] -> w3691
                  tunnel: w3697 -> [w3784]
                  tunnel: [w3784] -> w3692
                  tunnel: w3696 -> [w3783]
                  tunnel: [w3783] -> w3693
                  tunnel: w3695 -> [w3782]
                  tunnel: [w3782] -> w3694
                  tunnel: [w3789] -> w3690
                  tunnel: [w3790] -> w3689
                  tunnel: [w3786] -> w3688
                  tunnel: w3694 -> [w3786]
                  tunnel: w3693 -> [w3787]
                  tunnel: w3692 -> [w3791]
                  tunnel: w3691 -> [w3788]
                  tunnel: w3690 -> [w3802]
                  tunnel: w3689 -> [w3803]
                  tunnel: w3688 -> [w3805]
                  tunnel: [w3801] -> w3680
                  tunnel: [w3800] -> w3681
                  frame #0 {
                    n1951 = property on="R Step SP" class="DigNum (strict)"() -> ("Maximum"=w3748:dbl)  [unwired: 2 in, 2 out]
                    n1952 = property on="R Step SP" class="DigNum (strict)"() -> ("Minimum"=w3749:dbl)  [unwired: 2 in, 2 out]
                    n1953 = property on="R steps/rev" class="DigNum (strict)"() -> ("Value"=w3747:u32)  [unwired: 2 in, 2 out]
                    n1954 = property on="R offset deg" class="DigNum (strict)"() -> ("Value"=w3751:dbl)  [unwired: 2 in, 2 out]
                    n1955 = To Long Integer(number=w3748) -> (32bit integer=w3762:i32)
                    n1956 = To Long Integer(number=w3749) -> (32bit integer=w3763:i32)
                    n1957 = To Double Precision Float(number=w3747) -> (double precision float=w3761:dbl)
                    n1958 = call "mDrive Send Command.vi"("error in (no error)"=w3745, "Extra"="P", "Command"=T10."Print Parameter", "VISA resource name"=w3744) -> ("error out"=w3754:errorcluster, "read buffer"=w3765:string, "VISA resource name out"=w3755:refnum<visa-resource-name>)  [unwired: 3 in]
                    n1959 = Decimal String To Number(string=w3765, offset=0) -> (number=w3746:i32)  [unwired: 1 in, 1 out]
                    n1960 = property on="R Step PV" class="DigNum (strict)"("Val(Sgnl)"=w3746) -> ()  [unwired: 2 in, 2 out]
                    n1961 = In Range and Coerce(upper limit=w3762, x=w3746, lower limit=w3763) -> (In Range?=w3753:bool)  [unwired: 1 out]
                    n1962 = To Double Precision Float(number=w3746) -> (double precision float=w3758:dbl)
                    n1963 = property on="R in Range" class="Bool (strict)"("Val(Sgnl)"=w3753) -> ()  [unwired: 2 in, 2 out]
                    n1964 = Divide(x=w3758, y=w3761) -> (x/y=w3760:dbl)
                    n1965 = property on="R deg/rev" class="DigNum (strict)"() -> ("Value"=w3750:dbl)  [unwired: 2 in, 2 out]
                    n1966 = Multiply(x=w3760, y=w3750) -> (x*y=w3759:dbl)
                    n1967 = Add(x=w3759, y=w3751) -> (x+y=w3752:dbl)
                    n1968 = property on="R Position deg PV" class="DigNum (strict)"("Val(Sgnl)"=w3752) -> ()  [unwired: 2 in, 2 out]
                  }
                  frame #1 {
                    n1969 = call "mDrive Send Command.vi"("error in (no error)"=w3771, "Extra"="MV", "Command"=T10."Print Parameter", "VISA resource name"=w3772) -> ("error out"=w3774:errorcluster, "read buffer"=w3777:string, "VISA resource name out"=w3775:refnum<visa-resource-name>)  [unwired: 3 in]
                    n1970 = Decimal String To Number(string=w3777, offset=0 ("offset (0)")) -> (number=w3767:i32)  [unwired: 1 in, 1 out]
                    n1971 = Not Equal?(x=w3777, y="") -> (x != y?=w3770:bool)
                    n1972 = property on="R Ready" class="Bool (strict)"("Val(Sgnl)"=w3770) -> ()  [unwired: 2 in, 2 out]
                    n1973 = Number To Boolean Array(number=w3767) -> (Boolean array=w3769:bool[])
                    n1974 = Index Array(array=w3769, index=0) -> (element=w3766:bool)
                    n1975 = property on="R in Motion" class="Bool (strict)"("Val(Sgnl)"=w3766) -> ()  [unwired: 2 in, 2 out]
                  }
                  frame #2 {
                    n1976 = Wait (ms)(milliseconds to wait=u32 50) -> ()  [unwired: 1 out]
                  }
                  frame #3 {
                    n1977 = case shown="False" w3787 {
                      tunnel: w3788 -> [w3794 w3798]
                      tunnel: [w3795 w3798] -> w3789
                      tunnel: [w3796 w3797] -> w3790
                      tunnel: w3791 -> [w3793 w3797]
                      frame False {
                        n1978 = call "mDrive Send Command.vi"("error in (no error)"=w3793, "Command"=T10."Stop", "VISA resource name"=w3794) -> ("error out"=w3796:errorcluster, "VISA resource name out"=w3795:refnum<visa-resource-name>)  [unwired: 4 in, 1 out]
                      }
                      frame True {
                      }
                    }
                  }
                  frame #4 {
                    n1979 = property on="R Backlash corr" class="Bool (strict)"() -> ("Value"=w3799:bool)  [unwired: 2 in, 2 out]
                    n1980 = Implies(1:w3805, 2:w3799) -> (0:w3804:bool)
                    n1981 = case shown="False" w3804 {
                      tunnel: w3803 -> [w3813 w3870]
                      tunnel: w3802 -> [w3812 w3871]
                      tunnel: [w3807 w3870] -> w3801
                      tunnel: [w3811 w3871] -> w3800
                      frame False {
                        # "Backlash"
                        n1982 = flat-sequence {
                          tunnel: [w3826] -> w3825
                          tunnel: [w3830] -> w3824
                          tunnel: [w3829] -> w3823
                          tunnel: w3813 -> [w3828]
                          tunnel: w3812 -> [w3827]
                          tunnel: w3825 -> [w3838]
                          tunnel: [w3838] -> w3822
                          tunnel: w3824 -> [w3837]
                          tunnel: w3823 -> [w3836]
                          tunnel: [w3835] -> w3821
                          tunnel: [w3834] -> w3820
                          tunnel: [w3833] -> w3810
                          tunnel: w3822 -> [w3852]
                          tunnel: w3821 -> [w3843]
                          tunnel: w3820 -> [w3851]
                          tunnel: [w3843] -> w3819
                          tunnel: [w3851] -> w3818
                          tunnel: [w3842] -> w3815
                          tunnel: [w3850] -> w3814
                          tunnel: w3810 -> [w3850]
                          tunnel: w3819 -> [w3855]
                          tunnel: w3818 -> [w3856]
                          tunnel: [w3854] -> w3817
                          tunnel: [w3862] -> w3816
                          tunnel: w3815 -> [w3862]
                          tunnel: w3814 -> [w3858]
                          tunnel: [w3857] -> w3808
                          tunnel: w3817 -> [w3865]
                          tunnel: w3816 -> [w3864]
                          tunnel: [w3866] -> w3809
                          tunnel: w3808 -> [w3866]
                          tunnel: [w3865] -> w3806
                          tunnel: [w3869] -> w3811
                          tunnel: w3809 -> [w3869]
                          tunnel: [w3868] -> w3807
                          tunnel: w3806 -> [w3868]
                          frame #0 {
                            n1983 = property on="R Backlash steps/sec" class="DigNum (strict)"() -> ("Value"=w3826:i32)  [unwired: 2 in, 2 out]
                            n1984 = Number To Decimal String(number=w3826) -> (decimal integer string=w3831:string)  [unwired: 1 in]
                            n1985 = call "mDrive Send Command.vi"("error in (no error)"=w3828, "Extra"=w3831, "Command"=T10."Max Velocity", "VISA resource name"=w3827) -> ("error out"=w3829:errorcluster, "VISA resource name out"=w3830:refnum<visa-resource-name>)  [unwired: 3 in, 1 out]
                          }
                          frame #1 {
                            n1986 = property on="R Backlash steps/sec" class="DigNum (strict)"() -> ("Value"=w3833:i32)  [unwired: 2 in, 2 out]
                            n1987 = Number To Decimal String(number=w3833) -> (decimal integer string=w3839:string)  [unwired: 1 in]
                            n1988 = call "mDrive Send Command.vi"("error in (no error)"=w3836, "Extra"=w3839, "Command"=T10."Move to Relative Position", "VISA resource name"=w3837) -> ("error out"=w3835:errorcluster, "VISA resource name out"=w3834:refnum<visa-resource-name>)  [unwired: 3 in, 1 out]
                          }
                          frame #2 {
                            n1989 = To Double Precision Float(number=w3850) -> (double precision float=w3848:dbl)
                            n1990 = To Double Precision Float(number=w3852) -> (double precision float=w3853:dbl)
                            n1991 = Absolute Value(x=w3848) -> (abs(x)=w3849:dbl)
                            n1992 = Divide(x=w3849, y=w3853) -> (x/y=w3846:dbl)
                            n1993 = Multiply(x=1000.0, y=w3846) -> (x*y=w3844:dbl)
                            n1994 = Add(x=w3844, y=300.0) -> (x+y=w3842:dbl)
                            n1995 = To Unsigned Long Integer(number=w3842) -> (unsigned 32bit integer=w3841:u32)
                            n1996 = Wait (ms)(milliseconds to wait=w3841) -> ()  [unwired: 1 out]
                          }
                          frame #3 {
                            n1997 = Negate(x=w3858) -> (-x=w3859:i32)
                            n1998 = Number To Decimal String(number=w3859) -> (decimal integer string=w3860:string)  [unwired: 1 in]
                            n1999 = call "mDrive Send Command.vi"("error in (no error)"=w3855, "Extra"=w3860, "Command"=T10."Move to Relative Position", "VISA resource name"=w3856) -> ("error out"=w3854:errorcluster, "VISA resource name out"=w3857:refnum<visa-resource-name>)  [unwired: 3 in, 1 out]
                          }
                          frame #4 {
                            n2000 = To Unsigned Long Integer(number=w3864) -> (unsigned 32bit integer=w3863:u32)
                            n2001 = Wait (ms)(milliseconds to wait=w3863) -> ()  [unwired: 1 out]
                          }
                          frame #5 {
                            n2002 = property on="R Backlash corr" class="Bool (strict)"("Val(Sgnl)"=FALSE ("Value (Signaling)")) -> ()  [unwired: 2 in, 2 out]
                          }
                        }
                      }
                      frame True {
                      }
                    }
                  }
                }
                n2003 = property on="Y in Motion" class="Bool (strict)"() -> ("Value"=w3679:bool)  [unwired: 2 in, 2 out]
                n2004 = property on="Z in Motion" class="Bool (strict)"() -> ("Value"=w3667:bool)  [unwired: 2 in, 2 out]
                n2005 = property on="X  in Motion" class="Bool (strict)"() -> ("Value"=w3678:bool)  [unwired: 2 in, 2 out]
                n2006 = property on="R in Motion" class="Bool (strict)"() -> ("Value"=w3666:bool)  [unwired: 2 in, 2 out]
                n2007 = Compound Arithmetic op=OR(w3678, w3679, w3667, w3666) -> (w3677:bool)
                n2008 = Not(x=w3677) -> (.not. x?=w3672:bool)
              }
            }
            frame #7 {
              n2009 = Wait (ms)(milliseconds to wait=u32 1000) -> ()  [unwired: 1 out]
            }
          }
          n2010 = Increment(x=w2711) -> (x+1=w2712:i32)
          n2011 = property on="#th loop" class="DigNum (strict)"("Val(Sgnl)"=w2712) -> ()  [unwired: 2 in, 2 out]
          n2012 = property on="#th loop" class="DigNum (strict)"() -> ("Value"=w2701:dbl)  [unwired: 2 in, 2 out]
          n2013 = property on="# of loops" class="DigNum (strict)"() -> ("Value"=w2702:dbl)  [unwired: 2 in, 2 out]
          n2014 = Greater Or Equal?(x=w2701, y=w2702) -> (x >= y?=w2700:bool)
        }
        n2015 = flat-sequence {
          tunnel: [w4266] -> _
          tunnel: w2683 -> [w4266]
          tunnel: w2682 -> [_]
          tunnel: [w4265] -> _
          tunnel: w2681 -> [w4265]
          tunnel: w2680 -> [_]
          frame #0 {
            w4269 = T9."Enabled" ("Disabled")
            n2016 = local write "STATUS"("LEAVING LOOP" ("STATUS")) -> ()
            n2017 = property on="Z Scan Length SP steps" class="DigNum (strict)"("DisabledEnum"=T9."Enabled" ("Disabled")) -> ()  [unwired: 2 in, 2 out]
            n2018 = property on="Z Scan Velocity SP steps/sec" class="DigNum (strict)"("DisabledEnum"=T9."Enabled" ("Disabled")) -> ()  [unwired: 2 in, 2 out]
            n2019 = property on="R Scan Length SP steps" class="DigNum (strict)"("DisabledEnum"=T9."Enabled" ("Disabled")) -> ()  [unwired: 2 in, 2 out]
            n2020 = property on="X Scan Velocity SP steps/sec" class="DigNum (strict)"("DisabledEnum"=T9."Enabled" ("Disabled")) -> ()  [unwired: 2 in, 2 out]
            n2021 = property on="GO" class="Bool"("DisabledEnum"=w4269) -> ()  [unwired: 2 in, 2 out]
            n2022 = property on="Set Scan \nParameters" class="Bool"("DisabledEnum"=w4269) -> ()  [unwired: 2 in, 2 out]
            n2023 = property on="Y Scan Length SP steps" class="DigNum (strict)"("DisabledEnum"=T9."Enabled" ("Disabled")) -> ()  [unwired: 2 in, 2 out]
            n2024 = property on="R Scan Velocity SP steps/sec" class="DigNum (strict)"("DisabledEnum"=T9."Enabled" ("Disabled")) -> ()  [unwired: 2 in, 2 out]
            n2025 = property on="X Scan Length SP steps" class="DigNum (strict)"("DisabledEnum"=T9."Enabled" ("Disabled")) -> ()  [unwired: 2 in, 2 out]
            n2026 = property on="Y Scan Selocity SP steps/sec" class="DigNum (strict)"("DisabledEnum"=T9."Enabled" ("Disabled")) -> ()  [unwired: 2 in, 2 out]
            n2027 = property on="Send scan parameter" class="Bool"("DisabledEnum"=w4269) -> ()  [unwired: 2 in, 2 out]
            n2028 = property on="Scan Go" class="Bool (strict)"("DisabledEnum"=T9."Disabled and Grayed Out" ("Disabled")) -> ()  [unwired: 2 in, 2 out]
          }
        }
      }
    }
    n2029 = case shown="False" "Delete Button" {
      tunnel: w296 -> [_ w329]
      frame False {
      }
      frame True {
        n2030 = local read "Preset positions"() -> (w327:i32)
        n2031 = local read "Presets"() -> (w328:i32[][])
        n2032 = Delete From Array(array=w329, index=w327) -> (array with subset deleted=w325:string[])  [unwired: 1 in, 1 out]
        n2033 = property on="Preset positions" class="Ring (strict)"("Strings []"=w325) -> ()  [unwired: 2 in, 2 out]
        n2034 = Delete From Array(array=w328, index (row)=w327) -> (array with subset deleted=w326:i32[][])  [unwired: 2 in, 1 out]
        n2035 = local write "Presets"(w326) -> ()
      }
    }
    n2036 = case shown="False" "Add Button" {
      tunnel: w296 -> [_ w339]
      frame False {
      }
      frame True {
        n2037 = property on="X Step PV" class="DigNum (strict)"() -> ("Value"=w333:i32)  [unwired: 2 in, 2 out]
        n2038 = property on="Y Step PV" class="DigNum (strict)"() -> ("Value"=w332:i32)  [unwired: 2 in, 2 out]
        n2039 = property on="Z Step PV" class="DigNum (strict)"() -> ("Value"=w330:i32)  [unwired: 2 in, 2 out]
        n2040 = property on="R Step PV" class="DigNum (strict)"() -> ("Value"=w331:i32)  [unwired: 2 in, 2 out]
        n2041 = Build Array(w333, w332, w330, w331) -> (w336:i32[])
        n2042 = Build Array (concatenate)(w339, "String") -> (w334:string[])
        n2043 = local read "Presets"() -> (w337:i32[][])
        n2044 = property on="Preset positions" class="Ring (strict)"("Strings []"=w334) -> ()  [unwired: 2 in, 2 out]
        n2045 = Build Array (concatenate)(w337, w336) -> (w335:i32[][])
        n2046 = local write "Presets"(w335) -> ()
      }
    }
    n2047 = case shown="False" "Set Button" {
      tunnel: "Preset positions" -> [_ w346]
      frame False {
      }
      frame True {
        n2048 = local read "Presets"() -> (w347:i32[][])
        n2049 = Index Array(array=w347, index (row)=w346) -> (element=w345:i32[])  [unwired: 1 in]
        n2050 = Array To Cluster(array=w345) -> (cluster=w344:T11)
        n2051 = Unbundle(w344) -> ("Presets[0]"=w343:i32, "Presets[1]"=w342:i32, "Presets[2]"=w341:i32, "Presets[3]"=w340:i32)  [unwired: 5 out]
        n2052 = property on="X Step SP" class="DigNum (strict)"("Val(Sgnl)"=w343) -> ()  [unwired: 2 in, 2 out]
        n2053 = property on="Y Step SP" class="DigNum (strict)"("Val(Sgnl)"=w342) -> ()  [unwired: 2 in, 2 out]
        n2054 = property on="Z Step SP" class="DigNum (strict)"("Val(Sgnl)"=w341) -> ()  [unwired: 2 in, 2 out]
        n2055 = property on="R Step SP" class="DigNum (strict)"("Val(Sgnl)"=w340) -> ()  [unwired: 2 in, 2 out]
      }
    }
    n2056 = property on="STATUS" class="Str"() -> ("Value"=w289:string)  [unwired: 2 in, 2 out]
    n2057 = Equal?(x=w289, y="SCANNING MODE" ("STATUS")) -> (x = y?=w287:bool)
    "Scanning" <- w287
    n2058 = case shown="True" "Laser Shutter" {
      tunnel: "SHUTTER SYNC" -> [w323 _]
      tunnel: w287 -> [w322 _]
      frame False {
        # "SHUTTER SLAVE MODE"
        n2059 = And(x=w323, y=w322) -> (x .and. y?=w324:bool)
        n2060 = case shown="False" w324 {
          frame False {
            # "CLOE SHUTTER"
          }
          frame True {
            # "OPEN SHUTTER"
          }
        }
      }
      frame True {
        # "FORCE TO OPEN SHUTTER"
      }
    }
    n2061 = case shown="True" "Stop" {
      selector: "Stop" -> [w356 w398]
      tunnel: [w356 w395] -> w303
      tunnel: w286 -> [w355 w364]
      tunnel: w283 -> [w354 w363]
      tunnel: [w355 w371] -> w312
      tunnel: [w353 w377] -> w311
      tunnel: [w352 w374] -> w310
      tunnel: [w351 w383] -> w309
      tunnel: [w349 w366] -> w308
      tunnel: [w348 w365] -> w307
      tunnel: [w350 w380] -> w306
      tunnel: [w354 w368] -> w305
      tunnel: w302 -> [_ w390]
      tunnel: w301 -> [_ w367]
      tunnel: w285 -> [w353 w362]
      tunnel: w284 -> [w352 w361]
      tunnel: w282 -> [w351 w360]
      tunnel: w281 -> [w350 w359]
      tunnel: w280 -> [w348 w358]
      tunnel: w279 -> [w349 w357]
      frame False {
      }
      frame True {
        n2062 = flat-sequence {
          tunnel: w398 -> [w464]
          tunnel: [w464] -> w397
          tunnel: [w463] -> w393
          tunnel: [w462] -> w391
          tunnel: w390 -> [w462]
          tunnel: [w417] -> w388
          tunnel: [w416] -> w386
          tunnel: [w426] -> w384
          tunnel: [w425] -> w381
          tunnel: [w436] -> w378
          tunnel: [w434] -> w375
          tunnel: [w445] -> w372
          tunnel: [w443] -> w369
          tunnel: w367 -> [w453]
          tunnel: w364 -> [w406]
          tunnel: w363 -> [w405]
          tunnel: w362 -> [w404]
          tunnel: w361 -> [w403]
          tunnel: w360 -> [w402]
          tunnel: w359 -> [w401]
          tunnel: w358 -> [w400]
          tunnel: w357 -> [w399]
          tunnel: w397 -> [w476]
          tunnel: [w476] -> w396
          tunnel: [w465] -> w394
          tunnel: w393 -> [w475]
          tunnel: [w474] -> w392
          tunnel: w391 -> [w474]
          tunnel: [w473] -> w389
          tunnel: w388 -> [w473]
          tunnel: [w472] -> w387
          tunnel: w386 -> [w472]
          tunnel: [w471] -> w385
          tunnel: w384 -> [w471]
          tunnel: [w470] -> w382
          tunnel: w381 -> [w470]
          tunnel: [w469] -> w379
          tunnel: w378 -> [w469]
          tunnel: [w468] -> w376
          tunnel: w375 -> [w468]
          tunnel: [w467] -> w373
          tunnel: w372 -> [w467]
          tunnel: [w466] -> w370
          tunnel: w369 -> [w466]
          tunnel: w396 -> [w488]
          tunnel: [w488] -> w395
          tunnel: w394 -> [w479]
          tunnel: w392 -> [w487]
          tunnel: w389 -> [w478]
          tunnel: [w478] -> _
          tunnel: w387 -> [w486]
          tunnel: [w486] -> w365
          tunnel: w385 -> [w485]
          tunnel: [w485] -> w383
          tunnel: [w484] -> w380
          tunnel: w382 -> [w484]
          tunnel: [w483] -> w377
          tunnel: w379 -> [w483]
          tunnel: [w482] -> w374
          tunnel: w376 -> [w482]
          tunnel: [w481] -> w371
          tunnel: w373 -> [w481]
          tunnel: [w480] -> w368
          tunnel: w370 -> [w480]
          tunnel: [w478] -> w366
          frame #0 {
            # "R"
            # "Y"
            # "Z"
            # "X"
            n2063 = local read "Presets"() -> (w452:i32[][])
            n2064 = property on="Preset positions" class="Ring (strict)"() -> ("Strings []"=w451:string[])  [unwired: 2 in, 2 out]
            n2065 = property on="R Ready" class="Bool (strict)"("Val(Sgnl)"=FALSE ("Value (Signaling)")) -> ()  [unwired: 2 in, 2 out]
            n2066 = property on="R in Range" class="Bool (strict)"("Val(Sgnl)"=FALSE ("Value (Signaling)")) -> ()  [unwired: 2 in, 2 out]
            n2067 = property on="Z in Range" class="Bool (strict)"("Val(Sgnl)"=FALSE ("Value (Signaling)")) -> ()  [unwired: 2 in, 2 out]
            n2068 = property on="Z Ready" class="Bool (strict)"("Val(Sgnl)"=FALSE ("Value (Signaling)")) -> ()  [unwired: 2 in, 2 out]
            n2069 = property on="Y in Range" class="Bool (strict)"("Val(Sgnl)"=FALSE ("Value (Signaling)")) -> ()  [unwired: 2 in, 2 out]
            n2070 = property on="X  in Range" class="Bool (strict)"("Val(Sgnl)"=FALSE ("Value (Signaling)")) -> ()  [unwired: 2 in, 2 out]
            n2071 = property on="Y Ready" class="Bool (strict)"("Val(Sgnl)"=FALSE ("Value (Signaling)")) -> ()  [unwired: 2 in, 2 out]
            n2072 = property on="X Ready" class="Bool (strict)"("Val(Sgnl)"=FALSE ("Value (Signaling)")) -> ()  [unwired: 2 in, 2 out]
            n2073 = Number To Fractional String(number=w452) -> (F-format string=w454:string[][])  [unwired: 3 in]
            n2074 = call "mDrive Send Command.vi"("error in (no error)"=w405, "Command"=T10."Stop", "VISA resource name"=w406) -> ("error out"=w444:errorcluster, "VISA resource name out"=w446:refnum<visa-resource-name>)  [unwired: 4 in, 1 out]
            n2075 = call "mDrive Send Command.vi"("error in (no error)"=w403, "Command"=T10."Stop", "VISA resource name"=w404) -> ("error out"=w435:errorcluster, "VISA resource name out"=w437:refnum<visa-resource-name>)  [unwired: 4 in, 1 out]
            n2076 = Transpose 2D Array(2D array=w454) -> (transposed array=w455:string[][])
            n2077 = call "mDrive Send Command.vi"("error in (no error)"=w401, "Command"=T10."Stop", "VISA resource name"=w402) -> ("error out"=w427:errorcluster, "VISA resource name out"=w428:refnum<visa-resource-name>)  [unwired: 4 in, 1 out]
            n2078 = call "mDrive Send Command.vi"("error in (no error)"=w400, "Command"=T10."Stop", "VISA resource name"=w399) -> ("error out"=w418:errorcluster, "VISA resource name out"=w419:refnum<visa-resource-name>)  [unwired: 4 in, 1 out]
            n2079 = Build Array (concatenate)(w451, w455) -> (w456:string[][])
            n2080 = Transpose 2D Array(2D array=w456) -> (transposed array=w457:string[][])
            n2081 = call "mDrive Send Command.vi"("error in (no error)"=w444, "Extra"="P", "Command"=T10."Print Parameter", "VISA resource name"=w446) -> ("error out"=w443:errorcluster, "read buffer"=w450:string, "VISA resource name out"=w445:refnum<visa-resource-name>)  [unwired: 3 in]
            n2082 = call "mDrive Send Command.vi"("error in (no error)"=w435, "Extra"="P", "Command"=T10."Print Parameter", "VISA resource name"=w437) -> ("error out"=w434:errorcluster, "read buffer"=w441:string, "VISA resource name out"=w436:refnum<visa-resource-name>)  [unwired: 3 in]
            n2083 = call "mDrive Send Command.vi"("error in (no error)"=w427, "Extra"="P", "Command"=T10."Print Parameter", "VISA resource name"=w428) -> ("error out"=w425:errorcluster, "read buffer"=w432:string, "VISA resource name out"=w426:refnum<visa-resource-name>)  [unwired: 3 in]
            n2084 = call "mDrive Send Command.vi"("error in (no error)"=w418, "Extra"="P", "Command"=T10."Print Parameter", "VISA resource name"=w419) -> ("error out"=w416:errorcluster, "read buffer"=w423:string, "VISA resource name out"=w417:refnum<visa-resource-name>)  [unwired: 3 in]
            n2085 = call-poly <vilib>:"Write To Spreadsheet File.vi"("2D data"=w457, "file path (dialog if empty)"=w453) -> ()  [unwired: 6 in, 1 out]
            n2086 = Decimal String To Number(string=w450, offset=0) -> (number=w442:i32)  [unwired: 1 in, 1 out]
            n2087 = Decimal String To Number(string=w441, offset=0) -> (number=w433:i32)  [unwired: 1 in, 1 out]
            n2088 = Decimal String To Number(string=w432, offset=0) -> (number=w424:i32)  [unwired: 1 in, 1 out]
            n2089 = Decimal String To Number(string=w423, offset=0) -> (number=w415:i32)  [unwired: 1 in, 1 out]
            n2090 = Build Array(w442, w424, w433, w415) -> (w463:i32[])
          }
          frame #1 {
            n2091 = To Double Precision Float(number=w475) -> (double precision float=w465:dbl[])
            n2092 = Wait (ms)(milliseconds to wait=u32 20) -> ()  [unwired: 1 out]
          }
          frame #2 {
            n2093 = call-poly <vilib>:"Write To Spreadsheet File.vi"("1D data"=w479, "file path (dialog if empty)"=w487) -> ()  [unwired: 6 in, 1 out]
          }
        }
      }
    }
  }
  n2094 = flat-sequence {
    tunnel: w58 -> [w4300]
    tunnel: w57 -> [w4297]
    frame #0 {
      n2095 = call "mDrive Send Command.vi"("error in (no error)"=w4297, "Command"=T10."Stop", "VISA resource name"=w4300) -> ("error out"=w4298:errorcluster, "VISA resource name out"=w4299:refnum<visa-resource-name>)  [unwired: 4 in, 1 out]
      n2096 = VISA Close(VISA resource name=w4299, error in (no error)=w4298) -> ()  [unwired: 1 out]
    }
  }
  n2097 = flat-sequence {
    tunnel: w52 -> [w4305]
    tunnel: w51 -> [w4302]
    frame #0 {
      n2098 = call "mDrive Send Command.vi"("error in (no error)"=w4302, "Command"=T10."Stop", "VISA resource name"=w4305) -> ("error out"=w4303:errorcluster, "VISA resource name out"=w4304:refnum<visa-resource-name>)  [unwired: 4 in, 1 out]
      n2099 = VISA Close(VISA resource name=w4304, error in (no error)=w4303) -> ()  [unwired: 1 out]
    }
  }
  n2100 = flat-sequence {
    tunnel: w50 -> [w4310]
    tunnel: w49 -> [w4307]
    frame #0 {
      n2101 = call "mDrive Send Command.vi"("error in (no error)"=w4307, "Command"=T10."Stop", "VISA resource name"=w4310) -> ("error out"=w4308:errorcluster, "VISA resource name out"=w4309:refnum<visa-resource-name>)  [unwired: 4 in, 1 out]
      n2102 = VISA Close(VISA resource name=w4309, error in (no error)=w4308) -> ()  [unwired: 1 out]
    }
  }
  n2103 = flat-sequence {
    tunnel: w48 -> [w4315]
    tunnel: w47 -> [w4312]
    frame #0 {
      n2104 = call "mDrive Send Command.vi"("error in (no error)"=w4312, "Command"=T10."Stop", "VISA resource name"=w4315) -> ("error out"=w4313:errorcluster, "VISA resource name out"=w4314:refnum<visa-resource-name>)  [unwired: 4 in, 1 out]
      n2105 = VISA Close(VISA resource name=w4314, error in (no error)=w4313) -> ()  [unwired: 1 out]
    }
  }
  "YCONSTArray" <- w46
  "XCONSTArray" <- w45
  "RCONSTArray" <- w44
  "ZCONSTArray" <- w43
  "RUNHOLDArray" <- w42
